vi "Lab Panel V4.6.vi"() -> ()   [LabVIEW 2013]
uses:
  <vilib>/Platform/TimedLoop/XDataNode/timing_clust.ctl
  <vilib>/Platform/TimedLoop/XDataNode/nitl_modes.ctl
  <vilib>/Platform/TimedLoop/XDataNode/wakeup.ctl
  Global 1.vi
  <vilib>/platform/TimedLoop/XDataNode/XDataNode.xnode
  <vilib>/Platform/TimedLoop/XDataNode/XDNodeRunTimeDep.lvlib
panel:
  in  "ADMIN PAGE":bool
  out "TEMP update":bool
  out "AI update":bool
  in  "Tab Control 2":T1(tab)
  out "SIG LAB05-2":T2 {"PF" format="%.2f"; "AMPS" format="%.1f"}
  out "SIG LAB05-1":T2 {"PF" format="%.2f"; "AMPS" format="%.1f"}
  out "SIG LAB04-2":T2 {"PF" format="%.2f"; "AMPS" format="%.1f"}
  out "SIG LAB04-1":T2 {"PF" format="%.2f"; "AMPS" format="%.1f"}
  out "SIG LAB03-2":T2 {"PF" format="%.2f"; "AMPS" format="%.1f"}
  out "SIG LAB03-1":T2 {"PF" format="%.2f"; "AMPS" format="%.1f"}
  out "SIG LAB02-2":T2 {"PF" format="%.2f"; "AMPS" format="%.1f"}
  in  "RUN LAB01-1":bool
  in  "O/I  LAB05-1":bool
  in  "O/I  LAB05-2":bool
  in  "O/I  LAB04-1":bool
  in  "O/I  LAB04-2":bool
  in  "O/I  LAB02-1":bool
  in  "O/I  LAB02-2":bool
  in  "O/I  LAB01-2":bool
  in  "O/I  LAB01-1":bool
  in  "O/I  LAB03-1":bool
  in  "RUN LAB05-2":bool
  in  "RUN LAB05-1":bool
  in  "RUN LAB04-2":bool
  in  "RUN LAB04-1":bool
  in  "RUN LAB03-2":bool
  in  "RUN LAB03-1":bool
  in  "RUN LAB02-2":bool
  in  "RUN LAB02-1":bool
  in  "RUN LAB01-2":bool
  in  "SELECT LAB05-2":T3(radio)
  in  "SELECT LAB05-1":T3(radio)
  in  "SELECT LAB04-2":T3(radio)
  in  "SELECT LAB04-1":T3(radio)
  in  "SELECT LAB03-2":T3(radio)
  in  "SELECT LAB03-1":T3(radio)
  in  "SELECT LAB02-2":T3(radio)
  in  "SELECT LAB02-1":T3(radio)
  in  "SELECT LAB01-2":T3(radio)
  in  "SELECT LAB01-1":T3(radio)
  in  "O/I  LAB03-2":bool
  out "SIG LAB01-1":T2 {"PF" format="%.2f"; "AMPS" format="%.1f"}
  out "SIG LAB01-2":T2 {"PF" format="%.2f"; "AMPS" format="%.1f"}
  out "SIG LAB02-1":T2 {"PF" format="%.2f"; "AMPS" format="%.1f"}
  out "DISP LAB05-2":T4 {"MINS" format="%.2g"}
  out "DISP LAB05-1":T4 {"MINS" format="%.2g"}
  out "DISP LAB04-2":T4 {"MINS" format="%.2g"}
  out "DISP LAB04-1":T4 {"MINS" format="%.2g"}
  out "DISP LAB03-2":T4 {"MINS" format="%.2g"}
  out "DISP LAB03-1":T4 {"MINS" format="%.2g"}
  in  "SET LAB05-2":T5={"NAME"="", "DESCRIPTION"="", "CYCLES"=5.0, "T-RISE mins"=0.0, "T-RISE deg C"=0.0} {"CYCLES" min=5.0 step=1.0}
  in  "SET LAB05-1":T5={"NAME"="", "DESCRIPTION"="", "CYCLES"=5.0, "T-RISE mins"=0.0, "T-RISE deg C"=0.0} {"CYCLES" min=5.0 step=1.0}
  in  "SET LAB04-2":T5={"NAME"="", "DESCRIPTION"="", "CYCLES"=5.0, "T-RISE mins"=0.0, "T-RISE deg C"=0.0} {"CYCLES" min=5.0 step=1.0}
  in  "SET LAB04-1":T5={"NAME"="", "DESCRIPTION"="", "CYCLES"=5.0, "T-RISE mins"=0.0, "T-RISE deg C"=0.0} {"CYCLES" min=5.0 step=1.0}
  in  "SET LAB03-2":T5={"NAME"="", "DESCRIPTION"="", "CYCLES"=5.0, "T-RISE mins"=0.0, "T-RISE deg C"=0.0} {"CYCLES" min=5.0 step=1.0}
  in  "SET LAB03-1":T5={"NAME"="", "DESCRIPTION"="", "CYCLES"=5.0, "T-RISE mins"=0.0, "T-RISE deg C"=0.0} {"CYCLES" min=5.0 step=1.0}
  out "DISP LAB02-2":T4 {"MINS" format="%.2g"}
  out "DISP LAB02-1":T4 {"MINS" format="%.2g"}
  in  "SET LAB02-2":T5={"NAME"="", "DESCRIPTION"="", "CYCLES"=5.0, "T-RISE mins"=0.0, "T-RISE deg C"=0.0} {"CYCLES" min=5.0 step=1.0}
  in  "SET LAB02-1":T5={"NAME"="", "DESCRIPTION"="", "CYCLES"=5.0, "T-RISE mins"=0.0, "T-RISE deg C"=0.0} {"CYCLES" min=5.0 step=1.0}
  out "RESULT LAB05-2":bool
  out "RESULT LAB05-1":bool
  out "RESULT LAB04-2":bool
  out "RESULT LAB04-1":bool
  out "RESULT LAB03-2":bool
  out "RESULT LAB03-1":bool
  out "RESULT LAB02-2":bool
  out "RESULT LAB02-1":bool
  out "RESULT LAB01-2":bool
  out "RESULT LAB01-1":bool
  in  "SET LAB01-1":T5={"NAME"="", "DESCRIPTION"="", "CYCLES"=5.0, "T-RISE mins"=0.0, "T-RISE deg C"=0.0} {"CYCLES" min=5.0 step=1.0}
  in  "SET LAB01-2":T5={"NAME"="", "DESCRIPTION"="", "CYCLES"=5.0, "T-RISE mins"=0.0, "T-RISE deg C"=0.0} {"CYCLES" min=5.0 step=1.0}
  out "DISP LAB01-1":T4 {"MINS" format="%.2g"}
  out "DISP LAB01-2":T4 {"MINS" format="%.2f"}
  out "TEMP RISE LAB05-2":cluster{"TL":dbl, "TN":dbl}
  out "TEMP RISE LAB05-1":cluster{"TL":dbl, "TN":dbl}
  out "TEMP RISE LAB04-2":cluster{"TL":dbl, "TN":dbl}
  out "TEMP RISE LAB04-1":cluster{"TL":dbl, "TN":dbl}
  out "TEMP RISE LAB03-2":cluster{"TL":dbl, "TN":dbl}
  out "TEMP RISE LAB03-1":cluster{"TL":dbl, "TN":dbl}
  out "TEMP RISE LAB02-2":cluster{"TL":dbl, "TN":dbl}
  out "TEMP RISE LAB02-1":cluster{"TL":dbl, "TN":dbl}
  out "TEMP RISE LAB01-2":cluster{"TL":dbl, "TN":dbl}
  out "TEMP RISE LAB01-1":cluster{"TL":dbl, "TN":dbl}
  in  "JIG OFF TIME (S)":dbl=2.0 min=2.0 max=10.0 step=0.5 format="%.1g"
  in  "JIG ON TIME (S)":dbl=1.0 min=1.0 max=10.0 step=0.5 format="%.1g"
  out "JIG LAB05-2":bool
  out "JIG LAB05-1":bool
  out "JIG LAB04-2":bool
  out "JIG LAB04-1":bool
  out "JIG LAB03-2":bool
  out "JIG LAB03-1":bool
  out "JIG LAB02-2":bool
  out "JIG LAB02-1":bool
  out "JIG LAB01-2":bool
  out "JIG LAB01-1":bool
  out "TEMP START LAB01-1":cluster{"TL":dbl, "TN":dbl}
  out "TEMP START LAB02-1":cluster{"TL":dbl, "TN":dbl}
  out "TEMP START LAB03-1":cluster{"TL":dbl, "TN":dbl}
  out "TEMP START LAB04-1":cluster{"TL":dbl, "TN":dbl}
  out "TEMP START LAB01-2":cluster{"TL":dbl, "TN":dbl}
  out "TEMP START LAB02-2":cluster{"TL":dbl, "TN":dbl}
  out "TEMP START LAB03-2":cluster{"TL":dbl, "TN":dbl}
  out "TEMP START LAB04-2":cluster{"TL":dbl, "TN":dbl}
  out "TEMP START LAB05-2":cluster{"TL":dbl, "TN":dbl}
  out "TEMP START LAB05-1":cluster{"TL":dbl, "TN":dbl}
  in  "MAIL SETTINGS":T6
  out "MAIL REPORT":string
  in  "TO (string):":string
  in  "Send Mail Now":bool
  in  "Auto Mail Send":bool
  in  "Network Directory":path
  out "CAL LAB01":T7 {"2 (TN) cal" min=0.0 step=0.01 format="%.2f"; "2 (TL) cal" min=0.0 step=0.01 format="%.2f"; "2 (PF) cal" min=0.0 step=0.01 format="%.2f"; "2 (V) cal" min=0.0 step=0.01 format="%.2f"; "2 (A) cal" min=0.0 step=0.01 format="%.2f"; "1 (TN) cal" min=0.0 step=0.01 format="%.2f"; "1 (TL) cal" min=0.0 step=0.01 format="%.2f"; "1 (PF) cal" min=0.0 step=0.01 format="%.2f"; "1 (V) cal" min=0.0 step=0.01 format="%.2f"; "1  (A) cal" min=0.0 step=0.01 format="%.2f"}
  out "CAL LAB03":T7 {"2 (TN) cal" min=0.0 step=0.01 format="%.2f"; "2 (TL) cal" min=0.0 step=0.01 format="%.2f"; "2 (PF) cal" min=0.0 step=0.01 format="%.2f"; "2 (V) cal" min=0.0 step=0.01 format="%.2f"; "2 (A) cal" min=0.0 step=0.01 format="%.2f"; "1 (TN) cal" min=0.0 step=0.01 format="%.2f"; "1 (TL) cal" min=0.0 step=0.01 format="%.2f"; "1 (PF) cal" min=0.0 step=0.01 format="%.2f"; "1 (V) cal" min=0.0 step=0.01 format="%.2f"; "1  (A) cal" min=0.0 step=0.01 format="%.2f"}
  out "CAL LAB02":T8 {"2 (TN) cal" min=0.0 step=0.01 format="%.2f"; "2 (TL) cal" min=0.0 step=0.01 format="%.2f"; "2 (PF) cal" min=0.0 step=0.01 format="%.2f"; "2 (V) cal" min=0.0 step=0.01 format="%.2f"; "2 (A) cal" min=0.0 step=0.01 format="%.2f"; "1 (TN) cal" min=0.0 step=0.01 format="%.2f"; "1 (TL) cal" min=0.0 step=0.01 format="%.2f"; "1 (PF) cal" min=0.0 step=0.01 format="%.2f"; "1 (V) cal" min=0.0 step=0.01 format="%.2f"; "1 (A) cal" min=0.0 step=0.01 format="%.2f"}
  out "CAL LAB05":T7 {"2 (TN) cal" min=0.0 step=0.01 format="%.2f"; "2 (TL) cal" min=0.0 step=0.01 format="%.2f"; "2 (PF) cal" min=0.0 step=0.01 format="%.2f"; "2 (V) cal" min=0.0 step=0.01 format="%.2f"; "2 (A) cal" min=0.0 step=0.01 format="%.2f"; "1 (TN) cal" min=0.0 step=0.01 format="%.2f"; "1 (TL) cal" min=0.0 step=0.01 format="%.2f"; "1 (PF) cal" min=0.0 step=0.01 format="%.2f"; "1 (V) cal" min=0.0 step=0.01 format="%.2f"; "1  (A) cal" min=0.0 step=0.01 format="%.2f"}
  out "CAL LAB04":T7 {"2 (TN) cal" min=0.0 step=0.01 format="%.2f"; "2 (TL) cal" min=0.0 step=0.01 format="%.2f"; "2 (PF) cal" min=0.0 step=0.01 format="%.2f"; "2 (V) cal" min=0.0 step=0.01 format="%.2f"; "2 (A) cal" min=0.0 step=0.01 format="%.2f"; "1 (TN) cal" min=0.0 step=0.01 format="%.2f"; "1 (TL) cal" min=0.0 step=0.01 format="%.2f"; "1 (PF) cal" min=0.0 step=0.01 format="%.2f"; "1 (V) cal" min=0.0 step=0.01 format="%.2f"; "1  (A) cal" min=0.0 step=0.01 format="%.2f"}
  out "calibration file error out":errorcluster
  in  "CALIBRATE":bool
  out "ON L05-2":cluster{"amps":dbl, "volts":dbl, "pf":dbl}
  out "ON L05-1":cluster{"amps":dbl, "volts":dbl, "pf":dbl}
  out "FAIL LAB05-2":cluster{"LO":dbl, "HI":dbl}
  out "FAIL LAB05-1":cluster{"LO":dbl, "HI":dbl}
  out "FAIL LAB04-2":cluster{"LO":dbl, "HI":dbl}
  out "FAIL LAB04-1":cluster{"LO":dbl, "HI":dbl}
  out "FAIL LAB03-2":cluster{"LO":dbl, "HI":dbl}
  out "FAIL LAB03-1":cluster{"LO":dbl, "HI":dbl}
  out "FAIL LAB02-2":cluster{"LO":dbl, "HI":dbl}
  out "FAIL LAB02-1":cluster{"LO":dbl, "HI":dbl}
  out "FAIL LAB01-2":cluster{"LO":dbl, "HI":dbl}
  out "FAIL LAB01-1":cluster{"LO":dbl, "HI":dbl}
  out "ON L01-1":cluster{"amps":dbl, "volts":dbl, "pf":dbl}
  out "ON L01-2":cluster{"amps":dbl, "volts":dbl, "pf":dbl}
  out "ON L02-1":cluster{"amps":dbl, "volts":dbl, "pf":dbl}
  out "ON L02-2":cluster{"amps":dbl, "volts":dbl, "pf":dbl}
  out "ON L03-1":cluster{"amps":dbl, "volts":dbl, "pf":dbl}
  out "ON L03-2":cluster{"amps":dbl, "volts":dbl, "pf":dbl}
  out "ON L04-1":cluster{"amps":dbl, "volts":dbl, "pf":dbl}
  out "ON L04-2":cluster{"amps":dbl, "volts":dbl, "pf":dbl}
  out "TEST VOLTS CHART":T9(graph)
  in  "Select  Cycle":enum32{"ON CYCLE", "OFF CYCLE"}(radio)
  out "TEST AMPS CHART":T9(graph)
  out "TEMPERATURE (N) CHART":T9(graph)
  out "TEMPERATURE (L) CHART":T9(graph)
  in  "SAMPLES":dbl
  in  "RATE (Hz)":dbl
  in  "JIG TEST":T10
  in  "C drive data root dir":path
  out "run lab05-2":bool
  out "run lab05-1":bool
  out "run lab04-2":bool
  out "run lab04-1":bool
  out "run lab03-2":bool
  out "run lab03-1":bool
  out "run lab02-2":bool
  out "run lab02-1":bool
  out "run lab01-2":bool
  out "run lab01-1":bool
  out "stop2":bool
  in  "Tab Control":T11(tab)
  out "LAB01-2 (GRAPH)":dynamicdata(graph)
  out "LAB01-1 (GRAPH)":dynamicdata(graph)
  out "LAB02-2 (GRAPH)":dynamicdata(graph)
  out "LAB02-1 (GRAPH)":dynamicdata(graph)
  out "LAB03-2 (GRAPH)":dynamicdata(graph)
  out "LAB03-1 (GRAPH)":dynamicdata(graph)
  out "LAB04-2 (GRAPH)":dynamicdata(graph)
  out "LAB04-1 (GRAPH)":dynamicdata(graph)
  out "LAB05-2 (GRAPH)":dynamicdata(graph)
  out "LAB05-1 (GRAPH)":dynamicdata(graph)
  out "LAB05 TEMP":T12
  out "LAB04 TEMP":T12
  out "LAB02 TEMP":T12
  out "LAB01 TEMP":T12
  out "LAB03 TEMP":T12
  out "Analog Error Array":errorcluster[](array[cluster])
  out "AI loop time":dbl format="%.6g"
  out "loops":dbl
  in  "loop  delay(mS)":dbl
  out "on loops":dbl
  out "off loops":dbl
  out "jig cycle":dbl
  out "TDMS LAB01-1":refnum<k34>
  out "data file error":errorcluster
  out "TDMS LAB02-1":refnum<k34>
  out "TDMS LAB01-2":refnum<k34>
  out "TDMS LAB02-2":refnum<k34>
  out "TDMS LAB03-1":refnum<k34>
  out "TDMS LAB03-2":refnum<k34>
  out "TDMS LAB04-1":refnum<k34>
  out "TDMS LAB04-2":refnum<k34>
  out "TDMS LAB05-1":refnum<k34>
  out "TDMS LAB05-2":refnum<k34>
  out "mail control":string
  out "File Time Stamp":timestamp
  in  "stop":bool
  in  "Select COM port":refnum<visa-resource-name>="COM6"
  out "COM port":refnum<visa-resource-name>="COM6"
  # "LAB01"
  # "LAB02"
  # "LAB05"
  # "LAB03"
  # "LAB04"
  # "LAB01"
  # "LAB02"
  # "LAB03"
  # "LAB04"
  # "LAB05"
  # "JIG SET"
  # "(Enter recipients address seperated by comma)"
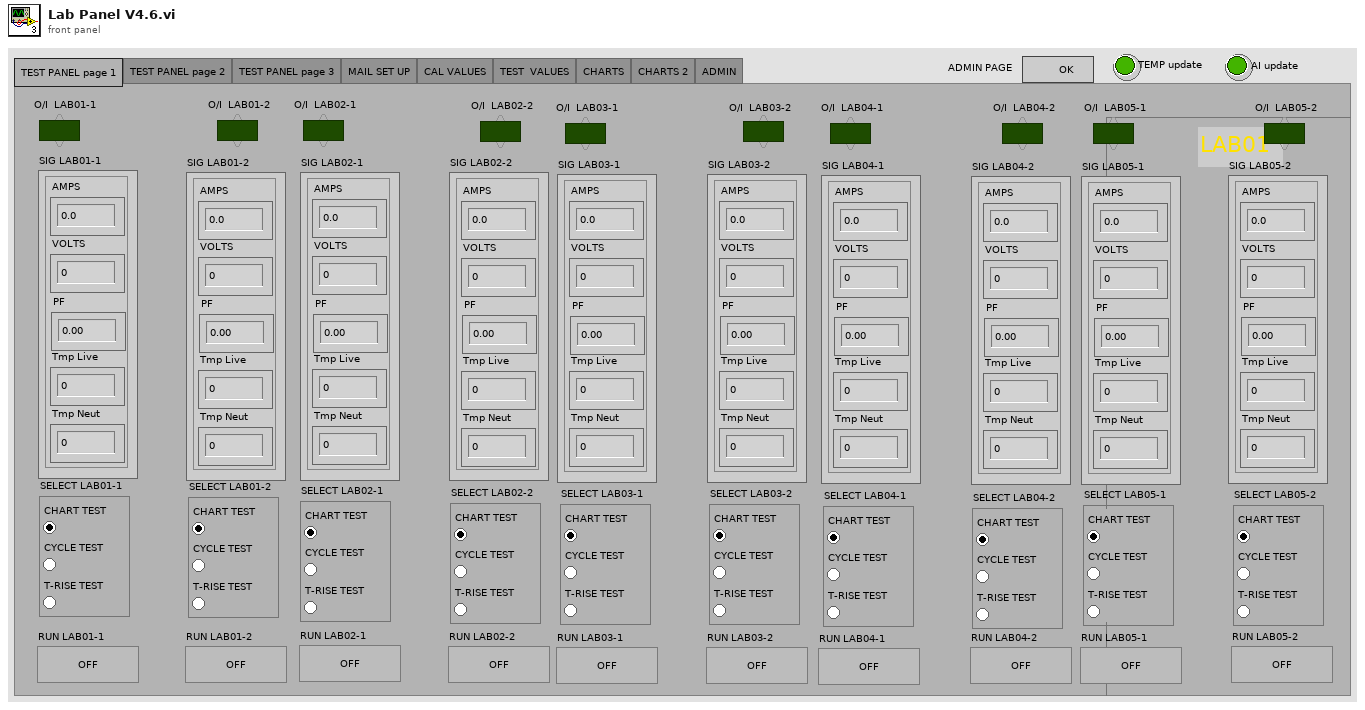
[diagram p1: front panel]
types:
  T1 = enum32{"TEST PANEL page 1", "TEST PANEL page 2", "TEST PANEL page 3", "MAIL SET UP", "CAL VALUES", "TEST  VALUES", "CHARTS", "CHARTS 2", "ADMIN"}
  T2 = cluster{"AMPS":dbl, "VOLTS":dbl, "PF":dbl, "Tmp Live":dbl, "Tmp Neut":dbl}
  T3 = enum32{"CHART TEST", "CYCLE TEST", "T-RISE TEST"}
  T4 = cluster{"CYCLE":dbl, "MINS":dbl, "STATUS":string}
  T5 = cluster{"NAME":string, "DESCRIPTION":string, "CYCLES":dbl, "T-RISE mins":dbl, "T-RISE deg C":dbl}
  T6 = cluster{"OUT SERVER ADDRESS":string, "FROM ACCOUNT":string, "USER NAME":string, "PASSWORD":string, "TEST MAIL":bool, "TEST MAIL STATUS":string, "mail error":errorcluster}
  T7 = cluster{"1  (A) cal":dbl, "1 (V) cal":dbl, "1 (PF) cal":dbl, "1 (TL) cal":dbl, "1 (TN) cal":dbl, "2 (A) cal":dbl, "2 (V) cal":dbl, "2 (PF) cal":dbl, "2 (TL) cal":dbl, "2 (TN) cal":dbl}
  T8 = cluster{"1 (A) cal":dbl, "1 (V) cal":dbl, "1 (PF) cal":dbl, "1 (TL) cal":dbl, "1 (TN) cal":dbl, "2 (A) cal":dbl, "2 (V) cal":dbl, "2 (PF) cal":dbl, "2 (TL) cal":dbl, "2 (TN) cal":dbl}
  T9 = cluster{"AMPS":dbl, "AMPS":dbl, "AMPS":dbl, "AMPS":dbl, "AMPS":dbl, "AMPS":dbl, "AMPS":dbl, "AMPS":dbl, "AMPS":dbl, "AMPS":dbl}
  T10 = cluster{" LAB01-1":bool, " LAB01-2":bool, "LAB02-1":bool, " LAB02-2":bool, "LAB03-1":bool, "LAB03-2":bool, "LAB04-1":bool, "LAB04-2":bool, "LAB05-1":bool, "LAB05-2":bool}
  T11 = enum32{"LAB01", "LAB02", "LAB03", "LAB04", "LAB05", "TEMPERATURE", "ERROR"}
  T12 = cluster{"T1 Live":dbl, "T1 Neut":dbl, "T2 Live":dbl, "T2 Neut":dbl, "ID":dbl, "ER":dbl}
  T13 = enum8{"Enabled", "Disabled", "Disabled and Grayed Out"}
  T14 = typedef "XDNodeRunTimeDep.lvlib/timing_clust.ctl" = cluster{"Expected End [f-1]":u64, "Actual End [f-1]":u64, "Finished Late? [f-1]":bool, "Expected End [i-1]":u64, "Actual End [i-1]":u64, "Finished Late? [i-1]":bool, "Expected Start [i]":u64, "Actual Start [i]":u64, "Expected Start [f]":u64, "Actual Start [f]":u64, "Source Name":string, "Structure Name":string, "Period":i64, "Deadline":i64, "Offset":i64, "Start":i64, "Priority":i32, "Timeout":i32, "Mode":T15, "Wakeup Reason":T16, "Error":errorcluster, "Source Type":string, "Secondary Source Type":string, "Global End Time":u64, "Global Start Time":u64, "Frame Duration":u64, "Iteration Duration":u64, "Assigned CPU":i32, "I/O Scan Engine Mode":u32}
  T15 = typedef "XDNodeRunTimeDep.lvlib/nitl_modes.ctl" = enum32{"No Change", "Process missed periods, maintain original phase", "Discard missed periods, maintain original phase", "Process missed periods, ignore original phase", "Discard missed periods, ignore original phase"}
  T16 = typedef "XDNodeRunTimeDep.lvlib/wakeup.ctl" = enum32{"Normal", "Aborted", "Asynchronous wakeup", "Timing source error", "Timed loop error", "Timeout"}
  T17 = enum16{"open", "open or create", "create or replace", "create", "open (read-only)"}
  T18 = enum16{"open", "replace", "create", "open or create", "replace or create", "replace or create with confirmation"}
  T19 = cluster{"SET LAB01-1":cluster{"NAME":string, "DESCRIPTION":string, "CYCLES":dbl, "T-RISE mins":dbl, "T-RISE deg C":dbl}, "SET LAB01-2":cluster{"NAME":string, "DESCRIPTION":string, "CYCLES":dbl, "T-RISE mins":dbl, "T-RISE deg C":dbl}, "SET LAB02-1":cluster{"NAME":string, "DESCRIPTION":string, "CYCLES":dbl, "T-RISE mins":dbl, "T-RISE deg C":dbl}, "SET LAB02-2":cluster{"NAME":string, "DESCRIPTION":string, "CYCLES":dbl, "T-RISE mins":dbl, "T-RISE deg C":dbl}, "SET LAB03-1":cluster{"NAME":string, "DESCRIPTION":string, "CYCLES":dbl, "T-RISE mins":dbl, "T-RISE deg C":dbl}, "SET LAB03-2":cluster{"NAME":string, "DESCRIPTION":string, "CYCLES":dbl, "T-RISE mins":dbl, "T-RISE deg C":dbl}, "SET LAB04-1":cluster{"NAME":string, "DESCRIPTION":string, "CYCLES":dbl, "T-RISE mins":dbl, "T-RISE deg C":dbl}, "SET LAB04-2":cluster{"NAME":string, "DESCRIPTION":string, "CYCLES":dbl, "T-RISE mins":dbl, "T-RISE deg C":dbl}, "SET LAB05-1":cluster{"NAME":string, "DESCRIPTION":string, "CYCLES":dbl, "T-RISE mins":dbl, "T-RISE deg C":dbl}, "SET LAB05-2":cluster{"NAME":string, "DESCRIPTION":string, "CYCLES":dbl, "T-RISE mins":dbl, "T-RISE deg C":dbl}, "Network Directory":path, "C drive data root dir":path, "RATE (Hz)":dbl, "SAMPLES":dbl, "Select COM port":refnum<visa-resource-name>}
  T20 = cluster{"MAIL SETTINGS":cluster{"OUT SERVER ADDRESS":string, "FROM ACCOUNT":string, "USER NAME":string, "PASSWORD":string, "TEST MAIL":bool, "TEST MAIL STATUS":string, "mail error":errorcluster}, "Auto Mail Send":bool, string}
  T21 = cluster{"T1":dbl, "T2":dbl, "T3":dbl, "T4":dbl, "ID":dbl, "ER":dbl}
  T22 = cluster{"LAB01-1 (A)":dbl, "LAB01-1 (V)":dbl, "LAB01-1 (PF)":dbl, "LAB01-2 (A)":dbl, "LAB01-2 (V)":dbl, "LAB01-2 (PF)":dbl}
  T23 = cluster{"LAB02-1 (A)":dbl, "LAB02-1 (V)":dbl, "LAB02-1 (PF)":dbl, "LAB02-2 (A)":dbl, "LAB02-2 (V)":dbl, "LAB02-2 (PF)":dbl}
  T24 = cluster{"LAB03-1 (A)":dbl, "LAB03-1 (V)":dbl, "LAB03-1 (PF)":dbl, "LAB03-2 (A)":dbl, "LAB03-2 (V)":dbl, "LAB03-2 (PF)":dbl}
  T25 = cluster{"LAB04-1 (A)":dbl, "LAB04-1 (V)":dbl, "LAB04-1 (PF)":dbl, "LAB04-2 (A)":dbl, "LAB04-2 (V)":dbl, "LAB04-2 (PF)":dbl}
  T26 = cluster{"LAB05-1 (A)":dbl, "LAB05-1 (V)":dbl, "LAB05-1 (PF)":dbl, "LAB05-2 (A)":dbl, "LAB05-2 (V)":dbl, "LAB05-2 (PF)":dbl}
  T27 = cluster{"VOLTS":dbl, "VOLTS":dbl, "VOLTS":dbl, "VOLTS":dbl, "VOLTS":dbl, "VOLTS":dbl, "VOLTS":dbl, "VOLTS":dbl, "VOLTS":dbl, "VOLTS":dbl}
  T28 = cluster{"Tmp Live":dbl, "Tmp Live":dbl, "Tmp Live":dbl, "Tmp Live":dbl, "Tmp Live":dbl, "Tmp Live":dbl, "Tmp Live":dbl, "Tmp Live":dbl, "Tmp Live":dbl, "Tmp Live":dbl}
  T29 = cluster{"Tmp Neut":dbl, "Tmp Neut":dbl, "Tmp Neut":dbl, "Tmp Neut":dbl, "Tmp Neut":dbl, "Tmp Neut":dbl, "Tmp Neut":dbl, "Tmp Neut":dbl, "Tmp Neut":dbl, "Tmp Neut":dbl}
  T30 = cluster{"FAIL LAB01-1":cluster{"LO":dbl, "HI":dbl}, "SIG LAB01-1":cluster{"AMPS":dbl, "VOLTS":dbl, "PF":dbl, "Tmp Live":dbl, "Tmp Neut":dbl}, "TEMP START LAB01-1":cluster{"TL":dbl, "TN":dbl}, "DISP LAB01-1":cluster{"CYCLE":dbl, "MINS":dbl, "STATUS":string}, "SET LAB01-1":cluster{"NAME":string, "DESCRIPTION":string, "CYCLES":dbl, "T-RISE mins":dbl, "T-RISE deg C":dbl}, "TDMS LAB01-1":refnum<k34>}
  T31 = cluster{"FAIL LAB01-2":cluster{"LO":dbl, "HI":dbl}, "SIG LAB01-2":cluster{"AMPS":dbl, "VOLTS":dbl, "PF":dbl, "Tmp Live":dbl, "Tmp Neut":dbl}, "TEMP START LAB01-2":cluster{"TL":dbl, "TN":dbl}, "DISP LAB01-2":cluster{"CYCLE":dbl, "MINS":dbl, "STATUS":string}, "SET LAB01-2":cluster{"NAME":string, "DESCRIPTION":string, "CYCLES":dbl, "T-RISE mins":dbl, "T-RISE deg C":dbl}, "TDMS LAB01-2":refnum<k34>}
  T32 = cluster{"FAIL LAB02-1":cluster{"LO":dbl, "HI":dbl}, "SIG LAB02-1":cluster{"AMPS":dbl, "VOLTS":dbl, "PF":dbl, "Tmp Live":dbl, "Tmp Neut":dbl}, "TEMP START LAB02-1":cluster{"TL":dbl, "TN":dbl}, "DISP LAB02-1":cluster{"CYCLE":dbl, "MINS":dbl, "STATUS":string}, "SET LAB02-1":cluster{"NAME":string, "DESCRIPTION":string, "CYCLES":dbl, "T-RISE mins":dbl, "T-RISE deg C":dbl}, "TDMS LAB02-1":refnum<k34>}
  T33 = cluster{"FAIL LAB02-2":cluster{"LO":dbl, "HI":dbl}, "SIG LAB02-2":cluster{"AMPS":dbl, "VOLTS":dbl, "PF":dbl, "Tmp Live":dbl, "Tmp Neut":dbl}, "TEMP START LAB02-2":cluster{"TL":dbl, "TN":dbl}, "DISP LAB02-2":cluster{"CYCLE":dbl, "MINS":dbl, "STATUS":string}, "SET LAB02-2":cluster{"NAME":string, "DESCRIPTION":string, "CYCLES":dbl, "T-RISE mins":dbl, "T-RISE deg C":dbl}, "TDMS LAB02-2":refnum<k34>}
  T34 = cluster{"FAIL LAB03-1":cluster{"LO":dbl, "HI":dbl}, "SIG LAB03-1":cluster{"AMPS":dbl, "VOLTS":dbl, "PF":dbl, "Tmp Live":dbl, "Tmp Neut":dbl}, "TEMP START LAB03-1":cluster{"TL":dbl, "TN":dbl}, "DISP LAB03-1":cluster{"CYCLE":dbl, "MINS":dbl, "STATUS":string}, "SET LAB03-1":cluster{"NAME":string, "DESCRIPTION":string, "CYCLES":dbl, "T-RISE mins":dbl, "T-RISE deg C":dbl}, "TDMS LAB03-1":refnum<k34>}
  T35 = cluster{"FAIL LAB03-2":cluster{"LO":dbl, "HI":dbl}, "SIG LAB03-2":cluster{"AMPS":dbl, "VOLTS":dbl, "PF":dbl, "Tmp Live":dbl, "Tmp Neut":dbl}, "TEMP START LAB03-2":cluster{"TL":dbl, "TN":dbl}, "DISP LAB03-2":cluster{"CYCLE":dbl, "MINS":dbl, "STATUS":string}, "SET LAB03-2":cluster{"NAME":string, "DESCRIPTION":string, "CYCLES":dbl, "T-RISE mins":dbl, "T-RISE deg C":dbl}, "TDMS LAB03-2":refnum<k34>}
  T36 = cluster{"FAIL LAB04-1":cluster{"LO":dbl, "HI":dbl}, "SIG LAB04-1":cluster{"AMPS":dbl, "VOLTS":dbl, "PF":dbl, "Tmp Live":dbl, "Tmp Neut":dbl}, "TEMP START LAB04-1":cluster{"TL":dbl, "TN":dbl}, "DISP LAB04-1":cluster{"CYCLE":dbl, "MINS":dbl, "STATUS":string}, "SET LAB04-1":cluster{"NAME":string, "DESCRIPTION":string, "CYCLES":dbl, "T-RISE mins":dbl, "T-RISE deg C":dbl}, "TDMS LAB04-1":refnum<k34>}
  T37 = cluster{"FAIL LAB04-2":cluster{"LO":dbl, "HI":dbl}, "SIG LAB04-2":cluster{"AMPS":dbl, "VOLTS":dbl, "PF":dbl, "Tmp Live":dbl, "Tmp Neut":dbl}, "TEMP START LAB04-2":cluster{"TL":dbl, "TN":dbl}, "DISP LAB04-2":cluster{"CYCLE":dbl, "MINS":dbl, "STATUS":string}, "SET LAB04-2":cluster{"NAME":string, "DESCRIPTION":string, "CYCLES":dbl, "T-RISE mins":dbl, "T-RISE deg C":dbl}, "TDMS LAB04-2":refnum<k34>}
  T38 = cluster{"FAIL LAB05-1":cluster{"LO":dbl, "HI":dbl}, "SIG LAB05-1":cluster{"AMPS":dbl, "VOLTS":dbl, "PF":dbl, "Tmp Live":dbl, "Tmp Neut":dbl}, "TEMP START LAB05-1":cluster{"TL":dbl, "TN":dbl}, "DISP LAB05-1":cluster{"CYCLE":dbl, "MINS":dbl, "STATUS":string}, "SET LAB05-1":cluster{"NAME":string, "DESCRIPTION":string, "CYCLES":dbl, "T-RISE mins":dbl, "T-RISE deg C":dbl}, "TDMS LAB05-1":refnum<k34>}
  T39 = cluster{"FAIL LAB05-2":cluster{"LO":dbl, "HI":dbl}, "SIG LAB05-2":cluster{"AMPS":dbl, "VOLTS":dbl, "PF":dbl, "Tmp Live":dbl, "Tmp Neut":dbl}, "TEMP START LAB05-2":cluster{"TL":dbl, "TN":dbl}, "DISP LAB05-2":cluster{"CYCLE":dbl, "MINS":dbl, "STATUS":string}, "SET LAB05-2":cluster{"NAME":string, "DESCRIPTION":string, "CYCLES":dbl, "T-RISE mins":dbl, "T-RISE deg C":dbl}, "TDMS LAB05-2":refnum<k34>}
  T40 = cluster{"MAIL SETTINGS":cluster{"OUT SERVER ADDRESS":string, "FROM ACCOUNT":string, "USER NAME":string, "PASSWORD":string, "TEST MAIL":bool, "TEST MAIL STATUS":string, "mail error":errorcluster}, "Auto Mail Send":bool, "TO (string):":string}
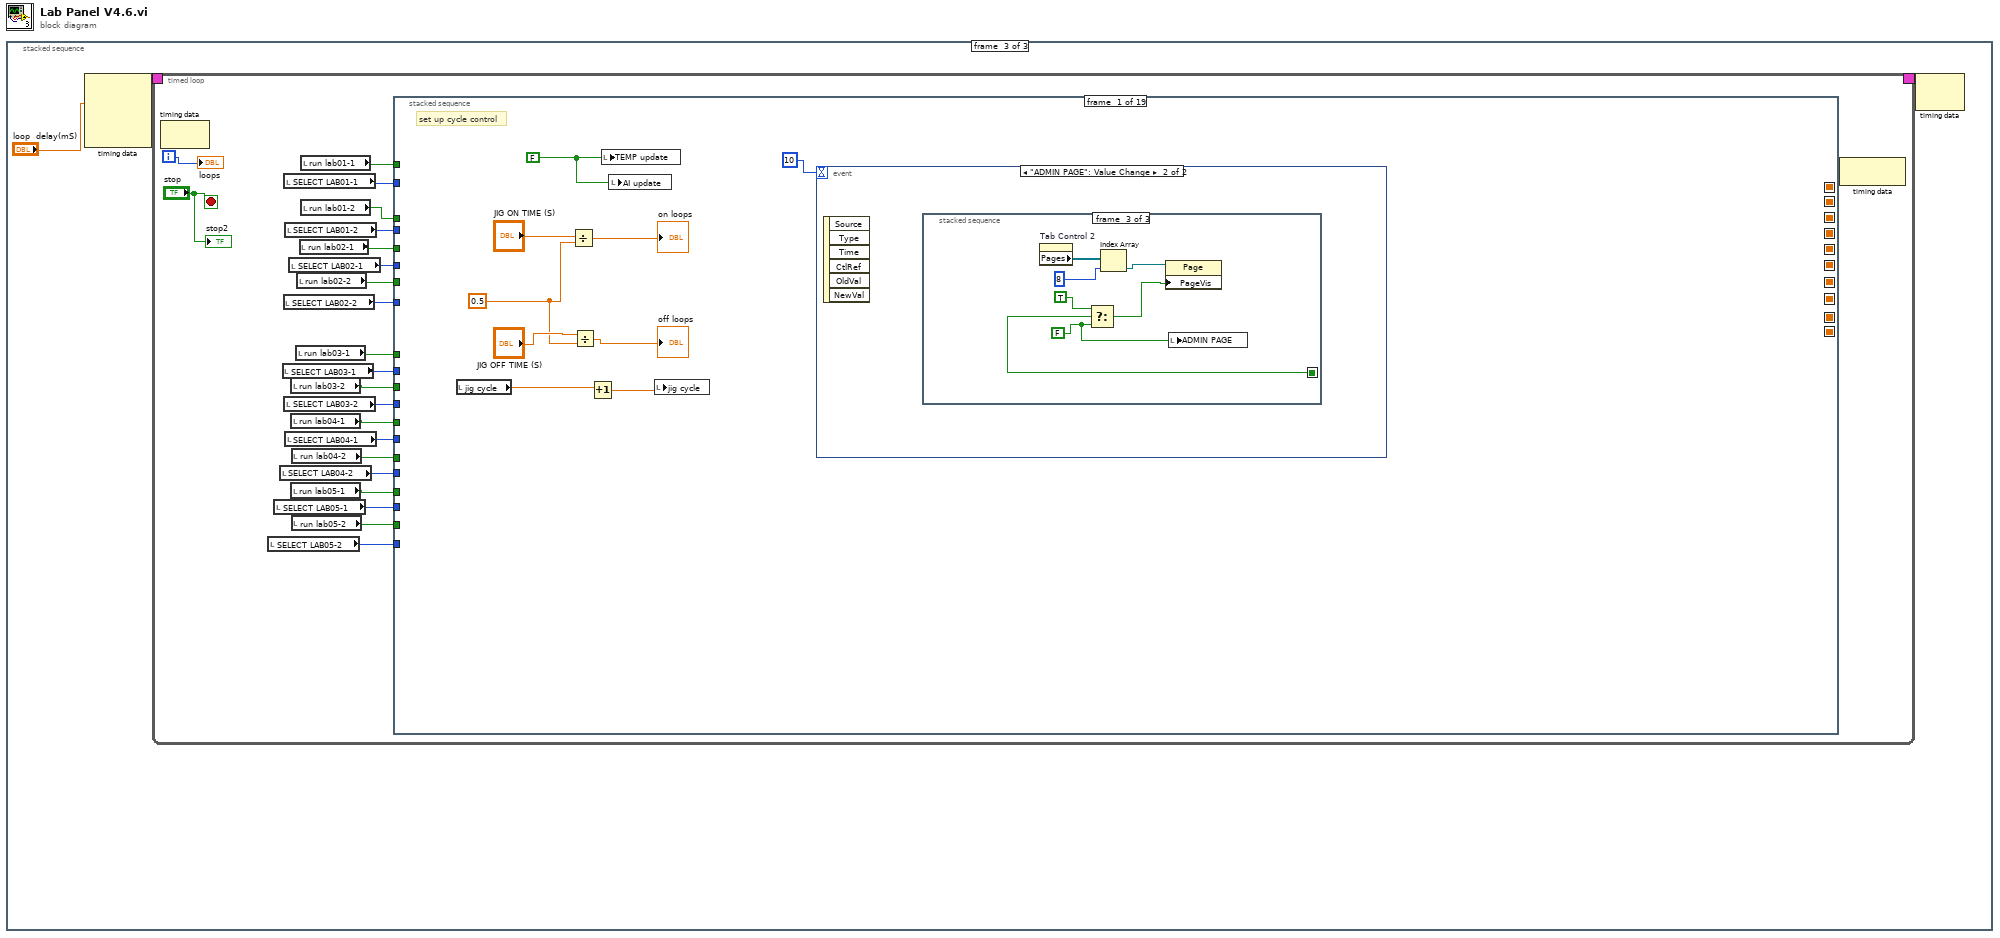
[diagram p0: block diagram]
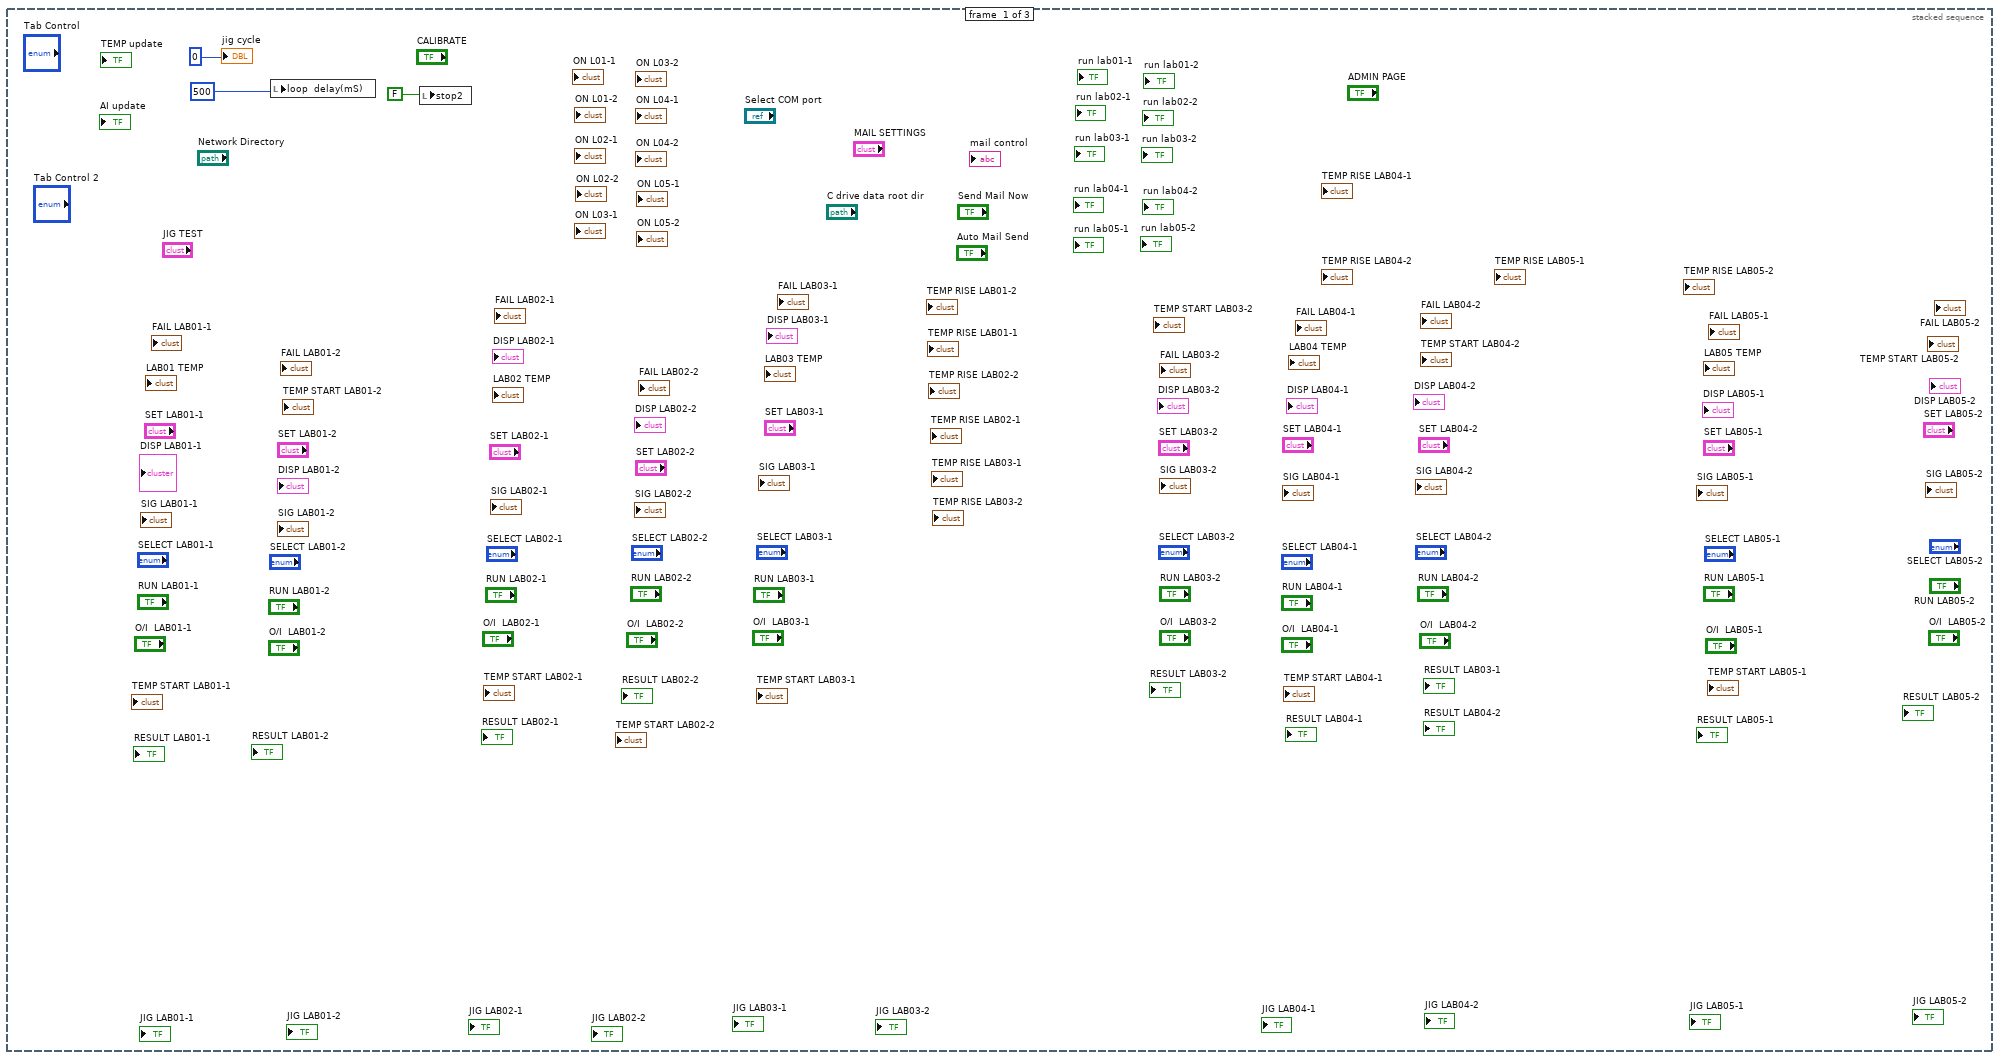
[diagram p2: hidden frame]
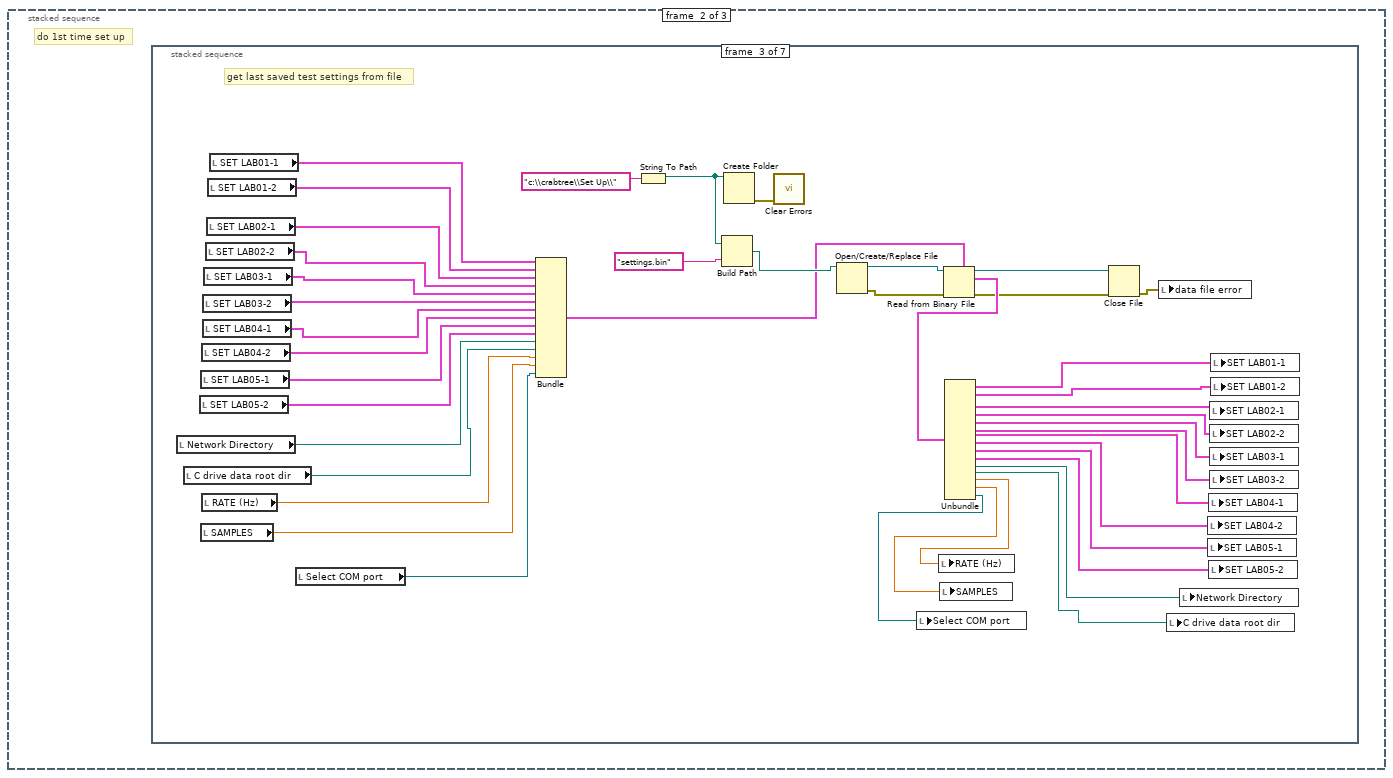
[diagram p3: hidden frame]
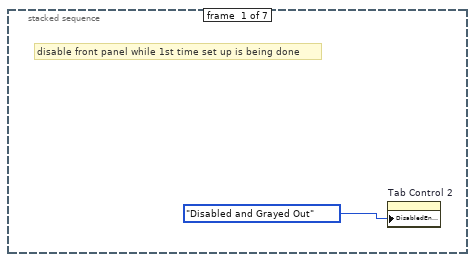
[diagram p4: hidden frame]
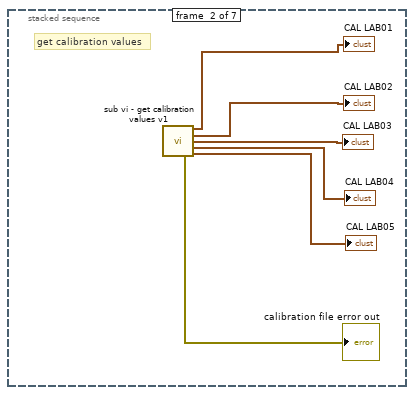
[diagram p5: hidden frame]
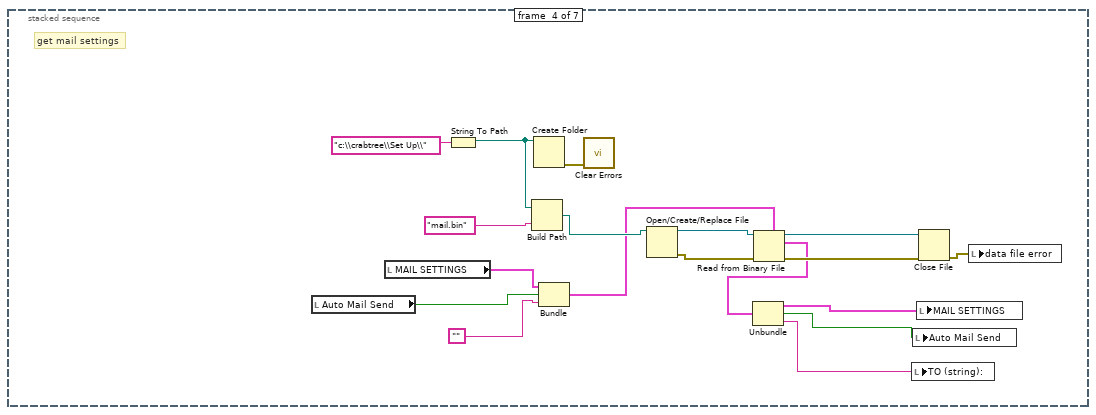
[diagram p6: hidden frame]
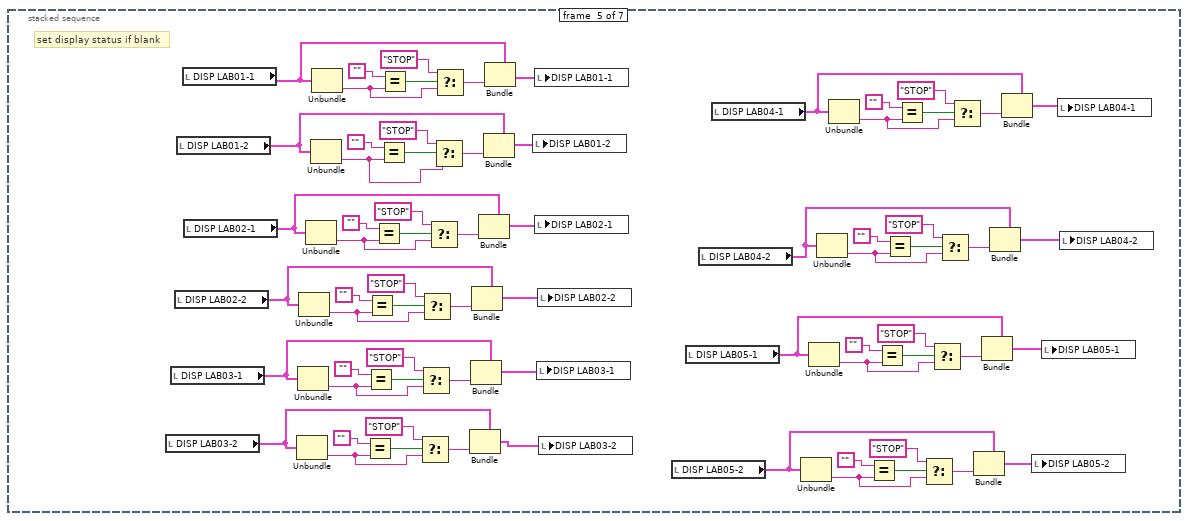
[diagram p7: hidden frame]
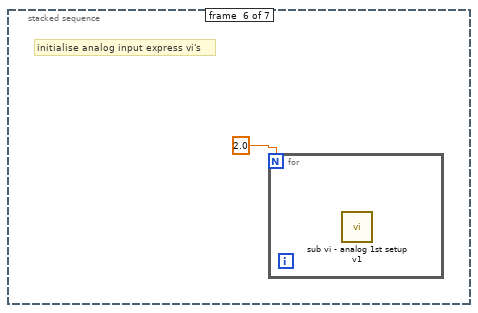
[diagram p8: hidden frame]
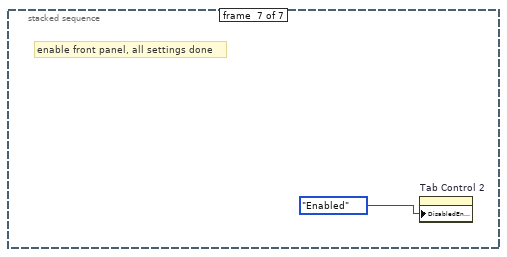
[diagram p9: hidden frame]
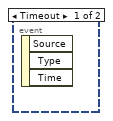
[diagram p10: hidden frame]
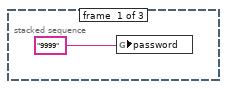
[diagram p11: hidden frame]
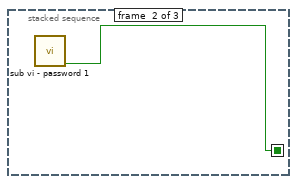
[diagram p12: hidden frame]
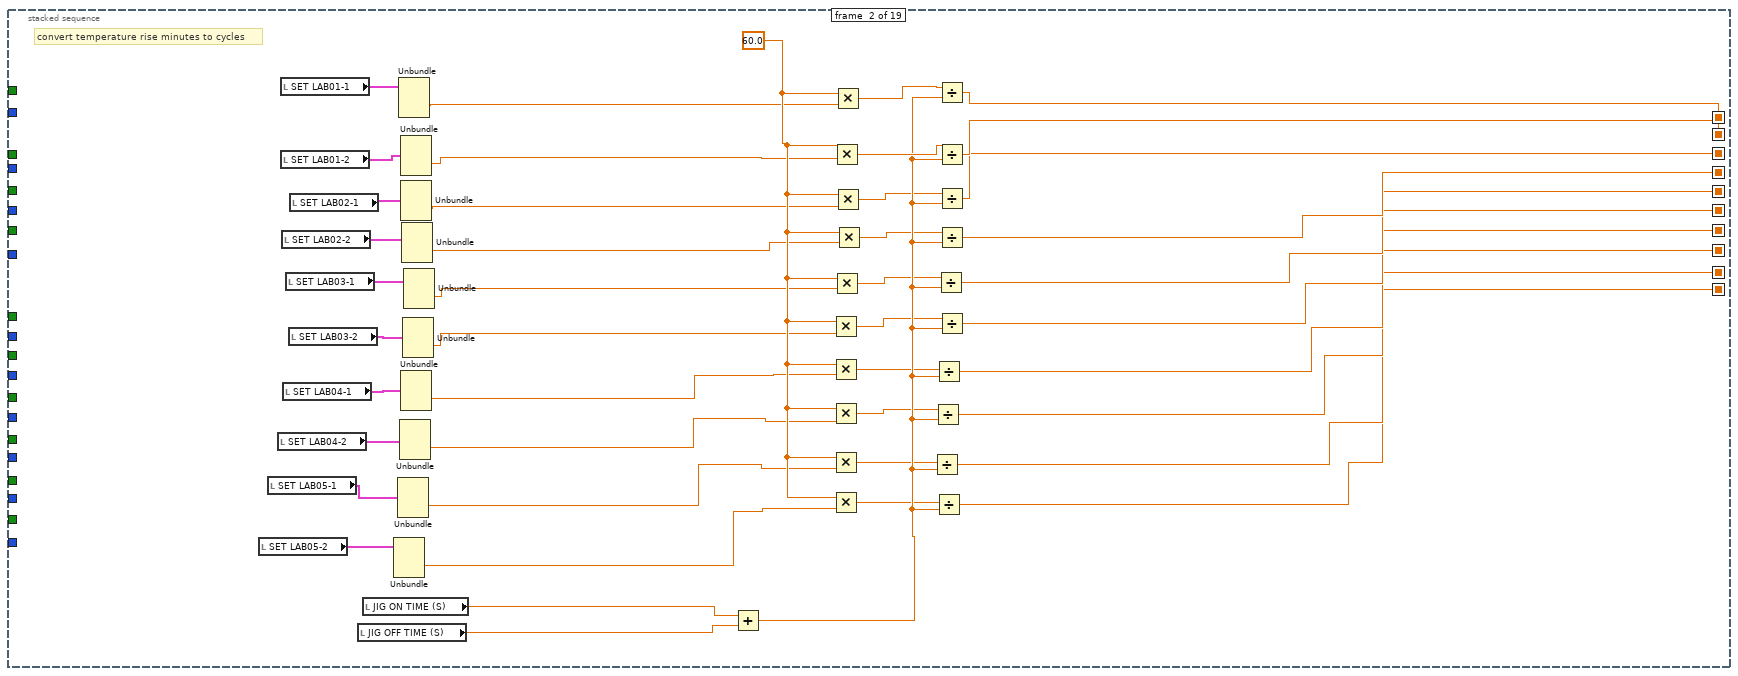
[diagram p13: hidden frame]
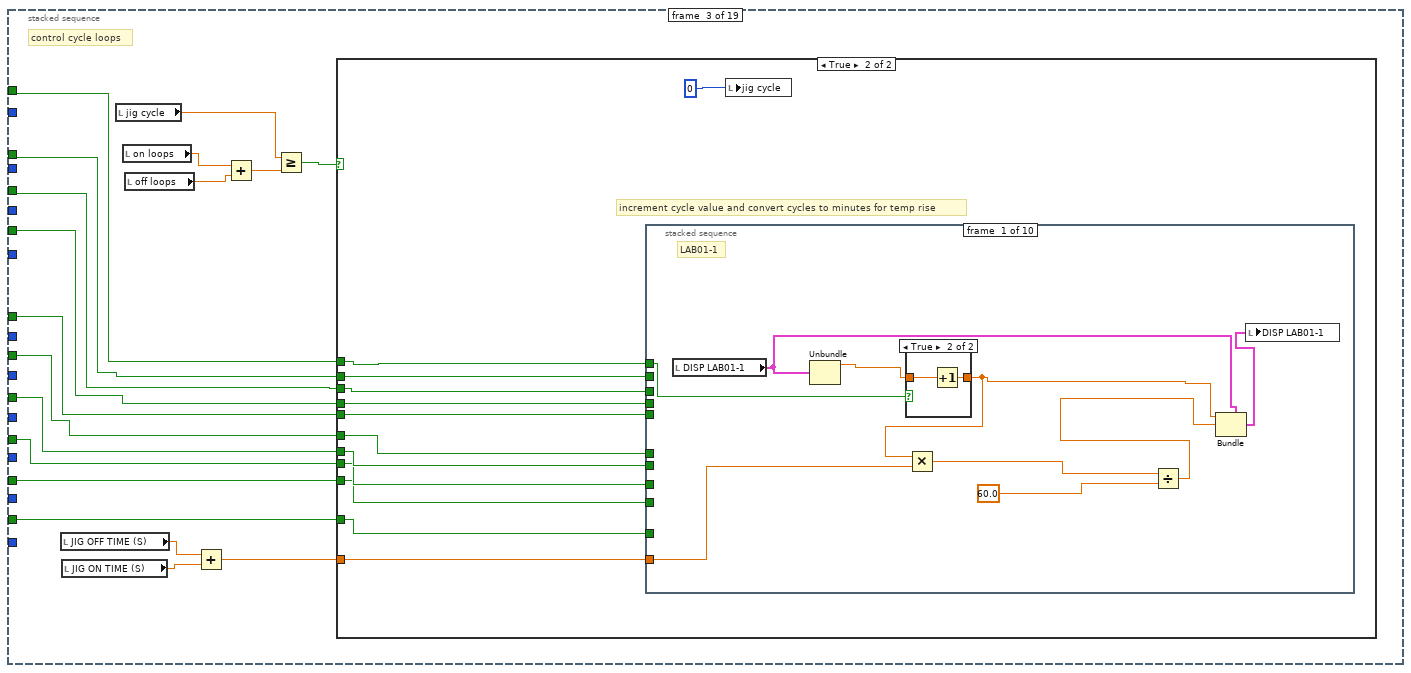
[diagram p14: hidden frame]
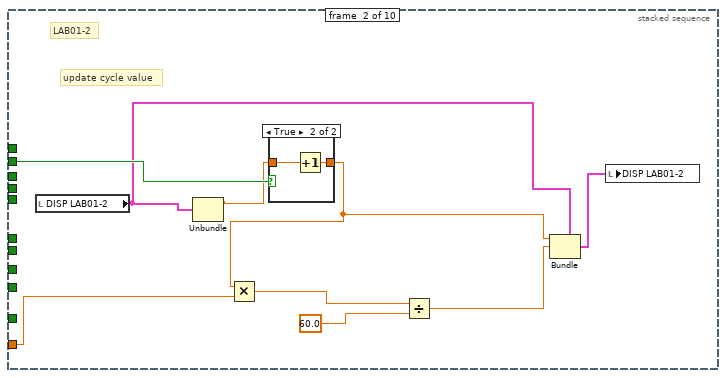
[diagram p17: hidden frame]
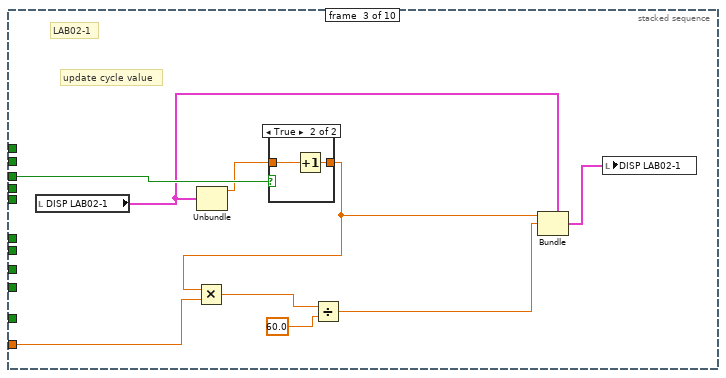
[diagram p19: hidden frame]
diagram:
  n1 = stacked-sequence {
    frame #0 {
      n2 = local write "loop  delay(mS)"(500) -> ()
      n3 = local write "stop2"(FALSE) -> ()
      "jig cycle" <- 0
    }
    frame #1 {
      # "do 1st time set up"
      n4 = stacked-sequence {
        frame #0 {
          # "disable front panel while 1st time set up is being done"
          n5 = property on="Tab Control 2" class="TabCtl (strict)"("DisabledEnum"=T13."Disabled and Grayed Out" ("Disabled")) -> ()  [unwired: 2 in, 2 out]
        }
        frame #1 {
          # "get calibration values"
          n6 = call "sub vi - get calibration values v1.vi"() -> ("LAB01 (CAL)"=→"CAL LAB01":T7, "LAB02 (CAL)"=→"CAL LAB02":T8, "LAB03 (CAL)"=→"CAL LAB03":T7, "LAB04 (CAL)"=→"CAL LAB04":T7, "calibration file error out"=→"calibration file error out":errorcluster, "LAB05 (CAL)"=→"CAL LAB05":T7)  [unwired: 10 in]
        }
        frame #2 {
          # "get last saved test settings from file"
          n7 = local read "Network Directory"() -> (w19:path)
          n8 = local read "C drive data root dir"() -> (w17:path)
          n9 = local read "SET LAB05-2"() -> (w49:T5)
          n10 = local read "SET LAB05-1"() -> (w50:T5)
          n11 = local read "SAMPLES"() -> (w15:dbl)
          n12 = local read "SET LAB04-2"() -> (w51:T5)
          n13 = local read "RATE (Hz)"() -> (w16:dbl)
          n14 = local read "SET LAB03-2"() -> (w48:T5)
          n15 = local read "SET LAB04-1"() -> (w52:T5)
          n16 = local read "SET LAB03-1"() -> (w47:T5)
          n17 = local read "SET LAB02-2"() -> (w46:T5)
          n18 = local read "SET LAB02-1"() -> (w45:T5)
          n19 = local read "SET LAB01-2"() -> (w44:T5)
          n20 = local read "SET LAB01-1"() -> (w43:T5)
          n21 = local read "Select COM port"() -> (w11:refnum<visa-resource-name>)
          n22 = Bundle("SET LAB01-1"=w43, "SET LAB01-2"=w44, "SET LAB02-1"=w45, "SET LAB02-2"=w46, "SET LAB03-1"=w47, "SET LAB03-2"=w48, "SET LAB04-1"=w52, "SET LAB04-2"=w51, "SET LAB05-1"=w50, "SET LAB05-2"=w49, "Network Directory"=w19, "C drive data root dir"=w17, "RATE (Hz)"=w16, "SAMPLES"=w15, "Select COM port"=w11) -> (w36:T19)  [unwired: 1 in]
          n23 = String To Path(string="c:\\crabtree\\Set Up\\") -> (path=w40:path)
          n24 = Build Path(base path=w40, name or relative path="settings.bin") -> (appended path=w38:path)
          n25 = Create Folder(path (use dialog)=w40) -> (error out=w42:errorcluster)  [unwired: 2 in, 2 out]
          n26 = call <vilib>:"Clear Errors.vi"("error in (no error)"=w42) -> ()  [unwired: 6 in, 1 out]
          n27 = Open/Create/Replace File(file path (use dialog)=w38) -> (refnum out=w35:refnum<file>, error out=w37:errorcluster)  [unwired: 5 in, 1 out]
          n28 = Read from Binary File(5:w36, 8:w37, 11:w35) -> (0:w32:errorcluster, 2:w34:T19, 3:w33:refnum<file>)  [unwired: 3 in, 1 out]
          n29 = Unbundle(w34) -> ("SET LAB01-1"=w30:T5, "SET LAB01-2"=w29:T5, "SET LAB02-1"=w28:T5, "SET LAB02-2"=w27:T5, "SET LAB03-1"=w26:T5, "SET LAB03-2"=w25:T5, "SET LAB04-1"=w24:T5, "SET LAB04-2"=w23:T5, "SET LAB05-1"=w22:T5, "SET LAB05-2"=w21:T5, "Network Directory"=w20:path, "C drive data root dir"=w18:path, "RATE (Hz)"=w13:dbl, "SAMPLES"=w14:dbl, "Select COM port"=w12:refnum<visa-resource-name>)
          n30 = local write "Select COM port"(w12) -> ()
          n31 = local write "RATE (Hz)"(w13) -> ()
          n32 = local write "SAMPLES"(w14) -> ()
          n33 = Close File(refnum=w33, error in=w32) -> (error out=w31:errorcluster)  [unwired: 1 out]
          n34 = local write "data file error"(w31) -> ()
          n35 = local write "C drive data root dir"(w18) -> ()
          n36 = local write "Network Directory"(w20) -> ()
          n37 = local write "SET LAB04-2"(w23) -> ()
          n38 = local write "SET LAB05-1"(w22) -> ()
          n39 = local write "SET LAB04-1"(w24) -> ()
          n40 = local write "SET LAB05-2"(w21) -> ()
          n41 = local write "SET LAB02-1"(w28) -> ()
          n42 = local write "SET LAB02-2"(w27) -> ()
          n43 = local write "SET LAB03-1"(w26) -> ()
          n44 = local write "SET LAB03-2"(w25) -> ()
          n45 = local write "SET LAB01-1"(w30) -> ()
          n46 = local write "SET LAB01-2"(w29) -> ()
        }
        frame #3 {
          # "get mail settings"
          n47 = local read "Auto Mail Send"() -> (w56:bool)
          n48 = local read "MAIL SETTINGS"() -> (w60:T6)
          n49 = String To Path(string="c:\\crabtree\\Set Up\\") -> (path=w68:path)
          n50 = Build Path(base path=w68, name or relative path="mail.bin") -> (appended path=w66:path)
          n51 = Create Folder(path (use dialog)=w68) -> (error out=w70:errorcluster)  [unwired: 2 in, 2 out]
          n52 = Bundle("MAIL SETTINGS"=w60, "Auto Mail Send"=w56, "") -> (w59:T20)  [unwired: 1 in]
          n53 = call <vilib>:"Clear Errors.vi"("error in (no error)"=w70) -> ()  [unwired: 6 in, 1 out]
          n54 = Open/Create/Replace File(file path (use dialog)=w66) -> (refnum out=w64:refnum<file>, error out=w65:errorcluster)  [unwired: 5 in, 1 out]
          n55 = Read from Binary File(5:w59, 8:w65, 11:w64) -> (0:w62:errorcluster, 2:w58:T20, 3:w63:refnum<file>)  [unwired: 3 in, 1 out]
          n56 = Unbundle(w58) -> ("MAIL SETTINGS"=w57:T6, "Auto Mail Send"=w55:bool, w54:string)
          n57 = local write "TO (string):"(w54) -> ()
          n58 = local write "Auto Mail Send"(w55) -> ()
          n59 = local write "MAIL SETTINGS"(w57) -> ()
          n60 = Close File(refnum=w63, error in=w62) -> (error out=w61:errorcluster)  [unwired: 1 out]
          n61 = local write "data file error"(w61) -> ()
        }
        frame #4 {
          # "set display status if blank"
          n62 = local read "DISP LAB03-2"() -> (w100:T4)
          n63 = local read "DISP LAB03-1"() -> (w107:T4)
          n64 = local read "DISP LAB02-2"() -> (w114:T4)
          n65 = local read "DISP LAB01-2"() -> (w127:T4)
          n66 = local read "DISP LAB01-1"() -> (w136:T4)
          n67 = local read "DISP LAB02-1"() -> (w121:T4)
          n68 = Unbundle(w100) -> ("STATUS"=w102:string)  [unwired: 2 out]
          n69 = Unbundle(w107) -> ("STATUS"=w109:string)  [unwired: 2 out]
          n70 = Unbundle(w114) -> ("STATUS"=w116:string)  [unwired: 2 out]
          n71 = Unbundle(w121) -> ("STATUS"=w123:string)  [unwired: 2 out]
          n72 = Unbundle(w127) -> ("STATUS"=w130:string)  [unwired: 2 out]
          n73 = Unbundle(w136) -> ("STATUS"=w137:string)  [unwired: 2 out]
          n74 = Equal?(x="", y=w102) -> (x = y?=w104:bool)
          n75 = Equal?(x="", y=w109) -> (x = y?=w111:bool)
          n76 = Equal?(x="", y=w116) -> (x = y?=w118:bool)
          n77 = Equal?(x="", y=w123) -> (x = y?=w125:bool)
          n78 = Equal?(x="", y=w130) -> (x = y?=w132:bool)
          n79 = Equal?(x="", y=w137) -> (x = y?=w139:bool)
          n80 = Select(t="STOP", s=w104, f=w102) -> (s? t:f=w101:string)
          n81 = Select(t="STOP", s=w111, f=w109) -> (s? t:f=w108:string)
          n82 = Select(t="STOP", s=w118, f=w116) -> (s? t:f=w115:string)
          n83 = Select(t="STOP", s=w125, f=w123) -> (s? t:f=w122:string)
          n84 = Select(t="STOP", s=w132, f=w130) -> (s? t:f=w129:string)
          n85 = Select(t="STOP", s=w139, f=w137) -> (s? t:f=w135:string)
          n86 = Bundle(cluster=w100, "STATUS"=w101) -> (w99:T4)  [unwired: 2 in]
          n87 = Bundle(cluster=w107, "STATUS"=w108) -> (w106:T4)  [unwired: 2 in]
          n88 = Bundle(cluster=w114, "STATUS"=w115) -> (w113:T4)  [unwired: 2 in]
          n89 = Bundle(cluster=w121, "STATUS"=w122) -> (w120:T4)  [unwired: 2 in]
          n90 = Bundle(cluster=w127, "STATUS"=w129) -> (w128:T4)  [unwired: 2 in]
          n91 = Bundle(cluster=w136, "STATUS"=w135) -> (w134:T4)  [unwired: 2 in]
          n92 = local write "DISP LAB01-2"(w128) -> ()
          n93 = local write "DISP LAB01-1"(w134) -> ()
          n94 = local write "DISP LAB02-1"(w120) -> ()
          n95 = local write "DISP LAB03-1"(w106) -> ()
          n96 = local write "DISP LAB02-2"(w113) -> ()
          n97 = local write "DISP LAB03-2"(w99) -> ()
          n98 = local read "DISP LAB05-2"() -> (w72:T4)
          n99 = local read "DISP LAB05-1"() -> (w79:T4)
          n100 = local read "DISP LAB04-2"() -> (w81:T4)
          n101 = local read "DISP LAB04-1"() -> (w83:T4)
          n102 = Unbundle(w72) -> ("STATUS"=w74:string)  [unwired: 2 out]
          n103 = Unbundle(w79) -> ("STATUS"=w85:string)  [unwired: 2 out]
          n104 = Unbundle(w81) -> ("STATUS"=w90:string)  [unwired: 2 out]
          n105 = Unbundle(w83) -> ("STATUS"=w95:string)  [unwired: 2 out]
          n106 = Equal?(x="", y=w74) -> (x = y?=w76:bool)
          n107 = Equal?(x="", y=w85) -> (x = y?=w87:bool)
          n108 = Equal?(x="", y=w90) -> (x = y?=w92:bool)
          n109 = Equal?(x="", y=w95) -> (x = y?=w97:bool)
          n110 = Select(t="STOP", s=w76, f=w74) -> (s? t:f=w73:string)
          n111 = Select(t="STOP", s=w87, f=w85) -> (s? t:f=w84:string)
          n112 = Select(t="STOP", s=w92, f=w90) -> (s? t:f=w89:string)
          n113 = Select(t="STOP", s=w97, f=w95) -> (s? t:f=w94:string)
          n114 = Bundle(cluster=w72, "STATUS"=w73) -> (w71:T4)  [unwired: 2 in]
          n115 = Bundle(cluster=w79, "STATUS"=w84) -> (w78:T4)  [unwired: 2 in]
          n116 = Bundle(cluster=w81, "STATUS"=w89) -> (w80:T4)  [unwired: 2 in]
          n117 = Bundle(cluster=w83, "STATUS"=w94) -> (w82:T4)  [unwired: 2 in]
          n118 = local write "DISP LAB05-2"(w71) -> ()
          n119 = local write "DISP LAB05-1"(w78) -> ()
          n120 = local write "DISP LAB04-1"(w82) -> ()
          n121 = local write "DISP LAB04-2"(w80) -> ()
        }
        frame #5 {
          # "initialise analog input express vi's"
          n122 = for {
            N: 2.0 -> [_]
            n123 = call "sub vi - analog 1st setup v1.vi"() -> ()  [unwired: 11 in, 5 out]
          }
        }
        frame #6 {
          # "enable front panel, all settings done"
          n124 = property on="Tab Control 2" class="TabCtl (strict)"("DisabledEnum"=T13."Enabled" ("Disabled")) -> ()  [unwired: 2 in, 2 out]
        }
      }
    }
    frame #2 {
      n125 = node-c288("loop  delay(mS)") -> (w145:T14)  [unwired: 3 in]
      n126 = timed-loop {
        timing: w145 -> [_]
        timing-out: [_] -> w144
        i -> [w167]
        stop <- "stop" stop-if-true
        n127 = node-c288() -> ()  [unwired: 1 in, 1 out]
        n128 = local read "SELECT LAB05-2"() -> (w147:T3)
        n129 = local read "SELECT LAB05-1"() -> (w148:T3)
        n130 = local read "SELECT LAB04-2"() -> (w149:T3)
        n131 = local read "SELECT LAB03-1"() -> (w152:T3)
        n132 = local read "SELECT LAB02-2"() -> (w153:T3)
        n133 = local read "SELECT LAB01-1"() -> (w156:T3)
        n134 = local read "SELECT LAB03-2"() -> (w151:T3)
        n135 = local read "SELECT LAB01-2"() -> (w155:T3)
        n136 = local read "SELECT LAB04-1"() -> (w150:T3)
        n137 = local read "SELECT LAB02-1"() -> (w154:T3)
        n138 = local read "run lab03-2"() -> (w161:bool)
        n139 = local read "run lab04-1"() -> (w160:bool)
        n140 = local read "run lab05-1"() -> (w158:bool)
        n141 = local read "run lab04-2"() -> (w159:bool)
        n142 = local read "run lab05-2"() -> (w157:bool)
        n143 = local read "run lab03-1"() -> (w162:bool)
        n144 = local read "run lab02-2"() -> (w163:bool)
        n145 = local read "run lab02-1"() -> (w164:bool)
        n146 = local read "run lab01-1"() -> (w166:bool)
        n147 = local read "run lab01-2"() -> (w165:bool)
        n148 = stacked-sequence {
          seq-local: [_ w229 _ _ _ _ _ _ _ _ _ _ _ _ _ _ _ _ _] -> [_ _ _ _ _ w1764 _ _ _ _ _ _ _ _ _ _ _ _ _]
          seq-local: [_ w228 _ _ _ _ _ _ _ _ _ _ _ _ _ _ _ _ _] -> [_ _ _ _ _ w1763 _ _ _ _ _ _ _ _ _ _ _ _ _]
          seq-local: [_ w215 _ _ _ _ _ _ _ _ _ _ _ _ _ _ _ _ _] -> [_ _ _ _ _ w1762 _ _ _ _ _ _ _ _ _ _ _ _ _]
          seq-local: [_ w214 _ _ _ _ _ _ _ _ _ _ _ _ _ _ _ _ _] -> [_ _ _ _ _ w1761 _ _ _ _ _ _ _ _ _ _ _ _ _]
          seq-local: [_ w213 _ _ _ _ _ _ _ _ _ _ _ _ _ _ _ _ _] -> [_ _ _ _ _ w1760 _ _ _ _ _ _ _ _ _ _ _ _ _]
          seq-local: [_ w212 _ _ _ _ _ _ _ _ _ _ _ _ _ _ _ _ _] -> [_ _ _ _ _ w1759 _ _ _ _ _ _ _ _ _ _ _ _ _]
          seq-local: [_ w211 _ _ _ _ _ _ _ _ _ _ _ _ _ _ _ _ _] -> [_ _ _ _ _ w1758 _ _ _ _ _ _ _ _ _ _ _ _ _]
          seq-local: [_ w210 _ _ _ _ _ _ _ _ _ _ _ _ _ _ _ _ _] -> [_ _ _ _ _ w1757 _ _ _ _ _ _ _ _ _ _ _ _ _]
          seq-local: [_ w209 _ _ _ _ _ _ _ _ _ _ _ _ _ _ _ _ _] -> [_ _ _ _ _ w1756 _ _ _ _ _ _ _ _ _ _ _ _ _]
          seq-local: [_ w208 _ _ _ _ _ _ _ _ _ _ _ _ _ _ _ _ _] -> [_ _ _ _ _ w1755 _ _ _ _ _ _ _ _ _ _ _ _ _]
          tunnel: w166 -> [_ _ w245 w410 w1354 w1784 w2094 w2339 _ _ _ _ _ w2815 _ w3742 _ _ w4020]
          tunnel: w165 -> [_ _ w244 w408 w1353 w1783 w2095 w2338 _ _ _ _ _ w2814 _ w3740 _ _ w4019]
          tunnel: w164 -> [_ _ w243 w406 w1352 w1782 w2093 w2337 _ _ _ _ _ w2813 _ w3738 _ _ w4018]
          tunnel: w163 -> [_ _ w242 w404 w1351 w1781 w2092 w2336 _ _ _ _ _ w2812 _ w3736 _ _ w4017]
          tunnel: w162 -> [_ _ w241 w402 w1350 w1780 w2091 w2335 _ _ _ _ _ w2811 _ w3734 _ _ w4016]
          tunnel: w161 -> [_ _ w240 w400 w1349 w1779 w2090 w2334 _ _ _ _ _ w2810 _ w3732 _ _ w4015]
          tunnel: w160 -> [_ _ w239 w398 w1348 w1778 w2089 w2333 _ _ _ _ _ w2809 _ w3730 _ _ w4014]
          tunnel: w159 -> [_ _ w238 w396 w1347 w1777 w2088 w2332 _ _ _ _ _ w2808 _ w3728 _ _ w4013]
          tunnel: w158 -> [_ _ w237 w394 w1346 w1776 w2087 w2331 _ _ _ _ _ w2807 _ w3726 _ _ w4012]
          tunnel: w157 -> [_ _ w236 w392 w1345 w1775 w2086 w2330 _ _ _ _ _ w2806 _ w3724 _ _ w4011]
          tunnel: w156 -> [_ _ _ w409 w1344 w1774 _ _ _ _ _ _ _ _ _ w3744 _ _ _]
          tunnel: w155 -> [_ _ _ w407 w1343 w1773 _ _ _ _ _ _ _ _ _ w3739 _ _ _]
          tunnel: w154 -> [_ _ _ w405 w1342 w1772 _ _ _ _ _ _ _ _ _ w3737 _ _ _]
          tunnel: w153 -> [_ _ _ w403 w1341 w1771 _ _ _ _ _ _ _ _ _ w3735 _ _ _]
          tunnel: w152 -> [_ _ _ w401 w1340 w1770 _ _ _ _ _ _ _ _ _ w3733 _ _ _]
          tunnel: w151 -> [_ _ _ w399 w1339 w1769 _ _ _ _ _ _ _ _ _ w3731 _ _ _]
          tunnel: w150 -> [_ _ _ w397 w1338 w1768 _ _ _ _ _ _ _ _ _ w3729 _ _ _]
          tunnel: w149 -> [_ _ _ w395 w1337 w1767 _ _ _ _ _ _ _ _ _ w3727 _ _ _]
          tunnel: w148 -> [_ _ _ w393 w1336 w1766 _ _ _ _ _ _ _ _ _ w3725 _ _ _]
          tunnel: w147 -> [_ _ _ w391 w1335 w1765 _ _ _ _ _ _ _ _ _ w3723 _ _ _]
          frame #0 {
            w171 = FALSE
            w176 = 0.5
            # "set up cycle control"
            n149 = local read "jig cycle"() -> (w175:dbl)
            n150 = Divide(x="JIG ON TIME (S)", y=w176) -> (x/y=→"on loops":dbl)
            n151 = Divide(x="JIG OFF TIME (S)", y=w176) -> (x/y=→"off loops":dbl)
            n152 = Increment(x=w175) -> (x+1=w174:dbl)
            n153 = local write "TEMP update"(w171) -> ()
            n154 = local write "AI update"(w171) -> ()
            n155 = local write "jig cycle"(w174) -> ()
            n156 = event shown="[1] \"ADMIN PAGE\": Value Change" {
              selector: _ -> [_ _]
              dyn-events: _ -> [_ _]
              timeout: 10 -> [_ _]
              event Timeout {
                n157 = event-data() -> ()  [unwired: 1 in, 3 out]
              }
              event "ADMIN PAGE": Value Change {
                n158 = event-data() -> ()  [unwired: 1 in, 6 out]
                n159 = stacked-sequence {
                  seq-local: [_ w180 _] -> [_ _ w181]
                  frame #0 {
                    n160 = global write "Global 1.vi" "password"("9999") -> ()
                  }
                  frame #1 {
                    n161 = call "sub vi - password 1.vi"() -> ("RESULT"=w180:bool)  [unwired: 11 in]
                  }
                  frame #2 {
                    w183 = FALSE
                    n162 = property on="Tab Control 2" class="TabCtl (strict)"() -> ("Pages"=w187:refnum<vi>[])  [unwired: 2 in, 2 out]
                    n163 = Select(t=TRUE, s=w181, f=w183) -> (s? t:f=w182:bool)
                    n164 = Index Array(array=w187, index=8) -> (element=w185:refnum<vi>)
                    n165 = property class="Page"(reference=w185, "PageVis"=w182) -> ()  [unwired: 1 in, 2 out]
                    n166 = local write "ADMIN PAGE"(w183) -> ()
                  }
                }
              }
            }
          }
          frame #1 {
            w225 = 60.0
            # "convert temperature rise minutes to cycles"
            n167 = local read "SET LAB05-2"() -> (w189:T5)
            n168 = local read "SET LAB05-1"() -> (w191:T5)
            n169 = local read "SET LAB04-2"() -> (w193:T5)
            n170 = local read "SET LAB01-1"() -> (w207:T5)
            n171 = local read "SET LAB01-2"() -> (w205:T5)
            n172 = local read "SET LAB02-2"() -> (w201:T5)
            n173 = local read "SET LAB04-1"() -> (w195:T5)
            n174 = local read "SET LAB03-1"() -> (w199:T5)
            n175 = local read "SET LAB03-2"() -> (w197:T5)
            n176 = local read "SET LAB02-1"() -> (w203:T5)
            n177 = local read "JIG OFF TIME (S)"() -> (w230:dbl)
            n178 = local read "JIG ON TIME (S)"() -> (w231:dbl)
            n179 = Unbundle(w189) -> ("T-RISE mins"=w188:dbl)  [unwired: 4 out]
            n180 = Unbundle(w191) -> ("T-RISE mins"=w190:dbl)  [unwired: 4 out]
            n181 = Unbundle(w207) -> ("T-RISE mins"=w206:dbl)  [unwired: 4 out]
            n182 = Unbundle(w193) -> ("T-RISE mins"=w192:dbl)  [unwired: 4 out]
            n183 = Unbundle(w205) -> ("T-RISE mins"=w204:dbl)  [unwired: 4 out]
            n184 = Unbundle(w203) -> ("T-RISE mins"=w202:dbl)  [unwired: 4 out]
            n185 = Unbundle(w195) -> ("T-RISE mins"=w194:dbl)  [unwired: 4 out]
            n186 = Unbundle(w201) -> ("T-RISE mins"=w200:dbl)  [unwired: 4 out]
            n187 = Unbundle(w197) -> ("T-RISE mins"=w196:dbl)  [unwired: 4 out]
            n188 = Unbundle(w199) -> ("T-RISE mins"=w198:dbl)  [unwired: 4 out]
            n189 = Add(x=w231, y=w230) -> (x+y=w224:dbl)
            n190 = Multiply(x=w225, y=w196) -> (x*y=w220:dbl)
            n191 = Multiply(x=w225, y=w194) -> (x*y=w219:dbl)
            n192 = Multiply(x=w225, y=w192) -> (x*y=w218:dbl)
            n193 = Multiply(x=w225, y=w190) -> (x*y=w217:dbl)
            n194 = Multiply(x=w225, y=w188) -> (x*y=w216:dbl)
            n195 = Multiply(x=w225, y=w204) -> (x*y=w226:dbl)
            n196 = Multiply(x=w225, y=w198) -> (x*y=w221:dbl)
            n197 = Multiply(x=w225, y=w206) -> (x*y=w227:dbl)
            n198 = Multiply(x=w225, y=w202) -> (x*y=w223:dbl)
            n199 = Multiply(x=w225, y=w200) -> (x*y=w222:dbl)
            n200 = Divide(x=w217, y=w224) -> (x/y=w209:dbl)
            n201 = Divide(x=w218, y=w224) -> (x/y=w210:dbl)
            n202 = Divide(x=w219, y=w224) -> (x/y=w211:dbl)
            n203 = Divide(x=w216, y=w224) -> (x/y=w208:dbl)
            n204 = Divide(x=w221, y=w224) -> (x/y=w213:dbl)
            n205 = Divide(x=w227, y=w224) -> (x/y=w229:dbl)
            n206 = Divide(x=w226, y=w224) -> (x/y=w228:dbl)
            n207 = Divide(x=w223, y=w224) -> (x/y=w215:dbl)
            n208 = Divide(x=w222, y=w224) -> (x/y=w214:dbl)
            n209 = Divide(x=w220, y=w224) -> (x/y=w212:dbl)
          }
          frame #2 {
            # "control cycle loops"
            n210 = local read "JIG OFF TIME (S)"() -> (w234:dbl)
            n211 = local read "JIG ON TIME (S)"() -> (w233:dbl)
            n212 = local read "jig cycle"() -> (w247:dbl)
            n213 = local read "on loops"() -> (w249:dbl)
            n214 = local read "off loops"() -> (w248:dbl)
            n215 = Add(x=w234, y=w233) -> (x+y=w232:dbl)
            n216 = Add(x=w249, y=w248) -> (x+y=w235:dbl)
            n217 = Greater Or Equal?(x=w247, y=w235) -> (x >= y?=w246:bool)
            n218 = case shown="True" w246 {
              tunnel: w245 -> [_ w260]
              tunnel: w244 -> [_ w259]
              tunnel: w243 -> [_ w258]
              tunnel: w242 -> [_ w257]
              tunnel: w241 -> [_ w256]
              tunnel: w240 -> [_ w255]
              tunnel: w239 -> [_ w254]
              tunnel: w238 -> [_ w253]
              tunnel: w237 -> [_ w252]
              tunnel: w236 -> [_ w251]
              tunnel: w232 -> [_ w250]
              frame False {
              }
              frame True {
                # "increment cycle value and convert cycles to minutes for temp rise"
                n219 = stacked-sequence {
                  tunnel: w260 -> [w270 _ _ _ _ _ _ _ _ _]
                  tunnel: w259 -> [_ w282 _ _ _ _ _ _ _ _]
                  tunnel: w258 -> [_ _ w294 _ _ _ _ _ _ _]
                  tunnel: w257 -> [_ _ _ w306 _ _ _ _ _ _]
                  tunnel: w256 -> [_ _ _ _ w318 _ _ _ _ _]
                  tunnel: w255 -> [_ _ _ _ _ w330 _ _ _ _]
                  tunnel: w254 -> [_ _ _ _ _ _ w342 _ _ _]
                  tunnel: w253 -> [_ _ _ _ _ _ _ w354 _ _]
                  tunnel: w252 -> [_ _ _ _ _ _ _ _ w366 _]
                  tunnel: w251 -> [_ _ _ _ _ _ _ _ _ w378]
                  tunnel: w250 -> [w267 w279 w291 w303 w315 w327 w339 w351 w363 w375]
                  frame #0 {
                    # "LAB01-1"
                    n220 = local read "DISP LAB01-1"() -> (w265:T4)
                    n221 = Unbundle(w265) -> ("CYCLE"=w266:dbl)  [unwired: 2 out]
                    n222 = case shown="True" w270 {
                      tunnel: w266 -> [w271 w273]
                      tunnel: [w271 w272] -> w264
                      frame False {
                      }
                      frame True {
                        n223 = Increment(x=w273) -> (x+1=w272:dbl)
                      }
                    }
                    n224 = Multiply(x=w264, y=w267) -> (x*y=w268:dbl)
                    n225 = Divide(x=w268, y=60.0) -> (x/y=w263:dbl)
                    n226 = Bundle(cluster=w265, "CYCLE"=w264, "MINS"=w263) -> (w262:T4)  [unwired: 1 in]
                    n227 = local write "DISP LAB01-1"(w262) -> ()
                  }
                  frame #1 {
                    # "update cycle value"
                    # "LAB01-2"
                    n228 = local read "DISP LAB01-2"() -> (w277:T4)
                    n229 = Unbundle(w277) -> ("CYCLE"=w278:dbl)  [unwired: 2 out]
                    n230 = case shown="True" w282 {
                      tunnel: w278 -> [w283 w285]
                      tunnel: [w283 w284] -> w275
                      frame False {
                      }
                      frame True {
                        n231 = Increment(x=w285) -> (x+1=w284:dbl)
                      }
                    }
                    n232 = Multiply(x=w275, y=w279) -> (x*y=w280:dbl)
                    n233 = Divide(x=w280, y=60.0) -> (x/y=w274:dbl)
                    n234 = Bundle(cluster=w277, "CYCLE"=w275, "MINS"=w274) -> (w276:T4)  [unwired: 1 in]
                    n235 = local write "DISP LAB01-2"(w276) -> ()
                  }
                  frame #2 {
                    # "update cycle value"
                    # "LAB02-1"
                    n236 = local read "DISP LAB02-1"() -> (w289:T4)
                    n237 = Unbundle(w289) -> ("CYCLE"=w290:dbl)  [unwired: 2 out]
                    n238 = case shown="True" w294 {
                      tunnel: [w295 w297] -> w287
                      tunnel: w290 -> [w295 w296]
                      frame False {
                      }
                      frame True {
                        n239 = Increment(x=w296) -> (x+1=w297:dbl)
                      }
                    }
                    n240 = Multiply(x=w287, y=w291) -> (x*y=w292:dbl)
                    n241 = Divide(x=w292, y=60.0) -> (x/y=w286:dbl)
                    n242 = Bundle(cluster=w289, "CYCLE"=w287, "MINS"=w286) -> (w288:T4)  [unwired: 1 in]
                    n243 = local write "DISP LAB02-1"(w288) -> ()
                  }
                  frame #3 {
                    # "update cycle value"
                    # "LAB02-2"
                    n244 = local read "DISP LAB02-2"() -> (w301:T4)
                    n245 = Unbundle(w301) -> ("CYCLE"=w302:dbl)  [unwired: 2 out]
                    n246 = case shown="True" w306 {
                      tunnel: [w307 w309] -> w300
                      tunnel: w302 -> [w307 w308]
                      frame False {
                      }
                      frame True {
                        n247 = Increment(x=w308) -> (x+1=w309:dbl)
                      }
                    }
                    n248 = Multiply(x=w300, y=w303) -> (x*y=w304:dbl)
                    n249 = Divide(x=w304, y=60.0) -> (x/y=w299:dbl)
                    n250 = Bundle(cluster=w301, "CYCLE"=w300, "MINS"=w299) -> (w298:T4)  [unwired: 1 in]
                    n251 = local write "DISP LAB02-2"(w298) -> ()
                  }
                  frame #4 {
                    # "update cycle value"
                    # "LAB03-1"
                    n252 = local read "DISP LAB03-1"() -> (w313:T4)
                    n253 = Unbundle(w313) -> ("CYCLE"=w314:dbl)  [unwired: 2 out]
                    n254 = case shown="True" w318 {
                      tunnel: [w319 w321] -> w310
                      tunnel: w314 -> [w319 w320]
                      frame False {
                      }
                      frame True {
                        n255 = Increment(x=w320) -> (x+1=w321:dbl)
                      }
                    }
                    n256 = Multiply(x=w310, y=w315) -> (x*y=w316:dbl)
                    n257 = Divide(x=w316, y=60.0) -> (x/y=w311:dbl)
                    n258 = Bundle(cluster=w313, "CYCLE"=w310, "MINS"=w311) -> (w312:T4)  [unwired: 1 in]
                    n259 = local write "DISP LAB03-1"(w312) -> ()
                  }
                  frame #5 {
                    # "update cycle value"
                    # "LAB03-2"
                    n260 = local read "DISP LAB03-2"() -> (w325:T4)
                    n261 = Unbundle(w325) -> ("CYCLE"=w326:dbl)  [unwired: 2 out]
                    n262 = case shown="False" w330 {
                      tunnel: [w331 w333] -> w324
                      tunnel: w326 -> [w331 w332]
                      frame False {
                      }
                      frame True {
                        n263 = Increment(x=w332) -> (x+1=w333:dbl)
                      }
                    }
                    n264 = Multiply(x=w324, y=w327) -> (x*y=w328:dbl)
                    n265 = Divide(x=w328, y=60.0) -> (x/y=w323:dbl)
                    n266 = Bundle(cluster=w325, "CYCLE"=w324, "MINS"=w323) -> (w322:T4)  [unwired: 1 in]
                    n267 = local write "DISP LAB03-2"(w322) -> ()
                  }
                  frame #6 {
                    # "update cycle value"
                    # "LAB04-1"
                    n268 = local read "DISP LAB04-1"() -> (w337:T4)
                    n269 = Unbundle(w337) -> ("CYCLE"=w338:dbl)  [unwired: 2 out]
                    n270 = case shown="True" w342 {
                      tunnel: [w343 w345] -> w335
                      tunnel: w338 -> [w343 w344]
                      frame False {
                      }
                      frame True {
                        n271 = Increment(x=w344) -> (x+1=w345:dbl)
                      }
                    }
                    n272 = Multiply(x=w335, y=w339) -> (x*y=w340:dbl)
                    n273 = Divide(x=w340, y=60.0) -> (x/y=w334:dbl)
                    n274 = Bundle(cluster=w337, "CYCLE"=w335, "MINS"=w334) -> (w336:T4)  [unwired: 1 in]
                    n275 = local write "DISP LAB04-1"(w336) -> ()
                  }
                  frame #7 {
                    # "update cycle value"
                    # "LAB04-2"
                    n276 = local read "DISP LAB04-2"() -> (w349:T4)
                    n277 = Unbundle(w349) -> ("CYCLE"=w350:dbl)  [unwired: 2 out]
                    n278 = case shown="True" w354 {
                      tunnel: [w355 w357] -> w347
                      tunnel: w350 -> [w355 w356]
                      frame False {
                      }
                      frame True {
                        n279 = Increment(x=w356) -> (x+1=w357:dbl)
                      }
                    }
                    n280 = Multiply(x=w347, y=w351) -> (x*y=w353:dbl)
                    n281 = Divide(x=w353, y=60.0) -> (x/y=w346:dbl)
                    n282 = Bundle(cluster=w349, "CYCLE"=w347, "MINS"=w346) -> (w348:T4)  [unwired: 1 in]
                    n283 = local write "DISP LAB04-2"(w348) -> ()
                  }
                  frame #8 {
                    # "update cycle value"
                    # "LAB05-1"
                    n284 = local read "DISP LAB05-1"() -> (w361:T4)
                    n285 = Unbundle(w361) -> ("CYCLE"=w362:dbl)  [unwired: 2 out]
                    n286 = case shown="True" w366 {
                      tunnel: [w367 w369] -> w359
                      tunnel: w362 -> [w367 w368]
                      frame False {
                      }
                      frame True {
                        n287 = Increment(x=w368) -> (x+1=w369:dbl)
                      }
                    }
                    n288 = Multiply(x=w359, y=w363) -> (x*y=w364:dbl)
                    n289 = Divide(x=w364, y=60.0) -> (x/y=w358:dbl)
                    n290 = Bundle(cluster=w361, "CYCLE"=w359, "MINS"=w358) -> (w360:T4)  [unwired: 1 in]
                    n291 = local write "DISP LAB05-1"(w360) -> ()
                  }
                  frame #9 {
                    # "update cycle value"
                    # "LAB05-2"
                    n292 = local read "DISP LAB05-2"() -> (w374:T4)
                    n293 = Unbundle(w374) -> ("CYCLE"=w373:dbl)  [unwired: 2 out]
                    n294 = case shown="True" w378 {
                      tunnel: [w379 w381] -> w372
                      tunnel: w373 -> [w379 w380]
                      frame False {
                      }
                      frame True {
                        n295 = Increment(x=w380) -> (x+1=w381:dbl)
                      }
                    }
                    n296 = Multiply(x=w372, y=w375) -> (x*y=w376:dbl)
                    n297 = Divide(x=w376, y=60.0) -> (x/y=w371:dbl)
                    n298 = Bundle(cluster=w374, "CYCLE"=w372, "MINS"=w371) -> (w370:T4)  [unwired: 1 in]
                    n299 = local write "DISP LAB05-2"(w370) -> ()
                  }
                }
                n300 = local write "jig cycle"(0) -> ()
              }
            }
          }
          frame #3 {
            # "START & STOP test RUN switch change, start test if true and stop test if false"
            n301 = Get Date/Time In Seconds() -> (seconds since 1Jan1904=w389:timestamp)
            n302 = local read "C drive data root dir"() -> (w382:path)
            n303 = Format Date/Time String(time format string (%c)="%b\\%a%d", seconds (now)=w389) -> (date/time string=w413:string)  [unwired: 1 in]
            n304 = Format Date/Time String(time format string (%c)="%H%M", seconds (now)=w389) -> (date/time string=w411:string)  [unwired: 1 in]
            n305 = Format Date/Time String(time format string (%c)="LabPanel%Y", seconds (now)=w389) -> (date/time string=w388:string)  [unwired: 1 in]
            n306 = Path To String(path=w382) -> (string=w385:string)
            n307 = global write "Global 1.vi" "C drive root path"(w382) -> ()
            n308 = Concatenate Strings(w385, "\\") -> (w383:string)
            n309 = event shown="[2] \"RUN LAB01-2\": Value Change" {
              selector: _ -> [_ _ _ _ _ _ _ _ _ _ _]
              dyn-events: _ -> [_ _ _ _ _ _ _ _ _ _ _]
              timeout: 10 -> [_ _ _ _ _ _ _ _ _ _ _]
              tunnel: w383 -> [_ w421 w513 w605 w697 w789 w881 w973 w1065 w1157 w1249]
              tunnel: w413 -> [_ w420 w512 w604 w696 w788 w880 w972 w1064 w1156 w1248]
              tunnel: w411 -> [_ w418 w511 w603 w695 w787 w879 w971 w1063 w1155 w1247]
              tunnel: w409 -> [_ w419 _ _ _ _ _ _ _ _ _]
              tunnel: w410 -> [_ _ _ _ _ _ _ _ _ _ _]
              tunnel: w408 -> [_ _ _ _ _ _ _ _ _ _ _]
              tunnel: w407 -> [_ _ w510 _ _ _ _ _ _ _ _]
              tunnel: w406 -> [_ _ _ _ _ _ _ _ _ _ _]
              tunnel: w405 -> [_ _ _ w602 _ _ _ _ _ _ _]
              tunnel: w404 -> [_ _ _ _ _ _ _ _ _ _ _]
              tunnel: w403 -> [_ _ _ _ w694 _ _ _ _ _ _]
              tunnel: w402 -> [_ _ _ _ _ _ _ _ _ _ _]
              tunnel: w401 -> [_ _ _ _ _ w786 _ _ _ _ _]
              tunnel: w400 -> [_ _ _ _ _ _ _ _ _ _ _]
              tunnel: w399 -> [_ _ _ _ _ _ w878 _ _ _ _]
              tunnel: w398 -> [_ _ _ _ _ _ _ _ _ _ _]
              tunnel: w397 -> [_ _ _ _ _ _ _ w970 _ _ _]
              tunnel: w396 -> [_ _ _ _ _ _ _ _ _ _ _]
              tunnel: w395 -> [_ _ _ _ _ _ _ _ w1062 _ _]
              tunnel: w394 -> [_ _ _ _ _ _ _ _ _ _ _]
              tunnel: w393 -> [_ _ _ _ _ _ _ _ _ w1154 _]
              tunnel: w392 -> [_ _ _ _ _ _ _ _ _ _ _]
              tunnel: w391 -> [_ _ _ _ _ _ _ _ _ _ w1246]
              tunnel: w388 -> [_ w417 w509 w601 w693 w785 w877 w969 w1061 w1153 w1245]
              tunnel: [_ w416 w508 w600 w692 w784 w876 w968 w1060 w1152 w1244] -> w386
              event Timeout {
                n310 = event-data() -> ()  [unwired: 1 in, 3 out]
              }
              event "RUN LAB01-1": Value Change {
                n311 = event-data() -> ("NewVal"=w415:bool)  [unwired: 1 in, 5 out]
                n312 = local write "run lab01-1"(w415) -> ()
                n313 = case shown="True" w415 {
                  tunnel: w421 -> [_ w454]
                  tunnel: w420 -> [_ w453]
                  tunnel: w419 -> [w423 w452]
                  tunnel: w418 -> [_ w451]
                  tunnel: w417 -> [_ w450]
                  tunnel: [w422 w449] -> w416
                  frame False {
                    # "stop test"
                    n314 = stacked-sequence {
                      tunnel: w423 -> [_ w435 _ _]
                      tunnel: [_ w427 _ _] -> w422
                      frame #0 {
                        n315 = local read "DISP LAB01-1"() -> (w426:T4)
                        n316 = Bundle(cluster=w426, "STATUS"="STOP") -> (w424:T4)  [unwired: 2 in]
                        n317 = local write "DISP LAB01-1"(w424) -> ()
                      }
                      frame #1 {
                        n318 = local read "DISP LAB01-1"() -> (w434:T4)
                        n319 = Unbundle(w434) -> ("CYCLE"=w432:dbl, "MINS"=w433:dbl)  [unwired: 1 out]
                        n320 = case shown="\"CYCLE TEST\"" w435 {
                          tunnel: w433 -> [_ _ w442]
                          tunnel: w432 -> [w440 w441 _]
                          tunnel: [w440 w441 w442] -> w431
                          frame "CHART TEST", Default {
                          }
                          frame "CYCLE TEST" {
                          }
                          frame "T-RISE TEST" {
                          }
                        }
                        n321 = local read "TDMS LAB01-1"() -> (w439:refnum<k34>)
                        n322 = Build Array("STOPPED") -> (w436:string[])
                        n323 = Build Array(w431) -> (w430:dbl[])
                        n324 = TDMS Write(0:w439, 5:"TEST RESULT", 7:w436, 9:w430) -> (4:w428:refnum<k34>, 15:w429:errorcluster)  [unwired: 2 in, 2 out]
                        n325 = TDMS Close(8:w429, 11:w428) -> (0:w427:errorcluster)  [unwired: 1 out]
                      }
                      frame #2 {
                        n326 = stacked-sequence {
                          tunnel: "LAB01-1" -> [w445 w447]
                          frame #0 {
                            n327 = call "sub vi - defrag tdms v1.vi"("panel id"=w445) -> ("error out"=w444:errorcluster)  [unwired: 10 in]
                            n328 = local write "data file error"(w444) -> ()
                          }
                          frame #1 {
                            n329 = call "Save data file to network drive v1.vi"("panel id"=w447) -> ("network file save error"=w446:errorcluster)  [unwired: 9 in, 1 out]
                            n330 = local write "RESULT LAB01-1"(FALSE) -> ()
                            n331 = local write "data file error"(w446) -> ()
                          }
                        }
                      }
                      frame #3 {
                      }
                    }
                  }
                  frame True {
                    # "start new test and create test file"
                    n332 = stacked-sequence {
                      seq-local: [w455 _ _ _ _] -> [_ w476 _ _ _]
                      tunnel: w454 -> [w460 _ _ _ _]
                      tunnel: w453 -> [w456 _ _ _ _]
                      tunnel: w452 -> [w470 _ _ _ _]
                      tunnel: w451 -> [w463 _ _ _ _]
                      tunnel: w450 -> [w458 _ _ _ _]
                      tunnel: [_ w477 _ _ _] -> w449
                      frame #0 {
                        w457 = "\\"
                        n333 = case shown="\"CHART TEST\", Default" w470 {
                          tunnel: ["L01-1-CHART TEST-" "L01-1-CYCLE TEST-" "L01-1-T-RISE TEST-"] -> w466
                          frame "CHART TEST", Default {
                          }
                          frame "CYCLE TEST" {
                          }
                          frame "T-RISE TEST" {
                          }
                        }
                        n334 = local read "SET LAB01-1"() -> (w465:T5)
                        n335 = Unbundle(w465) -> ("DESCRIPTION"=w464:string)  [unwired: 4 out]
                        n336 = Concatenate Strings(w460, "\\", w458, w457, w456, w457) -> (w467:string)
                        n337 = String To Path(string=w467) -> (path=w469:path)
                        n338 = Concatenate Strings(w467, w466, w464, "-", w463, ".tdms") -> (w455:string)
                        n339 = Create Folder(path (use dialog)=w469) -> (error out=w468:errorcluster)  [unwired: 2 in, 2 out]
                        n340 = call <vilib>:"Clear Errors.vi"("error in (no error)"=w468) -> ()  [unwired: 6 in, 1 out]
                        n341 = global write "Global 1.vi" "LAB01-1 FILE"(w455) -> ()
                      }
                      frame #1 {
                        n342 = String To Path(string=w476) -> (path=w474:path)
                        n343 = TDMS Open(5:FALSE, 6:FALSE, 10:T17."create or replace" ("operation (0:open)"), 11:w474) -> (0:w477:errorcluster, 3:→"TDMS LAB01-1":refnum<k34>)  [unwired: 3 in]
                      }
                      frame #2 {
                        n344 = local read "TDMS LAB01-1"() -> (w497:refnum<k34>)
                        n345 = local read "SET LAB01-1"() -> (w486:T5)
                        n346 = Build Array("Testers Name", "Description", "Set Test Cycles", "T-Rise minutes", "T-Rise Deg C") -> (w487:string[])
                        n347 = Unbundle(w486) -> ("NAME"=w485:string, "DESCRIPTION"=w484:string, "CYCLES"=w483:dbl, "T-RISE mins"=w482:dbl, "T-RISE deg C"=w481:dbl)
                        n348 = Number To Decimal String(number=w483) -> (decimal integer string=w496:string)  [unwired: 1 in]
                        n349 = Number To Decimal String(number=w482) -> (decimal integer string=w495:string)  [unwired: 1 in]
                        n350 = Number To Decimal String(number=w481) -> (decimal integer string=w494:string)  [unwired: 1 in]
                        n351 = Build Array(w485, w484, w496, w495, w494) -> (w493:string[])
                        n352 = TDMS Set Properties(5:w493, 7:w487, 11:w497) -> ()  [unwired: 3 in, 4 out]
                      }
                      frame #3 {
                        w498 = 0.0
                        n353 = local read "DISP LAB01-1"() -> (w501:T4)
                        n354 = Bundle(cluster=w501, "CYCLE"=w498, "MINS"=w498, "STATUS"="RUN") -> (w500:T4)
                        n355 = local write "DISP LAB01-1"(w500) -> ()
                      }
                      frame #4 {
                        n356 = local read "SIG LAB01-1"() -> (w504:T2)
                        n357 = local read "TEMP START LAB01-1"() -> (w506:cluster{"TL":dbl, "TN":dbl})
                        n358 = Unbundle(w504) -> ("Tmp Live"=w503:dbl, "Tmp Neut"=w502:dbl)  [unwired: 3 out]
                        n359 = Bundle(cluster=w506, "TL"=w503, "TN"=w502) -> (w505:cluster{"TL":dbl, "TN":dbl})
                        n360 = local write "TEMP START LAB01-1"(w505) -> ()
                      }
                    }
                  }
                }
              }
              event "RUN LAB01-2": Value Change {
                n361 = event-data() -> ("NewVal"=w507:bool)  [unwired: 1 in, 5 out]
                n362 = local write "run lab01-2"(w507) -> ()
                n363 = case shown="True" w507 {
                  tunnel: w513 -> [_ w546]
                  tunnel: w512 -> [_ w545]
                  tunnel: w510 -> [w515 w544]
                  tunnel: w511 -> [_ w543]
                  tunnel: w509 -> [_ w542]
                  tunnel: [w514 w541] -> w508
                  frame False {
                    # "stop test"
                    n364 = stacked-sequence {
                      tunnel: w515 -> [w524 _]
                      tunnel: [w516 _] -> w514
                      frame #0 {
                        n365 = local read "DISP LAB01-2"() -> (w523:T4)
                        n366 = Unbundle(w523) -> ("CYCLE"=w521:dbl, "MINS"=w522:dbl)  [unwired: 1 out]
                        n367 = case shown="\"CHART TEST\", Default" w524 {
                          tunnel: w522 -> [_ _ w531]
                          tunnel: w521 -> [w529 w530 _]
                          tunnel: [w529 w530 w531] -> w520
                          frame "CHART TEST", Default {
                          }
                          frame "CYCLE TEST" {
                          }
                          frame "T-RISE TEST" {
                          }
                        }
                        n368 = local read "TDMS LAB01-2"() -> (w528:refnum<k34>)
                        n369 = Build Array("STOPPED") -> (w525:string[])
                        n370 = Build Array(w520) -> (w519:dbl[])
                        n371 = TDMS Write(0:w528, 5:"TEST RESULT", 7:w525, 9:w519) -> (4:w517:refnum<k34>, 15:w518:errorcluster)  [unwired: 2 in, 2 out]
                        n372 = TDMS Close(8:w518, 11:w517) -> (0:w516:errorcluster)  [unwired: 1 out]
                      }
                      frame #1 {
                        n373 = local read "DISP LAB01-2"() -> (w535:T4)
                        n374 = stacked-sequence {
                          tunnel: "LAB01-2" -> [w537 w539]
                          frame #0 {
                            n375 = call "sub vi - defrag tdms v1.vi"("panel id"=w537) -> ("error out"=w536:errorcluster)  [unwired: 10 in]
                            n376 = local write "data file error"(w536) -> ()
                          }
                          frame #1 {
                            n377 = call "Save data file to network drive v1.vi"("panel id"=w539) -> ("network file save error"=w538:errorcluster)  [unwired: 9 in, 1 out]
                            n378 = local write "RESULT LAB01-2"(FALSE) -> ()
                            n379 = local write "data file error"(w538) -> ()
                          }
                        }
                        n380 = Bundle(cluster=w535, "STATUS"="STOP") -> (w533:T4)  [unwired: 2 in]
                        n381 = local write "DISP LAB01-2"(w533) -> ()
                      }
                    }
                  }
                  frame True {
                    # "start new test and create test file"
                    n382 = stacked-sequence {
                      seq-local: [w547 _ _ _ _] -> [_ w572 _ _ _]
                      tunnel: w546 -> [w552 _ _ _ _]
                      tunnel: w545 -> [w549 _ _ _ _]
                      tunnel: w544 -> [w562 _ _ _ _]
                      tunnel: w543 -> [w555 _ _ _ _]
                      tunnel: w542 -> [w550 _ _ _ _]
                      tunnel: [_ w566 _ _ _] -> w541
                      frame #0 {
                        w548 = "\\"
                        n383 = local read "SET LAB01-2"() -> (w557:T5)
                        n384 = case shown="\"CYCLE TEST\"" w562 {
                          tunnel: ["L01-2-CHART TEST-" "L01-2-CYCLE TEST-" "L01-2-T-RISE TEST-"] -> w558
                          frame "CHART TEST", Default {
                          }
                          frame "CYCLE TEST" {
                          }
                          frame "T-RISE TEST" {
                          }
                        }
                        n385 = Unbundle(w557) -> ("DESCRIPTION"=w556:string)  [unwired: 4 out]
                        n386 = Concatenate Strings(w552, "\\", w550, w548, w549, w548) -> (w559:string)
                        n387 = String To Path(string=w559) -> (path=w561:path)
                        n388 = Concatenate Strings(w559, w558, w556, "-", w555, ".tdms") -> (w547:string)
                        n389 = Create Folder(path (use dialog)=w561) -> (error out=w560:errorcluster)  [unwired: 2 in, 2 out]
                        n390 = global write "Global 1.vi" "LAB01-2 FILE"(w547) -> ()
                        n391 = call <vilib>:"Clear Errors.vi"("error in (no error)"=w560) -> ()  [unwired: 6 in, 1 out]
                      }
                      frame #1 {
                        n392 = String To Path(string=w572) -> (path=w567:path)
                        n393 = TDMS Open(5:FALSE, 6:FALSE, 10:T17."create or replace" ("operation (0:open)"), 11:w567) -> (0:w566:errorcluster, 3:→"TDMS LAB01-2":refnum<k34>)  [unwired: 3 in]
                      }
                      frame #2 {
                        n394 = local read "SET LAB01-2"() -> (w578:T5)
                        n395 = local read "TDMS LAB01-2"() -> (w589:refnum<k34>)
                        n396 = Build Array("Testers Name", "Description", "Set Test Cycles", "T-Rise minutes", "T-Rise Deg C") -> (w579:string[])
                        n397 = Unbundle(w578) -> ("NAME"=w577:string, "DESCRIPTION"=w576:string, "CYCLES"=w575:dbl, "T-RISE mins"=w574:dbl, "T-RISE deg C"=w573:dbl)
                        n398 = Number To Decimal String(number=w575) -> (decimal integer string=w588:string)  [unwired: 1 in]
                        n399 = Number To Decimal String(number=w574) -> (decimal integer string=w587:string)  [unwired: 1 in]
                        n400 = Number To Decimal String(number=w573) -> (decimal integer string=w586:string)  [unwired: 1 in]
                        n401 = Build Array(w577, w576, w588, w587, w586) -> (w585:string[])
                        n402 = TDMS Set Properties(5:w585, 7:w579, 11:w589) -> ()  [unwired: 3 in, 4 out]
                      }
                      frame #3 {
                        w591 = 0.0
                        n403 = local read "DISP LAB01-2"() -> (w593:T4)
                        n404 = Bundle(cluster=w593, "CYCLE"=w591, "MINS"=w591, "STATUS"="RUN") -> (w592:T4)
                        n405 = local write "DISP LAB01-2"(w592) -> ()
                      }
                      frame #4 {
                        n406 = local read "SIG LAB01-2"() -> (w596:T2)
                        n407 = local read "TEMP START LAB01-2"() -> (w598:cluster{"TL":dbl, "TN":dbl})
                        n408 = Unbundle(w596) -> ("Tmp Live"=w595:dbl, "Tmp Neut"=w594:dbl)  [unwired: 3 out]
                        n409 = Bundle(cluster=w598, "TL"=w595, "TN"=w594) -> (w597:cluster{"TL":dbl, "TN":dbl})
                        n410 = local write "TEMP START LAB01-2"(w597) -> ()
                      }
                    }
                  }
                }
              }
              event "RUN LAB02-1": Value Change {
                n411 = event-data() -> ("NewVal"=w599:bool)  [unwired: 1 in, 5 out]
                n412 = local write "run lab02-1"(w599) -> ()
                n413 = case shown="True" w599 {
                  tunnel: w605 -> [_ w638]
                  tunnel: w604 -> [_ w637]
                  tunnel: w602 -> [w607 w636]
                  tunnel: w603 -> [_ w635]
                  tunnel: w601 -> [_ w634]
                  tunnel: [w606 w633] -> w600
                  frame False {
                    # "stop test"
                    n414 = stacked-sequence {
                      tunnel: w607 -> [w616 _]
                      tunnel: [w608 _] -> w606
                      frame #0 {
                        n415 = local read "DISP LAB02-1"() -> (w615:T4)
                        n416 = Unbundle(w615) -> ("CYCLE"=w613:dbl, "MINS"=w614:dbl)  [unwired: 1 out]
                        n417 = case shown="\"CYCLE TEST\"" w616 {
                          tunnel: w614 -> [_ _ w623]
                          tunnel: w613 -> [w621 w622 _]
                          tunnel: [w621 w622 w623] -> w612
                          frame "CHART TEST", Default {
                          }
                          frame "CYCLE TEST" {
                          }
                          frame "T-RISE TEST" {
                          }
                        }
                        n418 = local read "TDMS LAB02-1"() -> (w620:refnum<k34>)
                        n419 = Build Array("STOPPED") -> (w617:string[])
                        n420 = Build Array(w612) -> (w611:dbl[])
                        n421 = TDMS Write(0:w620, 5:"TEST RESULT", 7:w617, 9:w611) -> (4:w609:refnum<k34>, 15:w610:errorcluster)  [unwired: 2 in, 2 out]
                        n422 = TDMS Close(8:w610, 11:w609) -> (0:w608:errorcluster)  [unwired: 1 out]
                      }
                      frame #1 {
                        n423 = local read "DISP LAB02-1"() -> (w627:T4)
                        n424 = stacked-sequence {
                          tunnel: "LAB02-1" -> [w629 w631]
                          frame #0 {
                            n425 = call "sub vi - defrag tdms v1.vi"("panel id"=w629) -> ("error out"=w628:errorcluster)  [unwired: 10 in]
                            n426 = local write "data file error"(w628) -> ()
                          }
                          frame #1 {
                            n427 = local write "RESULT LAB02-1"(FALSE) -> ()
                            n428 = call "Save data file to network drive v1.vi"("panel id"=w631) -> ("network file save error"=w630:errorcluster)  [unwired: 9 in, 1 out]
                            n429 = local write "data file error"(w630) -> ()
                          }
                        }
                        n430 = Bundle(cluster=w627, "STATUS"="STOP") -> (w625:T4)  [unwired: 2 in]
                        n431 = local write "DISP LAB02-1"(w625) -> ()
                      }
                    }
                  }
                  frame True {
                    # "start new test and create test file"
                    n432 = stacked-sequence {
                      seq-local: [w639 _ _ _ _] -> [_ w664 _ _ _]
                      tunnel: w638 -> [w644 _ _ _ _]
                      tunnel: w637 -> [w641 _ _ _ _]
                      tunnel: w636 -> [w654 _ _ _ _]
                      tunnel: w635 -> [w647 _ _ _ _]
                      tunnel: w634 -> [w642 _ _ _ _]
                      tunnel: [_ w658 _ _ _] -> w633
                      frame #0 {
                        w640 = "\\"
                        n433 = local read "SET LAB02-1"() -> (w649:T5)
                        n434 = case shown="\"CYCLE TEST\"" w654 {
                          tunnel: ["L02-1-CHART TEST-" "L02-1-CYCLE TEST-" "L02-1-T-RISE TEST-"] -> w650
                          frame "CHART TEST", Default {
                          }
                          frame "CYCLE TEST" {
                          }
                          frame "T-RISE TEST" {
                          }
                        }
                        n435 = Unbundle(w649) -> ("DESCRIPTION"=w648:string)  [unwired: 4 out]
                        n436 = Concatenate Strings(w644, "\\", w642, w640, w641, w640) -> (w651:string)
                        n437 = String To Path(string=w651) -> (path=w653:path)
                        n438 = Concatenate Strings(w651, w650, w648, "-", w647, ".tdms") -> (w639:string)
                        n439 = Create Folder(path (use dialog)=w653) -> (error out=w652:errorcluster)  [unwired: 2 in, 2 out]
                        n440 = global write "Global 1.vi" "LAB02-1 FILE"(w639) -> ()
                        n441 = call <vilib>:"Clear Errors.vi"("error in (no error)"=w652) -> ()  [unwired: 6 in, 1 out]
                      }
                      frame #1 {
                        n442 = String To Path(string=w664) -> (path=w659:path)
                        n443 = TDMS Open(5:FALSE, 6:FALSE, 10:T17."create or replace" ("operation (0:open)"), 11:w659) -> (0:w658:errorcluster, 3:→"TDMS LAB02-1":refnum<k34>)  [unwired: 3 in]
                      }
                      frame #2 {
                        n444 = local read "SET LAB02-1"() -> (w670:T5)
                        n445 = local read "TDMS LAB02-1"() -> (w681:refnum<k34>)
                        n446 = Build Array("Testers Name", "Description", "Set Test Cycles", "T-Rise minutes", "T-Rise Deg C") -> (w671:string[])
                        n447 = Unbundle(w670) -> ("NAME"=w669:string, "DESCRIPTION"=w668:string, "CYCLES"=w667:dbl, "T-RISE mins"=w666:dbl, "T-RISE deg C"=w665:dbl)
                        n448 = Number To Decimal String(number=w667) -> (decimal integer string=w680:string)  [unwired: 1 in]
                        n449 = Number To Decimal String(number=w666) -> (decimal integer string=w679:string)  [unwired: 1 in]
                        n450 = Number To Decimal String(number=w665) -> (decimal integer string=w678:string)  [unwired: 1 in]
                        n451 = Build Array(w669, w668, w680, w679, w678) -> (w677:string[])
                        n452 = TDMS Set Properties(5:w677, 7:w671, 11:w681) -> ()  [unwired: 3 in, 4 out]
                      }
                      frame #3 {
                        w683 = 0.0
                        n453 = local read "DISP LAB02-1"() -> (w685:T4)
                        n454 = Bundle(cluster=w685, "CYCLE"=w683, "MINS"=w683, "STATUS"="RUN") -> (w684:T4)
                        n455 = local write "DISP LAB02-1"(w684) -> ()
                      }
                      frame #4 {
                        n456 = local read "SIG LAB02-1"() -> (w688:T2)
                        n457 = local read "TEMP START LAB02-1"() -> (w690:cluster{"TL":dbl, "TN":dbl})
                        n458 = Unbundle(w688) -> ("Tmp Live"=w687:dbl, "Tmp Neut"=w686:dbl)  [unwired: 3 out]
                        n459 = Bundle(cluster=w690, "TL"=w687, "TN"=w686) -> (w689:cluster{"TL":dbl, "TN":dbl})
                        n460 = local write "TEMP START LAB02-1"(w689) -> ()
                      }
                    }
                  }
                }
              }
              event "RUN LAB02-2": Value Change {
                n461 = event-data() -> ("NewVal"=w691:bool)  [unwired: 1 in, 5 out]
                n462 = local write "run lab02-2"(w691) -> ()
                n463 = case shown="True" w691 {
                  tunnel: w697 -> [_ w730]
                  tunnel: w696 -> [_ w729]
                  tunnel: w694 -> [w699 w728]
                  tunnel: w695 -> [_ w727]
                  tunnel: w693 -> [_ w726]
                  tunnel: [w698 w725] -> w692
                  frame False {
                    # "stop test"
                    n464 = stacked-sequence {
                      tunnel: w699 -> [w708 _]
                      tunnel: [w700 _] -> w698
                      frame #0 {
                        n465 = local read "DISP LAB02-2"() -> (w707:T4)
                        n466 = Unbundle(w707) -> ("CYCLE"=w705:dbl, "MINS"=w706:dbl)  [unwired: 1 out]
                        n467 = case shown="\"CYCLE TEST\"" w708 {
                          tunnel: w706 -> [_ _ w715]
                          tunnel: w705 -> [w713 w714 _]
                          tunnel: [w713 w714 w715] -> w704
                          frame "CHART TEST", Default {
                          }
                          frame "CYCLE TEST" {
                          }
                          frame "T-RISE TEST" {
                          }
                        }
                        n468 = local read "TDMS LAB02-2"() -> (w712:refnum<k34>)
                        n469 = Build Array("STOPPED") -> (w709:string[])
                        n470 = Build Array(w704) -> (w703:dbl[])
                        n471 = TDMS Write(0:w712, 5:"TEST RESULT", 7:w709, 9:w703) -> (4:w701:refnum<k34>, 15:w702:errorcluster)  [unwired: 2 in, 2 out]
                        n472 = TDMS Close(8:w702, 11:w701) -> (0:w700:errorcluster)  [unwired: 1 out]
                      }
                      frame #1 {
                        n473 = local read "DISP LAB02-2"() -> (w719:T4)
                        n474 = stacked-sequence {
                          tunnel: "LAB02-2" -> [w721 w723]
                          frame #0 {
                            n475 = call "sub vi - defrag tdms v1.vi"("panel id"=w721) -> ("error out"=w720:errorcluster)  [unwired: 10 in]
                            n476 = local write "data file error"(w720) -> ()
                          }
                          frame #1 {
                            n477 = call "Save data file to network drive v1.vi"("panel id"=w723) -> ("network file save error"=w722:errorcluster)  [unwired: 9 in, 1 out]
                            n478 = local write "RESULT LAB02-2"(FALSE) -> ()
                            n479 = local write "data file error"(w722) -> ()
                          }
                        }
                        n480 = Bundle(cluster=w719, "STATUS"="STOP") -> (w717:T4)  [unwired: 2 in]
                        n481 = local write "DISP LAB02-2"(w717) -> ()
                      }
                    }
                  }
                  frame True {
                    # "start new test and create test file"
                    n482 = stacked-sequence {
                      seq-local: [w731 _ _ _ _] -> [_ w756 _ _ _]
                      tunnel: w730 -> [w736 _ _ _ _]
                      tunnel: w729 -> [w733 _ _ _ _]
                      tunnel: w728 -> [w746 _ _ _ _]
                      tunnel: w727 -> [w739 _ _ _ _]
                      tunnel: w726 -> [w734 _ _ _ _]
                      tunnel: [_ w750 _ _ _] -> w725
                      frame #0 {
                        w732 = "\\"
                        n483 = local read "SET LAB02-2"() -> (w741:T5)
                        n484 = case shown="\"CYCLE TEST\"" w746 {
                          tunnel: ["L02-2-CHART TEST-" "L02-2-CYCLE TEST-" "L02-2-T-RISE TEST-"] -> w742
                          frame "CHART TEST", Default {
                          }
                          frame "CYCLE TEST" {
                          }
                          frame "T-RISE TEST" {
                          }
                        }
                        n485 = Unbundle(w741) -> ("DESCRIPTION"=w740:string)  [unwired: 4 out]
                        n486 = Concatenate Strings(w736, "\\", w734, w732, w733, w732) -> (w743:string)
                        n487 = String To Path(string=w743) -> (path=w745:path)
                        n488 = Concatenate Strings(w743, w742, w740, "-", w739, ".tdms") -> (w731:string)
                        n489 = Create Folder(path (use dialog)=w745) -> (error out=w744:errorcluster)  [unwired: 2 in, 2 out]
                        n490 = global write "Global 1.vi" "LAB02-2 FILE"(w731) -> ()
                        n491 = call <vilib>:"Clear Errors.vi"("error in (no error)"=w744) -> ()  [unwired: 6 in, 1 out]
                      }
                      frame #1 {
                        n492 = String To Path(string=w756) -> (path=w751:path)
                        n493 = TDMS Open(5:FALSE, 6:FALSE, 10:T17."create or replace" ("operation (0:open)"), 11:w751) -> (0:w750:errorcluster, 3:→"TDMS LAB02-2":refnum<k34>)  [unwired: 3 in]
                      }
                      frame #2 {
                        n494 = local read "SET LAB02-2"() -> (w762:T5)
                        n495 = local read "TDMS LAB02-2"() -> (w773:refnum<k34>)
                        n496 = Build Array("Testers Name", "Description", "Set Test Cycles", "T-Rise minutes", "T-Rise Deg C") -> (w763:string[])
                        n497 = Unbundle(w762) -> ("NAME"=w761:string, "DESCRIPTION"=w760:string, "CYCLES"=w759:dbl, "T-RISE mins"=w758:dbl, "T-RISE deg C"=w757:dbl)
                        n498 = Number To Decimal String(number=w759) -> (decimal integer string=w772:string)  [unwired: 1 in]
                        n499 = Number To Decimal String(number=w758) -> (decimal integer string=w771:string)  [unwired: 1 in]
                        n500 = Number To Decimal String(number=w757) -> (decimal integer string=w770:string)  [unwired: 1 in]
                        n501 = Build Array(w761, w760, w772, w771, w770) -> (w769:string[])
                        n502 = TDMS Set Properties(5:w769, 7:w763, 11:w773) -> ()  [unwired: 3 in, 4 out]
                      }
                      frame #3 {
                        w775 = 0.0
                        n503 = local read "DISP LAB02-2"() -> (w777:T4)
                        n504 = Bundle(cluster=w777, "CYCLE"=w775, "MINS"=w775, "STATUS"="RUN") -> (w776:T4)
                        n505 = local write "DISP LAB02-2"(w776) -> ()
                      }
                      frame #4 {
                        n506 = local read "SIG LAB02-2"() -> (w780:T2)
                        n507 = local read "TEMP START LAB02-2"() -> (w782:cluster{"TL":dbl, "TN":dbl})
                        n508 = Unbundle(w780) -> ("Tmp Live"=w779:dbl, "Tmp Neut"=w778:dbl)  [unwired: 3 out]
                        n509 = Bundle(cluster=w782, "TL"=w779, "TN"=w778) -> (w781:cluster{"TL":dbl, "TN":dbl})
                        n510 = local write "TEMP START LAB02-2"(w781) -> ()
                      }
                    }
                  }
                }
              }
              event "RUN LAB03-1": Value Change {
                n511 = event-data() -> ("NewVal"=w783:bool)  [unwired: 1 in, 5 out]
                n512 = local write "run lab03-1"(w783) -> ()
                n513 = case shown="True" w783 {
                  tunnel: w789 -> [_ w822]
                  tunnel: w788 -> [_ w821]
                  tunnel: w786 -> [w791 w820]
                  tunnel: w787 -> [_ w819]
                  tunnel: w785 -> [_ w818]
                  tunnel: [w790 w817] -> w784
                  frame False {
                    # "stop test"
                    n514 = stacked-sequence {
                      tunnel: w791 -> [w800 _]
                      tunnel: [w792 _] -> w790
                      frame #0 {
                        n515 = local read "DISP LAB03-1"() -> (w799:T4)
                        n516 = Unbundle(w799) -> ("CYCLE"=w797:dbl, "MINS"=w798:dbl)  [unwired: 1 out]
                        n517 = case shown="\"CYCLE TEST\"" w800 {
                          tunnel: w798 -> [_ _ w807]
                          tunnel: w797 -> [w805 w806 _]
                          tunnel: [w805 w806 w807] -> w796
                          frame "CHART TEST", Default {
                          }
                          frame "CYCLE TEST" {
                          }
                          frame "T-RISE TEST" {
                          }
                        }
                        n518 = local read "TDMS LAB03-1"() -> (w804:refnum<k34>)
                        n519 = Build Array("STOPPED") -> (w801:string[])
                        n520 = Build Array(w796) -> (w795:dbl[])
                        n521 = TDMS Write(0:w804, 5:"TEST RESULT", 7:w801, 9:w795) -> (4:w793:refnum<k34>, 15:w794:errorcluster)  [unwired: 2 in, 2 out]
                        n522 = TDMS Close(8:w794, 11:w793) -> (0:w792:errorcluster)  [unwired: 1 out]
                      }
                      frame #1 {
                        n523 = local read "DISP LAB03-1"() -> (w811:T4)
                        n524 = stacked-sequence {
                          tunnel: "LAB03-1" -> [w813 w815]
                          frame #0 {
                            n525 = call "sub vi - defrag tdms v1.vi"("panel id"=w813) -> ("error out"=w812:errorcluster)  [unwired: 10 in]
                            n526 = local write "data file error"(w812) -> ()
                          }
                          frame #1 {
                            n527 = call "Save data file to network drive v1.vi"("panel id"=w815) -> ("network file save error"=w814:errorcluster)  [unwired: 9 in, 1 out]
                            n528 = local write "RESULT LAB03-1"(FALSE) -> ()
                            n529 = local write "data file error"(w814) -> ()
                          }
                        }
                        n530 = Bundle(cluster=w811, "STATUS"="STOP") -> (w809:T4)  [unwired: 2 in]
                        n531 = local write "DISP LAB03-1"(w809) -> ()
                      }
                    }
                  }
                  frame True {
                    # "start new test and create test file"
                    n532 = stacked-sequence {
                      seq-local: [w823 _ _ _ _] -> [_ w848 _ _ _]
                      tunnel: w822 -> [w828 _ _ _ _]
                      tunnel: w821 -> [w825 _ _ _ _]
                      tunnel: w820 -> [w838 _ _ _ _]
                      tunnel: w819 -> [w831 _ _ _ _]
                      tunnel: w818 -> [w826 _ _ _ _]
                      tunnel: [_ w842 _ _ _] -> w817
                      frame #0 {
                        w824 = "\\"
                        n533 = local read "SET LAB03-1"() -> (w833:T5)
                        n534 = case shown="\"T-RISE TEST\"" w838 {
                          tunnel: ["L03-1-CHART TEST-" "L03-1-CYCLE TEST-" "L03-1-T-RISE TEST-"] -> w834
                          frame "CHART TEST", Default {
                          }
                          frame "CYCLE TEST" {
                          }
                          frame "T-RISE TEST" {
                          }
                        }
                        n535 = Unbundle(w833) -> ("DESCRIPTION"=w832:string)  [unwired: 4 out]
                        n536 = Concatenate Strings(w828, "\\", w826, w824, w825, w824) -> (w835:string)
                        n537 = String To Path(string=w835) -> (path=w837:path)
                        n538 = Concatenate Strings(w835, w834, w832, "-", w831, ".tdms") -> (w823:string)
                        n539 = Create Folder(path (use dialog)=w837) -> (error out=w836:errorcluster)  [unwired: 2 in, 2 out]
                        n540 = global write "Global 1.vi" "LAB03-1 FILE"(w823) -> ()
                        n541 = call <vilib>:"Clear Errors.vi"("error in (no error)"=w836) -> ()  [unwired: 6 in, 1 out]
                      }
                      frame #1 {
                        n542 = String To Path(string=w848) -> (path=w843:path)
                        n543 = TDMS Open(5:FALSE, 6:FALSE, 10:T17."create or replace" ("operation (0:open)"), 11:w843) -> (0:w842:errorcluster, 3:→"TDMS LAB03-1":refnum<k34>)  [unwired: 3 in]
                      }
                      frame #2 {
                        n544 = local read "SET LAB03-1"() -> (w854:T5)
                        n545 = local read "TDMS LAB03-1"() -> (w865:refnum<k34>)
                        n546 = Build Array("Testers Name", "Description", "Set Test Cycles", "T-Rise minutes", "T-Rise Deg C") -> (w855:string[])
                        n547 = Unbundle(w854) -> ("NAME"=w853:string, "DESCRIPTION"=w852:string, "CYCLES"=w851:dbl, "T-RISE mins"=w850:dbl, "T-RISE deg C"=w849:dbl)
                        n548 = Number To Decimal String(number=w851) -> (decimal integer string=w864:string)  [unwired: 1 in]
                        n549 = Number To Decimal String(number=w850) -> (decimal integer string=w863:string)  [unwired: 1 in]
                        n550 = Number To Decimal String(number=w849) -> (decimal integer string=w862:string)  [unwired: 1 in]
                        n551 = Build Array(w853, w852, w864, w863, w862) -> (w861:string[])
                        n552 = TDMS Set Properties(5:w861, 7:w855, 11:w865) -> ()  [unwired: 3 in, 4 out]
                      }
                      frame #3 {
                        w867 = 0.0
                        n553 = local read "DISP LAB03-1"() -> (w869:T4)
                        n554 = Bundle(cluster=w869, "CYCLE"=w867, "MINS"=w867, "STATUS"="RUN") -> (w868:T4)
                        n555 = local write "DISP LAB03-1"(w868) -> ()
                      }
                      frame #4 {
                        n556 = local read "SIG LAB03-1"() -> (w872:T2)
                        n557 = local read "TEMP START LAB03-1"() -> (w874:cluster{"TL":dbl, "TN":dbl})
                        n558 = Unbundle(w872) -> ("Tmp Live"=w871:dbl, "Tmp Neut"=w870:dbl)  [unwired: 3 out]
                        n559 = Bundle(cluster=w874, "TL"=w871, "TN"=w870) -> (w873:cluster{"TL":dbl, "TN":dbl})
                        n560 = local write "TEMP START LAB03-1"(w873) -> ()
                      }
                    }
                  }
                }
              }
              event "RUN LAB03-2": Value Change {
                n561 = event-data() -> ("NewVal"=w875:bool)  [unwired: 1 in, 5 out]
                n562 = local write "run lab03-2"(w875) -> ()
                n563 = case shown="True" w875 {
                  tunnel: w881 -> [_ w914]
                  tunnel: w880 -> [_ w913]
                  tunnel: w878 -> [w883 w912]
                  tunnel: w879 -> [_ w911]
                  tunnel: w877 -> [_ w910]
                  tunnel: [w882 w909] -> w876
                  frame False {
                    # "stop test"
                    n564 = stacked-sequence {
                      tunnel: w883 -> [w892 _]
                      tunnel: [w884 _] -> w882
                      frame #0 {
                        n565 = local read "DISP LAB03-2"() -> (w891:T4)
                        n566 = Unbundle(w891) -> ("CYCLE"=w889:dbl, "MINS"=w890:dbl)  [unwired: 1 out]
                        n567 = case shown="\"CYCLE TEST\"" w892 {
                          tunnel: w890 -> [_ _ w899]
                          tunnel: w889 -> [w897 w898 _]
                          tunnel: [w897 w898 w899] -> w888
                          frame "CHART TEST", Default {
                          }
                          frame "CYCLE TEST" {
                          }
                          frame "T-RISE TEST" {
                          }
                        }
                        n568 = local read "TDMS LAB03-2"() -> (w896:refnum<k34>)
                        n569 = Build Array("STOPPED") -> (w893:string[])
                        n570 = Build Array(w888) -> (w887:dbl[])
                        n571 = TDMS Write(0:w896, 5:"TEST RESULT", 7:w893, 9:w887) -> (4:w885:refnum<k34>, 15:w886:errorcluster)  [unwired: 2 in, 2 out]
                        n572 = TDMS Close(8:w886, 11:w885) -> (0:w884:errorcluster)  [unwired: 1 out]
                      }
                      frame #1 {
                        n573 = local read "DISP LAB03-2"() -> (w903:T4)
                        n574 = stacked-sequence {
                          tunnel: "LAB03-2" -> [w905 w907]
                          frame #0 {
                            n575 = call "sub vi - defrag tdms v1.vi"("panel id"=w905) -> ("error out"=w904:errorcluster)  [unwired: 10 in]
                            n576 = local write "data file error"(w904) -> ()
                          }
                          frame #1 {
                            n577 = call "Save data file to network drive v1.vi"("panel id"=w907) -> ("network file save error"=w906:errorcluster)  [unwired: 9 in, 1 out]
                            n578 = local write "RESULT LAB03-2"(FALSE) -> ()
                            n579 = local write "data file error"(w906) -> ()
                          }
                        }
                        n580 = Bundle(cluster=w903, "STATUS"="STOP") -> (w901:T4)  [unwired: 2 in]
                        n581 = local write "DISP LAB03-2"(w901) -> ()
                      }
                    }
                  }
                  frame True {
                    # "start new test and create test file"
                    n582 = stacked-sequence {
                      seq-local: [w915 _ _ _ _] -> [_ w940 _ _ _]
                      tunnel: w914 -> [w920 _ _ _ _]
                      tunnel: w913 -> [w917 _ _ _ _]
                      tunnel: w912 -> [w930 _ _ _ _]
                      tunnel: w911 -> [w923 _ _ _ _]
                      tunnel: w910 -> [w918 _ _ _ _]
                      tunnel: [_ w934 _ _ _] -> w909
                      frame #0 {
                        w916 = "\\"
                        n583 = local read "SET LAB03-2"() -> (w925:T5)
                        n584 = case shown="\"T-RISE TEST\"" w930 {
                          tunnel: ["L03-2-CHART TEST-" "L03-2-CYCLE TEST-" "L03-2-T-RISE TEST-"] -> w926
                          frame "CHART TEST", Default {
                          }
                          frame "CYCLE TEST" {
                          }
                          frame "T-RISE TEST" {
                          }
                        }
                        n585 = Unbundle(w925) -> ("DESCRIPTION"=w924:string)  [unwired: 4 out]
                        n586 = Concatenate Strings(w920, "\\", w918, w916, w917, w916) -> (w927:string)
                        n587 = String To Path(string=w927) -> (path=w929:path)
                        n588 = Concatenate Strings(w927, w926, w924, "-", w923, ".tdms") -> (w915:string)
                        n589 = Create Folder(path (use dialog)=w929) -> (error out=w928:errorcluster)  [unwired: 2 in, 2 out]
                        n590 = global write "Global 1.vi" "LAB03-2 FILE"(w915) -> ()
                        n591 = call <vilib>:"Clear Errors.vi"("error in (no error)"=w928) -> ()  [unwired: 6 in, 1 out]
                      }
                      frame #1 {
                        n592 = String To Path(string=w940) -> (path=w935:path)
                        n593 = TDMS Open(5:FALSE, 6:FALSE, 10:T17."create or replace" ("operation (0:open)"), 11:w935) -> (0:w934:errorcluster, 3:→"TDMS LAB03-2":refnum<k34>)  [unwired: 3 in]
                      }
                      frame #2 {
                        n594 = local read "SET LAB03-2"() -> (w946:T5)
                        n595 = local read "TDMS LAB03-2"() -> (w957:refnum<k34>)
                        n596 = Build Array("Testers Name", "Description", "Set Test Cycles", "T-Rise minutes", "T-Rise Deg C") -> (w947:string[])
                        n597 = Unbundle(w946) -> ("NAME"=w945:string, "DESCRIPTION"=w944:string, "CYCLES"=w943:dbl, "T-RISE mins"=w942:dbl, "T-RISE deg C"=w941:dbl)
                        n598 = Number To Decimal String(number=w943) -> (decimal integer string=w956:string)  [unwired: 1 in]
                        n599 = Number To Decimal String(number=w942) -> (decimal integer string=w955:string)  [unwired: 1 in]
                        n600 = Number To Decimal String(number=w941) -> (decimal integer string=w954:string)  [unwired: 1 in]
                        n601 = Build Array(w945, w944, w956, w955, w954) -> (w953:string[])
                        n602 = TDMS Set Properties(5:w953, 7:w947, 11:w957) -> ()  [unwired: 3 in, 4 out]
                      }
                      frame #3 {
                        w959 = 0.0
                        n603 = local read "DISP LAB03-2"() -> (w961:T4)
                        n604 = Bundle(cluster=w961, "CYCLE"=w959, "MINS"=w959, "STATUS"="RUN") -> (w960:T4)
                        n605 = local write "DISP LAB03-2"(w960) -> ()
                      }
                      frame #4 {
                        n606 = local read "SIG LAB03-2"() -> (w964:T2)
                        n607 = local read "TEMP START LAB03-2"() -> (w966:cluster{"TL":dbl, "TN":dbl})
                        n608 = Unbundle(w964) -> ("Tmp Live"=w963:dbl, "Tmp Neut"=w962:dbl)  [unwired: 3 out]
                        n609 = Bundle(cluster=w966, "TL"=w963, "TN"=w962) -> (w965:cluster{"TL":dbl, "TN":dbl})
                        n610 = local write "TEMP START LAB03-2"(w965) -> ()
                      }
                    }
                  }
                }
              }
              event "RUN LAB04-1": Value Change {
                n611 = event-data() -> ("NewVal"=w967:bool)  [unwired: 1 in, 5 out]
                n612 = local write "run lab04-1"(w967) -> ()
                n613 = case shown="True" w967 {
                  tunnel: w973 -> [_ w1006]
                  tunnel: w972 -> [_ w1005]
                  tunnel: w970 -> [w975 w1004]
                  tunnel: w971 -> [_ w1003]
                  tunnel: w969 -> [_ w1002]
                  tunnel: [w974 w1001] -> w968
                  frame False {
                    # "stop test"
                    n614 = stacked-sequence {
                      tunnel: w975 -> [w984 _]
                      tunnel: [w976 _] -> w974
                      frame #0 {
                        n615 = local read "DISP LAB04-1"() -> (w983:T4)
                        n616 = Unbundle(w983) -> ("CYCLE"=w981:dbl, "MINS"=w982:dbl)  [unwired: 1 out]
                        n617 = case shown="\"CYCLE TEST\"" w984 {
                          tunnel: w982 -> [_ _ w991]
                          tunnel: w981 -> [w989 w990 _]
                          tunnel: [w989 w990 w991] -> w980
                          frame "CHART TEST", Default {
                          }
                          frame "CYCLE TEST" {
                          }
                          frame "T-RISE TEST" {
                          }
                        }
                        n618 = local read "TDMS LAB04-1"() -> (w988:refnum<k34>)
                        n619 = Build Array("STOPPED") -> (w985:string[])
                        n620 = Build Array(w980) -> (w979:dbl[])
                        n621 = TDMS Write(0:w988, 5:"TEST RESULT", 7:w985, 9:w979) -> (4:w977:refnum<k34>, 15:w978:errorcluster)  [unwired: 2 in, 2 out]
                        n622 = TDMS Close(8:w978, 11:w977) -> (0:w976:errorcluster)  [unwired: 1 out]
                      }
                      frame #1 {
                        n623 = local read "DISP LAB04-1"() -> (w995:T4)
                        n624 = stacked-sequence {
                          tunnel: "LAB04-1" -> [w997 w999]
                          frame #0 {
                            n625 = call "sub vi - defrag tdms v1.vi"("panel id"=w997) -> ("error out"=w996:errorcluster)  [unwired: 10 in]
                            n626 = local write "data file error"(w996) -> ()
                          }
                          frame #1 {
                            n627 = call "Save data file to network drive v1.vi"("panel id"=w999) -> ("network file save error"=w998:errorcluster)  [unwired: 9 in, 1 out]
                            n628 = local write "RESULT LAB04-1"(FALSE) -> ()
                            n629 = local write "data file error"(w998) -> ()
                          }
                        }
                        n630 = Bundle(cluster=w995, "STATUS"="STOP") -> (w993:T4)  [unwired: 2 in]
                        n631 = local write "DISP LAB04-1"(w993) -> ()
                      }
                    }
                  }
                  frame True {
                    # "start new test and create test file"
                    n632 = stacked-sequence {
                      seq-local: [w1007 _ _ _ _] -> [_ w1032 _ _ _]
                      tunnel: w1006 -> [w1012 _ _ _ _]
                      tunnel: w1005 -> [w1008 _ _ _ _]
                      tunnel: w1004 -> [w1022 _ _ _ _]
                      tunnel: w1003 -> [w1015 _ _ _ _]
                      tunnel: w1002 -> [w1010 _ _ _ _]
                      tunnel: [_ w1026 _ _ _] -> w1001
                      frame #0 {
                        w1009 = "\\"
                        n633 = local read "SET LAB04-1"() -> (w1017:T5)
                        n634 = case shown="\"CYCLE TEST\"" w1022 {
                          tunnel: ["L04-1-CHART TEST-" "L04-1-CYCLE TEST-" "L04-1-T-RISE TEST-"] -> w1018
                          frame "CHART TEST", Default {
                          }
                          frame "CYCLE TEST" {
                          }
                          frame "T-RISE TEST" {
                          }
                        }
                        n635 = Unbundle(w1017) -> ("DESCRIPTION"=w1016:string)  [unwired: 4 out]
                        n636 = Concatenate Strings(w1012, "\\", w1010, w1009, w1008, w1009) -> (w1019:string)
                        n637 = String To Path(string=w1019) -> (path=w1021:path)
                        n638 = Concatenate Strings(w1019, w1018, w1016, "-", w1015, ".tdms") -> (w1007:string)
                        n639 = Create Folder(path (use dialog)=w1021) -> (error out=w1020:errorcluster)  [unwired: 2 in, 2 out]
                        n640 = global write "Global 1.vi" "LAB04-1 FILE"(w1007) -> ()
                        n641 = call <vilib>:"Clear Errors.vi"("error in (no error)"=w1020) -> ()  [unwired: 6 in, 1 out]
                      }
                      frame #1 {
                        n642 = String To Path(string=w1032) -> (path=w1027:path)
                        n643 = TDMS Open(5:FALSE, 6:FALSE, 10:T17."create or replace" ("operation (0:open)"), 11:w1027) -> (0:w1026:errorcluster, 3:→"TDMS LAB04-1":refnum<k34>)  [unwired: 3 in]
                      }
                      frame #2 {
                        n644 = local read "SET LAB04-1"() -> (w1038:T5)
                        n645 = local read "TDMS LAB04-1"() -> (w1049:refnum<k34>)
                        n646 = Build Array("Testers Name", "Description", "Set Test Cycles", "T-Rise minutes", "T-Rise Deg C") -> (w1039:string[])
                        n647 = Unbundle(w1038) -> ("NAME"=w1037:string, "DESCRIPTION"=w1036:string, "CYCLES"=w1035:dbl, "T-RISE mins"=w1034:dbl, "T-RISE deg C"=w1033:dbl)
                        n648 = Number To Decimal String(number=w1035) -> (decimal integer string=w1048:string)  [unwired: 1 in]
                        n649 = Number To Decimal String(number=w1034) -> (decimal integer string=w1047:string)  [unwired: 1 in]
                        n650 = Number To Decimal String(number=w1033) -> (decimal integer string=w1046:string)  [unwired: 1 in]
                        n651 = Build Array(w1037, w1036, w1048, w1047, w1046) -> (w1045:string[])
                        n652 = TDMS Set Properties(5:w1045, 7:w1039, 11:w1049) -> ()  [unwired: 3 in, 4 out]
                      }
                      frame #3 {
                        w1051 = 0.0
                        n653 = local read "DISP LAB04-1"() -> (w1053:T4)
                        n654 = Bundle(cluster=w1053, "CYCLE"=w1051, "MINS"=w1051, "STATUS"="RUN") -> (w1052:T4)
                        n655 = local write "DISP LAB04-1"(w1052) -> ()
                      }
                      frame #4 {
                        n656 = local read "SIG LAB04-1"() -> (w1056:T2)
                        n657 = local read "TEMP START LAB04-1"() -> (w1058:cluster{"TL":dbl, "TN":dbl})
                        n658 = Unbundle(w1056) -> ("Tmp Live"=w1055:dbl, "Tmp Neut"=w1054:dbl)  [unwired: 3 out]
                        n659 = Bundle(cluster=w1058, "TL"=w1055, "TN"=w1054) -> (w1057:cluster{"TL":dbl, "TN":dbl})
                        n660 = local write "TEMP START LAB04-1"(w1057) -> ()
                      }
                    }
                  }
                }
              }
              event "RUN LAB04-2": Value Change {
                n661 = event-data() -> ("NewVal"=w1059:bool)  [unwired: 1 in, 5 out]
                n662 = local write "run lab04-2"(w1059) -> ()
                n663 = case shown="True" w1059 {
                  tunnel: w1065 -> [_ w1098]
                  tunnel: w1064 -> [_ w1097]
                  tunnel: w1062 -> [w1067 w1096]
                  tunnel: w1063 -> [_ w1095]
                  tunnel: w1061 -> [_ w1094]
                  tunnel: [w1066 w1093] -> w1060
                  frame False {
                    # "stop test"
                    n664 = stacked-sequence {
                      tunnel: w1067 -> [w1076 _]
                      tunnel: [w1068 _] -> w1066
                      frame #0 {
                        n665 = local read "DISP LAB04-2"() -> (w1075:T4)
                        n666 = Unbundle(w1075) -> ("CYCLE"=w1073:dbl, "MINS"=w1074:dbl)  [unwired: 1 out]
                        n667 = case shown="\"CYCLE TEST\"" w1076 {
                          tunnel: w1074 -> [_ _ w1083]
                          tunnel: w1073 -> [w1081 w1082 _]
                          tunnel: [w1081 w1082 w1083] -> w1072
                          frame "CHART TEST", Default {
                          }
                          frame "CYCLE TEST" {
                          }
                          frame "T-RISE TEST" {
                          }
                        }
                        n668 = local read "TDMS LAB04-2"() -> (w1080:refnum<k34>)
                        n669 = Build Array("STOPPED") -> (w1077:string[])
                        n670 = Build Array(w1072) -> (w1071:dbl[])
                        n671 = TDMS Write(0:w1080, 5:"TEST RESULT", 7:w1077, 9:w1071) -> (4:w1069:refnum<k34>, 15:w1070:errorcluster)  [unwired: 2 in, 2 out]
                        n672 = TDMS Close(8:w1070, 11:w1069) -> (0:w1068:errorcluster)  [unwired: 1 out]
                      }
                      frame #1 {
                        n673 = local read "DISP LAB04-2"() -> (w1087:T4)
                        n674 = stacked-sequence {
                          tunnel: "LAB04-2" -> [w1089 w1091]
                          frame #0 {
                            n675 = call "sub vi - defrag tdms v1.vi"("panel id"=w1089) -> ("error out"=w1088:errorcluster)  [unwired: 10 in]
                            n676 = local write "data file error"(w1088) -> ()
                          }
                          frame #1 {
                            n677 = call "Save data file to network drive v1.vi"("panel id"=w1091) -> ("network file save error"=w1090:errorcluster)  [unwired: 9 in, 1 out]
                            n678 = local write "RESULT LAB04-2"(FALSE) -> ()
                            n679 = local write "data file error"(w1090) -> ()
                          }
                        }
                        n680 = Bundle(cluster=w1087, "STATUS"="STOP") -> (w1085:T4)  [unwired: 2 in]
                        n681 = local write "DISP LAB04-2"(w1085) -> ()
                      }
                    }
                  }
                  frame True {
                    # "start new test and create test file"
                    n682 = stacked-sequence {
                      seq-local: [w1099 _ _ _ _] -> [_ w1124 _ _ _]
                      tunnel: w1098 -> [w1104 _ _ _ _]
                      tunnel: w1097 -> [w1100 _ _ _ _]
                      tunnel: w1096 -> [w1114 _ _ _ _]
                      tunnel: w1095 -> [w1107 _ _ _ _]
                      tunnel: w1094 -> [w1102 _ _ _ _]
                      tunnel: [_ w1118 _ _ _] -> w1093
                      frame #0 {
                        w1101 = "\\"
                        n683 = local read "SET LAB04-2"() -> (w1109:T5)
                        n684 = case shown="\"CHART TEST\", Default" w1114 {
                          tunnel: ["L04-2-CHART TEST-" "L04-2-CYCLE TEST-" "L04-2-T-RISE TEST-"] -> w1110
                          frame "CHART TEST", Default {
                          }
                          frame "CYCLE TEST" {
                          }
                          frame "T-RISE TEST" {
                          }
                        }
                        n685 = Unbundle(w1109) -> ("DESCRIPTION"=w1108:string)  [unwired: 4 out]
                        n686 = Concatenate Strings(w1104, "\\", w1102, w1101, w1100, w1101) -> (w1111:string)
                        n687 = String To Path(string=w1111) -> (path=w1113:path)
                        n688 = Concatenate Strings(w1111, w1110, w1108, "-", w1107, ".tdms") -> (w1099:string)
                        n689 = Create Folder(path (use dialog)=w1113) -> (error out=w1112:errorcluster)  [unwired: 2 in, 2 out]
                        n690 = global write "Global 1.vi" "LAB04-2 FILE"(w1099) -> ()
                        n691 = call <vilib>:"Clear Errors.vi"("error in (no error)"=w1112) -> ()  [unwired: 6 in, 1 out]
                      }
                      frame #1 {
                        n692 = String To Path(string=w1124) -> (path=w1119:path)
                        n693 = TDMS Open(5:FALSE, 6:FALSE, 10:T17."create or replace" ("operation (0:open)"), 11:w1119) -> (0:w1118:errorcluster, 3:→"TDMS LAB04-2":refnum<k34>)  [unwired: 3 in]
                      }
                      frame #2 {
                        n694 = local read "SET LAB04-2"() -> (w1130:T5)
                        n695 = local read "TDMS LAB04-2"() -> (w1141:refnum<k34>)
                        n696 = Build Array("Testers Name", "Description", "Set Test Cycles", "T-Rise minutes", "T-Rise Deg C") -> (w1131:string[])
                        n697 = Unbundle(w1130) -> ("NAME"=w1129:string, "DESCRIPTION"=w1128:string, "CYCLES"=w1127:dbl, "T-RISE mins"=w1126:dbl, "T-RISE deg C"=w1125:dbl)
                        n698 = Number To Decimal String(number=w1127) -> (decimal integer string=w1140:string)  [unwired: 1 in]
                        n699 = Number To Decimal String(number=w1126) -> (decimal integer string=w1139:string)  [unwired: 1 in]
                        n700 = Number To Decimal String(number=w1125) -> (decimal integer string=w1138:string)  [unwired: 1 in]
                        n701 = Build Array(w1129, w1128, w1140, w1139, w1138) -> (w1137:string[])
                        n702 = TDMS Set Properties(5:w1137, 7:w1131, 11:w1141) -> ()  [unwired: 3 in, 4 out]
                      }
                      frame #3 {
                        w1143 = 0.0
                        n703 = local read "DISP LAB04-2"() -> (w1145:T4)
                        n704 = Bundle(cluster=w1145, "CYCLE"=w1143, "MINS"=w1143, "STATUS"="RUN") -> (w1144:T4)
                        n705 = local write "DISP LAB04-2"(w1144) -> ()
                      }
                      frame #4 {
                        n706 = local read "SIG LAB04-2"() -> (w1148:T2)
                        n707 = local read "TEMP START LAB04-2"() -> (w1150:cluster{"TL":dbl, "TN":dbl})
                        n708 = Unbundle(w1148) -> ("Tmp Live"=w1147:dbl, "Tmp Neut"=w1146:dbl)  [unwired: 3 out]
                        n709 = Bundle(cluster=w1150, "TL"=w1147, "TN"=w1146) -> (w1149:cluster{"TL":dbl, "TN":dbl})
                        n710 = local write "TEMP START LAB04-2"(w1149) -> ()
                      }
                    }
                  }
                }
              }
              event "RUN LAB05-1": Value Change {
                n711 = event-data() -> ("NewVal"=w1151:bool)  [unwired: 1 in, 5 out]
                n712 = local write "run lab05-1"(w1151) -> ()
                n713 = case shown="True" w1151 {
                  tunnel: w1157 -> [_ w1190]
                  tunnel: w1156 -> [_ w1189]
                  tunnel: w1154 -> [w1159 w1188]
                  tunnel: w1155 -> [_ w1187]
                  tunnel: w1153 -> [_ w1186]
                  tunnel: [w1158 w1185] -> w1152
                  frame False {
                    # "stop test"
                    n714 = stacked-sequence {
                      tunnel: w1159 -> [w1168 _]
                      tunnel: [w1160 _] -> w1158
                      frame #0 {
                        n715 = local read "DISP LAB05-1"() -> (w1167:T4)
                        n716 = Unbundle(w1167) -> ("CYCLE"=w1165:dbl, "MINS"=w1166:dbl)  [unwired: 1 out]
                        n717 = case shown="\"CYCLE TEST\"" w1168 {
                          tunnel: w1166 -> [_ _ w1175]
                          tunnel: w1165 -> [w1173 w1174 _]
                          tunnel: [w1173 w1174 w1175] -> w1164
                          frame "CHART TEST", Default {
                          }
                          frame "CYCLE TEST" {
                          }
                          frame "T-RISE TEST" {
                          }
                        }
                        n718 = local read "TDMS LAB05-1"() -> (w1172:refnum<k34>)
                        n719 = Build Array("STOPPED") -> (w1169:string[])
                        n720 = Build Array(w1164) -> (w1163:dbl[])
                        n721 = TDMS Write(0:w1172, 5:"TEST RESULT", 7:w1169, 9:w1163) -> (4:w1161:refnum<k34>, 15:w1162:errorcluster)  [unwired: 2 in, 2 out]
                        n722 = TDMS Close(8:w1162, 11:w1161) -> (0:w1160:errorcluster)  [unwired: 1 out]
                      }
                      frame #1 {
                        n723 = local read "DISP LAB05-1"() -> (w1179:T4)
                        n724 = stacked-sequence {
                          tunnel: "LAB05-1" -> [w1181 w1183]
                          frame #0 {
                            n725 = call "sub vi - defrag tdms v1.vi"("panel id"=w1181) -> ("error out"=w1180:errorcluster)  [unwired: 10 in]
                            n726 = local write "data file error"(w1180) -> ()
                          }
                          frame #1 {
                            n727 = call "Save data file to network drive v1.vi"("panel id"=w1183) -> ("network file save error"=w1182:errorcluster)  [unwired: 9 in, 1 out]
                            n728 = local write "RESULT LAB05-1"(FALSE) -> ()
                            n729 = local write "data file error"(w1182) -> ()
                          }
                        }
                        n730 = Bundle(cluster=w1179, "STATUS"="STOP") -> (w1177:T4)  [unwired: 2 in]
                        n731 = local write "DISP LAB05-1"(w1177) -> ()
                      }
                    }
                  }
                  frame True {
                    # "start new test and create test file"
                    n732 = stacked-sequence {
                      seq-local: [w1191 _ _ _ _] -> [_ w1216 _ _ _]
                      tunnel: w1190 -> [w1196 _ _ _ _]
                      tunnel: w1189 -> [w1192 _ _ _ _]
                      tunnel: w1188 -> [w1206 _ _ _ _]
                      tunnel: w1187 -> [w1199 _ _ _ _]
                      tunnel: w1186 -> [w1194 _ _ _ _]
                      tunnel: [_ w1210 _ _ _] -> w1185
                      frame #0 {
                        w1193 = "\\"
                        n733 = local read "SET LAB05-1"() -> (w1201:T5)
                        n734 = case shown="\"CYCLE TEST\"" w1206 {
                          tunnel: ["L05-1-CHART TEST-" "L05-1-CYCLE TEST-" "L05-1-T-RISE TEST-"] -> w1202
                          frame "CHART TEST", Default {
                          }
                          frame "CYCLE TEST" {
                          }
                          frame "T-RISE TEST" {
                          }
                        }
                        n735 = Unbundle(w1201) -> ("DESCRIPTION"=w1200:string)  [unwired: 4 out]
                        n736 = Concatenate Strings(w1196, "\\", w1194, w1193, w1192, w1193) -> (w1203:string)
                        n737 = String To Path(string=w1203) -> (path=w1205:path)
                        n738 = Concatenate Strings(w1203, w1202, w1200, "-", w1199, ".tdms") -> (w1191:string)
                        n739 = Create Folder(path (use dialog)=w1205) -> (error out=w1204:errorcluster)  [unwired: 2 in, 2 out]
                        n740 = global write "Global 1.vi" "LAB05-1 FILE"(w1191) -> ()
                        n741 = call <vilib>:"Clear Errors.vi"("error in (no error)"=w1204) -> ()  [unwired: 6 in, 1 out]
                      }
                      frame #1 {
                        n742 = String To Path(string=w1216) -> (path=w1211:path)
                        n743 = TDMS Open(5:FALSE, 6:FALSE, 10:T17."create or replace" ("operation (0:open)"), 11:w1211) -> (0:w1210:errorcluster, 3:→"TDMS LAB05-1":refnum<k34>)  [unwired: 3 in]
                      }
                      frame #2 {
                        n744 = local read "SET LAB05-1"() -> (w1222:T5)
                        n745 = local read "TDMS LAB05-1"() -> (w1233:refnum<k34>)
                        n746 = Build Array("Testers Name", "Description", "Set Test Cycles", "T-Rise minutes", "T-Rise Deg C") -> (w1223:string[])
                        n747 = Unbundle(w1222) -> ("NAME"=w1221:string, "DESCRIPTION"=w1220:string, "CYCLES"=w1219:dbl, "T-RISE mins"=w1218:dbl, "T-RISE deg C"=w1217:dbl)
                        n748 = Number To Decimal String(number=w1219) -> (decimal integer string=w1232:string)  [unwired: 1 in]
                        n749 = Number To Decimal String(number=w1218) -> (decimal integer string=w1231:string)  [unwired: 1 in]
                        n750 = Number To Decimal String(number=w1217) -> (decimal integer string=w1230:string)  [unwired: 1 in]
                        n751 = Build Array(w1221, w1220, w1232, w1231, w1230) -> (w1229:string[])
                        n752 = TDMS Set Properties(5:w1229, 7:w1223, 11:w1233) -> ()  [unwired: 3 in, 4 out]
                      }
                      frame #3 {
                        w1235 = 0.0
                        n753 = local read "DISP LAB05-1"() -> (w1237:T4)
                        n754 = Bundle(cluster=w1237, "CYCLE"=w1235, "MINS"=w1235, "STATUS"="RUN") -> (w1236:T4)
                        n755 = local write "DISP LAB05-1"(w1236) -> ()
                      }
                      frame #4 {
                        n756 = local read "SIG LAB05-1"() -> (w1240:T2)
                        n757 = local read "TEMP START LAB05-1"() -> (w1242:cluster{"TL":dbl, "TN":dbl})
                        n758 = Unbundle(w1240) -> ("Tmp Live"=w1239:dbl, "Tmp Neut"=w1238:dbl)  [unwired: 3 out]
                        n759 = Bundle(cluster=w1242, "TL"=w1239, "TN"=w1238) -> (w1241:cluster{"TL":dbl, "TN":dbl})
                        n760 = local write "TEMP START LAB05-1"(w1241) -> ()
                      }
                    }
                  }
                }
              }
              event "RUN LAB05-2": Value Change {
                n761 = event-data() -> ("NewVal"=w1243:bool)  [unwired: 1 in, 5 out]
                n762 = local write "run lab05-2"(w1243) -> ()
                n763 = case shown="True" w1243 {
                  tunnel: w1249 -> [_ w1282]
                  tunnel: w1248 -> [_ w1281]
                  tunnel: w1246 -> [w1251 w1280]
                  tunnel: w1247 -> [_ w1279]
                  tunnel: w1245 -> [_ w1278]
                  tunnel: [w1250 w1277] -> w1244
                  frame False {
                    # "stop test"
                    n764 = stacked-sequence {
                      tunnel: w1251 -> [w1260 _]
                      tunnel: [w1252 _] -> w1250
                      frame #0 {
                        n765 = local read "DISP LAB05-2"() -> (w1259:T4)
                        n766 = Unbundle(w1259) -> ("CYCLE"=w1257:dbl, "MINS"=w1258:dbl)  [unwired: 1 out]
                        n767 = case shown="\"CYCLE TEST\"" w1260 {
                          tunnel: w1258 -> [_ _ w1267]
                          tunnel: w1257 -> [w1265 w1266 _]
                          tunnel: [w1265 w1266 w1267] -> w1256
                          frame "CHART TEST", Default {
                          }
                          frame "CYCLE TEST" {
                          }
                          frame "T-RISE TEST" {
                          }
                        }
                        n768 = local read "TDMS LAB05-2"() -> (w1264:refnum<k34>)
                        n769 = Build Array("STOPPED") -> (w1261:string[])
                        n770 = Build Array(w1256) -> (w1255:dbl[])
                        n771 = TDMS Write(0:w1264, 5:"TEST RESULT", 7:w1261, 9:w1255) -> (4:w1253:refnum<k34>, 15:w1254:errorcluster)  [unwired: 2 in, 2 out]
                        n772 = TDMS Close(8:w1254, 11:w1253) -> (0:w1252:errorcluster)  [unwired: 1 out]
                      }
                      frame #1 {
                        n773 = local read "DISP LAB05-2"() -> (w1271:T4)
                        n774 = stacked-sequence {
                          tunnel: "LAB05-2" -> [w1273 w1275]
                          frame #0 {
                            n775 = call "sub vi - defrag tdms v1.vi"("panel id"=w1273) -> ("error out"=w1272:errorcluster)  [unwired: 10 in]
                            n776 = local write "data file error"(w1272) -> ()
                          }
                          frame #1 {
                            n777 = local write "RESULT LAB05-2"(FALSE) -> ()
                            n778 = call "Save data file to network drive v1.vi"("panel id"=w1275) -> ("network file save error"=w1274:errorcluster)  [unwired: 9 in, 1 out]
                            n779 = local write "data file error"(w1274) -> ()
                          }
                        }
                        n780 = Bundle(cluster=w1271, "STATUS"="STOP") -> (w1269:T4)  [unwired: 2 in]
                        n781 = local write "DISP LAB05-2"(w1269) -> ()
                      }
                    }
                  }
                  frame True {
                    # "start new test and create test file"
                    n782 = stacked-sequence {
                      seq-local: [w1283 _ _ _ _] -> [_ w1308 _ _ _]
                      tunnel: w1282 -> [w1288 _ _ _ _]
                      tunnel: w1281 -> [w1284 _ _ _ _]
                      tunnel: w1280 -> [w1298 _ _ _ _]
                      tunnel: w1279 -> [w1291 _ _ _ _]
                      tunnel: w1278 -> [w1286 _ _ _ _]
                      tunnel: [_ w1302 _ _ _] -> w1277
                      frame #0 {
                        w1285 = "\\"
                        n783 = local read "SET LAB05-2"() -> (w1293:T5)
                        n784 = case shown="\"CYCLE TEST\"" w1298 {
                          tunnel: ["L05-2-CHART TEST-" "L05-2-CYCLE TEST-" "L05-2-T-RISE TEST-"] -> w1294
                          frame "CHART TEST", Default {
                          }
                          frame "CYCLE TEST" {
                          }
                          frame "T-RISE TEST" {
                          }
                        }
                        n785 = Unbundle(w1293) -> ("DESCRIPTION"=w1292:string)  [unwired: 4 out]
                        n786 = Concatenate Strings(w1288, "\\", w1286, w1285, w1284, w1285) -> (w1295:string)
                        n787 = String To Path(string=w1295) -> (path=w1297:path)
                        n788 = Concatenate Strings(w1295, w1294, w1292, "-", w1291, ".tdms") -> (w1283:string)
                        n789 = Create Folder(path (use dialog)=w1297) -> (error out=w1296:errorcluster)  [unwired: 2 in, 2 out]
                        n790 = global write "Global 1.vi" "LAB05-2 FILE"(w1283) -> ()
                        n791 = call <vilib>:"Clear Errors.vi"("error in (no error)"=w1296) -> ()  [unwired: 6 in, 1 out]
                      }
                      frame #1 {
                        n792 = String To Path(string=w1308) -> (path=w1303:path)
                        n793 = TDMS Open(5:FALSE, 6:FALSE, 10:T17."create or replace" ("operation (0:open)"), 11:w1303) -> (0:w1302:errorcluster, 3:→"TDMS LAB05-2":refnum<k34>)  [unwired: 3 in]
                      }
                      frame #2 {
                        n794 = local read "SET LAB05-2"() -> (w1314:T5)
                        n795 = local read "TDMS LAB05-2"() -> (w1325:refnum<k34>)
                        n796 = Build Array("Testers Name", "Description", "Set Test Cycles", "T-Rise minutes", "T-Rise Deg C") -> (w1315:string[])
                        n797 = Unbundle(w1314) -> ("NAME"=w1313:string, "DESCRIPTION"=w1312:string, "CYCLES"=w1311:dbl, "T-RISE mins"=w1310:dbl, "T-RISE deg C"=w1309:dbl)
                        n798 = Number To Decimal String(number=w1311) -> (decimal integer string=w1324:string)  [unwired: 1 in]
                        n799 = Number To Decimal String(number=w1310) -> (decimal integer string=w1323:string)  [unwired: 1 in]
                        n800 = Number To Decimal String(number=w1309) -> (decimal integer string=w1322:string)  [unwired: 1 in]
                        n801 = Build Array(w1313, w1312, w1324, w1323, w1322) -> (w1321:string[])
                        n802 = TDMS Set Properties(5:w1321, 7:w1315, 11:w1325) -> ()  [unwired: 3 in, 4 out]
                      }
                      frame #3 {
                        w1327 = 0.0
                        n803 = local read "DISP LAB05-2"() -> (w1329:T4)
                        n804 = Bundle(cluster=w1329, "CYCLE"=w1327, "MINS"=w1327, "STATUS"="RUN") -> (w1328:T4)
                        n805 = local write "DISP LAB05-2"(w1328) -> ()
                      }
                      frame #4 {
                        n806 = local read "SIG LAB05-2"() -> (w1332:T2)
                        n807 = local read "TEMP START LAB05-2"() -> (w1334:cluster{"TL":dbl, "TN":dbl})
                        n808 = Unbundle(w1332) -> ("Tmp Live"=w1331:dbl, "Tmp Neut"=w1330:dbl)  [unwired: 3 out]
                        n809 = Bundle(cluster=w1334, "TL"=w1331, "TN"=w1330) -> (w1333:cluster{"TL":dbl, "TN":dbl})
                        n810 = local write "TEMP START LAB05-2"(w1333) -> ()
                      }
                    }
                  }
                }
              }
            }
            n811 = local write "data file error"(w386) -> ()
          }
          frame #4 {
            # "check if test cycles reached for cycle tests, if so then test pass"
            n812 = stacked-sequence {
              tunnel: w1354 -> [_ _ _ _ _ _ _ _ _ _]
              tunnel: w1353 -> [_ _ _ _ _ _ _ _ _ _]
              tunnel: w1352 -> [_ _ _ _ _ _ _ _ _ _]
              tunnel: w1351 -> [_ _ _ _ _ _ _ _ _ _]
              tunnel: w1350 -> [_ _ _ _ _ _ _ _ _ _]
              tunnel: w1349 -> [_ _ _ _ _ _ _ _ _ _]
              tunnel: w1348 -> [_ _ _ _ _ _ _ _ _ _]
              tunnel: w1347 -> [_ _ _ _ _ _ _ _ _ _]
              tunnel: w1346 -> [_ _ _ _ _ _ _ _ _ _]
              tunnel: w1345 -> [_ _ _ _ _ _ _ _ _ _]
              tunnel: w1344 -> [w1360 _ _ _ _ _ _ _ _ _]
              tunnel: w1343 -> [_ w1395 _ _ _ _ _ _ _ _]
              tunnel: w1342 -> [_ _ w1435 _ _ _ _ _ _ _]
              tunnel: w1341 -> [_ _ _ w1475 _ _ _ _ _ _]
              tunnel: w1340 -> [_ _ _ _ w1515 _ _ _ _ _]
              tunnel: w1339 -> [_ _ _ _ _ w1555 _ _ _ _]
              tunnel: w1338 -> [_ _ _ _ _ _ w1595 _ _ _]
              tunnel: w1337 -> [_ _ _ _ _ _ _ w1635 _ _]
              tunnel: w1336 -> [_ _ _ _ _ _ _ _ w1675 _]
              tunnel: w1335 -> [_ _ _ _ _ _ _ _ _ w1715]
              frame #0 {
                # "LAB01-1"
                n813 = Less?(x=w1360, y=2) -> (x < y?=w1358:bool)
                n814 = local read "DISP LAB01-1"() -> (w1361:T4)
                n815 = Unbundle(w1361) -> ("STATUS"=w1355:string)  [unwired: 2 out]
                n816 = Equal?(x=w1355, y="RUN") -> (x = y?=w1357:bool)
                n817 = And(x=w1357, y=w1358) -> (x .and. y?=w1356:bool)
                n818 = case shown="True" w1356 {
                  tunnel: w1361 -> [_ w1366]
                  tunnel: w1360 -> [_ w1370]
                  frame False {
                  }
                  frame True {
                    n819 = local read "SET LAB01-1"() -> (w1372:T5)
                    n820 = local read "TDMS LAB01-1"() -> (w1365:refnum<k34>)
                    n821 = Unbundle(w1372) -> ("CYCLES"=w1363:dbl, "T-RISE mins"=w1369:dbl)  [unwired: 3 out]
                    n822 = case shown="\"CYCLE TEST\"" w1370 {
                      tunnel: w1369 -> [_ _ w1379]
                      tunnel: [w1374 w1376 w1379] -> w1368
                      tunnel: w1363 -> [w1374 w1376 _]
                      tunnel: ["CHART PASS" "CYCLE PASS" "T-RISE PASS"] -> w1367
                      frame "CHART TEST", Default {
                      }
                      frame "CYCLE TEST" {
                      }
                      frame "T-RISE TEST" {
                      }
                    }
                    n823 = Unbundle(w1366) -> ("CYCLE"=w1371:dbl)  [unwired: 2 out]
                    n824 = Increment(x=w1363) -> (x+1=w1364:dbl)
                    n825 = Greater Or Equal?(x=w1371, y=w1364) -> (x >= y?=w1373:bool)
                    n826 = case shown="True" w1373 {
                      tunnel: w1368 -> [w1383 _]
                      tunnel: w1367 -> [w1382 _]
                      tunnel: w1366 -> [w1381 _]
                      tunnel: w1365 -> [w1380 _]
                      frame True {
                        n827 = stacked-sequence {
                          tunnel: w1383 -> [w1387 _]
                          tunnel: w1382 -> [w1385 w1391]
                          tunnel: w1381 -> [_ w1394]
                          tunnel: w1380 -> [w1384 _]
                          frame #0 {
                            n828 = Build Array(w1385) -> (w1388:string[])
                            n829 = Build Array(w1387) -> (w1386:dbl[])
                            n830 = TDMS Write(0:w1384, 5:"TEST PASS", 7:w1388, 9:w1386) -> (15:w1390:errorcluster)  [unwired: 2 in, 3 out]
                            n831 = local write "data file error"(w1390) -> ()
                          }
                          frame #1 {
                            n832 = Bundle(cluster=w1394, "STATUS"=w1391) -> (w1392:T4)  [unwired: 2 in]
                            n833 = local write "RESULT LAB01-1"(TRUE) -> ()
                            n834 = local write "DISP LAB01-1"(w1392) -> ()
                          }
                        }
                      }
                      frame False {
                      }
                    }
                  }
                }
              }
              frame #1 {
                # "LAB01-2"
                n835 = Less?(x=w1395, y=2) -> (x < y?=w1398:bool)
                n836 = local read "DISP LAB01-2"() -> (w1400:T4)
                n837 = Unbundle(w1400) -> ("STATUS"=w1401:string)  [unwired: 2 out]
                n838 = Equal?(x=w1401, y="RUN") -> (x = y?=w1397:bool)
                n839 = And(x=w1397, y=w1398) -> (x .and. y?=w1396:bool)
                n840 = case shown="True" w1396 {
                  tunnel: w1400 -> [_ w1406]
                  tunnel: w1395 -> [_ w1410]
                  frame False {
                  }
                  frame True {
                    n841 = local read "SET LAB01-2"() -> (w1412:T5)
                    n842 = local read "TDMS LAB01-2"() -> (w1405:refnum<k34>)
                    n843 = Unbundle(w1412) -> ("CYCLES"=w1403:dbl, "T-RISE mins"=w1409:dbl)  [unwired: 3 out]
                    n844 = case shown="\"T-RISE TEST\"" w1410 {
                      tunnel: w1409 -> [_ _ w1419]
                      tunnel: [w1414 w1416 w1419] -> w1408
                      tunnel: w1403 -> [w1414 w1416 _]
                      tunnel: ["CHART PASS" "CYCLE PASS" "T-RISE PASS"] -> w1407
                      frame "CHART TEST", Default {
                      }
                      frame "CYCLE TEST" {
                      }
                      frame "T-RISE TEST" {
                      }
                    }
                    n845 = Unbundle(w1406) -> ("CYCLE"=w1411:dbl)  [unwired: 2 out]
                    n846 = Increment(x=w1403) -> (x+1=w1404:dbl)
                    n847 = Greater Or Equal?(x=w1411, y=w1404) -> (x >= y?=w1413:bool)
                    n848 = case shown="True" w1413 {
                      tunnel: w1408 -> [w1423 _]
                      tunnel: w1407 -> [w1422 _]
                      tunnel: w1406 -> [w1421 _]
                      tunnel: w1405 -> [w1420 _]
                      frame True {
                        n849 = stacked-sequence {
                          tunnel: w1423 -> [w1427 _]
                          tunnel: w1422 -> [w1425 w1431]
                          tunnel: w1421 -> [_ w1434]
                          tunnel: w1420 -> [w1424 _]
                          frame #0 {
                            n850 = Build Array(w1425) -> (w1428:string[])
                            n851 = Build Array(w1427) -> (w1426:dbl[])
                            n852 = TDMS Write(0:w1424, 5:"TEST PASS", 7:w1428, 9:w1426) -> (15:w1430:errorcluster)  [unwired: 2 in, 3 out]
                            n853 = local write "data file error"(w1430) -> ()
                          }
                          frame #1 {
                            n854 = Bundle(cluster=w1434, "STATUS"=w1431) -> (w1432:T4)  [unwired: 2 in]
                            n855 = local write "RESULT LAB01-2"(TRUE) -> ()
                            n856 = local write "DISP LAB01-2"(w1432) -> ()
                          }
                        }
                      }
                      frame False {
                      }
                    }
                  }
                }
              }
              frame #2 {
                # "LAB02-1"
                n857 = Less?(x=w1435, y=2) -> (x < y?=w1438:bool)
                n858 = local read "DISP LAB02-1"() -> (w1440:T4)
                n859 = Unbundle(w1440) -> ("STATUS"=w1441:string)  [unwired: 2 out]
                n860 = Equal?(x=w1441, y="RUN") -> (x = y?=w1437:bool)
                n861 = And(x=w1437, y=w1438) -> (x .and. y?=w1436:bool)
                n862 = case shown="True" w1436 {
                  tunnel: w1440 -> [_ w1446]
                  tunnel: w1435 -> [_ w1450]
                  frame False {
                  }
                  frame True {
                    n863 = local read "SET LAB02-1"() -> (w1452:T5)
                    n864 = local read "TDMS LAB02-1"() -> (w1445:refnum<k34>)
                    n865 = Unbundle(w1446) -> ("CYCLE"=w1451:dbl)  [unwired: 2 out]
                    n866 = Unbundle(w1452) -> ("CYCLES"=w1443:dbl, "T-RISE mins"=w1449:dbl)  [unwired: 3 out]
                    n867 = case shown="\"T-RISE TEST\"" w1450 {
                      tunnel: w1449 -> [_ _ w1459]
                      tunnel: [w1454 w1456 w1459] -> w1448
                      tunnel: w1443 -> [w1454 w1456 _]
                      tunnel: ["CHART PASS" "CYCLE PASS" "T-RISE PASS"] -> w1447
                      frame "CHART TEST", Default {
                      }
                      frame "CYCLE TEST" {
                      }
                      frame "T-RISE TEST" {
                      }
                    }
                    n868 = Increment(x=w1443) -> (x+1=w1444:dbl)
                    n869 = Greater Or Equal?(x=w1451, y=w1444) -> (x >= y?=w1453:bool)
                    n870 = case shown="True" w1453 {
                      tunnel: w1448 -> [w1463 _]
                      tunnel: w1447 -> [w1462 _]
                      tunnel: w1446 -> [w1461 _]
                      tunnel: w1445 -> [w1460 _]
                      frame True {
                        n871 = stacked-sequence {
                          tunnel: w1463 -> [w1467 _]
                          tunnel: w1462 -> [w1465 w1471]
                          tunnel: w1461 -> [_ w1474]
                          tunnel: w1460 -> [w1464 _]
                          frame #0 {
                            n872 = Build Array(w1465) -> (w1468:string[])
                            n873 = Build Array(w1467) -> (w1466:dbl[])
                            n874 = TDMS Write(0:w1464, 5:"TEST PASS", 7:w1468, 9:w1466) -> (15:w1470:errorcluster)  [unwired: 2 in, 3 out]
                            n875 = local write "data file error"(w1470) -> ()
                          }
                          frame #1 {
                            n876 = Bundle(cluster=w1474, "STATUS"=w1471) -> (w1472:T4)  [unwired: 2 in]
                            n877 = local write "RESULT LAB02-1"(TRUE) -> ()
                            n878 = local write "DISP LAB02-1"(w1472) -> ()
                          }
                        }
                      }
                      frame False {
                      }
                    }
                  }
                }
              }
              frame #3 {
                # "LAB02-2"
                n879 = Less?(x=w1475, y=2) -> (x < y?=w1478:bool)
                n880 = local read "DISP LAB02-2"() -> (w1480:T4)
                n881 = Unbundle(w1480) -> ("STATUS"=w1481:string)  [unwired: 2 out]
                n882 = Equal?(x=w1481, y="RUN") -> (x = y?=w1477:bool)
                n883 = And(x=w1477, y=w1478) -> (x .and. y?=w1476:bool)
                n884 = case shown="True" w1476 {
                  tunnel: w1480 -> [_ w1486]
                  tunnel: w1475 -> [_ w1490]
                  frame False {
                  }
                  frame True {
                    n885 = local read "SET LAB02-2"() -> (w1492:T5)
                    n886 = local read "TDMS LAB02-2"() -> (w1485:refnum<k34>)
                    n887 = Unbundle(w1486) -> ("CYCLE"=w1491:dbl)  [unwired: 2 out]
                    n888 = Unbundle(w1492) -> ("CYCLES"=w1483:dbl, "T-RISE mins"=w1489:dbl)  [unwired: 3 out]
                    n889 = case shown="\"T-RISE TEST\"" w1490 {
                      tunnel: w1489 -> [_ _ w1499]
                      tunnel: [w1494 w1496 w1499] -> w1488
                      tunnel: w1483 -> [w1494 w1496 _]
                      tunnel: ["CHART PASS" "CYCLE PASS" "T-RISE PASS"] -> w1487
                      frame "CHART TEST", Default {
                      }
                      frame "CYCLE TEST" {
                      }
                      frame "T-RISE TEST" {
                      }
                    }
                    n890 = Increment(x=w1483) -> (x+1=w1484:dbl)
                    n891 = Greater Or Equal?(x=w1491, y=w1484) -> (x >= y?=w1493:bool)
                    n892 = case shown="True" w1493 {
                      tunnel: w1488 -> [w1503 _]
                      tunnel: w1487 -> [w1502 _]
                      tunnel: w1486 -> [w1501 _]
                      tunnel: w1485 -> [w1500 _]
                      frame True {
                        n893 = stacked-sequence {
                          tunnel: w1503 -> [w1507 _]
                          tunnel: w1502 -> [w1505 w1511]
                          tunnel: w1501 -> [_ w1514]
                          tunnel: w1500 -> [w1504 _]
                          frame #0 {
                            n894 = Build Array(w1505) -> (w1508:string[])
                            n895 = Build Array(w1507) -> (w1506:dbl[])
                            n896 = TDMS Write(0:w1504, 5:"TEST PASS", 7:w1508, 9:w1506) -> (15:w1510:errorcluster)  [unwired: 2 in, 3 out]
                            n897 = local write "data file error"(w1510) -> ()
                          }
                          frame #1 {
                            n898 = Bundle(cluster=w1514, "STATUS"=w1511) -> (w1512:T4)  [unwired: 2 in]
                            n899 = local write "RESULT LAB02-2"(TRUE) -> ()
                            n900 = local write "DISP LAB02-2"(w1512) -> ()
                          }
                        }
                      }
                      frame False {
                      }
                    }
                  }
                }
              }
              frame #4 {
                # "LAB03-1"
                n901 = Less?(x=w1515, y=2) -> (x < y?=w1518:bool)
                n902 = local read "DISP LAB03-1"() -> (w1520:T4)
                n903 = Unbundle(w1520) -> ("STATUS"=w1521:string)  [unwired: 2 out]
                n904 = Equal?(x=w1521, y="RUN") -> (x = y?=w1517:bool)
                n905 = And(x=w1517, y=w1518) -> (x .and. y?=w1516:bool)
                n906 = case shown="True" w1516 {
                  tunnel: w1520 -> [_ w1526]
                  tunnel: w1515 -> [_ w1530]
                  frame False {
                  }
                  frame True {
                    n907 = local read "SET LAB03-1"() -> (w1532:T5)
                    n908 = local read "TDMS LAB03-1"() -> (w1525:refnum<k34>)
                    n909 = Unbundle(w1526) -> ("CYCLE"=w1531:dbl)  [unwired: 2 out]
                    n910 = Unbundle(w1532) -> ("CYCLES"=w1523:dbl, "T-RISE mins"=w1529:dbl)  [unwired: 3 out]
                    n911 = case shown="\"T-RISE TEST\"" w1530 {
                      tunnel: w1529 -> [_ _ w1539]
                      tunnel: [w1534 w1536 w1539] -> w1528
                      tunnel: w1523 -> [w1534 w1536 _]
                      tunnel: ["CHART PASS" "CYCLE PASS" "T-RISE PASS"] -> w1527
                      frame "CHART TEST", Default {
                      }
                      frame "CYCLE TEST" {
                      }
                      frame "T-RISE TEST" {
                      }
                    }
                    n912 = Increment(x=w1523) -> (x+1=w1524:dbl)
                    n913 = Greater Or Equal?(x=w1531, y=w1524) -> (x >= y?=w1533:bool)
                    n914 = case shown="True" w1533 {
                      tunnel: w1528 -> [w1543 _]
                      tunnel: w1527 -> [w1542 _]
                      tunnel: w1526 -> [w1541 _]
                      tunnel: w1525 -> [w1540 _]
                      frame True {
                        n915 = stacked-sequence {
                          tunnel: w1543 -> [w1547 _]
                          tunnel: w1542 -> [w1545 w1551]
                          tunnel: w1541 -> [_ w1554]
                          tunnel: w1540 -> [w1544 _]
                          frame #0 {
                            n916 = Build Array(w1545) -> (w1548:string[])
                            n917 = Build Array(w1547) -> (w1546:dbl[])
                            n918 = TDMS Write(0:w1544, 5:"TEST PASS", 7:w1548, 9:w1546) -> (15:w1550:errorcluster)  [unwired: 2 in, 3 out]
                            n919 = local write "data file error"(w1550) -> ()
                          }
                          frame #1 {
                            n920 = Bundle(cluster=w1554, "STATUS"=w1551) -> (w1552:T4)  [unwired: 2 in]
                            n921 = local write "RESULT LAB03-1"(TRUE) -> ()
                            n922 = local write "DISP LAB03-1"(w1552) -> ()
                          }
                        }
                      }
                      frame False {
                      }
                    }
                  }
                }
              }
              frame #5 {
                # "LAB03-2"
                n923 = Less?(x=w1555, y=2) -> (x < y?=w1558:bool)
                n924 = local read "DISP LAB03-2"() -> (w1560:T4)
                n925 = Unbundle(w1560) -> ("STATUS"=w1561:string)  [unwired: 2 out]
                n926 = Equal?(x=w1561, y="RUN") -> (x = y?=w1557:bool)
                n927 = And(x=w1557, y=w1558) -> (x .and. y?=w1556:bool)
                n928 = case shown="True" w1556 {
                  tunnel: w1560 -> [_ w1566]
                  tunnel: w1555 -> [_ w1570]
                  frame False {
                  }
                  frame True {
                    n929 = local read "SET LAB03-2"() -> (w1572:T5)
                    n930 = local read "TDMS LAB03-2"() -> (w1565:refnum<k34>)
                    n931 = Unbundle(w1566) -> ("CYCLE"=w1571:dbl)  [unwired: 2 out]
                    n932 = Unbundle(w1572) -> ("CYCLES"=w1563:dbl, "T-RISE mins"=w1569:dbl)  [unwired: 3 out]
                    n933 = case shown="\"T-RISE TEST\"" w1570 {
                      tunnel: w1569 -> [_ _ w1579]
                      tunnel: [w1574 w1576 w1579] -> w1568
                      tunnel: w1563 -> [w1574 w1576 _]
                      tunnel: ["CHART PASS" "CYCLE PASS" "T-RISE PASS"] -> w1567
                      frame "CHART TEST", Default {
                      }
                      frame "CYCLE TEST" {
                      }
                      frame "T-RISE TEST" {
                      }
                    }
                    n934 = Increment(x=w1563) -> (x+1=w1564:dbl)
                    n935 = Greater Or Equal?(x=w1571, y=w1564) -> (x >= y?=w1573:bool)
                    n936 = case shown="True" w1573 {
                      tunnel: w1568 -> [w1583 _]
                      tunnel: w1567 -> [w1582 _]
                      tunnel: w1566 -> [w1581 _]
                      tunnel: w1565 -> [w1580 _]
                      frame True {
                        n937 = stacked-sequence {
                          tunnel: w1583 -> [w1587 _]
                          tunnel: w1582 -> [w1585 w1591]
                          tunnel: w1581 -> [_ w1594]
                          tunnel: w1580 -> [w1584 _]
                          frame #0 {
                            n938 = Build Array(w1585) -> (w1588:string[])
                            n939 = Build Array(w1587) -> (w1586:dbl[])
                            n940 = TDMS Write(0:w1584, 5:"TEST PASS", 7:w1588, 9:w1586) -> (15:w1590:errorcluster)  [unwired: 2 in, 3 out]
                            n941 = local write "data file error"(w1590) -> ()
                          }
                          frame #1 {
                            n942 = Bundle(cluster=w1594, "STATUS"=w1591) -> (w1592:T4)  [unwired: 2 in]
                            n943 = local write "RESULT LAB03-2"(TRUE) -> ()
                            n944 = local write "DISP LAB03-2"(w1592) -> ()
                          }
                        }
                      }
                      frame False {
                      }
                    }
                  }
                }
              }
              frame #6 {
                # "LAB04-1"
                n945 = Less?(x=w1595, y=2) -> (x < y?=w1598:bool)
                n946 = local read "DISP LAB04-1"() -> (w1600:T4)
                n947 = Unbundle(w1600) -> ("STATUS"=w1601:string)  [unwired: 2 out]
                n948 = Equal?(x=w1601, y="RUN") -> (x = y?=w1597:bool)
                n949 = And(x=w1597, y=w1598) -> (x .and. y?=w1596:bool)
                n950 = case shown="True" w1596 {
                  tunnel: w1600 -> [_ w1606]
                  tunnel: w1595 -> [_ w1610]
                  frame False {
                  }
                  frame True {
                    n951 = local read "SET LAB04-1"() -> (w1612:T5)
                    n952 = local read "TDMS LAB04-1"() -> (w1605:refnum<k34>)
                    n953 = Unbundle(w1606) -> ("CYCLE"=w1611:dbl)  [unwired: 2 out]
                    n954 = Unbundle(w1612) -> ("CYCLES"=w1603:dbl, "T-RISE mins"=w1609:dbl)  [unwired: 3 out]
                    n955 = case shown="\"T-RISE TEST\"" w1610 {
                      tunnel: w1609 -> [_ _ w1619]
                      tunnel: [w1614 w1616 w1619] -> w1608
                      tunnel: w1603 -> [w1614 w1616 _]
                      tunnel: ["CHART PASS" "CYCLE PASS" "T-RISE PASS"] -> w1607
                      frame "CHART TEST", Default {
                      }
                      frame "CYCLE TEST" {
                      }
                      frame "T-RISE TEST" {
                      }
                    }
                    n956 = Increment(x=w1603) -> (x+1=w1604:dbl)
                    n957 = Greater Or Equal?(x=w1611, y=w1604) -> (x >= y?=w1613:bool)
                    n958 = case shown="True" w1613 {
                      tunnel: w1608 -> [w1623 _]
                      tunnel: w1607 -> [w1622 _]
                      tunnel: w1606 -> [w1621 _]
                      tunnel: w1605 -> [w1620 _]
                      frame True {
                        n959 = stacked-sequence {
                          tunnel: w1623 -> [w1627 _]
                          tunnel: w1622 -> [w1625 w1631]
                          tunnel: w1621 -> [_ w1634]
                          tunnel: w1620 -> [w1624 _]
                          frame #0 {
                            n960 = Build Array(w1625) -> (w1628:string[])
                            n961 = Build Array(w1627) -> (w1626:dbl[])
                            n962 = TDMS Write(0:w1624, 5:"TEST PASS", 7:w1628, 9:w1626) -> (15:w1630:errorcluster)  [unwired: 2 in, 3 out]
                            n963 = local write "data file error"(w1630) -> ()
                          }
                          frame #1 {
                            n964 = Bundle(cluster=w1634, "STATUS"=w1631) -> (w1632:T4)  [unwired: 2 in]
                            n965 = local write "RESULT LAB04-1"(TRUE) -> ()
                            n966 = local write "DISP LAB04-1"(w1632) -> ()
                          }
                        }
                      }
                      frame False {
                      }
                    }
                  }
                }
              }
              frame #7 {
                # "LAB04-2"
                n967 = Less?(x=w1635, y=2) -> (x < y?=w1638:bool)
                n968 = local read "DISP LAB04-2"() -> (w1640:T4)
                n969 = Unbundle(w1640) -> ("STATUS"=w1641:string)  [unwired: 2 out]
                n970 = Equal?(x=w1641, y="RUN") -> (x = y?=w1637:bool)
                n971 = And(x=w1637, y=w1638) -> (x .and. y?=w1636:bool)
                n972 = case shown="True" w1636 {
                  tunnel: w1640 -> [_ w1646]
                  tunnel: w1635 -> [_ w1650]
                  frame False {
                  }
                  frame True {
                    n973 = local read "SET LAB04-2"() -> (w1652:T5)
                    n974 = local read "TDMS LAB04-2"() -> (w1645:refnum<k34>)
                    n975 = Unbundle(w1646) -> ("CYCLE"=w1651:dbl)  [unwired: 2 out]
                    n976 = Unbundle(w1652) -> ("CYCLES"=w1643:dbl, "T-RISE mins"=w1649:dbl)  [unwired: 3 out]
                    n977 = case shown="\"T-RISE TEST\"" w1650 {
                      tunnel: w1649 -> [_ _ w1659]
                      tunnel: [w1654 w1656 w1659] -> w1648
                      tunnel: w1643 -> [w1654 w1656 _]
                      tunnel: ["CHART PASS" "CYCLE PASS" "T-RISE PASS"] -> w1647
                      frame "CHART TEST", Default {
                      }
                      frame "CYCLE TEST" {
                      }
                      frame "T-RISE TEST" {
                      }
                    }
                    n978 = Increment(x=w1643) -> (x+1=w1644:dbl)
                    n979 = Greater Or Equal?(x=w1651, y=w1644) -> (x >= y?=w1653:bool)
                    n980 = case shown="True" w1653 {
                      tunnel: w1648 -> [w1663 _]
                      tunnel: w1647 -> [w1662 _]
                      tunnel: w1646 -> [w1661 _]
                      tunnel: w1645 -> [w1660 _]
                      frame True {
                        n981 = stacked-sequence {
                          tunnel: w1663 -> [w1667 _]
                          tunnel: w1662 -> [w1665 w1671]
                          tunnel: w1661 -> [_ w1674]
                          tunnel: w1660 -> [w1664 _]
                          frame #0 {
                            n982 = Build Array(w1665) -> (w1668:string[])
                            n983 = Build Array(w1667) -> (w1666:dbl[])
                            n984 = TDMS Write(0:w1664, 5:"TEST PASS", 7:w1668, 9:w1666) -> (15:w1670:errorcluster)  [unwired: 2 in, 3 out]
                            n985 = local write "data file error"(w1670) -> ()
                          }
                          frame #1 {
                            n986 = Bundle(cluster=w1674, "STATUS"=w1671) -> (w1672:T4)  [unwired: 2 in]
                            n987 = local write "RESULT LAB04-2"(TRUE) -> ()
                            n988 = local write "DISP LAB04-2"(w1672) -> ()
                          }
                        }
                      }
                      frame False {
                      }
                    }
                  }
                }
              }
              frame #8 {
                # "LAB05-1"
                n989 = Less?(x=w1675, y=2) -> (x < y?=w1678:bool)
                n990 = local read "DISP LAB05-1"() -> (w1680:T4)
                n991 = Unbundle(w1680) -> ("STATUS"=w1681:string)  [unwired: 2 out]
                n992 = Equal?(x=w1681, y="RUN") -> (x = y?=w1677:bool)
                n993 = And(x=w1677, y=w1678) -> (x .and. y?=w1676:bool)
                n994 = case shown="True" w1676 {
                  tunnel: w1680 -> [_ w1686]
                  tunnel: w1675 -> [_ w1690]
                  frame False {
                  }
                  frame True {
                    n995 = local read "SET LAB05-1"() -> (w1692:T5)
                    n996 = local read "TDMS LAB05-1"() -> (w1685:refnum<k34>)
                    n997 = Unbundle(w1686) -> ("CYCLE"=w1691:dbl)  [unwired: 2 out]
                    n998 = Unbundle(w1692) -> ("CYCLES"=w1683:dbl, "T-RISE mins"=w1689:dbl)  [unwired: 3 out]
                    n999 = case shown="\"T-RISE TEST\"" w1690 {
                      tunnel: w1689 -> [_ _ w1699]
                      tunnel: [w1694 w1696 w1699] -> w1688
                      tunnel: w1683 -> [w1694 w1696 _]
                      tunnel: ["CHART PASS" "CYCLE PASS" "T-RISE PASS"] -> w1687
                      frame "CHART TEST", Default {
                      }
                      frame "CYCLE TEST" {
                      }
                      frame "T-RISE TEST" {
                      }
                    }
                    n1000 = Increment(x=w1683) -> (x+1=w1684:dbl)
                    n1001 = Greater Or Equal?(x=w1691, y=w1684) -> (x >= y?=w1693:bool)
                    n1002 = case shown="True" w1693 {
                      tunnel: w1688 -> [w1703 _]
                      tunnel: w1687 -> [w1702 _]
                      tunnel: w1686 -> [w1701 _]
                      tunnel: w1685 -> [w1700 _]
                      frame True {
                        n1003 = stacked-sequence {
                          tunnel: w1703 -> [w1707 _]
                          tunnel: w1702 -> [w1705 w1711]
                          tunnel: w1701 -> [_ w1714]
                          tunnel: w1700 -> [w1704 _]
                          frame #0 {
                            n1004 = Build Array(w1705) -> (w1708:string[])
                            n1005 = Build Array(w1707) -> (w1706:dbl[])
                            n1006 = TDMS Write(0:w1704, 5:"TEST PASS", 7:w1708, 9:w1706) -> (15:w1710:errorcluster)  [unwired: 2 in, 3 out]
                            n1007 = local write "data file error"(w1710) -> ()
                          }
                          frame #1 {
                            n1008 = Bundle(cluster=w1714, "STATUS"=w1711) -> (w1712:T4)  [unwired: 2 in]
                            n1009 = local write "RESULT LAB05-1"(TRUE) -> ()
                            n1010 = local write "DISP LAB05-1"(w1712) -> ()
                          }
                        }
                      }
                      frame False {
                      }
                    }
                  }
                }
              }
              frame #9 {
                # "LAB05-2"
                n1011 = Less?(x=w1715, y=2) -> (x < y?=w1718:bool)
                n1012 = local read "DISP LAB05-2"() -> (w1720:T4)
                n1013 = Unbundle(w1720) -> ("STATUS"=w1721:string)  [unwired: 2 out]
                n1014 = Equal?(x=w1721, y="RUN") -> (x = y?=w1717:bool)
                n1015 = And(x=w1717, y=w1718) -> (x .and. y?=w1716:bool)
                n1016 = case shown="True" w1716 {
                  tunnel: w1720 -> [_ w1726]
                  tunnel: w1715 -> [_ w1730]
                  frame False {
                  }
                  frame True {
                    n1017 = local read "SET LAB05-2"() -> (w1732:T5)
                    n1018 = local read "TDMS LAB05-2"() -> (w1725:refnum<k34>)
                    n1019 = Unbundle(w1726) -> ("CYCLE"=w1731:dbl)  [unwired: 2 out]
                    n1020 = Unbundle(w1732) -> ("CYCLES"=w1723:dbl, "T-RISE mins"=w1729:dbl)  [unwired: 3 out]
                    n1021 = case shown="\"T-RISE TEST\"" w1730 {
                      tunnel: w1729 -> [_ _ w1739]
                      tunnel: [w1734 w1736 w1739] -> w1728
                      tunnel: w1723 -> [w1734 w1736 _]
                      tunnel: ["CHART PASS" "CYCLE PASS" "T-RISE PASS"] -> w1727
                      frame "CHART TEST", Default {
                      }
                      frame "CYCLE TEST" {
                      }
                      frame "T-RISE TEST" {
                      }
                    }
                    n1022 = Increment(x=w1723) -> (x+1=w1724:dbl)
                    n1023 = Greater Or Equal?(x=w1731, y=w1724) -> (x >= y?=w1733:bool)
                    n1024 = case shown="True" w1733 {
                      tunnel: w1728 -> [w1743 _]
                      tunnel: w1727 -> [w1742 _]
                      tunnel: w1726 -> [w1741 _]
                      tunnel: w1725 -> [w1740 _]
                      frame True {
                        n1025 = stacked-sequence {
                          tunnel: w1743 -> [w1747 _]
                          tunnel: w1742 -> [w1745 w1751]
                          tunnel: w1741 -> [_ w1754]
                          tunnel: w1740 -> [w1744 _]
                          frame #0 {
                            n1026 = Build Array(w1745) -> (w1748:string[])
                            n1027 = Build Array(w1747) -> (w1746:dbl[])
                            n1028 = TDMS Write(0:w1744, 5:"TEST PASS", 7:w1748, 9:w1746) -> (15:w1750:errorcluster)  [unwired: 2 in, 3 out]
                            n1029 = local write "data file error"(w1750) -> ()
                          }
                          frame #1 {
                            n1030 = Bundle(cluster=w1754, "STATUS"=w1751) -> (w1752:T4)  [unwired: 2 in]
                            n1031 = local write "RESULT LAB05-2"(TRUE) -> ()
                            n1032 = local write "DISP LAB05-2"(w1752) -> ()
                          }
                        }
                      }
                      frame False {
                      }
                    }
                  }
                }
              }
            }
          }
          frame #5 {
            # "check if test cycles reached for temperature rise test"
            n1033 = stacked-sequence {
              tunnel: w1784 -> [_ _ _ _ _ _ _ _ _ _]
              tunnel: w1783 -> [_ _ _ _ _ _ _ _ _ _]
              tunnel: w1782 -> [_ _ _ _ _ _ _ _ _ _]
              tunnel: w1781 -> [_ _ _ _ _ _ _ _ _ _]
              tunnel: w1780 -> [_ _ _ _ _ _ _ _ _ _]
              tunnel: w1779 -> [_ _ _ _ _ _ _ _ _ _]
              tunnel: w1778 -> [_ _ _ _ _ _ _ _ _ _]
              tunnel: w1777 -> [_ _ _ _ _ _ _ _ _ _]
              tunnel: w1776 -> [_ _ _ _ _ _ _ _ _ _]
              tunnel: w1775 -> [_ _ _ _ _ _ _ _ _ _]
              tunnel: w1774 -> [w1790 _ _ _ _ _ _ _ _ _]
              tunnel: w1764 -> [w1785 _ _ _ _ _ _ _ _ _]
              tunnel: w1773 -> [_ w1816 _ _ _ _ _ _ _ _]
              tunnel: w1772 -> [_ _ w1846 _ _ _ _ _ _ _]
              tunnel: w1771 -> [_ _ _ w1876 _ _ _ _ _ _]
              tunnel: w1770 -> [_ _ _ _ w1906 _ _ _ _ _]
              tunnel: w1769 -> [_ _ _ _ _ w1936 _ _ _ _]
              tunnel: w1768 -> [_ _ _ _ _ _ w1966 _ _ _]
              tunnel: w1767 -> [_ _ _ _ _ _ _ w1996 _ _]
              tunnel: w1766 -> [_ _ _ _ _ _ _ _ w2026 _]
              tunnel: w1765 -> [_ _ _ _ _ _ _ _ _ w2056]
              tunnel: w1763 -> [_ w1815 _ _ _ _ _ _ _ _]
              tunnel: w1762 -> [_ _ w1845 _ _ _ _ _ _ _]
              tunnel: w1761 -> [_ _ _ w1875 _ _ _ _ _ _]
              tunnel: w1760 -> [_ _ _ _ w1905 _ _ _ _ _]
              tunnel: w1759 -> [_ _ _ _ _ w1935 _ _ _ _]
              tunnel: w1758 -> [_ _ _ _ _ _ w1965 _ _ _]
              tunnel: w1757 -> [_ _ _ _ _ _ _ w1995 _ _]
              tunnel: w1756 -> [_ _ _ _ _ _ _ _ w2025 _]
              tunnel: w1755 -> [_ _ _ _ _ _ _ _ _ w2055]
              frame #0 {
                # "LAB01-1"
                n1034 = Equal?(x=w1790, y=2) -> (x = y?=w1788:bool)
                n1035 = local read "DISP LAB01-1"() -> (w1791:T4)
                n1036 = Unbundle(w1791) -> ("STATUS"=w1792:string)  [unwired: 2 out]
                n1037 = Equal?(x=w1792, y="RUN") -> (x = y?=w1787:bool)
                n1038 = And(x=w1787, y=w1788) -> (x .and. y?=w1786:bool)
                n1039 = case shown="True" w1786 {
                  tunnel: w1791 -> [_ w1795]
                  tunnel: w1785 -> [_ w1798]
                  frame False {
                  }
                  frame True {
                    n1040 = local read "SET LAB01-1"() -> (w1797:T5)
                    n1041 = local read "TDMS LAB01-1"() -> (w1794:refnum<k34>)
                    n1042 = Unbundle(w1795) -> ("CYCLE"=w1799:dbl)  [unwired: 2 out]
                    n1043 = Unbundle(w1797) -> ("T-RISE mins"=w1796:dbl)  [unwired: 4 out]
                    n1044 = Greater Or Equal?(x=w1799, y=w1798) -> (x >= y?=w1800:bool)
                    n1045 = case shown="True" w1800 {
                      tunnel: w1796 -> [w1803 _]
                      tunnel: w1795 -> [w1802 _]
                      tunnel: w1794 -> [w1801 _]
                      frame True {
                        n1046 = stacked-sequence {
                          tunnel: w1803 -> [w1806 _]
                          tunnel: w1802 -> [_ w1811]
                          tunnel: w1801 -> [w1804 _]
                          frame #0 {
                            n1047 = Build Array("T-RISE") -> (w1808:string[])
                            n1048 = Build Array(w1806) -> (w1807:dbl[])
                            n1049 = TDMS Write(0:w1804, 5:"TEST PASS", 7:w1808, 9:w1807) -> (15:w1810:errorcluster)  [unwired: 2 in, 3 out]
                            n1050 = local write "data file error"(w1810) -> ()
                          }
                          frame #1 {
                            n1051 = Bundle(cluster=w1811, "STATUS"="T-RISE PASS") -> (w1813:T4)  [unwired: 2 in]
                            n1052 = local write "RESULT LAB01-1"(TRUE) -> ()
                            n1053 = local write "DISP LAB01-1"(w1813) -> ()
                          }
                        }
                      }
                      frame False {
                      }
                    }
                  }
                }
              }
              frame #1 {
                # "LAB01-2"
                n1054 = Equal?(x=w1816, y=2) -> (x = y?=w1819:bool)
                n1055 = local read "DISP LAB01-2"() -> (w1821:T4)
                n1056 = Unbundle(w1821) -> ("STATUS"=w1822:string)  [unwired: 2 out]
                n1057 = Equal?(x=w1822, y="RUN") -> (x = y?=w1818:bool)
                n1058 = And(x=w1818, y=w1819) -> (x .and. y?=w1817:bool)
                n1059 = case shown="True" w1817 {
                  tunnel: w1821 -> [_ w1825]
                  tunnel: w1815 -> [_ w1828]
                  frame False {
                  }
                  frame True {
                    n1060 = local read "SET LAB01-2"() -> (w1827:T5)
                    n1061 = local read "TDMS LAB01-2"() -> (w1824:refnum<k34>)
                    n1062 = Unbundle(w1825) -> ("CYCLE"=w1829:dbl)  [unwired: 2 out]
                    n1063 = Unbundle(w1827) -> ("T-RISE mins"=w1826:dbl)  [unwired: 4 out]
                    n1064 = Greater Or Equal?(x=w1829, y=w1828) -> (x >= y?=w1830:bool)
                    n1065 = case shown="True" w1830 {
                      tunnel: w1826 -> [w1833 _]
                      tunnel: w1825 -> [w1832 _]
                      tunnel: w1824 -> [w1831 _]
                      frame True {
                        n1066 = stacked-sequence {
                          tunnel: w1833 -> [w1836 _]
                          tunnel: w1832 -> [_ w1841]
                          tunnel: w1831 -> [w1834 _]
                          frame #0 {
                            n1067 = Build Array("T-RISE") -> (w1838:string[])
                            n1068 = Build Array(w1836) -> (w1837:dbl[])
                            n1069 = TDMS Write(0:w1834, 5:"TEST PASS", 7:w1838, 9:w1837) -> (15:w1840:errorcluster)  [unwired: 2 in, 3 out]
                            n1070 = local write "data file error"(w1840) -> ()
                          }
                          frame #1 {
                            n1071 = Bundle(cluster=w1841, "STATUS"="T-RISE PASS") -> (w1843:T4)  [unwired: 2 in]
                            n1072 = local write "RESULT LAB01-2"(TRUE) -> ()
                            n1073 = local write "DISP LAB01-2"(w1843) -> ()
                          }
                        }
                      }
                      frame False {
                      }
                    }
                  }
                }
              }
              frame #2 {
                # "LAB02-1"
                n1074 = Equal?(x=w1846, y=2) -> (x = y?=w1849:bool)
                n1075 = local read "DISP LAB02-1"() -> (w1851:T4)
                n1076 = Unbundle(w1851) -> ("STATUS"=w1852:string)  [unwired: 2 out]
                n1077 = Equal?(x=w1852, y="RUN") -> (x = y?=w1848:bool)
                n1078 = And(x=w1848, y=w1849) -> (x .and. y?=w1847:bool)
                n1079 = case shown="True" w1847 {
                  tunnel: w1851 -> [_ w1855]
                  tunnel: w1845 -> [_ w1858]
                  frame False {
                  }
                  frame True {
                    n1080 = local read "SET LAB02-1"() -> (w1857:T5)
                    n1081 = local read "TDMS LAB02-1"() -> (w1854:refnum<k34>)
                    n1082 = Unbundle(w1855) -> ("CYCLE"=w1859:dbl)  [unwired: 2 out]
                    n1083 = Unbundle(w1857) -> ("T-RISE mins"=w1856:dbl)  [unwired: 4 out]
                    n1084 = Greater Or Equal?(x=w1859, y=w1858) -> (x >= y?=w1860:bool)
                    n1085 = case shown="True" w1860 {
                      tunnel: w1856 -> [w1863 _]
                      tunnel: w1855 -> [w1862 _]
                      tunnel: w1854 -> [w1861 _]
                      frame True {
                        n1086 = stacked-sequence {
                          tunnel: w1863 -> [w1866 _]
                          tunnel: w1862 -> [_ w1871]
                          tunnel: w1861 -> [w1864 _]
                          frame #0 {
                            n1087 = Build Array("T-RISE") -> (w1868:string[])
                            n1088 = Build Array(w1866) -> (w1867:dbl[])
                            n1089 = TDMS Write(0:w1864, 5:"TEST PASS", 7:w1868, 9:w1867) -> (15:w1870:errorcluster)  [unwired: 2 in, 3 out]
                            n1090 = local write "data file error"(w1870) -> ()
                          }
                          frame #1 {
                            n1091 = Bundle(cluster=w1871, "STATUS"="T-RISE PASS") -> (w1873:T4)  [unwired: 2 in]
                            n1092 = local write "RESULT LAB02-1"(TRUE) -> ()
                            n1093 = local write "DISP LAB02-1"(w1873) -> ()
                          }
                        }
                      }
                      frame False {
                      }
                    }
                  }
                }
              }
              frame #3 {
                # "LAB02-2"
                n1094 = Equal?(x=w1876, y=2) -> (x = y?=w1879:bool)
                n1095 = local read "DISP LAB02-2"() -> (w1881:T4)
                n1096 = Unbundle(w1881) -> ("STATUS"=w1882:string)  [unwired: 2 out]
                n1097 = Equal?(x=w1882, y="RUN") -> (x = y?=w1878:bool)
                n1098 = And(x=w1878, y=w1879) -> (x .and. y?=w1877:bool)
                n1099 = case shown="True" w1877 {
                  tunnel: w1881 -> [_ w1885]
                  tunnel: w1875 -> [_ w1888]
                  frame False {
                  }
                  frame True {
                    n1100 = local read "SET LAB02-2"() -> (w1887:T5)
                    n1101 = local read "TDMS LAB02-2"() -> (w1884:refnum<k34>)
                    n1102 = Unbundle(w1885) -> ("CYCLE"=w1889:dbl)  [unwired: 2 out]
                    n1103 = Unbundle(w1887) -> ("T-RISE mins"=w1886:dbl)  [unwired: 4 out]
                    n1104 = Greater Or Equal?(x=w1889, y=w1888) -> (x >= y?=w1890:bool)
                    n1105 = case shown="True" w1890 {
                      tunnel: w1886 -> [w1893 _]
                      tunnel: w1885 -> [w1892 _]
                      tunnel: w1884 -> [w1891 _]
                      frame True {
                        n1106 = stacked-sequence {
                          tunnel: w1893 -> [w1896 _]
                          tunnel: w1892 -> [_ w1901]
                          tunnel: w1891 -> [w1894 _]
                          frame #0 {
                            n1107 = Build Array("T-RISE") -> (w1898:string[])
                            n1108 = Build Array(w1896) -> (w1897:dbl[])
                            n1109 = TDMS Write(0:w1894, 5:"TEST PASS", 7:w1898, 9:w1897) -> (15:w1900:errorcluster)  [unwired: 2 in, 3 out]
                            n1110 = local write "data file error"(w1900) -> ()
                          }
                          frame #1 {
                            n1111 = Bundle(cluster=w1901, "STATUS"="T-RISE PASS") -> (w1903:T4)  [unwired: 2 in]
                            n1112 = local write "RESULT LAB02-2"(TRUE) -> ()
                            n1113 = local write "DISP LAB02-2"(w1903) -> ()
                          }
                        }
                      }
                      frame False {
                      }
                    }
                  }
                }
              }
              frame #4 {
                # "LAB03-1"
                n1114 = Equal?(x=w1906, y=2) -> (x = y?=w1909:bool)
                n1115 = local read "DISP LAB03-1"() -> (w1911:T4)
                n1116 = Unbundle(w1911) -> ("STATUS"=w1912:string)  [unwired: 2 out]
                n1117 = Equal?(x=w1912, y="RUN") -> (x = y?=w1908:bool)
                n1118 = And(x=w1908, y=w1909) -> (x .and. y?=w1907:bool)
                n1119 = case shown="True" w1907 {
                  tunnel: w1911 -> [_ w1915]
                  tunnel: w1905 -> [_ w1918]
                  frame False {
                  }
                  frame True {
                    n1120 = local read "SET LAB03-1"() -> (w1917:T5)
                    n1121 = local read "TDMS LAB03-1"() -> (w1914:refnum<k34>)
                    n1122 = Unbundle(w1915) -> ("CYCLE"=w1919:dbl)  [unwired: 2 out]
                    n1123 = Unbundle(w1917) -> ("T-RISE mins"=w1916:dbl)  [unwired: 4 out]
                    n1124 = Greater Or Equal?(x=w1919, y=w1918) -> (x >= y?=w1920:bool)
                    n1125 = case shown="True" w1920 {
                      tunnel: w1916 -> [w1923 _]
                      tunnel: w1915 -> [w1922 _]
                      tunnel: w1914 -> [w1921 _]
                      frame True {
                        n1126 = stacked-sequence {
                          tunnel: w1923 -> [w1926 _]
                          tunnel: w1922 -> [_ w1931]
                          tunnel: w1921 -> [w1924 _]
                          frame #0 {
                            n1127 = Build Array("T-RISE") -> (w1928:string[])
                            n1128 = Build Array(w1926) -> (w1927:dbl[])
                            n1129 = TDMS Write(0:w1924, 5:"TEST PASS", 7:w1928, 9:w1927) -> (15:w1930:errorcluster)  [unwired: 2 in, 3 out]
                            n1130 = local write "data file error"(w1930) -> ()
                          }
                          frame #1 {
                            n1131 = Bundle(cluster=w1931, "STATUS"="T-RISE PASS") -> (w1933:T4)  [unwired: 2 in]
                            n1132 = local write "RESULT LAB03-1"(TRUE) -> ()
                            n1133 = local write "DISP LAB03-1"(w1933) -> ()
                          }
                        }
                      }
                      frame False {
                      }
                    }
                  }
                }
              }
              frame #5 {
                # "LAB03-2"
                n1134 = Equal?(x=w1936, y=2) -> (x = y?=w1939:bool)
                n1135 = local read "DISP LAB03-2"() -> (w1941:T4)
                n1136 = Unbundle(w1941) -> ("STATUS"=w1942:string)  [unwired: 2 out]
                n1137 = Equal?(x=w1942, y="RUN") -> (x = y?=w1938:bool)
                n1138 = And(x=w1938, y=w1939) -> (x .and. y?=w1937:bool)
                n1139 = case shown="True" w1937 {
                  tunnel: w1941 -> [_ w1945]
                  tunnel: w1935 -> [_ w1948]
                  frame False {
                  }
                  frame True {
                    n1140 = local read "SET LAB03-2"() -> (w1947:T5)
                    n1141 = local read "TDMS LAB03-2"() -> (w1944:refnum<k34>)
                    n1142 = Unbundle(w1945) -> ("CYCLE"=w1949:dbl)  [unwired: 2 out]
                    n1143 = Unbundle(w1947) -> ("T-RISE mins"=w1946:dbl)  [unwired: 4 out]
                    n1144 = Greater Or Equal?(x=w1949, y=w1948) -> (x >= y?=w1950:bool)
                    n1145 = case shown="True" w1950 {
                      tunnel: w1946 -> [w1953 _]
                      tunnel: w1945 -> [w1952 _]
                      tunnel: w1944 -> [w1951 _]
                      frame True {
                        n1146 = stacked-sequence {
                          tunnel: w1953 -> [w1956 _]
                          tunnel: w1952 -> [_ w1961]
                          tunnel: w1951 -> [w1954 _]
                          frame #0 {
                            n1147 = Build Array("T-RISE") -> (w1958:string[])
                            n1148 = Build Array(w1956) -> (w1957:dbl[])
                            n1149 = TDMS Write(0:w1954, 5:"TEST PASS", 7:w1958, 9:w1957) -> (15:w1960:errorcluster)  [unwired: 2 in, 3 out]
                            n1150 = local write "data file error"(w1960) -> ()
                          }
                          frame #1 {
                            n1151 = Bundle(cluster=w1961, "STATUS"="T-RISE PASS") -> (w1963:T4)  [unwired: 2 in]
                            n1152 = local write "RESULT LAB03-2"(TRUE) -> ()
                            n1153 = local write "DISP LAB03-2"(w1963) -> ()
                          }
                        }
                      }
                      frame False {
                      }
                    }
                  }
                }
              }
              frame #6 {
                # "LAB04-1"
                n1154 = Equal?(x=w1966, y=2) -> (x = y?=w1969:bool)
                n1155 = local read "DISP LAB04-1"() -> (w1971:T4)
                n1156 = Unbundle(w1971) -> ("STATUS"=w1972:string)  [unwired: 2 out]
                n1157 = Equal?(x=w1972, y="RUN") -> (x = y?=w1968:bool)
                n1158 = And(x=w1968, y=w1969) -> (x .and. y?=w1967:bool)
                n1159 = case shown="True" w1967 {
                  tunnel: w1971 -> [_ w1975]
                  tunnel: w1965 -> [_ w1978]
                  frame False {
                  }
                  frame True {
                    n1160 = local read "SET LAB04-1"() -> (w1977:T5)
                    n1161 = local read "TDMS LAB04-1"() -> (w1974:refnum<k34>)
                    n1162 = Unbundle(w1975) -> ("CYCLE"=w1979:dbl)  [unwired: 2 out]
                    n1163 = Unbundle(w1977) -> ("T-RISE mins"=w1976:dbl)  [unwired: 4 out]
                    n1164 = Greater Or Equal?(x=w1979, y=w1978) -> (x >= y?=w1980:bool)
                    n1165 = case shown="True" w1980 {
                      tunnel: w1976 -> [w1983 _]
                      tunnel: w1975 -> [w1982 _]
                      tunnel: w1974 -> [w1981 _]
                      frame True {
                        n1166 = stacked-sequence {
                          tunnel: w1983 -> [w1986 _]
                          tunnel: w1982 -> [_ w1991]
                          tunnel: w1981 -> [w1984 _]
                          frame #0 {
                            n1167 = Build Array("T-RISE") -> (w1988:string[])
                            n1168 = Build Array(w1986) -> (w1987:dbl[])
                            n1169 = TDMS Write(0:w1984, 5:"TEST PASS", 7:w1988, 9:w1987) -> (15:w1990:errorcluster)  [unwired: 2 in, 3 out]
                            n1170 = local write "data file error"(w1990) -> ()
                          }
                          frame #1 {
                            n1171 = Bundle(cluster=w1991, "STATUS"="T-RISE PASS") -> (w1993:T4)  [unwired: 2 in]
                            n1172 = local write "RESULT LAB04-1"(TRUE) -> ()
                            n1173 = local write "DISP LAB04-1"(w1993) -> ()
                          }
                        }
                      }
                      frame False {
                      }
                    }
                  }
                }
              }
              frame #7 {
                # "LAB04-2"
                n1174 = Equal?(x=w1996, y=2) -> (x = y?=w1999:bool)
                n1175 = local read "DISP LAB04-2"() -> (w2001:T4)
                n1176 = Unbundle(w2001) -> ("STATUS"=w2002:string)  [unwired: 2 out]
                n1177 = Equal?(x=w2002, y="RUN") -> (x = y?=w1998:bool)
                n1178 = And(x=w1998, y=w1999) -> (x .and. y?=w1997:bool)
                n1179 = case shown="True" w1997 {
                  tunnel: w2001 -> [_ w2005]
                  tunnel: w1995 -> [_ w2008]
                  frame False {
                  }
                  frame True {
                    n1180 = local read "SET LAB04-2"() -> (w2007:T5)
                    n1181 = local read "TDMS LAB04-2"() -> (w2004:refnum<k34>)
                    n1182 = Unbundle(w2005) -> ("CYCLE"=w2009:dbl)  [unwired: 2 out]
                    n1183 = Unbundle(w2007) -> ("T-RISE mins"=w2006:dbl)  [unwired: 4 out]
                    n1184 = Greater Or Equal?(x=w2009, y=w2008) -> (x >= y?=w2010:bool)
                    n1185 = case shown="True" w2010 {
                      tunnel: w2006 -> [w2013 _]
                      tunnel: w2005 -> [w2012 _]
                      tunnel: w2004 -> [w2011 _]
                      frame True {
                        n1186 = stacked-sequence {
                          tunnel: w2013 -> [w2016 _]
                          tunnel: w2012 -> [_ w2021]
                          tunnel: w2011 -> [w2014 _]
                          frame #0 {
                            n1187 = Build Array("T-RISE") -> (w2018:string[])
                            n1188 = Build Array(w2016) -> (w2017:dbl[])
                            n1189 = TDMS Write(0:w2014, 5:"TEST PASS", 7:w2018, 9:w2017) -> (15:w2020:errorcluster)  [unwired: 2 in, 3 out]
                            n1190 = local write "data file error"(w2020) -> ()
                          }
                          frame #1 {
                            n1191 = Bundle(cluster=w2021, "STATUS"="T-RISE PASS") -> (w2023:T4)  [unwired: 2 in]
                            n1192 = local write "RESULT LAB04-2"(TRUE) -> ()
                            n1193 = local write "DISP LAB04-2"(w2023) -> ()
                          }
                        }
                      }
                      frame False {
                      }
                    }
                  }
                }
              }
              frame #8 {
                # "LAB05-1"
                n1194 = Equal?(x=w2026, y=2) -> (x = y?=w2029:bool)
                n1195 = local read "DISP LAB05-1"() -> (w2031:T4)
                n1196 = Unbundle(w2031) -> ("STATUS"=w2032:string)  [unwired: 2 out]
                n1197 = Equal?(x=w2032, y="RUN") -> (x = y?=w2028:bool)
                n1198 = And(x=w2028, y=w2029) -> (x .and. y?=w2027:bool)
                n1199 = case shown="True" w2027 {
                  tunnel: w2031 -> [_ w2035]
                  tunnel: w2025 -> [_ w2038]
                  frame False {
                  }
                  frame True {
                    n1200 = local read "SET LAB05-1"() -> (w2037:T5)
                    n1201 = local read "TDMS LAB05-1"() -> (w2034:refnum<k34>)
                    n1202 = Unbundle(w2035) -> ("CYCLE"=w2039:dbl)  [unwired: 2 out]
                    n1203 = Unbundle(w2037) -> ("T-RISE mins"=w2036:dbl)  [unwired: 4 out]
                    n1204 = Greater Or Equal?(x=w2039, y=w2038) -> (x >= y?=w2040:bool)
                    n1205 = case shown="True" w2040 {
                      tunnel: w2036 -> [w2043 _]
                      tunnel: w2035 -> [w2042 _]
                      tunnel: w2034 -> [w2041 _]
                      frame True {
                        n1206 = stacked-sequence {
                          tunnel: w2043 -> [w2046 _]
                          tunnel: w2042 -> [_ w2051]
                          tunnel: w2041 -> [w2044 _]
                          frame #0 {
                            n1207 = Build Array("T-RISE") -> (w2048:string[])
                            n1208 = Build Array(w2046) -> (w2047:dbl[])
                            n1209 = TDMS Write(0:w2044, 5:"TEST PASS", 7:w2048, 9:w2047) -> (15:w2050:errorcluster)  [unwired: 2 in, 3 out]
                            n1210 = local write "data file error"(w2050) -> ()
                          }
                          frame #1 {
                            n1211 = Bundle(cluster=w2051, "STATUS"="T-RISE PASS") -> (w2053:T4)  [unwired: 2 in]
                            n1212 = local write "RESULT LAB05-1"(TRUE) -> ()
                            n1213 = local write "DISP LAB05-1"(w2053) -> ()
                          }
                        }
                      }
                      frame False {
                      }
                    }
                  }
                }
              }
              frame #9 {
                # "LAB05-2"
                n1214 = Equal?(x=w2056, y=2) -> (x = y?=w2059:bool)
                n1215 = local read "DISP LAB05-2"() -> (w2061:T4)
                n1216 = Unbundle(w2061) -> ("STATUS"=w2062:string)  [unwired: 2 out]
                n1217 = Equal?(x=w2062, y="RUN") -> (x = y?=w2058:bool)
                n1218 = And(x=w2058, y=w2059) -> (x .and. y?=w2057:bool)
                n1219 = case shown="True" w2057 {
                  tunnel: w2061 -> [_ w2065]
                  tunnel: w2055 -> [_ w2068]
                  frame False {
                  }
                  frame True {
                    n1220 = local read "SET LAB05-2"() -> (w2067:T5)
                    n1221 = local read "TDMS LAB05-2"() -> (w2064:refnum<k34>)
                    n1222 = Unbundle(w2065) -> ("CYCLE"=w2069:dbl)  [unwired: 2 out]
                    n1223 = Unbundle(w2067) -> ("T-RISE mins"=w2066:dbl)  [unwired: 4 out]
                    n1224 = Greater Or Equal?(x=w2069, y=w2068) -> (x >= y?=w2070:bool)
                    n1225 = case shown="True" w2070 {
                      tunnel: w2066 -> [w2073 _]
                      tunnel: w2065 -> [w2072 _]
                      tunnel: w2064 -> [w2071 _]
                      frame True {
                        n1226 = stacked-sequence {
                          tunnel: w2073 -> [w2076 _]
                          tunnel: w2072 -> [_ w2081]
                          tunnel: w2071 -> [w2074 _]
                          frame #0 {
                            n1227 = Build Array("T-RISE") -> (w2078:string[])
                            n1228 = Build Array(w2076) -> (w2077:dbl[])
                            n1229 = TDMS Write(0:w2074, 5:"TEST PASS", 7:w2078, 9:w2077) -> (15:w2080:errorcluster)  [unwired: 2 in, 3 out]
                            n1230 = local write "data file error"(w2080) -> ()
                          }
                          frame #1 {
                            n1231 = Bundle(cluster=w2081, "STATUS"="T-RISE PASS") -> (w2083:T4)  [unwired: 2 in]
                            n1232 = local write "RESULT LAB05-2"(TRUE) -> ()
                            n1233 = local write "DISP LAB05-2"(w2083) -> ()
                          }
                        }
                      }
                      frame False {
                      }
                    }
                  }
                }
              }
            }
          }
          frame #6 {
            # "end test & close test files"
            n1234 = stacked-sequence {
              tunnel: w2094 -> [_ _ _ _ _ _ _ _ _ _]
              tunnel: w2095 -> [_ _ _ _ _ _ _ _ _ _]
              tunnel: w2093 -> [_ _ _ _ _ _ _ _ _ _]
              tunnel: w2092 -> [_ _ _ _ _ _ _ _ _ _]
              tunnel: w2091 -> [_ _ _ _ _ _ _ _ _ _]
              tunnel: w2090 -> [_ _ _ _ _ _ _ _ _ _]
              tunnel: w2089 -> [_ _ _ _ _ _ _ _ _ _]
              tunnel: w2088 -> [_ _ _ _ _ _ _ _ _ _]
              tunnel: w2087 -> [_ _ _ _ _ _ _ _ _ _]
              tunnel: w2086 -> [_ _ _ _ _ _ _ _ _ _]
              frame #0 {
                # "LAB01-1"
                n1235 = local read "DISP LAB01-1"() -> (w2099:T4)
                n1236 = local read "run lab01-1"() -> (w2096:bool)
                n1237 = local read "TDMS LAB01-1"() -> (w2097:refnum<k34>)
                n1238 = Unbundle(w2099) -> ("CYCLE"=w2100:dbl, "STATUS"=w2098:string)  [unwired: 1 out]
                n1239 = case shown="True" w2096 {
                  tunnel: w2100 -> [_ w2104]
                  tunnel: w2099 -> [_ w2103]
                  tunnel: w2098 -> [_ w2102]
                  tunnel: w2097 -> [_ w2101]
                  frame False {
                  }
                  frame True {
                    n1240 = Not Equal?(x=w2102, y="RUN") -> (x != y?=w2105:bool)
                    n1241 = Greater?(x=w2104, y=2.0) -> (0:w2107:bool)
                    n1242 = And(x=w2107, y=w2105) -> (x .and. y?=w2106:bool)
                    n1243 = case shown="True" w2106 {
                      tunnel: w2103 -> [_ w2111]
                      tunnel: w2101 -> [_ w2110]
                      frame False {
                      }
                      frame True {
                        n1244 = stacked-sequence {
                          tunnel: w2111 -> [w2115 _ _]
                          tunnel: w2110 -> [_ w2117 _]
                          frame #0 {
                            w2112 = FALSE
                            n1245 = local write "mail control"("END") -> ()
                            n1246 = Bundle(cluster=w2115) -> (w2114:T4)  [unwired: 3 in]
                            n1247 = local write "DISP LAB01-1"(w2114) -> ()
                            n1248 = local write "O/I  LAB01-1"(w2112) -> ()
                            n1249 = local write "run lab01-1"(w2112) -> ()
                            n1250 = local write "RUN LAB01-1"(w2112) -> ()
                          }
                          frame #1 {
                            n1251 = TDMS Close(11:w2117) -> (0:w2116:errorcluster)  [unwired: 1 in, 1 out]
                            n1252 = local write "data file error"(w2116) -> ()
                          }
                          frame #2 {
                            n1253 = stacked-sequence {
                              tunnel: "LAB01-1" -> [w2120 w2122]
                              frame #0 {
                                n1254 = call "sub vi - defrag tdms v1.vi"("panel id"=w2120) -> ("error out"=w2119:errorcluster)  [unwired: 10 in]
                                n1255 = local write "data file error"(w2119) -> ()
                              }
                              frame #1 {
                                n1256 = call "Save data file to network drive v1.vi"("panel id"=w2122) -> ("network file save error"=w2121:errorcluster)  [unwired: 9 in, 1 out]
                                n1257 = local write "data file error"(w2121) -> ()
                              }
                            }
                          }
                        }
                      }
                    }
                  }
                }
              }
              frame #1 {
                # "LAB01-2"
                n1258 = local read "run lab01-2"() -> (w2123:bool)
                n1259 = case shown="True" w2123 {
                  frame False {
                  }
                  frame True {
                    n1260 = local read "DISP LAB01-2"() -> (w2130:T4)
                    n1261 = local read "TDMS LAB01-2"() -> (w2129:refnum<k34>)
                    n1262 = Unbundle(w2130) -> ("CYCLE"=w2126:dbl, "STATUS"=w2131:string)  [unwired: 1 out]
                    n1263 = Not Equal?(x=w2131, y="RUN") -> (x != y?=w2125:bool)
                    n1264 = Greater?(x=w2126, y=2.0) -> (0:w2127:bool)
                    n1265 = And(x=w2127, y=w2125) -> (x .and. y?=w2124:bool)
                    n1266 = case shown="True" w2124 {
                      tunnel: w2130 -> [_ w2134]
                      tunnel: w2129 -> [_ w2133]
                      frame False {
                      }
                      frame True {
                        n1267 = stacked-sequence {
                          tunnel: w2134 -> [w2137 _ _]
                          tunnel: w2133 -> [_ w2139 _]
                          frame #0 {
                            w2135 = FALSE
                            n1268 = local write "mail control"("END") -> ()
                            n1269 = Bundle(cluster=w2137) -> (w2138:T4)  [unwired: 3 in]
                            n1270 = local write "RUN LAB01-2"(w2135) -> ()
                            n1271 = local write "run lab01-2"(w2135) -> ()
                            n1272 = local write "O/I  LAB01-2"(w2135) -> ()
                            n1273 = local write "DISP LAB01-2"(w2138) -> ()
                          }
                          frame #1 {
                            n1274 = TDMS Close(11:w2139) -> (0:w2140:errorcluster)  [unwired: 1 in, 1 out]
                            n1275 = local write "data file error"(w2140) -> ()
                          }
                          frame #2 {
                            n1276 = stacked-sequence {
                              tunnel: "LAB01-2" -> [w2143 w2145]
                              frame #0 {
                                n1277 = call "sub vi - defrag tdms v1.vi"("panel id"=w2143) -> ("error out"=w2142:errorcluster)  [unwired: 10 in]
                                n1278 = local write "data file error"(w2142) -> ()
                              }
                              frame #1 {
                                n1279 = call "Save data file to network drive v1.vi"("panel id"=w2145) -> ("network file save error"=w2144:errorcluster)  [unwired: 9 in, 1 out]
                                n1280 = local write "data file error"(w2144) -> ()
                              }
                            }
                          }
                        }
                      }
                    }
                  }
                }
              }
              frame #2 {
                # "LAB02-1"
                n1281 = local read "run lab02-1"() -> (w2146:bool)
                n1282 = case shown="True" w2146 {
                  frame False {
                  }
                  frame True {
                    n1283 = local read "DISP LAB02-1"() -> (w2153:T4)
                    n1284 = Unbundle(w2153) -> ("CYCLE"=w2149:dbl, "STATUS"=w2154:string)  [unwired: 1 out]
                    n1285 = local read "TDMS LAB02-1"() -> (w2152:refnum<k34>)
                    n1286 = Not Equal?(x=w2154, y="RUN") -> (x != y?=w2148:bool)
                    n1287 = Greater?(x=w2149, y=2.0) -> (0:w2150:bool)
                    n1288 = And(x=w2150, y=w2148) -> (x .and. y?=w2147:bool)
                    n1289 = case shown="True" w2147 {
                      tunnel: w2153 -> [_ w2157]
                      tunnel: w2152 -> [_ w2156]
                      frame False {
                      }
                      frame True {
                        n1290 = stacked-sequence {
                          tunnel: w2157 -> [w2160 _ _]
                          tunnel: w2156 -> [_ w2162 _]
                          frame #0 {
                            w2158 = FALSE
                            n1291 = local write "mail control"("END") -> ()
                            n1292 = Bundle(cluster=w2160) -> (w2161:T4)  [unwired: 3 in]
                            n1293 = local write "O/I  LAB02-1"(w2158) -> ()
                            n1294 = local write "RUN LAB02-1"(w2158) -> ()
                            n1295 = local write "run lab02-1"(w2158) -> ()
                            n1296 = local write "DISP LAB02-1"(w2161) -> ()
                          }
                          frame #1 {
                            n1297 = TDMS Close(11:w2162) -> (0:w2163:errorcluster)  [unwired: 1 in, 1 out]
                            n1298 = local write "data file error"(w2163) -> ()
                          }
                          frame #2 {
                            n1299 = stacked-sequence {
                              tunnel: "LAB02-1" -> [w2166 w2168]
                              frame #0 {
                                n1300 = call "sub vi - defrag tdms v1.vi"("panel id"=w2166) -> ("error out"=w2165:errorcluster)  [unwired: 10 in]
                                n1301 = local write "data file error"(w2165) -> ()
                              }
                              frame #1 {
                                n1302 = call "Save data file to network drive v1.vi"("panel id"=w2168) -> ("network file save error"=w2167:errorcluster)  [unwired: 9 in, 1 out]
                                n1303 = local write "data file error"(w2167) -> ()
                              }
                            }
                          }
                        }
                      }
                    }
                  }
                }
              }
              frame #3 {
                # "LAB02-2"
                n1304 = local read "run lab02-2"() -> (w2169:bool)
                n1305 = case shown="True" w2169 {
                  frame False {
                  }
                  frame True {
                    n1306 = local read "DISP LAB02-2"() -> (w2176:T4)
                    n1307 = local read "TDMS LAB02-2"() -> (w2175:refnum<k34>)
                    n1308 = Unbundle(w2176) -> ("CYCLE"=w2172:dbl, "STATUS"=w2177:string)  [unwired: 1 out]
                    n1309 = Not Equal?(x=w2177, y="RUN") -> (x != y?=w2171:bool)
                    n1310 = Greater?(x=w2172, y=2.0) -> (0:w2173:bool)
                    n1311 = And(x=w2173, y=w2171) -> (x .and. y?=w2170:bool)
                    n1312 = case shown="True" w2170 {
                      tunnel: w2176 -> [_ w2180]
                      tunnel: w2175 -> [_ w2179]
                      frame False {
                      }
                      frame True {
                        n1313 = stacked-sequence {
                          tunnel: w2180 -> [w2183 _ _]
                          tunnel: w2179 -> [_ w2185 _]
                          frame #0 {
                            w2181 = FALSE
                            n1314 = local write "mail control"("END") -> ()
                            n1315 = Bundle(cluster=w2183) -> (w2184:T4)  [unwired: 3 in]
                            n1316 = local write "O/I  LAB02-2"(w2181) -> ()
                            n1317 = local write "run lab02-2"(w2181) -> ()
                            n1318 = local write "RUN LAB02-2"(w2181) -> ()
                            n1319 = local write "DISP LAB02-2"(w2184) -> ()
                          }
                          frame #1 {
                            n1320 = TDMS Close(11:w2185) -> (0:w2186:errorcluster)  [unwired: 1 in, 1 out]
                            n1321 = local write "data file error"(w2186) -> ()
                          }
                          frame #2 {
                            n1322 = stacked-sequence {
                              tunnel: "LAB02-2" -> [w2189 w2191]
                              frame #0 {
                                n1323 = call "sub vi - defrag tdms v1.vi"("panel id"=w2189) -> ("error out"=w2188:errorcluster)  [unwired: 10 in]
                                n1324 = local write "data file error"(w2188) -> ()
                              }
                              frame #1 {
                                n1325 = call "Save data file to network drive v1.vi"("panel id"=w2191) -> ("network file save error"=w2190:errorcluster)  [unwired: 9 in, 1 out]
                                n1326 = local write "data file error"(w2190) -> ()
                              }
                            }
                          }
                        }
                      }
                    }
                  }
                }
              }
              frame #4 {
                # "LAB03-1"
                n1327 = local read "run lab03-1"() -> (w2192:bool)
                n1328 = case shown="True" w2192 {
                  frame False {
                  }
                  frame True {
                    n1329 = local read "DISP LAB03-1"() -> (w2199:T4)
                    n1330 = local read "TDMS LAB03-1"() -> (w2198:refnum<k34>)
                    n1331 = Unbundle(w2199) -> ("CYCLE"=w2195:dbl, "STATUS"=w2200:string)  [unwired: 1 out]
                    n1332 = Not Equal?(x=w2200, y="RUN") -> (x != y?=w2194:bool)
                    n1333 = Greater?(x=w2195, y=2.0) -> (0:w2196:bool)
                    n1334 = And(x=w2196, y=w2194) -> (x .and. y?=w2193:bool)
                    n1335 = case shown="True" w2193 {
                      tunnel: w2199 -> [_ w2203]
                      tunnel: w2198 -> [_ w2202]
                      frame False {
                      }
                      frame True {
                        n1336 = stacked-sequence {
                          tunnel: w2203 -> [w2206 _ _]
                          tunnel: w2202 -> [_ w2208 _]
                          frame #0 {
                            w2204 = FALSE
                            n1337 = local write "mail control"("END") -> ()
                            n1338 = Bundle(cluster=w2206) -> (w2207:T4)  [unwired: 3 in]
                            n1339 = local write "O/I  LAB03-1"(w2204) -> ()
                            n1340 = local write "run lab03-1"(w2204) -> ()
                            n1341 = local write "RUN LAB03-1"(w2204) -> ()
                            n1342 = local write "DISP LAB03-1"(w2207) -> ()
                          }
                          frame #1 {
                            n1343 = TDMS Close(11:w2208) -> (0:w2209:errorcluster)  [unwired: 1 in, 1 out]
                            n1344 = local write "data file error"(w2209) -> ()
                          }
                          frame #2 {
                            n1345 = stacked-sequence {
                              tunnel: "LAB03-1" -> [w2212 w2214]
                              frame #0 {
                                n1346 = call "sub vi - defrag tdms v1.vi"("panel id"=w2212) -> ("error out"=w2211:errorcluster)  [unwired: 10 in]
                                n1347 = local write "data file error"(w2211) -> ()
                              }
                              frame #1 {
                                n1348 = call "Save data file to network drive v1.vi"("panel id"=w2214) -> ("network file save error"=w2213:errorcluster)  [unwired: 9 in, 1 out]
                                n1349 = local write "data file error"(w2213) -> ()
                              }
                            }
                          }
                        }
                      }
                    }
                  }
                }
              }
              frame #5 {
                # "LAB03-2"
                n1350 = local read "run lab03-2"() -> (w2215:bool)
                n1351 = case shown="True" w2215 {
                  frame False {
                  }
                  frame True {
                    n1352 = local read "DISP LAB03-2"() -> (w2222:T4)
                    n1353 = Unbundle(w2222) -> ("CYCLE"=w2218:dbl, "STATUS"=w2223:string)  [unwired: 1 out]
                    n1354 = local read "TDMS LAB03-2"() -> (w2221:refnum<k34>)
                    n1355 = Not Equal?(x=w2223, y="RUN") -> (x != y?=w2217:bool)
                    n1356 = Greater?(x=w2218, y=2.0) -> (0:w2219:bool)
                    n1357 = And(x=w2219, y=w2217) -> (x .and. y?=w2216:bool)
                    n1358 = case shown="True" w2216 {
                      tunnel: w2222 -> [_ w2226]
                      tunnel: w2221 -> [_ w2225]
                      frame False {
                      }
                      frame True {
                        n1359 = stacked-sequence {
                          tunnel: w2226 -> [w2229 _ _]
                          tunnel: w2225 -> [_ w2231 _]
                          frame #0 {
                            w2227 = FALSE
                            n1360 = local write "mail control"("END") -> ()
                            n1361 = Bundle(cluster=w2229) -> (w2230:T4)  [unwired: 3 in]
                            n1362 = local write "RUN LAB03-2"(w2227) -> ()
                            n1363 = local write "O/I  LAB03-2"(w2227) -> ()
                            n1364 = local write "DISP LAB03-2"(w2230) -> ()
                            n1365 = local write "run lab03-2"(w2227) -> ()
                          }
                          frame #1 {
                            n1366 = TDMS Close(11:w2231) -> (0:w2232:errorcluster)  [unwired: 1 in, 1 out]
                            n1367 = local write "data file error"(w2232) -> ()
                          }
                          frame #2 {
                            n1368 = stacked-sequence {
                              tunnel: "LAB03-2" -> [w2235 w2237]
                              frame #0 {
                                n1369 = call "sub vi - defrag tdms v1.vi"("panel id"=w2235) -> ("error out"=w2234:errorcluster)  [unwired: 10 in]
                                n1370 = local write "data file error"(w2234) -> ()
                              }
                              frame #1 {
                                n1371 = call "Save data file to network drive v1.vi"("panel id"=w2237) -> ("network file save error"=w2236:errorcluster)  [unwired: 9 in, 1 out]
                                n1372 = local write "data file error"(w2236) -> ()
                              }
                            }
                          }
                        }
                      }
                    }
                  }
                }
              }
              frame #6 {
                # "LAB04-1"
                n1373 = local read "run lab04-1"() -> (w2238:bool)
                n1374 = case shown="True" w2238 {
                  frame False {
                  }
                  frame True {
                    n1375 = local read "DISP LAB04-1"() -> (w2245:T4)
                    n1376 = Unbundle(w2245) -> ("CYCLE"=w2241:dbl, "STATUS"=w2246:string)  [unwired: 1 out]
                    n1377 = local read "TDMS LAB04-1"() -> (w2244:refnum<k34>)
                    n1378 = Not Equal?(x=w2246, y="RUN") -> (x != y?=w2240:bool)
                    n1379 = Greater?(x=w2241, y=2.0) -> (0:w2242:bool)
                    n1380 = And(x=w2242, y=w2240) -> (x .and. y?=w2239:bool)
                    n1381 = case shown="True" w2239 {
                      tunnel: w2245 -> [_ w2249]
                      tunnel: w2244 -> [_ w2248]
                      frame False {
                      }
                      frame True {
                        n1382 = stacked-sequence {
                          tunnel: w2249 -> [w2252 _ _]
                          tunnel: w2248 -> [_ w2254 _]
                          frame #0 {
                            w2250 = FALSE
                            n1383 = local write "mail control"("END") -> ()
                            n1384 = Bundle(cluster=w2252) -> (w2253:T4)  [unwired: 3 in]
                            n1385 = local write "RUN LAB04-1"(w2250) -> ()
                            n1386 = local write "O/I  LAB04-1"(w2250) -> ()
                            n1387 = local write "run lab04-1"(w2250) -> ()
                            n1388 = local write "DISP LAB04-1"(w2253) -> ()
                          }
                          frame #1 {
                            n1389 = TDMS Close(11:w2254) -> (0:w2255:errorcluster)  [unwired: 1 in, 1 out]
                            n1390 = local write "data file error"(w2255) -> ()
                          }
                          frame #2 {
                            n1391 = stacked-sequence {
                              tunnel: "LAB04-1" -> [w2258 w2260]
                              frame #0 {
                                n1392 = call "sub vi - defrag tdms v1.vi"("panel id"=w2258) -> ("error out"=w2257:errorcluster)  [unwired: 10 in]
                                n1393 = local write "data file error"(w2257) -> ()
                              }
                              frame #1 {
                                n1394 = call "Save data file to network drive v1.vi"("panel id"=w2260) -> ("network file save error"=w2259:errorcluster)  [unwired: 9 in, 1 out]
                                n1395 = local write "data file error"(w2259) -> ()
                              }
                            }
                          }
                        }
                      }
                    }
                  }
                }
              }
              frame #7 {
                # "LAB04-2"
                n1396 = local read "run lab04-2"() -> (w2261:bool)
                n1397 = case shown="True" w2261 {
                  frame False {
                  }
                  frame True {
                    n1398 = local read "DISP LAB04-2"() -> (w2268:T4)
                    n1399 = Unbundle(w2268) -> ("CYCLE"=w2264:dbl, "STATUS"=w2269:string)  [unwired: 1 out]
                    n1400 = Not Equal?(x=w2269, y="RUN") -> (x != y?=w2263:bool)
                    n1401 = local read "TDMS LAB04-2"() -> (w2267:refnum<k34>)
                    n1402 = Greater?(x=w2264, y=2.0) -> (0:w2265:bool)
                    n1403 = And(x=w2265, y=w2263) -> (x .and. y?=w2262:bool)
                    n1404 = case shown="True" w2262 {
                      tunnel: w2268 -> [_ w2272]
                      tunnel: w2267 -> [_ w2271]
                      frame False {
                      }
                      frame True {
                        n1405 = stacked-sequence {
                          tunnel: w2272 -> [w2275 _ _]
                          tunnel: w2271 -> [_ w2277 _]
                          frame #0 {
                            w2273 = FALSE
                            n1406 = local write "mail control"("END") -> ()
                            n1407 = Bundle(cluster=w2275) -> (w2276:T4)  [unwired: 3 in]
                            n1408 = local write "O/I  LAB04-2"(w2273) -> ()
                            n1409 = local write "RUN LAB04-2"(w2273) -> ()
                            n1410 = local write "run lab04-2"(w2273) -> ()
                            n1411 = local write "DISP LAB04-2"(w2276) -> ()
                          }
                          frame #1 {
                            n1412 = TDMS Close(11:w2277) -> (0:w2278:errorcluster)  [unwired: 1 in, 1 out]
                            n1413 = local write "data file error"(w2278) -> ()
                          }
                          frame #2 {
                            n1414 = stacked-sequence {
                              tunnel: "LAB04-2" -> [w2281 w2283]
                              frame #0 {
                                n1415 = call "sub vi - defrag tdms v1.vi"("panel id"=w2281) -> ("error out"=w2280:errorcluster)  [unwired: 10 in]
                                n1416 = local write "data file error"(w2280) -> ()
                              }
                              frame #1 {
                                n1417 = call "Save data file to network drive v1.vi"("panel id"=w2283) -> ("network file save error"=w2282:errorcluster)  [unwired: 9 in, 1 out]
                                n1418 = local write "data file error"(w2282) -> ()
                              }
                            }
                          }
                        }
                      }
                    }
                  }
                }
              }
              frame #8 {
                # "LAB05-1"
                n1419 = local read "run lab05-1"() -> (w2284:bool)
                n1420 = case shown="True" w2284 {
                  frame False {
                  }
                  frame True {
                    n1421 = local read "DISP LAB05-1"() -> (w2291:T4)
                    n1422 = Unbundle(w2291) -> ("CYCLE"=w2287:dbl, "STATUS"=w2292:string)  [unwired: 1 out]
                    n1423 = Not Equal?(x=w2292, y="RUN") -> (x != y?=w2286:bool)
                    n1424 = local read "TDMS LAB05-1"() -> (w2290:refnum<k34>)
                    n1425 = Greater?(x=w2287, y=2.0) -> (0:w2288:bool)
                    n1426 = And(x=w2288, y=w2286) -> (x .and. y?=w2285:bool)
                    n1427 = case shown="True" w2285 {
                      tunnel: w2291 -> [_ w2295]
                      tunnel: w2290 -> [_ w2294]
                      frame False {
                      }
                      frame True {
                        n1428 = stacked-sequence {
                          tunnel: w2295 -> [w2298 _ _]
                          tunnel: w2294 -> [_ w2300 _]
                          frame #0 {
                            w2296 = FALSE
                            n1429 = local write "mail control"("END") -> ()
                            n1430 = Bundle(cluster=w2298) -> (w2299:T4)  [unwired: 3 in]
                            n1431 = local write "O/I  LAB05-1"(w2296) -> ()
                            n1432 = local write "RUN LAB05-1"(w2296) -> ()
                            n1433 = local write "run lab05-1"(w2296) -> ()
                            n1434 = local write "DISP LAB05-1"(w2299) -> ()
                          }
                          frame #1 {
                            n1435 = TDMS Close(11:w2300) -> (0:w2301:errorcluster)  [unwired: 1 in, 1 out]
                            n1436 = local write "data file error"(w2301) -> ()
                          }
                          frame #2 {
                            n1437 = stacked-sequence {
                              tunnel: "LAB05-1" -> [w2304 w2306]
                              frame #0 {
                                n1438 = call "sub vi - defrag tdms v1.vi"("panel id"=w2304) -> ("error out"=w2303:errorcluster)  [unwired: 10 in]
                                n1439 = local write "data file error"(w2303) -> ()
                              }
                              frame #1 {
                                n1440 = call "Save data file to network drive v1.vi"("panel id"=w2306) -> ("network file save error"=w2305:errorcluster)  [unwired: 9 in, 1 out]
                                n1441 = local write "data file error"(w2305) -> ()
                              }
                            }
                          }
                        }
                      }
                    }
                  }
                }
              }
              frame #9 {
                # "LAB05-2"
                n1442 = local read "run lab05-2"() -> (w2307:bool)
                n1443 = case shown="True" w2307 {
                  frame False {
                  }
                  frame True {
                    n1444 = local read "DISP LAB05-2"() -> (w2314:T4)
                    n1445 = Unbundle(w2314) -> ("CYCLE"=w2310:dbl, "STATUS"=w2315:string)  [unwired: 1 out]
                    n1446 = Not Equal?(x=w2315, y="RUN") -> (x != y?=w2309:bool)
                    n1447 = local read "TDMS LAB05-2"() -> (w2313:refnum<k34>)
                    n1448 = Greater?(x=w2310, y=2.0) -> (0:w2311:bool)
                    n1449 = And(x=w2311, y=w2309) -> (x .and. y?=w2308:bool)
                    n1450 = case shown="True" w2308 {
                      tunnel: w2314 -> [_ w2318]
                      tunnel: w2313 -> [_ w2317]
                      frame False {
                      }
                      frame True {
                        n1451 = stacked-sequence {
                          tunnel: w2318 -> [w2321 _ _]
                          tunnel: w2317 -> [_ w2323 _]
                          frame #0 {
                            w2319 = FALSE
                            n1452 = local write "mail control"("END") -> ()
                            n1453 = Bundle(cluster=w2321) -> (w2322:T4)  [unwired: 3 in]
                            n1454 = local write "RUN LAB05-2"(w2319) -> ()
                            n1455 = local write "O/I  LAB05-2"(w2319) -> ()
                            n1456 = local write "run lab05-2"(w2319) -> ()
                            n1457 = local write "DISP LAB05-2"(w2322) -> ()
                          }
                          frame #1 {
                            n1458 = TDMS Close(11:w2323) -> (0:w2324:errorcluster)  [unwired: 1 in, 1 out]
                            n1459 = local write "data file error"(w2324) -> ()
                          }
                          frame #2 {
                            n1460 = stacked-sequence {
                              tunnel: "LAB05-2" -> [w2327 w2329]
                              frame #0 {
                                n1461 = call "sub vi - defrag tdms v1.vi"("panel id"=w2327) -> ("error out"=w2326:errorcluster)  [unwired: 10 in]
                                n1462 = local write "data file error"(w2326) -> ()
                              }
                              frame #1 {
                                n1463 = call "Save data file to network drive v1.vi"("panel id"=w2329) -> ("network file save error"=w2328:errorcluster)  [unwired: 9 in, 1 out]
                                n1464 = local write "data file error"(w2328) -> ()
                              }
                            }
                          }
                        }
                      }
                    }
                  }
                }
              }
            }
            n1465 = local read "Network Directory"() -> (w2085:path)
            n1466 = global write "Global 1.vi" "Network Drive"(w2085) -> ()
          }
          frame #7 {
            # "disable functions"
            n1467 = stacked-sequence {
              tunnel: w2339 -> [w2353 _ w2409]
              tunnel: w2338 -> [w2348 _ w2408]
              tunnel: w2337 -> [w2347 _ w2407]
              tunnel: w2336 -> [w2345 _ w2406]
              tunnel: w2335 -> [w2346 _ w2405]
              tunnel: w2334 -> [_ w2370 w2404]
              tunnel: w2333 -> [_ w2371 w2403]
              tunnel: w2332 -> [_ w2372 w2402]
              tunnel: w2331 -> [_ w2373 w2401]
              tunnel: w2330 -> [_ w2374 w2400]
              frame #0 {
                n1468 = Select(t=2, s=w2345, f=0) -> (s? t:f=w2341:i32)
                n1469 = Select(t=2, s=w2347, f=0) -> (s? t:f=w2342:i32)
                n1470 = Select(t=2, s=w2346, f=0) -> (s? t:f=w2340:i32)
                n1471 = Select(t=2, s=w2353, f=0) -> (s? t:f=w2344:i32)
                n1472 = Select(t=2, s=w2348, f=0) -> (s? t:f=w2343:i32)
                n1473 = property on="SELECT LAB02-2" class="RadioBtnsControl (strict)"("DisabledEnum"=w2341) -> ()  [unwired: 2 in, 2 out]
                n1474 = property on="SELECT LAB02-1" class="RadioBtnsControl (strict)"("DisabledEnum"=w2342) -> ()  [unwired: 2 in, 2 out]
                n1475 = property on="SELECT LAB03-1" class="RadioBtnsControl (strict)"("DisabledEnum"=w2340) -> ()  [unwired: 2 in, 2 out]
                n1476 = property on="SELECT LAB01-1" class="RadioBtnsControl (strict)"("DisabledEnum"=w2344) -> ()  [unwired: 2 in, 2 out]
                n1477 = property on="SELECT LAB01-2" class="RadioBtnsControl (strict)"("DisabledEnum"=w2343) -> ()  [unwired: 2 in, 2 out]
                n1478 = Not(x=w2353) -> (.not. x?=w2354:bool)
                n1479 = property on="RESULT LAB01-1" class="Bool (strict)"("Visible"=w2354) -> ()  [unwired: 2 in, 2 out]
                n1480 = Not(x=w2348) -> (.not. x?=w2352:bool)
                n1481 = Not(x=w2347) -> (.not. x?=w2351:bool)
                n1482 = Not(x=w2345) -> (.not. x?=w2350:bool)
                n1483 = property on="RESULT LAB01-2" class="Bool (strict)"("Visible"=w2352) -> ()  [unwired: 2 in, 2 out]
                n1484 = Not(x=w2346) -> (.not. x?=w2349:bool)
                n1485 = property on="RESULT LAB02-1" class="Bool (strict)"("Visible"=w2351) -> ()  [unwired: 2 in, 2 out]
                n1486 = property on="RESULT LAB02-2" class="Bool (strict)"("Visible"=w2350) -> ()  [unwired: 2 in, 2 out]
                n1487 = property on="RESULT LAB03-1" class="Bool (strict)"("Visible"=w2349) -> ()  [unwired: 2 in, 2 out]
                n1488 = property on="SET LAB01-1" class="Clust (strict)"("DisabledEnum"=w2344) -> ()  [unwired: 2 in, 2 out]
                n1489 = property on="SET LAB01-2" class="Clust (strict)"("DisabledEnum"=w2343) -> ()  [unwired: 2 in, 2 out]
                n1490 = property on="SET LAB02-1" class="Clust (strict)"("DisabledEnum"=w2342) -> ()  [unwired: 2 in, 2 out]
                n1491 = property on="SET LAB02-2" class="Clust (strict)"("DisabledEnum"=w2341) -> ()  [unwired: 2 in, 2 out]
                n1492 = property on="SET LAB03-1" class="Clust (strict)"("DisabledEnum"=w2340) -> ()  [unwired: 2 in, 2 out]
                n1493 = property on="O/I  LAB01-1" class="Bool (strict)"("DisabledEnum"=w2344) -> ()  [unwired: 2 in, 2 out]
                n1494 = property on="O/I  LAB01-2" class="Bool (strict)"("DisabledEnum"=w2343) -> ()  [unwired: 2 in, 2 out]
                n1495 = property on="O/I  LAB02-1" class="Bool (strict)"("DisabledEnum"=w2342) -> ()  [unwired: 2 in, 2 out]
                n1496 = property on="O/I  LAB02-2" class="Bool (strict)"("DisabledEnum"=w2341) -> ()  [unwired: 2 in, 2 out]
                n1497 = property on="O/I  LAB03-1" class="Bool (strict)"("DisabledEnum"=w2340) -> ()  [unwired: 2 in, 2 out]
              }
              frame #1 {
                n1498 = Select(t=2, s=w2374, f=0) -> (s? t:f=w2365:i32)
                n1499 = Select(t=2, s=w2373, f=0) -> (s? t:f=w2366:i32)
                n1500 = Select(t=2, s=w2370, f=0) -> (s? t:f=w2369:i32)
                n1501 = Select(t=2, s=w2371, f=0) -> (s? t:f=w2368:i32)
                n1502 = Select(t=2, s=w2372, f=0) -> (s? t:f=w2367:i32)
                n1503 = property on="SELECT LAB05-2" class="RadioBtnsControl (strict)"("DisabledEnum"=w2365) -> ()  [unwired: 2 in, 2 out]
                n1504 = property on="SELECT LAB05-1" class="RadioBtnsControl (strict)"("DisabledEnum"=w2366) -> ()  [unwired: 2 in, 2 out]
                n1505 = property on="SELECT LAB03-2" class="RadioBtnsControl (strict)"("DisabledEnum"=w2369) -> ()  [unwired: 2 in, 2 out]
                n1506 = property on="SELECT LAB04-1" class="RadioBtnsControl (strict)"("DisabledEnum"=w2368) -> ()  [unwired: 2 in, 2 out]
                n1507 = property on="SELECT LAB04-2" class="RadioBtnsControl (strict)"("DisabledEnum"=w2367) -> ()  [unwired: 2 in, 2 out]
                n1508 = property on="SET LAB05-2" class="Clust (strict)"("DisabledEnum"=w2365) -> ()  [unwired: 2 in, 2 out]
                n1509 = property on="SET LAB05-1" class="Clust (strict)"("DisabledEnum"=w2366) -> ()  [unwired: 2 in, 2 out]
                n1510 = property on="SET LAB03-2" class="Clust (strict)"("DisabledEnum"=w2369) -> ()  [unwired: 2 in, 2 out]
                n1511 = property on="SET LAB04-1" class="Clust (strict)"("DisabledEnum"=w2368) -> ()  [unwired: 2 in, 2 out]
                n1512 = property on="SET LAB04-2" class="Clust (strict)"("DisabledEnum"=w2367) -> ()  [unwired: 2 in, 2 out]
                n1513 = property on="O/I  LAB05-2" class="Bool (strict)"("DisabledEnum"=w2365) -> ()  [unwired: 2 in, 2 out]
                n1514 = property on="O/I  LAB05-1" class="Bool (strict)"("DisabledEnum"=w2366) -> ()  [unwired: 2 in, 2 out]
                n1515 = property on="O/I  LAB04-1" class="Bool (strict)"("DisabledEnum"=w2368) -> ()  [unwired: 2 in, 2 out]
                n1516 = property on="O/I  LAB04-2" class="Bool (strict)"("DisabledEnum"=w2367) -> ()  [unwired: 2 in, 2 out]
                n1517 = property on="O/I  LAB03-2" class="Bool (strict)"("DisabledEnum"=w2369) -> ()  [unwired: 2 in, 2 out]
                n1518 = Not(x=w2374) -> (.not. x?=w2375:bool)
                n1519 = Not(x=w2373) -> (.not. x?=w2376:bool)
                n1520 = Not(x=w2372) -> (.not. x?=w2377:bool)
                n1521 = property on="RESULT LAB05-2" class="Bool (strict)"("Visible"=w2375) -> ()  [unwired: 2 in, 2 out]
                n1522 = property on="RESULT LAB05-1" class="Bool (strict)"("Visible"=w2376) -> ()  [unwired: 2 in, 2 out]
                n1523 = Not(x=w2371) -> (.not. x?=w2378:bool)
                n1524 = property on="RESULT LAB04-2" class="Bool (strict)"("Visible"=w2377) -> ()  [unwired: 2 in, 2 out]
                n1525 = Not(x=w2370) -> (.not. x?=w2379:bool)
                n1526 = property on="RESULT LAB04-1" class="Bool (strict)"("Visible"=w2378) -> ()  [unwired: 2 in, 2 out]
                n1527 = property on="RESULT LAB03-2" class="Bool (strict)"("Visible"=w2379) -> ()  [unwired: 2 in, 2 out]
              }
              frame #2 {
                # "disable calibrate if any test running"
                n1528 = Or(x=w2401, y=w2400) -> (x .or. y?=w2394:bool)
                n1529 = Or(x=w2403, y=w2402) -> (x .or. y?=w2396:bool)
                n1530 = Or(x=w2407, y=w2406) -> (x .or. y?=w2398:bool)
                n1531 = Or(x=w2405, y=w2404) -> (x .or. y?=w2397:bool)
                n1532 = Or(x=w2409, y=w2408) -> (x .or. y?=w2399:bool)
                n1533 = Or(x=w2397, y=w2396) -> (x .or. y?=w2395:bool)
                n1534 = Or(x=w2399, y=w2398) -> (x .or. y?=w2393:bool)
                n1535 = Or(x=w2395, y=w2394) -> (x .or. y?=w2392:bool)
                n1536 = Or(x=w2393, y=w2392) -> (x .or. y?=w2391:bool)
                n1537 = case shown="True" w2391 {
                  tunnel: [0 2] -> w2390
                  frame False {
                  }
                  frame True {
                  }
                }
                n1538 = property on="JIG TEST" class="Clust (strict)"("DisabledEnum"=w2390) -> ()  [unwired: 2 in, 2 out]
                n1539 = property on="Network Directory" class="Path"("DisabledEnum"=w2390) -> ()  [unwired: 2 in, 2 out]
                n1540 = property on="MAIL SETTINGS" class="Clust (strict)"("DisabledEnum"=w2390) -> ()  [unwired: 2 in, 2 out]
                n1541 = property on="CALIBRATE" class="Bool (strict)"("DisabledEnum"=w2390) -> ()  [unwired: 2 in, 2 out]
                n1542 = property on="ADMIN PAGE" class="Bool (strict)"("DisabledEnum"=w2390) -> ()  [unwired: 2 in, 2 out]
              }
            }
          }
          frame #8 {
            # "drive jigs"
            n1543 = stacked-sequence {
              frame #0 {
                # "jig on"
                n1544 = local read "jig cycle"() -> (w2417:dbl)
                n1545 = property on="JIG TEST" class="Clust (strict)"() -> ("DisabledEnum"=w2414:T13)  [unwired: 2 in, 2 out]
                n1546 = Equal?(x=w2414, y=2) -> (x = y?=w2413:bool)
                n1547 = Equal?(x=w2417, y=0) -> (x = y?=w2415:bool)
                n1548 = And(x=w2415, y=w2413) -> (x .and. y?=w2412:bool)
                n1549 = case shown="True" w2412 {
                  frame False {
                  }
                  frame True {
                    n1550 = local read "run lab01-1"() -> (w2428:bool)
                    n1551 = local read "run lab01-2"() -> (w2427:bool)
                    n1552 = local read "run lab02-1"() -> (w2426:bool)
                    n1553 = local read "run lab02-2"() -> (w2425:bool)
                    n1554 = local read "run lab03-1"() -> (w2424:bool)
                    n1555 = local read "run lab03-2"() -> (w2423:bool)
                    n1556 = local read "run lab04-1"() -> (w2422:bool)
                    n1557 = local read "run lab04-2"() -> (w2421:bool)
                    n1558 = local read "run lab05-1"() -> (w2420:bool)
                    n1559 = local read "run lab05-2"() -> (w2419:bool)
                    n1560 = local write "JIG LAB03-2"(w2423) -> ()
                    n1561 = local write "JIG LAB01-1"(w2428) -> ()
                    n1562 = local write "JIG LAB01-2"(w2427) -> ()
                    n1563 = local write "JIG LAB02-1"(w2426) -> ()
                    n1564 = local write "JIG LAB02-2"(w2425) -> ()
                    n1565 = local write "JIG LAB03-1"(w2424) -> ()
                    n1566 = local write "JIG LAB04-1"(w2422) -> ()
                    n1567 = local write "JIG LAB04-2"(w2421) -> ()
                    n1568 = local write "JIG LAB05-1"(w2420) -> ()
                    n1569 = local write "JIG LAB05-2"(w2419) -> ()
                  }
                }
              }
              frame #1 {
                # "jig off"
                n1570 = local read "jig cycle"() -> (w2435:dbl)
                n1571 = local read "on loops"() -> (w2434:dbl)
                n1572 = property on="JIG TEST" class="Clust (strict)"() -> ("DisabledEnum"=w2433:T13)  [unwired: 2 in, 2 out]
                n1573 = Equal?(x=w2433, y=2) -> (x = y?=w2431:bool)
                n1574 = Equal?(x=w2435, y=w2434) -> (x = y?=w2430:bool)
                n1575 = And(x=w2430, y=w2431) -> (x .and. y?=w2429:bool)
                n1576 = case shown="True" w2429 {
                  frame False {
                  }
                  frame True {
                    w2486 = FALSE
                    w2487 = TRUE
                    w2485 = 2
                    n1577 = local read "SELECT LAB05-2"() -> (w2476:T3)
                    n1578 = local read "SELECT LAB04-2"() -> (w2478:T3)
                    n1579 = local read "SELECT LAB04-1"() -> (w2479:T3)
                    n1580 = local read "SELECT LAB05-1"() -> (w2477:T3)
                    n1581 = local read "SELECT LAB03-2"() -> (w2480:T3)
                    n1582 = local read "SELECT LAB02-1"() -> (w2483:T3)
                    n1583 = local read "SELECT LAB03-1"() -> (w2481:T3)
                    n1584 = local read "SELECT LAB02-2"() -> (w2482:T3)
                    n1585 = local read "SELECT LAB01-2"() -> (w2484:T3)
                    n1586 = local read "run lab05-1"() -> (w2446:bool)
                    n1587 = local read "run lab05-2"() -> (w2445:bool)
                    n1588 = local read "SELECT LAB01-1"() -> (w2488:T3)
                    n1589 = local read "run lab04-2"() -> (w2447:bool)
                    n1590 = local read "run lab04-1"() -> (w2448:bool)
                    n1591 = local read "run lab01-1"() -> (w2464:bool)
                    n1592 = local read "run lab01-2"() -> (w2453:bool)
                    n1593 = local read "run lab03-2"() -> (w2449:bool)
                    n1594 = local read "run lab03-1"() -> (w2450:bool)
                    n1595 = local read "run lab02-1"() -> (w2452:bool)
                    n1596 = local read "run lab02-2"() -> (w2451:bool)
                    n1597 = Equal?(x=w2485, y=w2481) -> (x = y?=w2459:bool)
                    n1598 = Equal?(x=w2485, y=w2480) -> (x = y?=w2458:bool)
                    n1599 = Equal?(x=w2485, y=w2479) -> (x = y?=w2457:bool)
                    n1600 = Equal?(x=w2485, y=w2478) -> (x = y?=w2456:bool)
                    n1601 = Equal?(x=w2485, y=w2477) -> (x = y?=w2455:bool)
                    n1602 = Equal?(x=w2485, y=w2476) -> (x = y?=w2454:bool)
                    n1603 = Equal?(x=w2485, y=w2488) -> (x = y?=w2465:bool)
                    n1604 = Equal?(x=w2485, y=w2483) -> (x = y?=w2461:bool)
                    n1605 = Equal?(x=w2485, y=w2482) -> (x = y?=w2460:bool)
                    n1606 = Equal?(x=w2485, y=w2484) -> (x = y?=w2462:bool)
                    n1607 = And(x=w2456, y=w2447) -> (x .and. y?=w2438:bool)
                    n1608 = And(x=w2459, y=w2450) -> (x .and. y?=w2441:bool)
                    n1609 = And(x=w2457, y=w2448) -> (x .and. y?=w2439:bool)
                    n1610 = And(x=w2454, y=w2445) -> (x .and. y?=w2436:bool)
                    n1611 = And(x=w2460, y=w2451) -> (x .and. y?=w2442:bool)
                    n1612 = And(x=w2458, y=w2449) -> (x .and. y?=w2440:bool)
                    n1613 = And(x=w2455, y=w2446) -> (x .and. y?=w2437:bool)
                    n1614 = And(x=w2462, y=w2453) -> (x .and. y?=w2444:bool)
                    n1615 = And(x=w2465, y=w2464) -> (x .and. y?=w2463:bool)
                    n1616 = And(x=w2461, y=w2452) -> (x .and. y?=w2443:bool)
                    n1617 = Select(t=w2487, s=w2463, f=w2486) -> (s? t:f=w2466:bool)
                    n1618 = Select(t=w2487, s=w2444, f=w2486) -> (s? t:f=w2467:bool)
                    n1619 = Select(t=w2487, s=w2443, f=w2486) -> (s? t:f=w2468:bool)
                    n1620 = Select(t=w2487, s=w2442, f=w2486) -> (s? t:f=w2469:bool)
                    n1621 = Select(t=w2487, s=w2441, f=w2486) -> (s? t:f=w2470:bool)
                    n1622 = Select(t=w2487, s=w2440, f=w2486) -> (s? t:f=w2471:bool)
                    n1623 = Select(t=w2487, s=w2439, f=w2486) -> (s? t:f=w2472:bool)
                    n1624 = Select(t=w2487, s=w2438, f=w2486) -> (s? t:f=w2473:bool)
                    n1625 = Select(t=w2487, s=w2437, f=w2486) -> (s? t:f=w2474:bool)
                    n1626 = Select(t=w2487, s=w2436, f=w2486) -> (s? t:f=w2475:bool)
                    n1627 = local write "JIG LAB03-2"(w2471) -> ()
                    n1628 = local write "JIG LAB02-1"(w2468) -> ()
                    n1629 = local write "JIG LAB02-2"(w2469) -> ()
                    n1630 = local write "JIG LAB01-2"(w2467) -> ()
                    n1631 = local write "JIG LAB03-1"(w2470) -> ()
                    n1632 = local write "JIG LAB01-1"(w2466) -> ()
                    n1633 = local write "JIG LAB05-2"(w2475) -> ()
                    n1634 = local write "JIG LAB04-1"(w2472) -> ()
                    n1635 = local write "JIG LAB05-1"(w2474) -> ()
                    n1636 = local write "JIG LAB04-2"(w2473) -> ()
                  }
                }
              }
            }
          }
          frame #9 {
            # "enable  jig test output if no test busy"
            n1637 = property on="JIG TEST" class="Clust (strict)"() -> ("DisabledEnum"=w2491:T13)  [unwired: 2 in, 2 out]
            n1638 = Equal?(x=w2491, y=0) -> (x = y?=w2489:bool)
            n1639 = case shown="True" w2489 {
              frame False {
              }
              frame True {
                n1640 = local read "JIG TEST"() -> (w2502:T10)
                n1641 = Unbundle(w2502) -> ("LAB01-1"=w2501:bool, "LAB01-2"=w2500:bool, "LAB02-1"=w2499:bool, "LAB02-2"=w2498:bool, "LAB03-1"=w2497:bool, "LAB03-2"=w2496:bool, "LAB04-1"=w2495:bool, "LAB04-2"=w2494:bool, "LAB05-1"=w2493:bool, "LAB05-2"=w2492:bool)
                n1642 = local write "JIG LAB05-1"(w2493) -> ()
                n1643 = local write "JIG LAB05-2"(w2492) -> ()
                n1644 = local write "JIG LAB04-1"(w2495) -> ()
                n1645 = local write "JIG LAB04-2"(w2494) -> ()
                n1646 = local write "JIG LAB03-2"(w2496) -> ()
                n1647 = local write "JIG LAB01-1"(w2501) -> ()
                n1648 = local write "JIG LAB02-1"(w2499) -> ()
                n1649 = local write "JIG LAB03-1"(w2497) -> ()
                n1650 = local write "JIG LAB01-2"(w2500) -> ()
                n1651 = local write "JIG LAB02-2"(w2498) -> ()
              }
            }
          }
          frame #10 {
            # "drive digital output"
            n1652 = local read "O/I  LAB05-2"() -> (w2508:bool)
            n1653 = local read "O/I  LAB05-1"() -> (w2510:bool)
            n1654 = local read "JIG LAB05-2"() -> (w2507:bool)
            n1655 = local read "O/I  LAB04-2"() -> (w2512:bool)
            n1656 = local read "JIG LAB05-1"() -> (w2509:bool)
            n1657 = local read "JIG LAB04-2"() -> (w2511:bool)
            n1658 = local read "O/I  LAB03-1"() -> (w2517:bool)
            n1659 = local read "O/I  LAB04-1"() -> (w2513:bool)
            n1660 = local read "O/I  LAB02-1"() -> (w2521:bool)
            n1661 = local read "O/I  LAB02-2"() -> (w2519:bool)
            n1662 = local read "O/I  LAB03-2"() -> (w2515:bool)
            n1663 = local read "JIG LAB04-1"() -> (w2506:bool)
            n1664 = local read "JIG LAB03-2"() -> (w2514:bool)
            n1665 = local read "O/I  LAB01-2"() -> (w2523:bool)
            n1666 = local read "JIG LAB02-1"() -> (w2520:bool)
            n1667 = local read "JIG LAB02-2"() -> (w2518:bool)
            n1668 = local read "JIG LAB03-1"() -> (w2516:bool)
            n1669 = local read "O/I  LAB01-1"() -> (w2525:bool)
            n1670 = local read "JIG LAB01-2"() -> (w2522:bool)
            n1671 = local read "JIG LAB01-1"() -> (w2524:bool)
            n1672 = Build Array(w2512, w2511, w2510, w2509, w2508, w2507) -> (w2503:bool[])
            n1673 = Build Array(w2518, w2517, w2516, w2515, w2514, w2513, w2506) -> (w2504:bool[])
            n1674 = Build Array(w2525, w2524, w2523, w2522, w2521, w2520, w2519) -> (w2505:bool[])
            n1675 = call "sub vi - Drive Relays All v6.vi"("Array #2"=w2503, "Array #1"=w2504, "Array #0"=w2505) -> ()  [unwired: 8 in, 1 out]
          }
          frame #11 {
            # "get temperature values"
            n1676 = stacked-sequence {
              frame #0 {
                n1677 = local read "Select COM port"() -> (w2526:refnum<visa-resource-name>)
                "COM port" <- w2526
                n1678 = local read "jig cycle"() -> (w2527:dbl)
                n1679 = local read "on loops"() -> (w2530:dbl)
                n1680 = local read "jig cycle"() -> (w2532:dbl)
                n1681 = Add(x=w2530, y=2) -> (x+y=w2531:dbl)
                n1682 = global write "Global 1.vi" "COM port"(w2526) -> ()
                n1683 = Equal?(x=w2532, y=0) -> (x = y?=w2533:bool)
                n1684 = Equal?(x=w2527, y=w2531) -> (x = y?=w2528:bool)
                n1685 = case shown="True" w2533 {
                  frame False {
                  }
                  frame True {
                    w2545 = FALSE
                    w2546 = TRUE
                    n1686 = local write "TEMP update"(TRUE) -> ()
                    n1687 = call "sub vi - GET ALL TEMP v4.vi"("LA01-EN"=w2546, "LA02-EN"=w2546, "LA03-EN"=w2546, "LA04-EN"=w2545, "LA05-EN"=w2545, "Gen Cal Value"=1.0) -> ("LA01 TEMP"=w2544:T21, "LA02 TEMP"=w2542:T21, "LA03 TEMP"=w2541:T21)  [unwired: 4 in, 3 out]
                    n1688 = local write "LAB03 TEMP"(w2541) -> ()
                    n1689 = local write "LAB02 TEMP"(w2542) -> ()
                    n1690 = local write "LAB01 TEMP"(w2544) -> ()
                  }
                }
                n1691 = case shown="True" w2528 {
                  frame False {
                  }
                  frame True {
                    w2538 = TRUE
                    w2539 = FALSE
                    n1692 = local write "TEMP update"(TRUE) -> ()
                    n1693 = call "sub vi - GET ALL TEMP v4.vi"("LA01-EN"=w2539, "LA02-EN"=w2539, "LA03-EN"=w2539, "LA04-EN"=w2538, "LA05-EN"=w2538, "Gen Cal Value"=1.0) -> ("LA04 TEMP"=w2536:T21, "LA05 TEMP"=w2535:T21)  [unwired: 4 in, 4 out]
                    n1694 = local write "LAB04 TEMP"(w2536) -> ()
                    n1695 = local write "LAB05 TEMP"(w2535) -> ()
                  }
                }
              }
              frame #1 {
                n1696 = local read "CAL LAB01"() -> (w2564:T7)
                n1697 = local read "LAB01 TEMP"() -> (w2565:T12)
                n1698 = Unbundle By Name(w2565) -> ("T1 Live"=w2555:dbl, "T1 Neut"=w2554:dbl, "T2 Live"=w2553:dbl, "T2 Neut"=w2552:dbl)  [unwired: 2 out]
                n1699 = Unbundle By Name(w2564) -> ("1 (TL) cal"=w2551:dbl, "1 (TN) cal"=w2550:dbl, "2 (TL) cal"=w2549:dbl, "2 (TN) cal"=w2548:dbl)  [unwired: 6 out]
                n1700 = Multiply(x=w2555, y=w2551) -> (x*y=w2561:dbl)
                n1701 = Multiply(x=w2554, y=w2550) -> (x*y=w2560:dbl)
                n1702 = Multiply(x=w2553, y=w2549) -> (x*y=w2557:dbl)
                n1703 = Multiply(x=w2552, y=w2548) -> (x*y=w2556:dbl)
                n1704 = local read "SIG LAB01-2"() -> (w2559:T2)
                n1705 = local read "SIG LAB01-1"() -> (w2563:T2)
                n1706 = Bundle By Name(cluster=w2563, "Tmp Live"=w2561, "Tmp Neut"=w2560) -> (w2562:T2)
                n1707 = Bundle By Name(cluster=w2559, "Tmp Live"=w2557, "Tmp Neut"=w2556) -> (w2558:T2)
                n1708 = local write "SIG LAB01-1"(w2562) -> ()
                n1709 = local write "SIG LAB01-2"(w2558) -> ()
              }
              frame #2 {
                n1710 = local read "CAL LAB02"() -> (w2582:T8)
                n1711 = local read "LAB02 TEMP"() -> (w2583:T12)
                n1712 = Unbundle By Name(w2583) -> ("T1 Live"=w2573:dbl, "T1 Neut"=w2572:dbl, "T2 Live"=w2571:dbl, "T2 Neut"=w2570:dbl)  [unwired: 2 out]
                n1713 = Unbundle By Name(w2582) -> ("1 (TL) cal"=w2569:dbl, "1 (TN) cal"=w2568:dbl, "2 (TL) cal"=w2567:dbl, "2 (TN) cal"=w2566:dbl)  [unwired: 6 out]
                n1714 = Multiply(x=w2573, y=w2569) -> (x*y=w2579:dbl)
                n1715 = Multiply(x=w2572, y=w2568) -> (x*y=w2578:dbl)
                n1716 = Multiply(x=w2571, y=w2567) -> (x*y=w2575:dbl)
                n1717 = Multiply(x=w2570, y=w2566) -> (x*y=w2574:dbl)
                n1718 = local read "SIG LAB02-2"() -> (w2577:T2)
                n1719 = local read "SIG LAB02-1"() -> (w2581:T2)
                n1720 = Bundle By Name(cluster=w2581, "Tmp Live"=w2579, "Tmp Neut"=w2578) -> (w2580:T2)
                n1721 = Bundle By Name(cluster=w2577, "Tmp Live"=w2575, "Tmp Neut"=w2574) -> (w2576:T2)
                n1722 = local write "SIG LAB02-1"(w2580) -> ()
                n1723 = local write "SIG LAB02-2"(w2576) -> ()
              }
              frame #3 {
                n1724 = local read "CAL LAB03"() -> (w2600:T7)
                n1725 = local read "LAB03 TEMP"() -> (w2601:T12)
                n1726 = Unbundle By Name(w2601) -> ("T1 Live"=w2591:dbl, "T1 Neut"=w2590:dbl, "T2 Live"=w2589:dbl, "T2 Neut"=w2588:dbl)  [unwired: 2 out]
                n1727 = Unbundle By Name(w2600) -> ("1 (TL) cal"=w2587:dbl, "1 (TN) cal"=w2586:dbl, "2 (TL) cal"=w2585:dbl, "2 (TN) cal"=w2584:dbl)  [unwired: 6 out]
                n1728 = Multiply(x=w2591, y=w2587) -> (x*y=w2597:dbl)
                n1729 = Multiply(x=w2590, y=w2586) -> (x*y=w2596:dbl)
                n1730 = Multiply(x=w2589, y=w2585) -> (x*y=w2593:dbl)
                n1731 = Multiply(x=w2588, y=w2584) -> (x*y=w2592:dbl)
                n1732 = local read "SIG LAB03-2"() -> (w2595:T2)
                n1733 = local read "SIG LAB03-1"() -> (w2599:T2)
                n1734 = Bundle By Name(cluster=w2599, "Tmp Live"=w2597, "Tmp Neut"=w2596) -> (w2598:T2)
                n1735 = Bundle By Name(cluster=w2595, "Tmp Live"=w2593, "Tmp Neut"=w2592) -> (w2594:T2)
                n1736 = local write "SIG LAB03-1"(w2598) -> ()
                n1737 = local write "SIG LAB03-2"(w2594) -> ()
              }
              frame #4 {
                n1738 = local read "CAL LAB04"() -> (w2618:T7)
                n1739 = local read "LAB04 TEMP"() -> (w2619:T12)
                n1740 = Unbundle By Name(w2619) -> ("T1 Live"=w2609:dbl, "T1 Neut"=w2608:dbl, "T2 Live"=w2607:dbl, "T2 Neut"=w2606:dbl)  [unwired: 2 out]
                n1741 = Unbundle By Name(w2618) -> ("1 (TL) cal"=w2605:dbl, "1 (TN) cal"=w2604:dbl, "2 (TL) cal"=w2603:dbl, "2 (TN) cal"=w2602:dbl)  [unwired: 6 out]
                n1742 = Multiply(x=w2609, y=w2605) -> (x*y=w2615:dbl)
                n1743 = Multiply(x=w2608, y=w2604) -> (x*y=w2614:dbl)
                n1744 = Multiply(x=w2607, y=w2603) -> (x*y=w2611:dbl)
                n1745 = Multiply(x=w2606, y=w2602) -> (x*y=w2610:dbl)
                n1746 = local read "SIG LAB04-2"() -> (w2613:T2)
                n1747 = local read "SIG LAB04-1"() -> (w2617:T2)
                n1748 = Bundle By Name(cluster=w2617, "Tmp Live"=w2615, "Tmp Neut"=w2614) -> (w2616:T2)
                n1749 = Bundle By Name(cluster=w2613, "Tmp Live"=w2611, "Tmp Neut"=w2610) -> (w2612:T2)
                n1750 = local write "SIG LAB04-1"(w2616) -> ()
                n1751 = local write "SIG LAB04-2"(w2612) -> ()
              }
              frame #5 {
                n1752 = local read "CAL LAB05"() -> (w2636:T7)
                n1753 = local read "LAB05 TEMP"() -> (w2637:T12)
                n1754 = Unbundle By Name(w2637) -> ("T1 Live"=w2627:dbl, "T1 Neut"=w2626:dbl, "T2 Live"=w2625:dbl, "T2 Neut"=w2624:dbl)  [unwired: 2 out]
                n1755 = Unbundle By Name(w2636) -> ("1 (TL) cal"=w2623:dbl, "1 (TN) cal"=w2622:dbl, "2 (TL) cal"=w2621:dbl, "2 (TN) cal"=w2620:dbl)  [unwired: 6 out]
                n1756 = Multiply(x=w2627, y=w2623) -> (x*y=w2633:dbl)
                n1757 = Multiply(x=w2626, y=w2622) -> (x*y=w2632:dbl)
                n1758 = Multiply(x=w2625, y=w2621) -> (x*y=w2629:dbl)
                n1759 = Multiply(x=w2624, y=w2620) -> (x*y=w2628:dbl)
                n1760 = local read "SIG LAB05-2"() -> (w2631:T2)
                n1761 = local read "SIG LAB05-1"() -> (w2635:T2)
                n1762 = Bundle By Name(cluster=w2635, "Tmp Live"=w2633, "Tmp Neut"=w2632) -> (w2634:T2)
                n1763 = Bundle By Name(cluster=w2631, "Tmp Live"=w2629, "Tmp Neut"=w2628) -> (w2630:T2)
                n1764 = local write "SIG LAB05-1"(w2634) -> ()
                n1765 = local write "SIG LAB05-2"(w2630) -> ()
              }
            }
          }
          frame #12 {
            # "get analog values"
            n1766 = local read "on loops"() -> (w2644:dbl)
            n1767 = local read "jig cycle"() -> (w2641:dbl)
            n1768 = Add(x=w2644, y=1) -> (x+y=w2642:dbl)
            n1769 = Equal?(x=w2641, y=1) -> (x = y?=w2639:bool)
            n1770 = Equal?(x=w2641, y=w2642) -> (x = y?=w2640:bool)
            n1771 = Or(x=w2639, y=w2640) -> (x .or. y?=w2638:bool)
            n1772 = case shown="True" w2638 {
              frame False {
              }
              frame True {
                n1773 = call "sub vi - Read Analog All v8.vi"() -> ("Analog loop time"=w2652:dbl, "array GRAPH"=w2651:dynamicdata[], "LAB01"=w2650:T22, "LAB02"=w2649:T23, "LAB03"=w2648:T24, "LAB04"=w2647:T25, "array ERROR"=w2653:errorcluster[], "LAB05"=w2646:T26)  [unwired: 8 in]
                n1774 = stacked-sequence {
                  tunnel: w2653 -> [w2658 _ _ _ _ _]
                  tunnel: w2652 -> [w2657 _ _ _ _ _]
                  tunnel: w2651 -> [w2656 _ _ _ _ _]
                  tunnel: w2650 -> [_ w2703 _ _ _ _]
                  tunnel: w2649 -> [_ _ w2704 _ _ _]
                  tunnel: w2648 -> [_ _ _ w2729 _ _]
                  tunnel: w2647 -> [_ _ _ _ w2752 _]
                  tunnel: w2646 -> [_ _ _ _ _ w2777]
                  frame #0 {
                    n1775 = local write "AI update"(TRUE) -> ()
                    n1776 = global write "Global 1.vi" "RATE(Hz)"("RATE (Hz)") -> ()
                    n1777 = global write "Global 1.vi" "SAMPLES"("SAMPLES") -> ()
                    n1778 = Index Array(array=w2656, index=6) -> (element=→"LAB04-1 (GRAPH)":dynamicdata)
                    n1779 = Index Array(array=w2656, index=7) -> (element=→"LAB04-2 (GRAPH)":dynamicdata)
                    n1780 = Index Array(array=w2656, index=9) -> (element=→"LAB05-2 (GRAPH)":dynamicdata)
                    n1781 = Index Array(array=w2656, index=8) -> (element=→"LAB05-1 (GRAPH)":dynamicdata)
                    n1782 = Index Array(array=w2656, index=5) -> (element=→"LAB03-2 (GRAPH)":dynamicdata)
                    n1783 = Index Array(array=w2656, index=0) -> (element=→"LAB01-1 (GRAPH)":dynamicdata)
                    n1784 = Index Array(array=w2656, index=1) -> (element=→"LAB01-2 (GRAPH)":dynamicdata)
                    n1785 = Index Array(array=w2656, index=2) -> (element=→"LAB02-1 (GRAPH)":dynamicdata)
                    n1786 = Index Array(array=w2656, index=3) -> (element=→"LAB02-2 (GRAPH)":dynamicdata)
                    n1787 = Index Array(array=w2656, index=4) -> (element=→"LAB03-1 (GRAPH)":dynamicdata)
                    "AI loop time" <- w2657
                    "Analog Error Array" <- w2658
                  }
                  frame #1 {
                    n1788 = local read "CAL LAB01"() -> (w2702:T7)
                    n1789 = Unbundle By Name(w2703) -> ("LAB01-1 (A)"=w2701:dbl, "LAB01-1 (V)"=w2700:dbl, "LAB01-1 (PF)"=w2699:dbl, "LAB01-2 (A)"=w2698:dbl, "LAB01-2 (V)"=w2697:dbl, "LAB01-2 (PF)"=w2696:dbl)
                    n1790 = Unbundle By Name(w2702) -> ("1  (A) cal"=w2695:dbl, "1 (V) cal"=w2694:dbl, "1 (PF) cal"=w2693:dbl, "2 (A) cal"=w2692:dbl, "2 (V) cal"=w2691:dbl, "2 (PF) cal"=w2690:dbl)  [unwired: 4 out]
                    n1791 = Multiply(x=w2701, y=w2695) -> (x*y=w2688:dbl)
                    n1792 = Multiply(x=w2700, y=w2694) -> (x*y=w2687:dbl)
                    n1793 = Multiply(x=w2699, y=w2693) -> (x*y=w2686:dbl)
                    n1794 = Multiply(x=w2698, y=w2692) -> (x*y=w2682:dbl)
                    n1795 = Multiply(x=w2697, y=w2691) -> (x*y=w2681:dbl)
                    n1796 = Multiply(x=w2696, y=w2690) -> (x*y=w2680:dbl)
                    n1797 = local read "SIG LAB01-1"() -> (w2689:T2)
                    n1798 = local read "SIG LAB01-2"() -> (w2684:T2)
                    n1799 = Bundle By Name(cluster=w2689, "AMPS"=w2688, "VOLTS"=w2687, "PF"=w2686) -> (w2685:T2)
                    n1800 = Bundle By Name(cluster=w2684, "AMPS"=w2682, "VOLTS"=w2681, "PF"=w2680) -> (w2683:T2)
                    n1801 = local write "SIG LAB01-2"(w2683) -> ()
                    n1802 = local write "SIG LAB01-1"(w2685) -> ()
                  }
                  frame #2 {
                    n1803 = local read "CAL LAB02"() -> (w2727:T8)
                    n1804 = Unbundle By Name(w2704) -> ("LAB02-1 (A)"=w2726:dbl, "LAB02-1 (V)"=w2725:dbl, "LAB02-1 (PF)"=w2724:dbl, "LAB02-2 (A)"=w2723:dbl, "LAB02-2 (V)"=w2722:dbl, "LAB02-2 (PF)"=w2721:dbl)
                    n1805 = Unbundle By Name(w2727) -> ("1 (A) cal"=w2720:dbl, "1 (V) cal"=w2719:dbl, "1 (PF) cal"=w2718:dbl, "2 (A) cal"=w2717:dbl, "2 (V) cal"=w2716:dbl, "2 (PF) cal"=w2715:dbl)  [unwired: 4 out]
                    n1806 = Multiply(x=w2726, y=w2720) -> (x*y=w2713:dbl)
                    n1807 = Multiply(x=w2725, y=w2719) -> (x*y=w2712:dbl)
                    n1808 = Multiply(x=w2724, y=w2718) -> (x*y=w2711:dbl)
                    n1809 = Multiply(x=w2723, y=w2717) -> (x*y=w2707:dbl)
                    n1810 = Multiply(x=w2722, y=w2716) -> (x*y=w2706:dbl)
                    n1811 = Multiply(x=w2721, y=w2715) -> (x*y=w2705:dbl)
                    n1812 = local read "SIG LAB02-1"() -> (w2714:T2)
                    n1813 = local read "SIG LAB02-2"() -> (w2709:T2)
                    n1814 = Bundle By Name(cluster=w2714, "AMPS"=w2713, "VOLTS"=w2712, "PF"=w2711) -> (w2710:T2)
                    n1815 = Bundle By Name(cluster=w2709, "AMPS"=w2707, "VOLTS"=w2706, "PF"=w2705) -> (w2708:T2)
                    n1816 = local write "SIG LAB02-2"(w2708) -> ()
                    n1817 = local write "SIG LAB02-1"(w2710) -> ()
                  }
                  frame #3 {
                    n1818 = local read "CAL LAB03"() -> (w2751:T7)
                    n1819 = Unbundle By Name(w2729) -> ("LAB03-1 (A)"=w2750:dbl, "LAB03-1 (V)"=w2749:dbl, "LAB03-1 (PF)"=w2748:dbl, "LAB03-2 (A)"=w2747:dbl, "LAB03-2 (V)"=w2746:dbl, "LAB03-2 (PF)"=w2745:dbl)
                    n1820 = Unbundle By Name(w2751) -> ("1  (A) cal"=w2744:dbl, "1 (V) cal"=w2743:dbl, "1 (PF) cal"=w2742:dbl, "2 (A) cal"=w2741:dbl, "2 (V) cal"=w2740:dbl, "2 (PF) cal"=w2739:dbl)  [unwired: 4 out]
                    n1821 = Multiply(x=w2750, y=w2744) -> (x*y=w2737:dbl)
                    n1822 = Multiply(x=w2749, y=w2743) -> (x*y=w2728:dbl)
                    n1823 = Multiply(x=w2748, y=w2742) -> (x*y=w2736:dbl)
                    n1824 = Multiply(x=w2747, y=w2741) -> (x*y=w2732:dbl)
                    n1825 = Multiply(x=w2746, y=w2740) -> (x*y=w2731:dbl)
                    n1826 = Multiply(x=w2745, y=w2739) -> (x*y=w2730:dbl)
                    n1827 = local read "SIG LAB03-1"() -> (w2738:T2)
                    n1828 = local read "SIG LAB03-2"() -> (w2734:T2)
                    n1829 = Bundle By Name(cluster=w2738, "AMPS"=w2737, "VOLTS"=w2728, "PF"=w2736) -> (w2735:T2)
                    n1830 = Bundle By Name(cluster=w2734, "AMPS"=w2732, "VOLTS"=w2731, "PF"=w2730) -> (w2733:T2)
                    n1831 = local write "SIG LAB03-2"(w2733) -> ()
                    n1832 = local write "SIG LAB03-1"(w2735) -> ()
                  }
                  frame #4 {
                    n1833 = local read "CAL LAB04"() -> (w2775:T7)
                    n1834 = Unbundle By Name(w2752) -> ("LAB04-1 (A)"=w2774:dbl, "LAB04-1 (V)"=w2773:dbl, "LAB04-1 (PF)"=w2772:dbl, "LAB04-2 (A)"=w2771:dbl, "LAB04-2 (V)"=w2770:dbl, "LAB04-2 (PF)"=w2769:dbl)
                    n1835 = Unbundle By Name(w2775) -> ("1  (A) cal"=w2768:dbl, "1 (V) cal"=w2767:dbl, "1 (PF) cal"=w2766:dbl, "2 (A) cal"=w2765:dbl, "2 (V) cal"=w2764:dbl, "2 (PF) cal"=w2763:dbl)  [unwired: 4 out]
                    n1836 = Multiply(x=w2774, y=w2768) -> (x*y=w2761:dbl)
                    n1837 = Multiply(x=w2773, y=w2767) -> (x*y=w2760:dbl)
                    n1838 = Multiply(x=w2772, y=w2766) -> (x*y=w2759:dbl)
                    n1839 = Multiply(x=w2771, y=w2765) -> (x*y=w2755:dbl)
                    n1840 = Multiply(x=w2770, y=w2764) -> (x*y=w2754:dbl)
                    n1841 = Multiply(x=w2769, y=w2763) -> (x*y=w2753:dbl)
                    n1842 = local read "SIG LAB04-1"() -> (w2762:T2)
                    n1843 = local read "SIG LAB04-2"() -> (w2757:T2)
                    n1844 = Bundle By Name(cluster=w2762, "AMPS"=w2761, "VOLTS"=w2760, "PF"=w2759) -> (w2758:T2)
                    n1845 = Bundle By Name(cluster=w2757, "AMPS"=w2755, "VOLTS"=w2754, "PF"=w2753) -> (w2756:T2)
                    n1846 = local write "SIG LAB04-2"(w2756) -> ()
                    n1847 = local write "SIG LAB04-1"(w2758) -> ()
                  }
                  frame #5 {
                    n1848 = local read "CAL LAB05"() -> (w2799:T7)
                    n1849 = Unbundle By Name(w2777) -> ("LAB05-1 (A)"=w2798:dbl, "LAB05-1 (V)"=w2776:dbl, "LAB05-1 (PF)"=w2797:dbl, "LAB05-2 (A)"=w2796:dbl, "LAB05-2 (V)"=w2795:dbl, "LAB05-2 (PF)"=w2794:dbl)
                    n1850 = Unbundle By Name(w2799) -> ("1  (A) cal"=w2793:dbl, "1 (V) cal"=w2792:dbl, "1 (PF) cal"=w2791:dbl, "2 (A) cal"=w2790:dbl, "2 (V) cal"=w2789:dbl, "2 (PF) cal"=w2788:dbl)  [unwired: 4 out]
                    n1851 = Multiply(x=w2798, y=w2793) -> (x*y=w2786:dbl)
                    n1852 = Multiply(x=w2776, y=w2792) -> (x*y=w2785:dbl)
                    n1853 = Multiply(x=w2797, y=w2791) -> (x*y=w2784:dbl)
                    n1854 = Multiply(x=w2796, y=w2790) -> (x*y=w2780:dbl)
                    n1855 = Multiply(x=w2795, y=w2789) -> (x*y=w2779:dbl)
                    n1856 = Multiply(x=w2794, y=w2788) -> (x*y=w2778:dbl)
                    n1857 = local read "SIG LAB05-1"() -> (w2787:T2)
                    n1858 = local read "SIG LAB05-2"() -> (w2782:T2)
                    n1859 = Bundle By Name(cluster=w2787, "AMPS"=w2786, "VOLTS"=w2785, "PF"=w2784) -> (w2783:T2)
                    n1860 = Bundle By Name(cluster=w2782, "AMPS"=w2780, "VOLTS"=w2779, "PF"=w2778) -> (w2781:T2)
                    n1861 = local write "SIG LAB05-2"(w2781) -> ()
                    n1862 = local write "SIG LAB05-1"(w2783) -> ()
                  }
                }
              }
            }
          }
          frame #13 {
            # "save test data to file"
            n1863 = Get Date/Time In Seconds() -> (seconds since 1Jan1904=w2800:timestamp)
            "File Time Stamp" <- w2800
            n1864 = local read "on loops"() -> (w2819:dbl)
            n1865 = local read "jig cycle"() -> (w2816:dbl)
            n1866 = Format Date/Time String(time format string (%c)="%H:%M%:%S", seconds (now)=w2800) -> (date/time string=w2804:string)  [unwired: 1 in]
            n1867 = Add(x=w2819, y=2) -> (x+y=w2817:dbl)
            n1868 = Build Array(w2804) -> (w2803:string[])
            n1869 = Equal?(x=w2816, y=1) -> (x = y?=w2802:bool)
            n1870 = Equal?(x=w2816, y=w2817) -> (x = y?=w2801:bool)
            n1871 = stacked-sequence {
              tunnel: w2815 -> [w2825 _ _ _ _ _ _ _ _ _]
              tunnel: w2814 -> [_ w2901 _ _ _ _ _ _ _ _]
              tunnel: w2813 -> [_ _ w2981 _ _ _ _ _ _ _]
              tunnel: w2812 -> [_ _ _ w3061 _ _ _ _ _ _]
              tunnel: w2811 -> [_ _ _ _ w3141 _ _ _ _ _]
              tunnel: w2810 -> [_ _ _ _ _ w3221 _ _ _ _]
              tunnel: w2809 -> [_ _ _ _ _ _ w3301 _ _ _]
              tunnel: w2808 -> [_ _ _ _ _ _ _ w3381 _ _]
              tunnel: w2807 -> [_ _ _ _ _ _ _ _ w3461 _]
              tunnel: w2806 -> [_ _ _ _ _ _ _ _ _ w3541]
              tunnel: w2803 -> [w2824 w2905 w2985 w3065 w3145 w3225 w3305 w3385 w3465 w3545]
              tunnel: w2802 -> [w2823 w2904 w2984 w3064 w3144 w3224 w3304 w3384 w3464 w3544]
              tunnel: w2801 -> [w2822 w2903 w2983 w3063 w3143 w3223 w3303 w3383 w3463 w3543]
              tunnel: w2800 -> [w2821 w2902 w2982 w3062 w3142 w3222 w3302 w3382 w3462 w3542]
              frame #0 {
                n1872 = case shown="True" w2825 {
                  tunnel: w2824 -> [_ w2830]
                  tunnel: w2823 -> [_ w2829]
                  tunnel: w2822 -> [_ w2827]
                  tunnel: w2821 -> [_ w2826]
                  frame False {
                  }
                  frame True {
                    n1873 = local read "DISP LAB01-1"() -> (w2831:T4)
                    n1874 = local read "SIG LAB01-1"() -> (w2832:T2)
                    n1875 = local read "ON L01-1"() -> (w2828:cluster{"amps":dbl, "volts":dbl, "pf":dbl})
                    n1876 = Unbundle(w2832) -> ("AMPS"=w2838:dbl, "VOLTS"=w2836:dbl, "PF"=w2835:dbl, "Tmp Live"=w2834:dbl, "Tmp Neut"=w2837:dbl)
                    n1877 = Unbundle(w2831) -> ("CYCLE"=w2833:dbl)  [unwired: 2 out]
                    n1878 = stacked-sequence {
                      tunnel: w2838 -> [w2842 w2861]
                      tunnel: w2837 -> [_ w2860]
                      tunnel: w2836 -> [w2841 w2859]
                      tunnel: w2835 -> [w2840 w2858]
                      tunnel: w2834 -> [_ w2857]
                      tunnel: w2833 -> [_ w2856]
                      tunnel: w2830 -> [_ w2855]
                      tunnel: w2829 -> [w2843 _]
                      tunnel: w2828 -> [w2839 w2853]
                      tunnel: w2827 -> [_ w2854]
                      tunnel: w2826 -> [_ w2849]
                      frame #0 {
                        n1879 = case shown="True" w2843 {
                          tunnel: w2842 -> [_ w2848]
                          tunnel: w2841 -> [_ w2847]
                          tunnel: w2840 -> [_ w2846]
                          tunnel: w2839 -> [_ w2844]
                          frame False {
                          }
                          frame True {
                            n1880 = Bundle(cluster=w2844, "amps"=w2848, "volts"=w2847, "pf"=w2846) -> (w2845:cluster{"amps":dbl, "volts":dbl, "pf":dbl})
                            n1881 = local write "ON L01-1"(w2845) -> ()
                          }
                        }
                      }
                      frame #1 {
                        n1882 = Unbundle(w2853) -> ("amps"=w2852:dbl, "volts"=w2851:dbl, "pf"=w2850:dbl)
                        n1883 = case shown="True" w2854 {
                          tunnel: w2861 -> [_ w2862]
                          tunnel: w2860 -> [_ w2900]
                          tunnel: w2859 -> [_ _]
                          tunnel: w2858 -> [_ _]
                          tunnel: w2857 -> [_ w2899]
                          tunnel: w2856 -> [_ w2898]
                          tunnel: w2855 -> [_ w2866]
                          tunnel: w2852 -> [_ w2863]
                          tunnel: w2851 -> [_ w2895]
                          tunnel: w2850 -> [_ w2894]
                          tunnel: w2849 -> [_ w2864]
                          frame False {
                          }
                          frame True {
                            n1884 = local read "TDMS LAB01-1"() -> (w2897:refnum<k34>)
                            n1885 = Build Array(w2895) -> (w2891:dbl[])
                            n1886 = Build Array(w2894) -> (w2890:dbl[])
                            n1887 = Build Array(w2899) -> (w2889:dbl[])
                            n1888 = Build Array(w2900) -> (w2888:dbl[])
                            n1889 = Build Array(w2863) -> (w2893:dbl[])
                            n1890 = Build Array(w2862) -> (w2892:dbl[])
                            n1891 = Build Array(w2898) -> (w2887:dbl[])
                            n1892 = Build Array("AMPS ON", "AMPS OFF", "VOLTS", "PF", "TEMP Live", "TEMP Neut", "CYCLE") -> (w2871:string[])
                            n1893 = Bundle By Name("Y"=w2893, "t0"=w2864) -> (w2886:waveform(dbl))  [unwired: 1 in]
                            n1894 = Bundle By Name("Y"=w2892, "t0"=w2864) -> (w2885:waveform(dbl))  [unwired: 1 in]
                            n1895 = Bundle By Name("Y"=w2891, "t0"=w2864) -> (w2884:waveform(dbl))  [unwired: 1 in]
                            n1896 = Bundle By Name("Y"=w2890, "t0"=w2864) -> (w2883:waveform(dbl))  [unwired: 1 in]
                            n1897 = Bundle By Name("Y"=w2889, "t0"=w2864) -> (w2882:waveform(dbl))  [unwired: 1 in]
                            n1898 = Bundle By Name("Y"=w2888, "t0"=w2864) -> (w2881:waveform(dbl))  [unwired: 1 in]
                            n1899 = Bundle By Name("Y"=w2887, "t0"=w2864) -> (w2880:waveform(dbl))  [unwired: 1 in]
                            n1900 = Build Array(w2886, w2885, w2884, w2883, w2882, w2881, w2880) -> (w2879:waveform(dbl)[])
                            n1901 = TDMS Write(0:w2897, 5:"TEST VALUES", 7:w2871, 9:w2879) -> (4:w2870:refnum<k34>, 6:w2869:string, 15:w2868:errorcluster)  [unwired: 2 in, 1 out]
                            n1902 = TDMS Write(0:w2870, 5:w2869, 7:"TIME", 9:w2866, 11:w2868) -> (15:w2865:errorcluster)  [unwired: 1 in, 3 out]
                            n1903 = local write "data file error"(w2865) -> ()
                          }
                        }
                      }
                    }
                  }
                }
              }
              frame #1 {
                n1904 = case shown="True" w2901 {
                  tunnel: w2905 -> [_ w2910]
                  tunnel: w2904 -> [_ w2909]
                  tunnel: w2903 -> [_ w2907]
                  tunnel: w2902 -> [_ w2906]
                  frame False {
                  }
                  frame True {
                    n1905 = local read "DISP LAB01-2"() -> (w2911:T4)
                    n1906 = local read "SIG LAB01-2"() -> (w2912:T2)
                    n1907 = local read "ON L01-2"() -> (w2908:cluster{"amps":dbl, "volts":dbl, "pf":dbl})
                    n1908 = Unbundle(w2912) -> ("AMPS"=w2918:dbl, "VOLTS"=w2916:dbl, "PF"=w2915:dbl, "Tmp Live"=w2914:dbl, "Tmp Neut"=w2917:dbl)
                    n1909 = Unbundle(w2911) -> ("CYCLE"=w2913:dbl)  [unwired: 2 out]
                    n1910 = stacked-sequence {
                      tunnel: w2918 -> [w2922 w2941]
                      tunnel: w2917 -> [_ w2940]
                      tunnel: w2916 -> [w2921 w2939]
                      tunnel: w2915 -> [w2920 w2938]
                      tunnel: w2914 -> [_ w2937]
                      tunnel: w2913 -> [_ w2936]
                      tunnel: w2910 -> [_ w2935]
                      tunnel: w2909 -> [w2923 _]
                      tunnel: w2908 -> [w2919 w2933]
                      tunnel: w2907 -> [_ w2934]
                      tunnel: w2906 -> [_ w2929]
                      frame #0 {
                        n1911 = case shown="True" w2923 {
                          tunnel: w2922 -> [_ w2928]
                          tunnel: w2921 -> [_ w2927]
                          tunnel: w2920 -> [_ w2926]
                          tunnel: w2919 -> [_ w2924]
                          frame False {
                          }
                          frame True {
                            n1912 = Bundle(cluster=w2924, "amps"=w2928, "volts"=w2927, "pf"=w2926) -> (w2925:cluster{"amps":dbl, "volts":dbl, "pf":dbl})
                            n1913 = local write "ON L01-2"(w2925) -> ()
                          }
                        }
                      }
                      frame #1 {
                        n1914 = Unbundle(w2933) -> ("amps"=w2932:dbl, "volts"=w2931:dbl, "pf"=w2930:dbl)
                        n1915 = case shown="True" w2934 {
                          tunnel: w2941 -> [_ w2973]
                          tunnel: w2940 -> [_ w2980]
                          tunnel: w2939 -> [_ _]
                          tunnel: w2938 -> [_ _]
                          tunnel: w2937 -> [_ w2979]
                          tunnel: w2936 -> [_ w2978]
                          tunnel: w2935 -> [_ w2943]
                          tunnel: w2932 -> [_ w2975]
                          tunnel: w2931 -> [_ w2974]
                          tunnel: w2930 -> [_ w2972]
                          tunnel: w2929 -> [_ w2964]
                          frame False {
                          }
                          frame True {
                            n1916 = local read "TDMS LAB01-2"() -> (w2977:refnum<k34>)
                            n1917 = Build Array(w2974) -> (w2969:dbl[])
                            n1918 = Build Array(w2972) -> (w2968:dbl[])
                            n1919 = Build Array(w2979) -> (w2967:dbl[])
                            n1920 = Build Array(w2980) -> (w2966:dbl[])
                            n1921 = Build Array(w2975) -> (w2971:dbl[])
                            n1922 = Build Array(w2973) -> (w2970:dbl[])
                            n1923 = Build Array(w2978) -> (w2965:dbl[])
                            n1924 = Build Array("AMPS ON", "AMPS OFF", "VOLTS", "PF", "TEMP Live", "TEMP Neut", "CYCLE") -> (w2948:string[])
                            n1925 = Bundle By Name("Y"=w2971, "t0"=w2964) -> (w2963:waveform(dbl))  [unwired: 1 in]
                            n1926 = Bundle By Name("Y"=w2970, "t0"=w2964) -> (w2962:waveform(dbl))  [unwired: 1 in]
                            n1927 = Bundle By Name("Y"=w2969, "t0"=w2964) -> (w2961:waveform(dbl))  [unwired: 1 in]
                            n1928 = Bundle By Name("Y"=w2968, "t0"=w2964) -> (w2960:waveform(dbl))  [unwired: 1 in]
                            n1929 = Bundle By Name("Y"=w2967, "t0"=w2964) -> (w2959:waveform(dbl))  [unwired: 1 in]
                            n1930 = Bundle By Name("Y"=w2966, "t0"=w2964) -> (w2958:waveform(dbl))  [unwired: 1 in]
                            n1931 = Bundle By Name("Y"=w2965, "t0"=w2964) -> (w2957:waveform(dbl))  [unwired: 1 in]
                            n1932 = Build Array(w2963, w2962, w2961, w2960, w2959, w2958, w2957) -> (w2956:waveform(dbl)[])
                            n1933 = TDMS Write(0:w2977, 5:"TEST VALUES", 7:w2948, 9:w2956) -> (4:w2947:refnum<k34>, 6:w2946:string, 15:w2945:errorcluster)  [unwired: 2 in, 1 out]
                            n1934 = TDMS Write(0:w2947, 5:w2946, 7:"TIME", 9:w2943, 11:w2945) -> (15:w2942:errorcluster)  [unwired: 1 in, 3 out]
                            n1935 = local write "data file error"(w2942) -> ()
                          }
                        }
                      }
                    }
                  }
                }
              }
              frame #2 {
                n1936 = case shown="True" w2981 {
                  tunnel: w2985 -> [_ w2990]
                  tunnel: w2984 -> [_ w2989]
                  tunnel: w2983 -> [_ w2987]
                  tunnel: w2982 -> [_ w2986]
                  frame False {
                  }
                  frame True {
                    n1937 = local read "DISP LAB02-1"() -> (w2991:T4)
                    n1938 = local read "SIG LAB02-1"() -> (w2992:T2)
                    n1939 = local read "ON L02-1"() -> (w2988:cluster{"amps":dbl, "volts":dbl, "pf":dbl})
                    n1940 = Unbundle(w2992) -> ("AMPS"=w2998:dbl, "VOLTS"=w2996:dbl, "PF"=w2995:dbl, "Tmp Live"=w2994:dbl, "Tmp Neut"=w2997:dbl)
                    n1941 = Unbundle(w2991) -> ("CYCLE"=w2993:dbl)  [unwired: 2 out]
                    n1942 = stacked-sequence {
                      tunnel: w2998 -> [w3002 w3021]
                      tunnel: w2997 -> [_ w3020]
                      tunnel: w2996 -> [w3001 w3019]
                      tunnel: w2995 -> [w3000 w3018]
                      tunnel: w2994 -> [_ w3017]
                      tunnel: w2993 -> [_ w3016]
                      tunnel: w2990 -> [_ w3015]
                      tunnel: w2989 -> [w3003 _]
                      tunnel: w2988 -> [w2999 w3013]
                      tunnel: w2987 -> [_ w3014]
                      tunnel: w2986 -> [_ w3009]
                      frame #0 {
                        n1943 = case shown="True" w3003 {
                          tunnel: w3002 -> [_ w3008]
                          tunnel: w3001 -> [_ w3007]
                          tunnel: w3000 -> [_ w3006]
                          tunnel: w2999 -> [_ w3004]
                          frame False {
                          }
                          frame True {
                            n1944 = Bundle(cluster=w3004, "amps"=w3008, "volts"=w3007, "pf"=w3006) -> (w3005:cluster{"amps":dbl, "volts":dbl, "pf":dbl})
                            n1945 = local write "ON L02-1"(w3005) -> ()
                          }
                        }
                      }
                      frame #1 {
                        n1946 = Unbundle(w3013) -> ("amps"=w3012:dbl, "volts"=w3011:dbl, "pf"=w3010:dbl)
                        n1947 = case shown="True" w3014 {
                          tunnel: w3021 -> [_ w3053]
                          tunnel: w3020 -> [_ w3060]
                          tunnel: w3019 -> [_ _]
                          tunnel: w3018 -> [_ _]
                          tunnel: w3017 -> [_ w3059]
                          tunnel: w3016 -> [_ w3058]
                          tunnel: w3015 -> [_ w3023]
                          tunnel: w3012 -> [_ w3055]
                          tunnel: w3011 -> [_ w3054]
                          tunnel: w3010 -> [_ w3052]
                          tunnel: w3009 -> [_ w3044]
                          frame False {
                          }
                          frame True {
                            n1948 = local read "TDMS LAB02-1"() -> (w3057:refnum<k34>)
                            n1949 = Build Array(w3054) -> (w3049:dbl[])
                            n1950 = Build Array(w3052) -> (w3048:dbl[])
                            n1951 = Build Array(w3059) -> (w3047:dbl[])
                            n1952 = Build Array(w3060) -> (w3046:dbl[])
                            n1953 = Build Array(w3055) -> (w3051:dbl[])
                            n1954 = Build Array(w3053) -> (w3050:dbl[])
                            n1955 = Build Array(w3058) -> (w3045:dbl[])
                            n1956 = Build Array("AMPS ON", "AMPS OFF", "VOLTS", "PF", "TEMP Live", "TEMP Neut", "CYCLE") -> (w3028:string[])
                            n1957 = Bundle By Name("Y"=w3051, "t0"=w3044) -> (w3043:waveform(dbl))  [unwired: 1 in]
                            n1958 = Bundle By Name("Y"=w3050, "t0"=w3044) -> (w3042:waveform(dbl))  [unwired: 1 in]
                            n1959 = Bundle By Name("Y"=w3049, "t0"=w3044) -> (w3041:waveform(dbl))  [unwired: 1 in]
                            n1960 = Bundle By Name("Y"=w3048, "t0"=w3044) -> (w3040:waveform(dbl))  [unwired: 1 in]
                            n1961 = Bundle By Name("Y"=w3047, "t0"=w3044) -> (w3039:waveform(dbl))  [unwired: 1 in]
                            n1962 = Bundle By Name("Y"=w3046, "t0"=w3044) -> (w3038:waveform(dbl))  [unwired: 1 in]
                            n1963 = Bundle By Name("Y"=w3045, "t0"=w3044) -> (w3037:waveform(dbl))  [unwired: 1 in]
                            n1964 = Build Array(w3043, w3042, w3041, w3040, w3039, w3038, w3037) -> (w3036:waveform(dbl)[])
                            n1965 = TDMS Write(0:w3057, 5:"TEST VALUES", 7:w3028, 9:w3036) -> (4:w3027:refnum<k34>, 6:w3026:string, 15:w3025:errorcluster)  [unwired: 2 in, 1 out]
                            n1966 = TDMS Write(0:w3027, 5:w3026, 7:"TIME", 9:w3023, 11:w3025) -> (15:w3022:errorcluster)  [unwired: 1 in, 3 out]
                            n1967 = local write "data file error"(w3022) -> ()
                          }
                        }
                      }
                    }
                  }
                }
              }
              frame #3 {
                n1968 = case shown="True" w3061 {
                  tunnel: w3065 -> [_ w3070]
                  tunnel: w3064 -> [_ w3069]
                  tunnel: w3063 -> [_ w3067]
                  tunnel: w3062 -> [_ w3066]
                  frame False {
                  }
                  frame True {
                    n1969 = local read "DISP LAB02-2"() -> (w3071:T4)
                    n1970 = local read "SIG LAB02-2"() -> (w3072:T2)
                    n1971 = local read "ON L02-2"() -> (w3068:cluster{"amps":dbl, "volts":dbl, "pf":dbl})
                    n1972 = Unbundle(w3072) -> ("AMPS"=w3078:dbl, "VOLTS"=w3076:dbl, "PF"=w3075:dbl, "Tmp Live"=w3074:dbl, "Tmp Neut"=w3077:dbl)
                    n1973 = Unbundle(w3071) -> ("CYCLE"=w3073:dbl)  [unwired: 2 out]
                    n1974 = stacked-sequence {
                      tunnel: w3078 -> [w3082 w3101]
                      tunnel: w3077 -> [_ w3100]
                      tunnel: w3076 -> [w3081 w3099]
                      tunnel: w3075 -> [w3080 w3098]
                      tunnel: w3074 -> [_ w3097]
                      tunnel: w3073 -> [_ w3096]
                      tunnel: w3070 -> [_ w3095]
                      tunnel: w3069 -> [w3083 _]
                      tunnel: w3068 -> [w3079 w3093]
                      tunnel: w3067 -> [_ w3094]
                      tunnel: w3066 -> [_ w3089]
                      frame #0 {
                        n1975 = case shown="True" w3083 {
                          tunnel: w3082 -> [_ w3088]
                          tunnel: w3081 -> [_ w3087]
                          tunnel: w3080 -> [_ w3086]
                          tunnel: w3079 -> [_ w3084]
                          frame False {
                          }
                          frame True {
                            n1976 = Bundle(cluster=w3084, "amps"=w3088, "volts"=w3087, "pf"=w3086) -> (w3085:cluster{"amps":dbl, "volts":dbl, "pf":dbl})
                            n1977 = local write "ON L02-2"(w3085) -> ()
                          }
                        }
                      }
                      frame #1 {
                        n1978 = Unbundle(w3093) -> ("amps"=w3092:dbl, "volts"=w3091:dbl, "pf"=w3090:dbl)
                        n1979 = case shown="True" w3094 {
                          tunnel: w3101 -> [_ w3133]
                          tunnel: w3100 -> [_ w3140]
                          tunnel: w3099 -> [_ _]
                          tunnel: w3098 -> [_ _]
                          tunnel: w3097 -> [_ w3139]
                          tunnel: w3096 -> [_ w3138]
                          tunnel: w3095 -> [_ w3103]
                          tunnel: w3092 -> [_ w3135]
                          tunnel: w3091 -> [_ w3134]
                          tunnel: w3090 -> [_ w3132]
                          tunnel: w3089 -> [_ w3124]
                          frame False {
                          }
                          frame True {
                            n1980 = local read "TDMS LAB02-2"() -> (w3137:refnum<k34>)
                            n1981 = Build Array(w3134) -> (w3129:dbl[])
                            n1982 = Build Array(w3132) -> (w3128:dbl[])
                            n1983 = Build Array(w3139) -> (w3127:dbl[])
                            n1984 = Build Array(w3140) -> (w3126:dbl[])
                            n1985 = Build Array(w3135) -> (w3131:dbl[])
                            n1986 = Build Array(w3133) -> (w3130:dbl[])
                            n1987 = Build Array(w3138) -> (w3125:dbl[])
                            n1988 = Build Array("AMPS ON", "AMPS OFF", "VOLTS", "PF", "TEMP Live", "TEMP Neut", "CYCLE") -> (w3108:string[])
                            n1989 = Bundle By Name("Y"=w3131, "t0"=w3124) -> (w3123:waveform(dbl))  [unwired: 1 in]
                            n1990 = Bundle By Name("Y"=w3130, "t0"=w3124) -> (w3122:waveform(dbl))  [unwired: 1 in]
                            n1991 = Bundle By Name("Y"=w3129, "t0"=w3124) -> (w3121:waveform(dbl))  [unwired: 1 in]
                            n1992 = Bundle By Name("Y"=w3128, "t0"=w3124) -> (w3120:waveform(dbl))  [unwired: 1 in]
                            n1993 = Bundle By Name("Y"=w3127, "t0"=w3124) -> (w3119:waveform(dbl))  [unwired: 1 in]
                            n1994 = Bundle By Name("Y"=w3126, "t0"=w3124) -> (w3118:waveform(dbl))  [unwired: 1 in]
                            n1995 = Bundle By Name("Y"=w3125, "t0"=w3124) -> (w3117:waveform(dbl))  [unwired: 1 in]
                            n1996 = Build Array(w3123, w3122, w3121, w3120, w3119, w3118, w3117) -> (w3116:waveform(dbl)[])
                            n1997 = TDMS Write(0:w3137, 5:"TEST VALUES", 7:w3108, 9:w3116) -> (4:w3107:refnum<k34>, 6:w3106:string, 15:w3105:errorcluster)  [unwired: 2 in, 1 out]
                            n1998 = TDMS Write(0:w3107, 5:w3106, 7:"TIME", 9:w3103, 11:w3105) -> (15:w3102:errorcluster)  [unwired: 1 in, 3 out]
                            n1999 = local write "data file error"(w3102) -> ()
                          }
                        }
                      }
                    }
                  }
                }
              }
              frame #4 {
                n2000 = case shown="True" w3141 {
                  tunnel: w3145 -> [_ w3150]
                  tunnel: w3144 -> [_ w3149]
                  tunnel: w3143 -> [_ w3147]
                  tunnel: w3142 -> [_ w3146]
                  frame False {
                  }
                  frame True {
                    n2001 = local read "DISP LAB03-1"() -> (w3151:T4)
                    n2002 = local read "SIG LAB03-1"() -> (w3152:T2)
                    n2003 = local read "ON L03-1"() -> (w3148:cluster{"amps":dbl, "volts":dbl, "pf":dbl})
                    n2004 = Unbundle(w3152) -> ("AMPS"=w3158:dbl, "VOLTS"=w3156:dbl, "PF"=w3155:dbl, "Tmp Live"=w3154:dbl, "Tmp Neut"=w3157:dbl)
                    n2005 = Unbundle(w3151) -> ("CYCLE"=w3153:dbl)  [unwired: 2 out]
                    n2006 = stacked-sequence {
                      tunnel: w3158 -> [w3162 w3181]
                      tunnel: w3157 -> [_ w3180]
                      tunnel: w3156 -> [w3161 w3179]
                      tunnel: w3155 -> [w3160 w3178]
                      tunnel: w3154 -> [_ w3177]
                      tunnel: w3153 -> [_ w3176]
                      tunnel: w3150 -> [_ w3175]
                      tunnel: w3149 -> [w3163 _]
                      tunnel: w3148 -> [w3159 w3173]
                      tunnel: w3147 -> [_ w3174]
                      tunnel: w3146 -> [_ w3169]
                      frame #0 {
                        n2007 = case shown="True" w3163 {
                          tunnel: w3162 -> [_ w3168]
                          tunnel: w3161 -> [_ w3167]
                          tunnel: w3160 -> [_ w3166]
                          tunnel: w3159 -> [_ w3164]
                          frame False {
                          }
                          frame True {
                            n2008 = Bundle(cluster=w3164, "amps"=w3168, "volts"=w3167, "pf"=w3166) -> (w3165:cluster{"amps":dbl, "volts":dbl, "pf":dbl})
                            n2009 = local write "ON L03-1"(w3165) -> ()
                          }
                        }
                      }
                      frame #1 {
                        n2010 = Unbundle(w3173) -> ("amps"=w3172:dbl, "volts"=w3171:dbl, "pf"=w3170:dbl)
                        n2011 = case shown="True" w3174 {
                          tunnel: w3181 -> [_ w3213]
                          tunnel: w3180 -> [_ w3220]
                          tunnel: w3179 -> [_ _]
                          tunnel: w3178 -> [_ _]
                          tunnel: w3177 -> [_ w3219]
                          tunnel: w3176 -> [_ w3218]
                          tunnel: w3175 -> [_ w3183]
                          tunnel: w3172 -> [_ w3215]
                          tunnel: w3171 -> [_ w3214]
                          tunnel: w3170 -> [_ w3212]
                          tunnel: w3169 -> [_ w3204]
                          frame False {
                          }
                          frame True {
                            n2012 = local read "TDMS LAB03-1"() -> (w3217:refnum<k34>)
                            n2013 = Build Array(w3214) -> (w3209:dbl[])
                            n2014 = Build Array(w3212) -> (w3208:dbl[])
                            n2015 = Build Array(w3219) -> (w3207:dbl[])
                            n2016 = Build Array(w3220) -> (w3206:dbl[])
                            n2017 = Build Array(w3215) -> (w3211:dbl[])
                            n2018 = Build Array(w3213) -> (w3210:dbl[])
                            n2019 = Build Array(w3218) -> (w3205:dbl[])
                            n2020 = Build Array("AMPS ON", "AMPS OFF", "VOLTS", "PF", "TEMP Live", "TEMP Neut", "CYCLE") -> (w3188:string[])
                            n2021 = Bundle By Name("Y"=w3211, "t0"=w3204) -> (w3203:waveform(dbl))  [unwired: 1 in]
                            n2022 = Bundle By Name("Y"=w3210, "t0"=w3204) -> (w3202:waveform(dbl))  [unwired: 1 in]
                            n2023 = Bundle By Name("Y"=w3209, "t0"=w3204) -> (w3201:waveform(dbl))  [unwired: 1 in]
                            n2024 = Bundle By Name("Y"=w3208, "t0"=w3204) -> (w3200:waveform(dbl))  [unwired: 1 in]
                            n2025 = Bundle By Name("Y"=w3207, "t0"=w3204) -> (w3199:waveform(dbl))  [unwired: 1 in]
                            n2026 = Bundle By Name("Y"=w3206, "t0"=w3204) -> (w3198:waveform(dbl))  [unwired: 1 in]
                            n2027 = Bundle By Name("Y"=w3205, "t0"=w3204) -> (w3197:waveform(dbl))  [unwired: 1 in]
                            n2028 = Build Array(w3203, w3202, w3201, w3200, w3199, w3198, w3197) -> (w3196:waveform(dbl)[])
                            n2029 = TDMS Write(0:w3217, 5:"TEST VALUES", 7:w3188, 9:w3196) -> (4:w3187:refnum<k34>, 6:w3186:string, 15:w3185:errorcluster)  [unwired: 2 in, 1 out]
                            n2030 = TDMS Write(0:w3187, 5:w3186, 7:"TIME", 9:w3183, 11:w3185) -> (15:w3182:errorcluster)  [unwired: 1 in, 3 out]
                            n2031 = local write "data file error"(w3182) -> ()
                          }
                        }
                      }
                    }
                  }
                }
              }
              frame #5 {
                n2032 = case shown="True" w3221 {
                  tunnel: w3225 -> [_ w3230]
                  tunnel: w3224 -> [_ w3229]
                  tunnel: w3223 -> [_ w3227]
                  tunnel: w3222 -> [_ w3226]
                  frame False {
                  }
                  frame True {
                    n2033 = local read "DISP LAB03-2"() -> (w3231:T4)
                    n2034 = local read "SIG LAB03-2"() -> (w3232:T2)
                    n2035 = local read "ON L03-2"() -> (w3228:cluster{"amps":dbl, "volts":dbl, "pf":dbl})
                    n2036 = Unbundle(w3232) -> ("AMPS"=w3238:dbl, "VOLTS"=w3236:dbl, "PF"=w3235:dbl, "Tmp Live"=w3234:dbl, "Tmp Neut"=w3237:dbl)
                    n2037 = Unbundle(w3231) -> ("CYCLE"=w3233:dbl)  [unwired: 2 out]
                    n2038 = stacked-sequence {
                      tunnel: w3238 -> [w3242 w3261]
                      tunnel: w3237 -> [_ w3260]
                      tunnel: w3236 -> [w3241 w3259]
                      tunnel: w3235 -> [w3240 w3258]
                      tunnel: w3234 -> [_ w3257]
                      tunnel: w3233 -> [_ w3256]
                      tunnel: w3230 -> [_ w3255]
                      tunnel: w3229 -> [w3243 _]
                      tunnel: w3228 -> [w3239 w3253]
                      tunnel: w3227 -> [_ w3254]
                      tunnel: w3226 -> [_ w3249]
                      frame #0 {
                        n2039 = case shown="True" w3243 {
                          tunnel: w3242 -> [_ w3248]
                          tunnel: w3241 -> [_ w3247]
                          tunnel: w3240 -> [_ w3246]
                          tunnel: w3239 -> [_ w3244]
                          frame False {
                          }
                          frame True {
                            n2040 = Bundle(cluster=w3244, "amps"=w3248, "volts"=w3247, "pf"=w3246) -> (w3245:cluster{"amps":dbl, "volts":dbl, "pf":dbl})
                            n2041 = local write "ON L03-2"(w3245) -> ()
                          }
                        }
                      }
                      frame #1 {
                        n2042 = Unbundle(w3253) -> ("amps"=w3252:dbl, "volts"=w3251:dbl, "pf"=w3250:dbl)
                        n2043 = case shown="True" w3254 {
                          tunnel: w3261 -> [_ w3293]
                          tunnel: w3260 -> [_ w3300]
                          tunnel: w3259 -> [_ _]
                          tunnel: w3258 -> [_ _]
                          tunnel: w3257 -> [_ w3299]
                          tunnel: w3256 -> [_ w3298]
                          tunnel: w3255 -> [_ w3263]
                          tunnel: w3252 -> [_ w3295]
                          tunnel: w3251 -> [_ w3294]
                          tunnel: w3250 -> [_ w3292]
                          tunnel: w3249 -> [_ w3284]
                          frame False {
                          }
                          frame True {
                            n2044 = local read "TDMS LAB03-2"() -> (w3297:refnum<k34>)
                            n2045 = Build Array(w3294) -> (w3289:dbl[])
                            n2046 = Build Array(w3292) -> (w3288:dbl[])
                            n2047 = Build Array(w3299) -> (w3287:dbl[])
                            n2048 = Build Array(w3300) -> (w3286:dbl[])
                            n2049 = Build Array(w3295) -> (w3291:dbl[])
                            n2050 = Build Array(w3293) -> (w3290:dbl[])
                            n2051 = Build Array(w3298) -> (w3285:dbl[])
                            n2052 = Build Array("AMPS ON", "AMPS OFF", "VOLTS", "PF", "TEMP Live", "TEMP Neut", "CYCLE") -> (w3268:string[])
                            n2053 = Bundle By Name("Y"=w3291, "t0"=w3284) -> (w3283:waveform(dbl))  [unwired: 1 in]
                            n2054 = Bundle By Name("Y"=w3290, "t0"=w3284) -> (w3282:waveform(dbl))  [unwired: 1 in]
                            n2055 = Bundle By Name("Y"=w3289, "t0"=w3284) -> (w3281:waveform(dbl))  [unwired: 1 in]
                            n2056 = Bundle By Name("Y"=w3288, "t0"=w3284) -> (w3280:waveform(dbl))  [unwired: 1 in]
                            n2057 = Bundle By Name("Y"=w3287, "t0"=w3284) -> (w3279:waveform(dbl))  [unwired: 1 in]
                            n2058 = Bundle By Name("Y"=w3286, "t0"=w3284) -> (w3278:waveform(dbl))  [unwired: 1 in]
                            n2059 = Bundle By Name("Y"=w3285, "t0"=w3284) -> (w3277:waveform(dbl))  [unwired: 1 in]
                            n2060 = Build Array(w3283, w3282, w3281, w3280, w3279, w3278, w3277) -> (w3276:waveform(dbl)[])
                            n2061 = TDMS Write(0:w3297, 5:"TEST VALUES", 7:w3268, 9:w3276) -> (4:w3267:refnum<k34>, 6:w3266:string, 15:w3265:errorcluster)  [unwired: 2 in, 1 out]
                            n2062 = TDMS Write(0:w3267, 5:w3266, 7:"TIME", 9:w3263, 11:w3265) -> (15:w3262:errorcluster)  [unwired: 1 in, 3 out]
                            n2063 = local write "data file error"(w3262) -> ()
                          }
                        }
                      }
                    }
                  }
                }
              }
              frame #6 {
                n2064 = case shown="True" w3301 {
                  tunnel: w3305 -> [_ w3310]
                  tunnel: w3304 -> [_ w3309]
                  tunnel: w3303 -> [_ w3307]
                  tunnel: w3302 -> [_ w3306]
                  frame False {
                  }
                  frame True {
                    n2065 = local read "DISP LAB04-1"() -> (w3311:T4)
                    n2066 = local read "SIG LAB04-1"() -> (w3312:T2)
                    n2067 = local read "ON L04-1"() -> (w3308:cluster{"amps":dbl, "volts":dbl, "pf":dbl})
                    n2068 = Unbundle(w3312) -> ("AMPS"=w3318:dbl, "VOLTS"=w3316:dbl, "PF"=w3315:dbl, "Tmp Live"=w3314:dbl, "Tmp Neut"=w3317:dbl)
                    n2069 = Unbundle(w3311) -> ("CYCLE"=w3313:dbl)  [unwired: 2 out]
                    n2070 = stacked-sequence {
                      tunnel: w3318 -> [w3322 w3341]
                      tunnel: w3317 -> [_ w3340]
                      tunnel: w3316 -> [w3321 w3339]
                      tunnel: w3315 -> [w3320 w3338]
                      tunnel: w3314 -> [_ w3337]
                      tunnel: w3313 -> [_ w3336]
                      tunnel: w3310 -> [_ w3335]
                      tunnel: w3309 -> [w3323 _]
                      tunnel: w3308 -> [w3319 w3333]
                      tunnel: w3307 -> [_ w3334]
                      tunnel: w3306 -> [_ w3329]
                      frame #0 {
                        n2071 = case shown="True" w3323 {
                          tunnel: w3322 -> [_ w3328]
                          tunnel: w3321 -> [_ w3327]
                          tunnel: w3320 -> [_ w3326]
                          tunnel: w3319 -> [_ w3324]
                          frame False {
                          }
                          frame True {
                            n2072 = Bundle(cluster=w3324, "amps"=w3328, "volts"=w3327, "pf"=w3326) -> (w3325:cluster{"amps":dbl, "volts":dbl, "pf":dbl})
                            n2073 = local write "ON L04-1"(w3325) -> ()
                          }
                        }
                      }
                      frame #1 {
                        n2074 = Unbundle(w3333) -> ("amps"=w3332:dbl, "volts"=w3331:dbl, "pf"=w3330:dbl)
                        n2075 = case shown="True" w3334 {
                          tunnel: w3341 -> [_ w3373]
                          tunnel: w3340 -> [_ w3380]
                          tunnel: w3339 -> [_ _]
                          tunnel: w3338 -> [_ _]
                          tunnel: w3337 -> [_ w3379]
                          tunnel: w3336 -> [_ w3378]
                          tunnel: w3335 -> [_ w3343]
                          tunnel: w3332 -> [_ w3375]
                          tunnel: w3331 -> [_ w3374]
                          tunnel: w3330 -> [_ w3372]
                          tunnel: w3329 -> [_ w3364]
                          frame False {
                          }
                          frame True {
                            n2076 = local read "TDMS LAB04-1"() -> (w3377:refnum<k34>)
                            n2077 = Build Array(w3374) -> (w3369:dbl[])
                            n2078 = Build Array(w3372) -> (w3368:dbl[])
                            n2079 = Build Array(w3379) -> (w3367:dbl[])
                            n2080 = Build Array(w3380) -> (w3366:dbl[])
                            n2081 = Build Array(w3375) -> (w3371:dbl[])
                            n2082 = Build Array(w3373) -> (w3370:dbl[])
                            n2083 = Build Array(w3378) -> (w3365:dbl[])
                            n2084 = Build Array("AMPS ON", "AMPS OFF", "VOLTS", "PF", "TEMP Live", "TEMP Neut", "CYCLE") -> (w3348:string[])
                            n2085 = Bundle By Name("Y"=w3371, "t0"=w3364) -> (w3363:waveform(dbl))  [unwired: 1 in]
                            n2086 = Bundle By Name("Y"=w3370, "t0"=w3364) -> (w3362:waveform(dbl))  [unwired: 1 in]
                            n2087 = Bundle By Name("Y"=w3369, "t0"=w3364) -> (w3361:waveform(dbl))  [unwired: 1 in]
                            n2088 = Bundle By Name("Y"=w3368, "t0"=w3364) -> (w3360:waveform(dbl))  [unwired: 1 in]
                            n2089 = Bundle By Name("Y"=w3367, "t0"=w3364) -> (w3359:waveform(dbl))  [unwired: 1 in]
                            n2090 = Bundle By Name("Y"=w3366, "t0"=w3364) -> (w3358:waveform(dbl))  [unwired: 1 in]
                            n2091 = Bundle By Name("Y"=w3365, "t0"=w3364) -> (w3357:waveform(dbl))  [unwired: 1 in]
                            n2092 = Build Array(w3363, w3362, w3361, w3360, w3359, w3358, w3357) -> (w3356:waveform(dbl)[])
                            n2093 = TDMS Write(0:w3377, 5:"TEST VALUES", 7:w3348, 9:w3356) -> (4:w3347:refnum<k34>, 6:w3346:string, 15:w3345:errorcluster)  [unwired: 2 in, 1 out]
                            n2094 = TDMS Write(0:w3347, 5:w3346, 7:"TIME", 9:w3343, 11:w3345) -> (15:w3342:errorcluster)  [unwired: 1 in, 3 out]
                            n2095 = local write "data file error"(w3342) -> ()
                          }
                        }
                      }
                    }
                  }
                }
              }
              frame #7 {
                n2096 = case shown="True" w3381 {
                  tunnel: w3385 -> [_ w3390]
                  tunnel: w3384 -> [_ w3389]
                  tunnel: w3383 -> [_ w3387]
                  tunnel: w3382 -> [_ w3386]
                  frame False {
                  }
                  frame True {
                    n2097 = local read "DISP LAB04-2"() -> (w3391:T4)
                    n2098 = local read "SIG LAB04-2"() -> (w3392:T2)
                    n2099 = local read "ON L04-2"() -> (w3388:cluster{"amps":dbl, "volts":dbl, "pf":dbl})
                    n2100 = Unbundle(w3392) -> ("AMPS"=w3398:dbl, "VOLTS"=w3396:dbl, "PF"=w3395:dbl, "Tmp Live"=w3394:dbl, "Tmp Neut"=w3397:dbl)
                    n2101 = Unbundle(w3391) -> ("CYCLE"=w3393:dbl)  [unwired: 2 out]
                    n2102 = stacked-sequence {
                      tunnel: w3398 -> [w3402 w3421]
                      tunnel: w3397 -> [_ w3420]
                      tunnel: w3396 -> [w3401 w3419]
                      tunnel: w3395 -> [w3400 w3418]
                      tunnel: w3394 -> [_ w3417]
                      tunnel: w3393 -> [_ w3416]
                      tunnel: w3390 -> [_ w3415]
                      tunnel: w3389 -> [w3403 _]
                      tunnel: w3388 -> [w3399 w3413]
                      tunnel: w3387 -> [_ w3414]
                      tunnel: w3386 -> [_ w3409]
                      frame #0 {
                        n2103 = case shown="True" w3403 {
                          tunnel: w3402 -> [_ w3408]
                          tunnel: w3401 -> [_ w3407]
                          tunnel: w3400 -> [_ w3406]
                          tunnel: w3399 -> [_ w3404]
                          frame False {
                          }
                          frame True {
                            n2104 = Bundle(cluster=w3404, "amps"=w3408, "volts"=w3407, "pf"=w3406) -> (w3405:cluster{"amps":dbl, "volts":dbl, "pf":dbl})
                            n2105 = local write "ON L04-2"(w3405) -> ()
                          }
                        }
                      }
                      frame #1 {
                        n2106 = Unbundle(w3413) -> ("amps"=w3412:dbl, "volts"=w3411:dbl, "pf"=w3410:dbl)
                        n2107 = case shown="True" w3414 {
                          tunnel: w3421 -> [_ w3453]
                          tunnel: w3420 -> [_ w3460]
                          tunnel: w3419 -> [_ _]
                          tunnel: w3418 -> [_ _]
                          tunnel: w3417 -> [_ w3459]
                          tunnel: w3416 -> [_ w3458]
                          tunnel: w3415 -> [_ w3423]
                          tunnel: w3412 -> [_ w3455]
                          tunnel: w3411 -> [_ w3454]
                          tunnel: w3410 -> [_ w3452]
                          tunnel: w3409 -> [_ w3444]
                          frame False {
                          }
                          frame True {
                            n2108 = local read "TDMS LAB04-2"() -> (w3457:refnum<k34>)
                            n2109 = Build Array(w3454) -> (w3449:dbl[])
                            n2110 = Build Array(w3452) -> (w3448:dbl[])
                            n2111 = Build Array(w3459) -> (w3447:dbl[])
                            n2112 = Build Array(w3460) -> (w3446:dbl[])
                            n2113 = Build Array(w3455) -> (w3451:dbl[])
                            n2114 = Build Array(w3453) -> (w3450:dbl[])
                            n2115 = Build Array(w3458) -> (w3445:dbl[])
                            n2116 = Build Array("AMPS ON", "AMPS OFF", "VOLTS", "PF", "TEMP Live", "TEMP Neut", "CYCLE") -> (w3428:string[])
                            n2117 = Bundle By Name("Y"=w3451, "t0"=w3444) -> (w3443:waveform(dbl))  [unwired: 1 in]
                            n2118 = Bundle By Name("Y"=w3450, "t0"=w3444) -> (w3442:waveform(dbl))  [unwired: 1 in]
                            n2119 = Bundle By Name("Y"=w3449, "t0"=w3444) -> (w3441:waveform(dbl))  [unwired: 1 in]
                            n2120 = Bundle By Name("Y"=w3448, "t0"=w3444) -> (w3440:waveform(dbl))  [unwired: 1 in]
                            n2121 = Bundle By Name("Y"=w3447, "t0"=w3444) -> (w3439:waveform(dbl))  [unwired: 1 in]
                            n2122 = Bundle By Name("Y"=w3446, "t0"=w3444) -> (w3438:waveform(dbl))  [unwired: 1 in]
                            n2123 = Bundle By Name("Y"=w3445, "t0"=w3444) -> (w3437:waveform(dbl))  [unwired: 1 in]
                            n2124 = Build Array(w3443, w3442, w3441, w3440, w3439, w3438, w3437) -> (w3436:waveform(dbl)[])
                            n2125 = TDMS Write(0:w3457, 5:"TEST VALUES", 7:w3428, 9:w3436) -> (4:w3427:refnum<k34>, 6:w3426:string, 15:w3425:errorcluster)  [unwired: 2 in, 1 out]
                            n2126 = TDMS Write(0:w3427, 5:w3426, 7:"TIME", 9:w3423, 11:w3425) -> (15:w3422:errorcluster)  [unwired: 1 in, 3 out]
                            n2127 = local write "data file error"(w3422) -> ()
                          }
                        }
                      }
                    }
                  }
                }
              }
              frame #8 {
                n2128 = case shown="True" w3461 {
                  tunnel: w3465 -> [_ w3470]
                  tunnel: w3464 -> [_ w3469]
                  tunnel: w3463 -> [_ w3467]
                  tunnel: w3462 -> [_ w3466]
                  frame False {
                  }
                  frame True {
                    n2129 = local read "DISP LAB05-1"() -> (w3471:T4)
                    n2130 = local read "SIG LAB05-1"() -> (w3472:T2)
                    n2131 = local read "ON L05-1"() -> (w3468:cluster{"amps":dbl, "volts":dbl, "pf":dbl})
                    n2132 = Unbundle(w3472) -> ("AMPS"=w3478:dbl, "VOLTS"=w3476:dbl, "PF"=w3475:dbl, "Tmp Live"=w3474:dbl, "Tmp Neut"=w3477:dbl)
                    n2133 = Unbundle(w3471) -> ("CYCLE"=w3473:dbl)  [unwired: 2 out]
                    n2134 = stacked-sequence {
                      tunnel: w3478 -> [w3482 w3501]
                      tunnel: w3477 -> [_ w3500]
                      tunnel: w3476 -> [w3481 w3499]
                      tunnel: w3475 -> [w3480 w3498]
                      tunnel: w3474 -> [_ w3497]
                      tunnel: w3473 -> [_ w3496]
                      tunnel: w3470 -> [_ w3495]
                      tunnel: w3469 -> [w3483 _]
                      tunnel: w3468 -> [w3479 w3493]
                      tunnel: w3467 -> [_ w3494]
                      tunnel: w3466 -> [_ w3489]
                      frame #0 {
                        n2135 = case shown="True" w3483 {
                          tunnel: w3482 -> [_ w3488]
                          tunnel: w3481 -> [_ w3487]
                          tunnel: w3480 -> [_ w3486]
                          tunnel: w3479 -> [_ w3484]
                          frame False {
                          }
                          frame True {
                            n2136 = Bundle(cluster=w3484, "amps"=w3488, "volts"=w3487, "pf"=w3486) -> (w3485:cluster{"amps":dbl, "volts":dbl, "pf":dbl})
                            n2137 = local write "ON L05-1"(w3485) -> ()
                          }
                        }
                      }
                      frame #1 {
                        n2138 = Unbundle(w3493) -> ("amps"=w3492:dbl, "volts"=w3491:dbl, "pf"=w3490:dbl)
                        n2139 = case shown="True" w3494 {
                          tunnel: w3501 -> [_ w3533]
                          tunnel: w3500 -> [_ w3540]
                          tunnel: w3499 -> [_ _]
                          tunnel: w3498 -> [_ _]
                          tunnel: w3497 -> [_ w3539]
                          tunnel: w3496 -> [_ w3538]
                          tunnel: w3495 -> [_ w3503]
                          tunnel: w3492 -> [_ w3535]
                          tunnel: w3491 -> [_ w3534]
                          tunnel: w3490 -> [_ w3532]
                          tunnel: w3489 -> [_ w3524]
                          frame False {
                          }
                          frame True {
                            n2140 = local read "TDMS LAB05-1"() -> (w3537:refnum<k34>)
                            n2141 = Build Array(w3534) -> (w3529:dbl[])
                            n2142 = Build Array(w3532) -> (w3528:dbl[])
                            n2143 = Build Array(w3539) -> (w3527:dbl[])
                            n2144 = Build Array(w3540) -> (w3526:dbl[])
                            n2145 = Build Array(w3535) -> (w3531:dbl[])
                            n2146 = Build Array(w3533) -> (w3530:dbl[])
                            n2147 = Build Array(w3538) -> (w3525:dbl[])
                            n2148 = Build Array("AMPS ON", "AMPS OFF", "VOLTS", "PF", "TEMP Live", "TEMP Neut", "CYCLE") -> (w3508:string[])
                            n2149 = Bundle By Name("Y"=w3531, "t0"=w3524) -> (w3523:waveform(dbl))  [unwired: 1 in]
                            n2150 = Bundle By Name("Y"=w3530, "t0"=w3524) -> (w3522:waveform(dbl))  [unwired: 1 in]
                            n2151 = Bundle By Name("Y"=w3529, "t0"=w3524) -> (w3521:waveform(dbl))  [unwired: 1 in]
                            n2152 = Bundle By Name("Y"=w3528, "t0"=w3524) -> (w3520:waveform(dbl))  [unwired: 1 in]
                            n2153 = Bundle By Name("Y"=w3527, "t0"=w3524) -> (w3519:waveform(dbl))  [unwired: 1 in]
                            n2154 = Bundle By Name("Y"=w3526, "t0"=w3524) -> (w3518:waveform(dbl))  [unwired: 1 in]
                            n2155 = Bundle By Name("Y"=w3525, "t0"=w3524) -> (w3517:waveform(dbl))  [unwired: 1 in]
                            n2156 = Build Array(w3523, w3522, w3521, w3520, w3519, w3518, w3517) -> (w3516:waveform(dbl)[])
                            n2157 = TDMS Write(0:w3537, 5:"TEST VALUES", 7:w3508, 9:w3516) -> (4:w3507:refnum<k34>, 6:w3506:string, 15:w3505:errorcluster)  [unwired: 2 in, 1 out]
                            n2158 = TDMS Write(0:w3507, 5:w3506, 7:"TIME", 9:w3503, 11:w3505) -> (15:w3502:errorcluster)  [unwired: 1 in, 3 out]
                            n2159 = local write "data file error"(w3502) -> ()
                          }
                        }
                      }
                    }
                  }
                }
              }
              frame #9 {
                n2160 = case shown="True" w3541 {
                  tunnel: w3545 -> [_ w3550]
                  tunnel: w3544 -> [_ w3549]
                  tunnel: w3543 -> [_ w3547]
                  tunnel: w3542 -> [_ w3546]
                  frame False {
                  }
                  frame True {
                    n2161 = local read "DISP LAB05-2"() -> (w3551:T4)
                    n2162 = local read "SIG LAB05-2"() -> (w3552:T2)
                    n2163 = local read "ON L05-2"() -> (w3548:cluster{"amps":dbl, "volts":dbl, "pf":dbl})
                    n2164 = Unbundle(w3552) -> ("AMPS"=w3558:dbl, "VOLTS"=w3556:dbl, "PF"=w3555:dbl, "Tmp Live"=w3554:dbl, "Tmp Neut"=w3557:dbl)
                    n2165 = Unbundle(w3551) -> ("CYCLE"=w3553:dbl)  [unwired: 2 out]
                    n2166 = stacked-sequence {
                      tunnel: w3558 -> [w3562 w3581]
                      tunnel: w3557 -> [_ w3580]
                      tunnel: w3556 -> [w3561 w3579]
                      tunnel: w3555 -> [w3560 w3578]
                      tunnel: w3554 -> [_ w3577]
                      tunnel: w3553 -> [_ w3576]
                      tunnel: w3550 -> [_ w3575]
                      tunnel: w3549 -> [w3563 _]
                      tunnel: w3548 -> [w3559 w3573]
                      tunnel: w3547 -> [_ w3574]
                      tunnel: w3546 -> [_ w3569]
                      frame #0 {
                        n2167 = case shown="True" w3563 {
                          tunnel: w3562 -> [_ w3568]
                          tunnel: w3561 -> [_ w3567]
                          tunnel: w3560 -> [_ w3566]
                          tunnel: w3559 -> [_ w3564]
                          frame False {
                          }
                          frame True {
                            n2168 = Bundle(cluster=w3564, "amps"=w3568, "volts"=w3567, "pf"=w3566) -> (w3565:cluster{"amps":dbl, "volts":dbl, "pf":dbl})
                            n2169 = local write "ON L05-2"(w3565) -> ()
                          }
                        }
                      }
                      frame #1 {
                        n2170 = Unbundle(w3573) -> ("amps"=w3572:dbl, "volts"=w3571:dbl, "pf"=w3570:dbl)
                        n2171 = case shown="True" w3574 {
                          tunnel: w3581 -> [_ w3613]
                          tunnel: w3580 -> [_ w3620]
                          tunnel: w3579 -> [_ _]
                          tunnel: w3578 -> [_ _]
                          tunnel: w3577 -> [_ w3619]
                          tunnel: w3576 -> [_ w3618]
                          tunnel: w3575 -> [_ w3583]
                          tunnel: w3572 -> [_ w3615]
                          tunnel: w3571 -> [_ w3614]
                          tunnel: w3570 -> [_ w3612]
                          tunnel: w3569 -> [_ w3604]
                          frame False {
                          }
                          frame True {
                            n2172 = local read "TDMS LAB05-2"() -> (w3617:refnum<k34>)
                            n2173 = Build Array(w3614) -> (w3609:dbl[])
                            n2174 = Build Array(w3612) -> (w3608:dbl[])
                            n2175 = Build Array(w3619) -> (w3607:dbl[])
                            n2176 = Build Array(w3620) -> (w3606:dbl[])
                            n2177 = Build Array(w3615) -> (w3611:dbl[])
                            n2178 = Build Array(w3613) -> (w3610:dbl[])
                            n2179 = Build Array(w3618) -> (w3605:dbl[])
                            n2180 = Build Array("AMPS ON", "AMPS OFF", "VOLTS", "PF", "TEMP Live", "TEMP Neut", "CYCLE") -> (w3588:string[])
                            n2181 = Bundle By Name("Y"=w3611, "t0"=w3604) -> (w3603:waveform(dbl))  [unwired: 1 in]
                            n2182 = Bundle By Name("Y"=w3610, "t0"=w3604) -> (w3602:waveform(dbl))  [unwired: 1 in]
                            n2183 = Bundle By Name("Y"=w3609, "t0"=w3604) -> (w3601:waveform(dbl))  [unwired: 1 in]
                            n2184 = Bundle By Name("Y"=w3608, "t0"=w3604) -> (w3600:waveform(dbl))  [unwired: 1 in]
                            n2185 = Bundle By Name("Y"=w3607, "t0"=w3604) -> (w3599:waveform(dbl))  [unwired: 1 in]
                            n2186 = Bundle By Name("Y"=w3606, "t0"=w3604) -> (w3598:waveform(dbl))  [unwired: 1 in]
                            n2187 = Bundle By Name("Y"=w3605, "t0"=w3604) -> (w3597:waveform(dbl))  [unwired: 1 in]
                            n2188 = Build Array(w3603, w3602, w3601, w3600, w3599, w3598, w3597) -> (w3596:waveform(dbl)[])
                            n2189 = TDMS Write(0:w3617, 5:"TEST VALUES", 7:w3588, 9:w3596) -> (4:w3587:refnum<k34>, 6:w3586:string, 15:w3585:errorcluster)  [unwired: 2 in, 1 out]
                            n2190 = TDMS Write(0:w3587, 5:w3586, 7:"TIME", 9:w3583, 11:w3585) -> (15:w3582:errorcluster)  [unwired: 1 in, 3 out]
                            n2191 = local write "data file error"(w3582) -> ()
                          }
                        }
                      }
                    }
                  }
                }
              }
            }
          }
          frame #14 {
            # "display test values on chart"
            n2192 = case shown="\"OFF CYCLE\"" "Select  Cycle" {
              tunnel: [1 w3626] -> w3621
              frame "ON CYCLE", Default {
              }
              frame "OFF CYCLE" {
                n2193 = local read "on loops"() -> (w3628:dbl)
                n2194 = Add(x=w3628, y=2) -> (x+y=w3626:dbl)
              }
            }
            n2195 = local read "jig cycle"() -> (w3623:dbl)
            n2196 = Equal?(x=w3623, y=w3621) -> (x = y?=w3624:bool)
            n2197 = case shown="True" w3624 {
              frame False {
              }
              frame True {
                n2198 = local read "SIG LAB05-1"() -> (w3670:T2)
                n2199 = local read "SIG LAB04-2"() -> (w3671:T2)
                n2200 = local read "SIG LAB05-2"() -> (w3669:T2)
                n2201 = local read "SIG LAB04-1"() -> (w3672:T2)
                n2202 = local read "SIG LAB03-1"() -> (w3674:T2)
                n2203 = local read "SIG LAB03-2"() -> (w3673:T2)
                n2204 = local read "SIG LAB01-1"() -> (w3678:T2)
                n2205 = local read "SIG LAB02-2"() -> (w3675:T2)
                n2206 = local read "SIG LAB02-1"() -> (w3676:T2)
                n2207 = local read "SIG LAB01-2"() -> (w3677:T2)
                n2208 = Unbundle(w3671) -> ("AMPS"=w3661:dbl, "VOLTS"=w3651:dbl, "Tmp Live"=w3641:dbl, "Tmp Neut"=w3631:dbl)  [unwired: 1 out]
                n2209 = Unbundle(w3670) -> ("AMPS"=w3660:dbl, "VOLTS"=w3650:dbl, "Tmp Live"=w3640:dbl, "Tmp Neut"=w3630:dbl)  [unwired: 1 out]
                n2210 = Unbundle(w3669) -> ("AMPS"=w3659:dbl, "VOLTS"=w3649:dbl, "Tmp Live"=w3639:dbl, "Tmp Neut"=w3629:dbl)  [unwired: 1 out]
                n2211 = Unbundle(w3672) -> ("AMPS"=w3662:dbl, "VOLTS"=w3652:dbl, "Tmp Live"=w3642:dbl, "Tmp Neut"=w3632:dbl)  [unwired: 1 out]
                n2212 = Unbundle(w3673) -> ("AMPS"=w3663:dbl, "VOLTS"=w3653:dbl, "Tmp Live"=w3643:dbl, "Tmp Neut"=w3633:dbl)  [unwired: 1 out]
                n2213 = Unbundle(w3674) -> ("AMPS"=w3664:dbl, "VOLTS"=w3654:dbl, "Tmp Live"=w3644:dbl, "Tmp Neut"=w3634:dbl)  [unwired: 1 out]
                n2214 = Unbundle(w3675) -> ("AMPS"=w3665:dbl, "VOLTS"=w3655:dbl, "Tmp Live"=w3645:dbl, "Tmp Neut"=w3635:dbl)  [unwired: 1 out]
                n2215 = Unbundle(w3676) -> ("AMPS"=w3666:dbl, "VOLTS"=w3656:dbl, "Tmp Live"=w3646:dbl, "Tmp Neut"=w3636:dbl)  [unwired: 1 out]
                n2216 = Unbundle(w3678) -> ("AMPS"=w3668:dbl, "VOLTS"=w3658:dbl, "Tmp Live"=w3648:dbl, "Tmp Neut"=w3638:dbl)  [unwired: 1 out]
                n2217 = Unbundle(w3677) -> ("AMPS"=w3667:dbl, "VOLTS"=w3657:dbl, "Tmp Live"=w3647:dbl, "Tmp Neut"=w3637:dbl)  [unwired: 1 out]
                n2218 = stacked-sequence {
                  tunnel: w3668 -> [w3689 _ _ _]
                  tunnel: w3667 -> [w3688 _ _ _]
                  tunnel: w3666 -> [w3687 _ _ _]
                  tunnel: w3665 -> [w3686 _ _ _]
                  tunnel: w3664 -> [w3685 _ _ _]
                  tunnel: w3663 -> [w3684 _ _ _]
                  tunnel: w3662 -> [w3683 _ _ _]
                  tunnel: w3661 -> [w3682 _ _ _]
                  tunnel: w3660 -> [w3681 _ _ _]
                  tunnel: w3659 -> [w3680 _ _ _]
                  tunnel: w3658 -> [_ w3700 _ _]
                  tunnel: w3657 -> [_ w3699 _ _]
                  tunnel: w3656 -> [_ w3698 _ _]
                  tunnel: w3655 -> [_ w3697 _ _]
                  tunnel: w3654 -> [_ w3696 _ _]
                  tunnel: w3653 -> [_ w3695 _ _]
                  tunnel: w3652 -> [_ w3694 _ _]
                  tunnel: w3651 -> [_ w3693 _ _]
                  tunnel: w3650 -> [_ w3692 _ _]
                  tunnel: w3649 -> [_ w3691 _ _]
                  tunnel: w3648 -> [_ _ w3711 _]
                  tunnel: w3647 -> [_ _ w3710 _]
                  tunnel: w3646 -> [_ _ w3709 _]
                  tunnel: w3645 -> [_ _ w3708 _]
                  tunnel: w3644 -> [_ _ w3707 _]
                  tunnel: w3643 -> [_ _ w3706 _]
                  tunnel: w3642 -> [_ _ w3705 _]
                  tunnel: w3641 -> [_ _ w3704 _]
                  tunnel: w3640 -> [_ _ w3703 _]
                  tunnel: w3639 -> [_ _ w3702 _]
                  tunnel: w3638 -> [_ _ _ w3722]
                  tunnel: w3637 -> [_ _ _ w3721]
                  tunnel: w3636 -> [_ _ _ w3720]
                  tunnel: w3635 -> [_ _ _ w3719]
                  tunnel: w3634 -> [_ _ _ w3718]
                  tunnel: w3633 -> [_ _ _ w3717]
                  tunnel: w3632 -> [_ _ _ w3716]
                  tunnel: w3631 -> [_ _ _ w3715]
                  tunnel: w3630 -> [_ _ _ w3714]
                  tunnel: w3629 -> [_ _ _ w3713]
                  frame #0 {
                    n2219 = Bundle("AMPS"=w3689, "AMPS"=w3688, "AMPS"=w3687, "AMPS"=w3686, "AMPS"=w3685, "AMPS"=w3684, "AMPS"=w3683, "AMPS"=w3682, "AMPS"=w3681, "AMPS"=w3680) -> (→"TEST AMPS CHART":T9)  [unwired: 1 in]
                  }
                  frame #1 {
                    n2220 = Bundle("VOLTS"=w3700, "VOLTS"=w3699, "VOLTS"=w3698, "VOLTS"=w3697, "VOLTS"=w3696, "VOLTS"=w3695, "VOLTS"=w3694, "VOLTS"=w3693, "VOLTS"=w3692, "VOLTS"=w3691) -> (→"TEST VOLTS CHART":T27)  [unwired: 1 in]
                  }
                  frame #2 {
                    n2221 = Bundle("Tmp Live"=w3711, "Tmp Live"=w3710, "Tmp Live"=w3709, "Tmp Live"=w3708, "Tmp Live"=w3707, "Tmp Live"=w3706, "Tmp Live"=w3705, "Tmp Live"=w3704, "Tmp Live"=w3703, "Tmp Live"=w3702) -> (→"TEMPERATURE (L) CHART":T28)  [unwired: 1 in]
                  }
                  frame #3 {
                    n2222 = Bundle("Tmp Neut"=w3722, "Tmp Neut"=w3721, "Tmp Neut"=w3720, "Tmp Neut"=w3719, "Tmp Neut"=w3718, "Tmp Neut"=w3717, "Tmp Neut"=w3716, "Tmp Neut"=w3715, "Tmp Neut"=w3714, "Tmp Neut"=w3713) -> (→"TEMPERATURE (N) CHART":T29)  [unwired: 1 in]
                  }
                }
              }
            }
          }
          frame #15 {
            # "check for amps fail"
            # "check for cycle test & temperature rise fail conditions"
            n2223 = local read "on loops"() -> (w3748:dbl)
            n2224 = local read "jig cycle"() -> (w3745:dbl)
            n2225 = local read "jig cycle"() -> (w3750:dbl)
            n2226 = Add(x=w3748, y=3.0) -> (x+y=w3746:dbl)
            n2227 = Equal?(x=w3745, y=w3746) -> (x = y?=w3741:bool)
            n2228 = Equal?(x=w3750, y=1.0) -> (x = y?=w3743:bool)
            n2229 = stacked-sequence {
              tunnel: w3744 -> [w3753 _ _ _ _ _ _ _ _ _]
              tunnel: w3743 -> [w3754 w3774 w3794 w3814 w3834 w3854 w3874 w3894 w3914 w3934]
              tunnel: w3742 -> [w3751 _ _ _ _ _ _ _ _ _]
              tunnel: w3741 -> [w3752 w3773 w3793 w3813 w3833 w3853 w3873 w3893 w3913 w3933]
              tunnel: w3740 -> [_ w3772 _ _ _ _ _ _ _ _]
              tunnel: w3739 -> [_ w3771 _ _ _ _ _ _ _ _]
              tunnel: w3738 -> [_ _ w3792 _ _ _ _ _ _ _]
              tunnel: w3737 -> [_ _ w3791 _ _ _ _ _ _ _]
              tunnel: w3736 -> [_ _ _ w3812 _ _ _ _ _ _]
              tunnel: w3735 -> [_ _ _ w3811 _ _ _ _ _ _]
              tunnel: w3734 -> [_ _ _ _ w3832 _ _ _ _ _]
              tunnel: w3733 -> [_ _ _ _ w3831 _ _ _ _ _]
              tunnel: w3732 -> [_ _ _ _ _ w3852 _ _ _ _]
              tunnel: w3731 -> [_ _ _ _ _ w3851 _ _ _ _]
              tunnel: w3730 -> [_ _ _ _ _ _ w3872 _ _ _]
              tunnel: w3729 -> [_ _ _ _ _ _ w3871 _ _ _]
              tunnel: w3728 -> [_ _ _ _ _ _ _ w3892 _ _]
              tunnel: w3727 -> [_ _ _ _ _ _ _ w3891 _ _]
              tunnel: w3726 -> [_ _ _ _ _ _ _ _ w3912 _]
              tunnel: w3725 -> [_ _ _ _ _ _ _ _ w3911 _]
              tunnel: w3724 -> [_ _ _ _ _ _ _ _ _ w3932]
              tunnel: w3723 -> [_ _ _ _ _ _ _ _ _ w3931]
              frame #0 {
                # "LAB01-1"
                n2230 = case shown="True" w3751 {
                  tunnel: w3754 -> [_ w3767]
                  tunnel: w3753 -> [_ w3764]
                  tunnel: w3752 -> [_ w3763]
                  frame False {
                  }
                  frame True {
                    n2231 = local read "TEMP START LAB01-1"() -> (w3769:cluster{"TL":dbl, "TN":dbl})
                    n2232 = local read "RESULT LAB01-1"() -> (w3758:bool)
                    n2233 = local read "FAIL LAB01-1"() -> (w3761:cluster{"LO":dbl, "HI":dbl})
                    n2234 = local read "TDMS LAB01-1"() -> (w3768:refnum<k34>)
                    n2235 = local read "SET LAB01-1"() -> (w3765:T5)
                    n2236 = local read "DISP LAB01-1"() -> (w3766:T4)
                    n2237 = local read "SIG LAB01-1"() -> (w3770:T2)
                    n2238 = Bundle("FAIL LAB01-1"=w3761, "SIG LAB01-1"=w3770, "TEMP START LAB01-1"=w3769, "DISP LAB01-1"=w3766, "SET LAB01-1"=w3765, "TDMS LAB01-1"=w3768) -> (w3755:T30)  [unwired: 1 in]
                    n2239 = call "sub vi - cycle&temp fail v6.vi"("Amps Lo?"=w3767, "Input Cluster"=w3755, "SELECT"=w3764, "Amps Hi?"=w3763, "Result In"=w3758) -> ("(FAIL) out"=w3760:cluster{"FAIL LO":dbl, "FAIL HI":dbl}, "(DISP) out"=w3756:T4, "T-RISE"=w3757:cluster{"T-RISE (L)":dbl, "T-RISE (N)":dbl}, "Result Out"=w3759:bool, "file error"=w3762:errorcluster)  [unwired: 10 in]
                    n2240 = local write "TEMP RISE LAB01-1"(w3757) -> ()
                    n2241 = local write "FAIL LAB01-1"(w3760) -> ()
                    n2242 = local write "DISP LAB01-1"(w3756) -> ()
                    n2243 = local write "RESULT LAB01-1"(w3759) -> ()
                    n2244 = local write "data file error"(w3762) -> ()
                  }
                }
              }
              frame #1 {
                # "LAB01-2"
                n2245 = case shown="True" w3772 {
                  tunnel: w3774 -> [_ w3787]
                  tunnel: w3771 -> [_ w3784]
                  tunnel: w3773 -> [_ w3783]
                  frame False {
                  }
                  frame True {
                    n2246 = local read "TEMP START LAB01-2"() -> (w3789:cluster{"TL":dbl, "TN":dbl})
                    n2247 = local read "FAIL LAB01-2"() -> (w3780:cluster{"LO":dbl, "HI":dbl})
                    n2248 = local read "TDMS LAB01-2"() -> (w3788:refnum<k34>)
                    n2249 = local read "SET LAB01-2"() -> (w3785:T5)
                    n2250 = local read "DISP LAB01-2"() -> (w3786:T4)
                    n2251 = local read "RESULT LAB01-2"() -> (w3777:bool)
                    n2252 = local read "SIG LAB01-2"() -> (w3790:T2)
                    n2253 = Bundle("FAIL LAB01-2"=w3780, "SIG LAB01-2"=w3790, "TEMP START LAB01-2"=w3789, "DISP LAB01-2"=w3786, "SET LAB01-2"=w3785, "TDMS LAB01-2"=w3788) -> (w3775:T31)  [unwired: 1 in]
                    n2254 = call "sub vi - cycle&temp fail v6.vi"("Amps Lo?"=w3787, "Input Cluster"=w3775, "SELECT"=w3784, "Amps Hi?"=w3783, "Result In"=w3777) -> ("(FAIL) out"=w3779:cluster{"FAIL LO":dbl, "FAIL HI":dbl}, "(DISP) out"=w3782:T4, "T-RISE"=w3776:cluster{"T-RISE (L)":dbl, "T-RISE (N)":dbl}, "Result Out"=w3778:bool, "file error"=w3781:errorcluster)  [unwired: 10 in]
                    n2255 = local write "TEMP RISE LAB01-2"(w3776) -> ()
                    n2256 = local write "FAIL LAB01-2"(w3779) -> ()
                    n2257 = local write "DISP LAB01-2"(w3782) -> ()
                    n2258 = local write "RESULT LAB01-2"(w3778) -> ()
                    n2259 = local write "data file error"(w3781) -> ()
                  }
                }
              }
              frame #2 {
                # "LAB02-1"
                n2260 = case shown="True" w3792 {
                  tunnel: w3794 -> [_ w3807]
                  tunnel: w3791 -> [_ w3804]
                  tunnel: w3793 -> [_ w3803]
                  frame False {
                  }
                  frame True {
                    n2261 = local read "TEMP START LAB02-1"() -> (w3809:cluster{"TL":dbl, "TN":dbl})
                    n2262 = local read "FAIL LAB02-1"() -> (w3800:cluster{"LO":dbl, "HI":dbl})
                    n2263 = local read "TDMS LAB02-1"() -> (w3808:refnum<k34>)
                    n2264 = local read "SET LAB02-1"() -> (w3805:T5)
                    n2265 = local read "DISP LAB02-1"() -> (w3806:T4)
                    n2266 = local read "SIG LAB02-1"() -> (w3810:T2)
                    n2267 = local read "RESULT LAB02-1"() -> (w3797:bool)
                    n2268 = Bundle("FAIL LAB02-1"=w3800, "SIG LAB02-1"=w3810, "TEMP START LAB02-1"=w3809, "DISP LAB02-1"=w3806, "SET LAB02-1"=w3805, "TDMS LAB02-1"=w3808) -> (w3795:T32)  [unwired: 1 in]
                    n2269 = call "sub vi - cycle&temp fail v6.vi"("Amps Lo?"=w3807, "Input Cluster"=w3795, "SELECT"=w3804, "Amps Hi?"=w3803, "Result In"=w3797) -> ("(FAIL) out"=w3799:cluster{"FAIL LO":dbl, "FAIL HI":dbl}, "(DISP) out"=w3802:T4, "T-RISE"=w3796:cluster{"T-RISE (L)":dbl, "T-RISE (N)":dbl}, "Result Out"=w3798:bool, "file error"=w3801:errorcluster)  [unwired: 10 in]
                    n2270 = local write "TEMP RISE LAB02-1"(w3796) -> ()
                    n2271 = local write "FAIL LAB02-1"(w3799) -> ()
                    n2272 = local write "DISP LAB02-1"(w3802) -> ()
                    n2273 = local write "RESULT LAB02-1"(w3798) -> ()
                    n2274 = local write "data file error"(w3801) -> ()
                  }
                }
              }
              frame #3 {
                # "LAB02-2"
                n2275 = case shown="True" w3812 {
                  tunnel: w3814 -> [_ w3827]
                  tunnel: w3811 -> [_ w3824]
                  tunnel: w3813 -> [_ w3823]
                  frame False {
                  }
                  frame True {
                    n2276 = local read "TEMP START LAB02-2"() -> (w3829:cluster{"TL":dbl, "TN":dbl})
                    n2277 = local read "FAIL LAB02-2"() -> (w3820:cluster{"LO":dbl, "HI":dbl})
                    n2278 = local read "TDMS LAB02-2"() -> (w3828:refnum<k34>)
                    n2279 = local read "SET LAB02-2"() -> (w3825:T5)
                    n2280 = local read "DISP LAB02-2"() -> (w3826:T4)
                    n2281 = local read "SIG LAB02-2"() -> (w3830:T2)
                    n2282 = local read "RESULT LAB02-2"() -> (w3817:bool)
                    n2283 = Bundle("FAIL LAB02-2"=w3820, "SIG LAB02-2"=w3830, "TEMP START LAB02-2"=w3829, "DISP LAB02-2"=w3826, "SET LAB02-2"=w3825, "TDMS LAB02-2"=w3828) -> (w3815:T33)  [unwired: 1 in]
                    n2284 = call "sub vi - cycle&temp fail v6.vi"("Amps Lo?"=w3827, "Input Cluster"=w3815, "SELECT"=w3824, "Amps Hi?"=w3823, "Result In"=w3817) -> ("(FAIL) out"=w3819:cluster{"FAIL LO":dbl, "FAIL HI":dbl}, "(DISP) out"=w3822:T4, "T-RISE"=w3816:cluster{"T-RISE (L)":dbl, "T-RISE (N)":dbl}, "Result Out"=w3818:bool, "file error"=w3821:errorcluster)  [unwired: 10 in]
                    n2285 = local write "TEMP RISE LAB02-2"(w3816) -> ()
                    n2286 = local write "FAIL LAB02-2"(w3819) -> ()
                    n2287 = local write "DISP LAB02-2"(w3822) -> ()
                    n2288 = local write "RESULT LAB02-2"(w3818) -> ()
                    n2289 = local write "data file error"(w3821) -> ()
                  }
                }
              }
              frame #4 {
                # "LAB03-1"
                n2290 = case shown="True" w3832 {
                  tunnel: w3834 -> [_ w3847]
                  tunnel: w3831 -> [_ w3844]
                  tunnel: w3833 -> [_ w3843]
                  frame False {
                  }
                  frame True {
                    n2291 = local read "TEMP START LAB03-1"() -> (w3849:cluster{"TL":dbl, "TN":dbl})
                    n2292 = local read "FAIL LAB03-1"() -> (w3840:cluster{"LO":dbl, "HI":dbl})
                    n2293 = local read "TDMS LAB03-1"() -> (w3848:refnum<k34>)
                    n2294 = local read "SET LAB03-1"() -> (w3845:T5)
                    n2295 = local read "DISP LAB03-1"() -> (w3846:T4)
                    n2296 = local read "SIG LAB03-1"() -> (w3850:T2)
                    n2297 = local read "RESULT LAB03-1"() -> (w3837:bool)
                    n2298 = Bundle("FAIL LAB03-1"=w3840, "SIG LAB03-1"=w3850, "TEMP START LAB03-1"=w3849, "DISP LAB03-1"=w3846, "SET LAB03-1"=w3845, "TDMS LAB03-1"=w3848) -> (w3835:T34)  [unwired: 1 in]
                    n2299 = call "sub vi - cycle&temp fail v6.vi"("Amps Lo?"=w3847, "Input Cluster"=w3835, "SELECT"=w3844, "Amps Hi?"=w3843, "Result In"=w3837) -> ("(FAIL) out"=w3839:cluster{"FAIL LO":dbl, "FAIL HI":dbl}, "(DISP) out"=w3842:T4, "T-RISE"=w3836:cluster{"T-RISE (L)":dbl, "T-RISE (N)":dbl}, "Result Out"=w3838:bool, "file error"=w3841:errorcluster)  [unwired: 10 in]
                    n2300 = local write "TEMP RISE LAB03-1"(w3836) -> ()
                    n2301 = local write "FAIL LAB03-1"(w3839) -> ()
                    n2302 = local write "DISP LAB03-1"(w3842) -> ()
                    n2303 = local write "RESULT LAB03-1"(w3838) -> ()
                    n2304 = local write "data file error"(w3841) -> ()
                  }
                }
              }
              frame #5 {
                # "LAB03-2"
                n2305 = case shown="True" w3852 {
                  tunnel: w3854 -> [_ w3867]
                  tunnel: w3851 -> [_ w3864]
                  tunnel: w3853 -> [_ w3863]
                  frame False {
                  }
                  frame True {
                    n2306 = local read "TEMP START LAB03-2"() -> (w3869:cluster{"TL":dbl, "TN":dbl})
                    n2307 = local read "FAIL LAB03-2"() -> (w3860:cluster{"LO":dbl, "HI":dbl})
                    n2308 = local read "TDMS LAB03-2"() -> (w3868:refnum<k34>)
                    n2309 = local read "SET LAB03-2"() -> (w3865:T5)
                    n2310 = local read "DISP LAB03-2"() -> (w3866:T4)
                    n2311 = local read "RESULT LAB03-2"() -> (w3857:bool)
                    n2312 = local read "SIG LAB03-2"() -> (w3870:T2)
                    n2313 = Bundle("FAIL LAB03-2"=w3860, "SIG LAB03-2"=w3870, "TEMP START LAB03-2"=w3869, "DISP LAB03-2"=w3866, "SET LAB03-2"=w3865, "TDMS LAB03-2"=w3868) -> (w3855:T35)  [unwired: 1 in]
                    n2314 = call "sub vi - cycle&temp fail v6.vi"("Amps Lo?"=w3867, "Input Cluster"=w3855, "SELECT"=w3864, "Amps Hi?"=w3863, "Result In"=w3857) -> ("(FAIL) out"=w3859:cluster{"FAIL LO":dbl, "FAIL HI":dbl}, "(DISP) out"=w3862:T4, "T-RISE"=w3856:cluster{"T-RISE (L)":dbl, "T-RISE (N)":dbl}, "Result Out"=w3858:bool, "file error"=w3861:errorcluster)  [unwired: 10 in]
                    n2315 = local write "FAIL LAB03-2"(w3859) -> ()
                    n2316 = local write "TEMP RISE LAB03-2"(w3856) -> ()
                    n2317 = local write "DISP LAB03-2"(w3862) -> ()
                    n2318 = local write "RESULT LAB03-2"(w3858) -> ()
                    n2319 = local write "data file error"(w3861) -> ()
                  }
                }
              }
              frame #6 {
                # "LAB04-1"
                n2320 = case shown="True" w3872 {
                  tunnel: w3874 -> [_ w3887]
                  tunnel: w3871 -> [_ w3884]
                  tunnel: w3873 -> [_ w3883]
                  frame False {
                  }
                  frame True {
                    n2321 = local read "TEMP START LAB04-1"() -> (w3889:cluster{"TL":dbl, "TN":dbl})
                    n2322 = local read "FAIL LAB04-1"() -> (w3880:cluster{"LO":dbl, "HI":dbl})
                    n2323 = local read "TDMS LAB04-1"() -> (w3888:refnum<k34>)
                    n2324 = local read "SET LAB04-1"() -> (w3885:T5)
                    n2325 = local read "DISP LAB04-1"() -> (w3886:T4)
                    n2326 = local read "SIG LAB04-1"() -> (w3890:T2)
                    n2327 = local read "RESULT LAB04-1"() -> (w3877:bool)
                    n2328 = Bundle("FAIL LAB04-1"=w3880, "SIG LAB04-1"=w3890, "TEMP START LAB04-1"=w3889, "DISP LAB04-1"=w3886, "SET LAB04-1"=w3885, "TDMS LAB04-1"=w3888) -> (w3875:T36)  [unwired: 1 in]
                    n2329 = call "sub vi - cycle&temp fail v6.vi"("Amps Lo?"=w3887, "Input Cluster"=w3875, "SELECT"=w3884, "Amps Hi?"=w3883, "Result In"=w3877) -> ("(FAIL) out"=w3879:cluster{"FAIL LO":dbl, "FAIL HI":dbl}, "(DISP) out"=w3882:T4, "T-RISE"=w3876:cluster{"T-RISE (L)":dbl, "T-RISE (N)":dbl}, "Result Out"=w3878:bool, "file error"=w3881:errorcluster)  [unwired: 10 in]
                    n2330 = local write "TEMP RISE LAB04-1"(w3876) -> ()
                    n2331 = local write "FAIL LAB04-1"(w3879) -> ()
                    n2332 = local write "DISP LAB04-1"(w3882) -> ()
                    n2333 = local write "RESULT LAB04-1"(w3878) -> ()
                    n2334 = local write "data file error"(w3881) -> ()
                  }
                }
              }
              frame #7 {
                # "LAB04-2"
                n2335 = case shown="True" w3892 {
                  tunnel: w3894 -> [_ w3907]
                  tunnel: w3891 -> [_ w3904]
                  tunnel: w3893 -> [_ w3903]
                  frame False {
                  }
                  frame True {
                    n2336 = local read "TEMP START LAB04-2"() -> (w3909:cluster{"TL":dbl, "TN":dbl})
                    n2337 = local read "FAIL LAB04-2"() -> (w3900:cluster{"LO":dbl, "HI":dbl})
                    n2338 = local read "TDMS LAB04-2"() -> (w3908:refnum<k34>)
                    n2339 = local read "SET LAB04-2"() -> (w3905:T5)
                    n2340 = local read "DISP LAB04-2"() -> (w3906:T4)
                    n2341 = local read "SIG LAB04-2"() -> (w3910:T2)
                    n2342 = local read "RESULT LAB04-2"() -> (w3897:bool)
                    n2343 = Bundle("FAIL LAB04-2"=w3900, "SIG LAB04-2"=w3910, "TEMP START LAB04-2"=w3909, "DISP LAB04-2"=w3906, "SET LAB04-2"=w3905, "TDMS LAB04-2"=w3908) -> (w3895:T37)  [unwired: 1 in]
                    n2344 = call "sub vi - cycle&temp fail v6.vi"("Amps Lo?"=w3907, "Input Cluster"=w3895, "SELECT"=w3904, "Amps Hi?"=w3903, "Result In"=w3897) -> ("(FAIL) out"=w3899:cluster{"FAIL LO":dbl, "FAIL HI":dbl}, "(DISP) out"=w3902:T4, "T-RISE"=w3896:cluster{"T-RISE (L)":dbl, "T-RISE (N)":dbl}, "Result Out"=w3898:bool, "file error"=w3901:errorcluster)  [unwired: 10 in]
                    n2345 = local write "TEMP RISE LAB04-2"(w3896) -> ()
                    n2346 = local write "FAIL LAB04-2"(w3899) -> ()
                    n2347 = local write "DISP LAB04-2"(w3902) -> ()
                    n2348 = local write "RESULT LAB04-2"(w3898) -> ()
                    n2349 = local write "data file error"(w3901) -> ()
                  }
                }
              }
              frame #8 {
                # "LAB05-1"
                n2350 = case shown="True" w3912 {
                  tunnel: w3914 -> [_ w3927]
                  tunnel: w3911 -> [_ w3924]
                  tunnel: w3913 -> [_ w3923]
                  frame False {
                  }
                  frame True {
                    n2351 = local read "TEMP START LAB05-1"() -> (w3929:cluster{"TL":dbl, "TN":dbl})
                    n2352 = local read "FAIL LAB05-1"() -> (w3920:cluster{"LO":dbl, "HI":dbl})
                    n2353 = local read "TDMS LAB05-1"() -> (w3928:refnum<k34>)
                    n2354 = local read "SET LAB05-1"() -> (w3925:T5)
                    n2355 = local read "DISP LAB05-1"() -> (w3926:T4)
                    n2356 = local read "SIG LAB05-1"() -> (w3930:T2)
                    n2357 = local read "RESULT LAB05-1"() -> (w3917:bool)
                    n2358 = Bundle("FAIL LAB05-1"=w3920, "SIG LAB05-1"=w3930, "TEMP START LAB05-1"=w3929, "DISP LAB05-1"=w3926, "SET LAB05-1"=w3925, "TDMS LAB05-1"=w3928) -> (w3915:T38)  [unwired: 1 in]
                    n2359 = call "sub vi - cycle&temp fail v6.vi"("Amps Lo?"=w3927, "Input Cluster"=w3915, "SELECT"=w3924, "Amps Hi?"=w3923, "Result In"=w3917) -> ("(FAIL) out"=w3919:cluster{"FAIL LO":dbl, "FAIL HI":dbl}, "(DISP) out"=w3922:T4, "T-RISE"=w3916:cluster{"T-RISE (L)":dbl, "T-RISE (N)":dbl}, "Result Out"=w3918:bool, "file error"=w3921:errorcluster)  [unwired: 10 in]
                    n2360 = local write "TEMP RISE LAB05-1"(w3916) -> ()
                    n2361 = local write "FAIL LAB05-1"(w3919) -> ()
                    n2362 = local write "DISP LAB05-1"(w3922) -> ()
                    n2363 = local write "RESULT LAB05-1"(w3918) -> ()
                    n2364 = local write "data file error"(w3921) -> ()
                  }
                }
              }
              frame #9 {
                # "LAB05-2"
                n2365 = case shown="True" w3932 {
                  tunnel: w3934 -> [_ w3947]
                  tunnel: w3931 -> [_ w3944]
                  tunnel: w3933 -> [_ w3943]
                  frame False {
                  }
                  frame True {
                    n2366 = local read "TEMP START LAB05-2"() -> (w3949:cluster{"TL":dbl, "TN":dbl})
                    n2367 = local read "FAIL LAB05-2"() -> (w3940:cluster{"LO":dbl, "HI":dbl})
                    n2368 = local read "TDMS LAB05-2"() -> (w3948:refnum<k34>)
                    n2369 = local read "SET LAB05-2"() -> (w3945:T5)
                    n2370 = local read "DISP LAB05-2"() -> (w3946:T4)
                    n2371 = local read "SIG LAB05-2"() -> (w3950:T2)
                    n2372 = local read "RESULT LAB05-2"() -> (w3937:bool)
                    n2373 = Bundle("FAIL LAB05-2"=w3940, "SIG LAB05-2"=w3950, "TEMP START LAB05-2"=w3949, "DISP LAB05-2"=w3946, "SET LAB05-2"=w3945, "TDMS LAB05-2"=w3948) -> (w3935:T39)  [unwired: 1 in]
                    n2374 = call "sub vi - cycle&temp fail v6.vi"("Amps Lo?"=w3947, "Input Cluster"=w3935, "SELECT"=w3944, "Amps Hi?"=w3943, "Result In"=w3937) -> ("(FAIL) out"=w3939:cluster{"FAIL LO":dbl, "FAIL HI":dbl}, "(DISP) out"=w3942:T4, "T-RISE"=w3936:cluster{"T-RISE (L)":dbl, "T-RISE (N)":dbl}, "Result Out"=w3938:bool, "file error"=w3941:errorcluster)  [unwired: 10 in]
                    n2375 = local write "TEMP RISE LAB05-2"(w3936) -> ()
                    n2376 = local write "FAIL LAB05-2"(w3939) -> ()
                    n2377 = local write "DISP LAB05-2"(w3942) -> ()
                    n2378 = local write "RESULT LAB05-2"(w3938) -> ()
                    n2379 = local write "data file error"(w3941) -> ()
                  }
                }
              }
            }
          }
          frame #16 {
            # "run calibration routine"
            n2380 = local read "CALIBRATE"() -> (w3951:bool)
            n2381 = case shown="True" w3951 {
              frame False {
              }
              frame True {
                n2382 = stacked-sequence {
                  seq-local: [w3952 _ _] -> [_ w3954 _]
                  frame #0 {
                    n2383 = call "CALIBRATION PASSWORD"() -> ("PASSWORD"=w3952:string)  [unwired: 17 in, 2 out]
                  }
                  frame #1 {
                    n2384 = Equal?(x=w3954, y="7777") -> (x = y?=w3953:bool)
                    n2385 = case shown="True" w3953 {
                      frame False {
                      }
                      frame True {
                        n2386 = stacked-sequence {
                          frame #0 {
                            n2387 = call "sub vi - calibration v1.vi"() -> ()  [unwired: 12 in]
                          }
                          frame #1 {
                            n2388 = call "sub vi - get calibration values v1.vi"() -> ("LAB01 (CAL)"=w3960:T7, "LAB02 (CAL)"=w3959:T8, "LAB03 (CAL)"=w3958:T7, "LAB04 (CAL)"=w3957:T7, "calibration file error out"=w3961:errorcluster, "LAB05 (CAL)"=w3956:T7)  [unwired: 10 in]
                            n2389 = local write "calibration file error out"(w3961) -> ()
                            n2390 = local write "CAL LAB04"(w3957) -> ()
                            n2391 = local write "CAL LAB05"(w3956) -> ()
                            n2392 = local write "CAL LAB01"(w3960) -> ()
                            n2393 = local write "CAL LAB02"(w3959) -> ()
                            n2394 = local write "CAL LAB03"(w3958) -> ()
                          }
                        }
                      }
                    }
                  }
                  frame #2 {
                    n2395 = local write "CALIBRATE"(FALSE) -> ()
                  }
                }
              }
            }
          }
          frame #17 {
            # "save certain settings to file"
            n2396 = String To Path(string="c:\\crabtree\\Set Up\\") -> (path=w3964:path)
            n2397 = Build Path(base path=w3964, name or relative path="settings.bin") -> (appended path=w3966:path)
            n2398 = Build Path(base path=w3964, name or relative path="mail.bin") -> (appended path=w3963:path)
            n2399 = Create Folder(path (use dialog)=w3964) -> (error out=w3969:errorcluster)  [unwired: 2 in, 2 out]
            n2400 = call <vilib>:"Clear Errors.vi"("error in (no error)"=w3969) -> ()  [unwired: 6 in, 1 out]
            n2401 = stacked-sequence {
              seq-local: [w3974 _] -> [_ w3987]
              tunnel: w3966 -> [_ w3988]
              tunnel: w3963 -> [_ w3986]
              frame #0 {
                n2402 = local read "C drive data root dir"() -> (w3973:path)
                n2403 = local read "Select COM port"() -> (w3970:refnum<visa-resource-name>)
                n2404 = local read "Network Directory"() -> (w3979:path)
                n2405 = local read "SET LAB05-2"() -> (w3978:T5)
                n2406 = local read "SET LAB05-1"() -> (w3977:T5)
                n2407 = local read "SET LAB04-2"() -> (w3976:T5)
                n2408 = local read "SET LAB03-2"() -> (w3980:T5)
                n2409 = local read "SET LAB04-1"() -> (w3975:T5)
                n2410 = local read "SET LAB03-1"() -> (w3981:T5)
                n2411 = local read "SET LAB02-2"() -> (w3982:T5)
                n2412 = local read "SET LAB02-1"() -> (w3983:T5)
                n2413 = local read "SET LAB01-2"() -> (w3984:T5)
                n2414 = local read "SET LAB01-1"() -> (w3985:T5)
                n2415 = local read "RATE (Hz)"() -> (w3972:dbl)
                n2416 = local read "SAMPLES"() -> (w3971:dbl)
                n2417 = Bundle("SET LAB01-1"=w3985, "SET LAB01-2"=w3984, "SET LAB02-1"=w3983, "SET LAB02-2"=w3982, "SET LAB03-1"=w3981, "SET LAB03-2"=w3980, "SET LAB04-1"=w3975, "SET LAB04-2"=w3976, "SET LAB05-1"=w3977, "SET LAB05-2"=w3978, "Network Directory"=w3979, "C drive data root dir"=w3973, "RATE (Hz)"=w3972, "SAMPLES"=w3971, "Select COM port"=w3970) -> (w3974:T19)  [unwired: 1 in]
              }
              frame #1 {
                n2418 = event shown="[1] \"SET LAB01-1\", \"SET LAB01-2\", \"SET LAB02-1\", \"SET LAB02-2\", \"SET LAB03-1\", \"SET LAB03-2\", \"SET LAB04-1\", \"SET LAB04-2\", \"SET LAB05-1\", \"SET LAB05-2\", \"Network Directory\", \"C drive data root dir\", \"RATE (Hz)\", \"SAMPLES\", \"Select COM port\": Value Change" {
                  selector: _ -> [_ _ _]
                  dyn-events: _ -> [_ _ _]
                  timeout: 10.0 -> [_ _ _]
                  tunnel: w3988 -> [_ w3990 _]
                  tunnel: w3987 -> [_ w3991 _]
                  tunnel: w3986 -> [_ _ w4002]
                  event Timeout {
                    n2419 = event-data() -> ()  [unwired: 1 in, 3 out]
                  }
                  event "SET LAB01-1", "SET LAB01-2", "SET LAB02-1", "SET LAB02-2", "SET LAB03-1", "SET LAB03-2", "SET LAB04-1", "SET LAB04-2", "SET LAB05-1", "SET LAB05-2", "Network Directory", "C drive data root dir", "RATE (Hz)", "SAMPLES", "Select COM port": Value Change {
                    n2420 = event-data() -> ()  [unwired: 1 in, 6 out]
                    n2421 = Open/Create/Replace File(file path (use dialog)=w3990, operation (0:open)=T18."replace or create") -> (refnum out=w3996:refnum<file>, error out=w3995:errorcluster)  [unwired: 4 in, 1 out]
                    n2422 = Write to Binary File(file (use dialog)=w3996, data=w3991, error in=w3995) -> (refnum out=w3994:refnum<file>, error out=w3993:errorcluster)  [unwired: 3 in, 1 out]
                    n2423 = Close File(refnum=w3994, error in=w3993) -> (error out=w3992:errorcluster)  [unwired: 1 out]
                    n2424 = local write "data file error"(w3992) -> ()
                  }
                  event "MAIL SETTINGS.OUT SERVER ADDRESS", "MAIL SETTINGS.FROM ACCOUNT", "MAIL SETTINGS.USER NAME", "MAIL SETTINGS.PASSWORD", "Auto Mail Send", "TO (string):": Value Change {
                    n2425 = event-data() -> ()  [unwired: 1 in, 6 out]
                    n2426 = local read "MAIL SETTINGS"() -> (w4001:T6)
                    n2427 = local read "Auto Mail Send"() -> (w3999:bool)
                    n2428 = local read "TO (string):"() -> (w3998:string)
                    n2429 = Open/Create/Replace File(file path (use dialog)=w4002, operation (0:open)=T18."replace or create") -> (refnum out=w4007:refnum<file>, error out=w4006:errorcluster)  [unwired: 4 in, 1 out]
                    n2430 = Bundle("MAIL SETTINGS"=w4001, "Auto Mail Send"=w3999, "TO (string):"=w3998) -> (w4000:T40)  [unwired: 1 in]
                    n2431 = Write to Binary File(file (use dialog)=w4007, data=w4000, error in=w4006) -> (refnum out=w4005:refnum<file>, error out=w4004:errorcluster)  [unwired: 3 in, 1 out]
                    n2432 = Close File(refnum=w4005, error in=w4004) -> (error out=w4003:errorcluster)  [unwired: 1 out]
                    n2433 = local write "data file error"(w4003) -> ()
                  }
                }
              }
            }
          }
          frame #18 {
            # "mail control"
            n2434 = local read "MAIL SETTINGS"() -> (w4024:T6)
            n2435 = local read "Auto Mail Send"() -> (w4010:bool)
            n2436 = Unbundle(w4024) -> ("OUT SERVER ADDRESS"=w4023:string, "FROM ACCOUNT"=w4022:string, "TEST MAIL"=w4021:bool)  [unwired: 4 out]
            n2437 = stacked-sequence {
              tunnel: "TO (string):" -> [_ w4063]
              tunnel: w4024 -> [w4029 w4062]
              tunnel: w4023 -> [w4028 w4061]
              tunnel: w4022 -> [w4027 w4060]
              tunnel: w4021 -> [w4026 _]
              tunnel: w4010 -> [_ w4059]
              tunnel: w4020 -> [_ w4058]
              tunnel: w4019 -> [_ w4057]
              tunnel: w4018 -> [_ w4056]
              tunnel: w4017 -> [_ w4055]
              tunnel: w4016 -> [_ w4054]
              tunnel: w4015 -> [_ w4053]
              tunnel: w4014 -> [_ w4052]
              tunnel: w4013 -> [_ w4051]
              tunnel: w4012 -> [_ w4050]
              tunnel: w4011 -> [_ w4049]
              tunnel: "TO (string):" -> [w4025 _]
              frame #0 {
                # "mail test"
                n2438 = case shown="True" w4026 {
                  tunnel: w4029 -> [_ w4033]
                  tunnel: w4025 -> [_ w4032]
                  tunnel: w4028 -> [_ w4031]
                  tunnel: w4027 -> [_ w4030]
                  frame False {
                  }
                  frame True {
                    n2439 = stacked-sequence {
                      seq-local: [_ _ w4043 _] -> [_ _ _ w4044]
                      tunnel: w4033 -> [w4036 _ _ w4048]
                      tunnel: w4032 -> [_ _ w4041 _]
                      tunnel: w4031 -> [_ _ w4039 _]
                      tunnel: w4030 -> [_ _ w4040 _]
                      frame #0 {
                        n2440 = Bundle(cluster=w4036, "TEST MAIL STATUS"="TEST START") -> (w4034:T6)  [unwired: 6 in]
                        n2441 = local write "MAIL SETTINGS"(w4034) -> ()
                      }
                      frame #1 {
                        n2442 = Wait (ms)(milliseconds to wait=500) -> ()  [unwired: 1 out]
                      }
                      frame #2 {
                        n2443 = call "sub vi - send mail with attach v5.vi"("TO:"=w4041, "subject"="MAIL TEST FROM LAB PANEL", "from"=w4040, "out going server"=w4039, "message"="TEST MESSAGE") -> ("error out"=w4043:errorcluster)  [unwired: 10 in]
                      }
                      frame #3 {
                        n2444 = Bundle(cluster=w4048, "TEST MAIL"=FALSE, "TEST MAIL STATUS"="TEST END", "mail error"=w4044) -> (w4046:T6)  [unwired: 4 in]
                        n2445 = local write "MAIL SETTINGS"(w4046) -> ()
                      }
                    }
                  }
                }
              }
              frame #1 {
                # "mail report"
                n2446 = stacked-sequence {
                  seq-local: [_ w4128 _ _] -> [_ _ _ w4296]
                  seq-local: [_ _ w4209 _] -> [_ _ _ w4286]
                  seq-local: [w4073 _ _ _] -> [_ w4122 _ _]
                  seq-local: [w4072 _ _ _] -> [_ w4121 _ _]
                  seq-local: [w4070 _ _ _] -> [_ w4119 _ _]
                  seq-local: [w4071 _ _ _] -> [_ w4120 _ _]
                  seq-local: [w4069 _ _ _] -> [_ w4118 _ _]
                  seq-local: [w4068 _ _ _] -> [_ w4113 _ _]
                  seq-local: [w4067 _ _ _] -> [_ w4114 _ _]
                  seq-local: [w4066 _ _ _] -> [_ w4115 _ _]
                  seq-local: [w4065 _ _ _] -> [_ w4116 _ _]
                  seq-local: [w4064 _ _ _] -> [_ w4117 _ _]
                  tunnel: w4063 -> [_ _ _ w4297]
                  tunnel: w4062 -> [_ _ _ w4280]
                  tunnel: w4061 -> [_ _ _ w4294]
                  tunnel: w4060 -> [_ _ _ w4293]
                  tunnel: w4059 -> [w4104 _ _ w4288]
                  tunnel: w4058 -> [_ _ w4239 _]
                  tunnel: w4057 -> [_ _ w4236 _]
                  tunnel: w4056 -> [_ _ w4235 _]
                  tunnel: w4055 -> [_ _ w4234 _]
                  tunnel: w4054 -> [_ _ w4233 _]
                  tunnel: w4053 -> [_ _ w4232 _]
                  tunnel: w4052 -> [_ _ w4231 _]
                  tunnel: w4051 -> [_ _ w4230 _]
                  tunnel: w4050 -> [_ _ w4229 _]
                  tunnel: w4049 -> [_ _ w4228 _]
                  frame #0 {
                    n2447 = case shown="False" w4104 {
                      frame False {
                        n2448 = local write "mail control"("") -> ()
                      }
                      frame True {
                      }
                    }
                    n2449 = local read "SET LAB01-1"() -> (w4103:T5)
                    n2450 = local read "SET LAB01-2"() -> (w4102:T5)
                    n2451 = local read "SET LAB02-1"() -> (w4101:T5)
                    n2452 = local read "SET LAB02-2"() -> (w4100:T5)
                    n2453 = local read "SET LAB03-1"() -> (w4099:T5)
                    n2454 = local read "SET LAB04-1"() -> (w4097:T5)
                    n2455 = local read "SET LAB05-1"() -> (w4095:T5)
                    n2456 = local read "SET LAB03-2"() -> (w4098:T5)
                    n2457 = local read "SET LAB04-2"() -> (w4096:T5)
                    n2458 = local read "SET LAB05-2"() -> (w4094:T5)
                    n2459 = Unbundle(w4099) -> ("DESCRIPTION"=w4079:string)  [unwired: 4 out]
                    n2460 = Unbundle(w4098) -> ("DESCRIPTION"=w4078:string)  [unwired: 4 out]
                    n2461 = Unbundle(w4097) -> ("DESCRIPTION"=w4077:string)  [unwired: 4 out]
                    n2462 = Unbundle(w4094) -> ("DESCRIPTION"=w4074:string)  [unwired: 4 out]
                    n2463 = Unbundle(w4100) -> ("DESCRIPTION"=w4080:string)  [unwired: 4 out]
                    n2464 = Unbundle(w4096) -> ("DESCRIPTION"=w4076:string)  [unwired: 4 out]
                    n2465 = Unbundle(w4103) -> ("DESCRIPTION"=w4092:string)  [unwired: 4 out]
                    n2466 = Unbundle(w4101) -> ("DESCRIPTION"=w4081:string)  [unwired: 4 out]
                    n2467 = Unbundle(w4095) -> ("DESCRIPTION"=w4075:string)  [unwired: 4 out]
                    n2468 = Unbundle(w4102) -> ("DESCRIPTION"=w4082:string)  [unwired: 4 out]
                    n2469 = Concatenate Strings("[LAB05-1/", w4074) -> (w4064:string)
                    n2470 = Concatenate Strings("[LAB05-2/", w4075) -> (w4065:string)
                    n2471 = Concatenate Strings("[LAB04-2/", w4076) -> (w4066:string)
                    n2472 = Concatenate Strings("[LAB03-2/", w4078) -> (w4068:string)
                    n2473 = Concatenate Strings("[LAB04-1/", w4077) -> (w4067:string)
                    n2474 = Concatenate Strings("[LAB03-1/", w4079) -> (w4069:string)
                    n2475 = Concatenate Strings("[LAB01-2/", w4082) -> (w4072:string)
                    n2476 = Concatenate Strings("[LAB02-2/", w4080) -> (w4070:string)
                    n2477 = Concatenate Strings("[LAB01-1/", w4092) -> (w4073:string)
                    n2478 = Concatenate Strings("[LAB02-1/", w4081) -> (w4071:string)
                  }
                  frame #1 {
                    w4126 = "/"
                    w4127 = 2.0
                    n2479 = local read "DISP LAB01-2"() -> (w4207:T4)
                    n2480 = local read "DISP LAB01-1"() -> (w4208:T4)
                    n2481 = local read "DISP LAB02-1"() -> (w4206:T4)
                    n2482 = local read "DISP LAB03-2"() -> (w4203:T4)
                    n2483 = local read "DISP LAB02-2"() -> (w4205:T4)
                    n2484 = local read "DISP LAB03-1"() -> (w4204:T4)
                    n2485 = local read "DISP LAB04-2"() -> (w4201:T4)
                    n2486 = local read "DISP LAB04-1"() -> (w4202:T4)
                    n2487 = local read "DISP LAB05-1"() -> (w4200:T4)
                    n2488 = local read "DISP LAB05-2"() -> (w4199:T4)
                    n2489 = Unbundle(w4207) -> ("CYCLE"=w4191:dbl, "MINS"=w4190:dbl, "STATUS"=w4187:string)
                    n2490 = Unbundle(w4208) -> ("CYCLE"=w4196:dbl, "MINS"=w4195:dbl, "STATUS"=w4192:string)
                    n2491 = Unbundle(w4206) -> ("CYCLE"=w4184:dbl, "MINS"=w4183:dbl, "STATUS"=w4182:string)
                    n2492 = Unbundle(w4203) -> ("CYCLE"=w4171:dbl, "MINS"=w4170:dbl, "STATUS"=w4167:string)
                    n2493 = Unbundle(w4204) -> ("CYCLE"=w4176:dbl, "MINS"=w4175:dbl, "STATUS"=w4172:string)
                    n2494 = Unbundle(w4205) -> ("CYCLE"=w4181:dbl, "MINS"=w4180:dbl, "STATUS"=w4177:string)
                    n2495 = Unbundle(w4202) -> ("CYCLE"=w4166:dbl, "MINS"=w4165:dbl, "STATUS"=w4162:string)
                    n2496 = Unbundle(w4201) -> ("CYCLE"=w4161:dbl, "MINS"=w4160:dbl, "STATUS"=w4157:string)
                    n2497 = Unbundle(w4200) -> ("CYCLE"=w4156:dbl, "MINS"=w4155:dbl, "STATUS"=w4152:string)
                    n2498 = Unbundle(w4199) -> ("CYCLE"=w4198:dbl, "MINS"=w4197:dbl, "STATUS"=w4149:string)
                    n2499 = Number To Decimal String(number=w4184) -> (decimal integer string=w4186:string)  [unwired: 1 in]
                    n2500 = Number To Decimal String(number=w4181) -> (decimal integer string=w4179:string)  [unwired: 1 in]
                    n2501 = Number To Decimal String(number=w4176) -> (decimal integer string=w4174:string)  [unwired: 1 in]
                    n2502 = Number To Decimal String(number=w4191) -> (decimal integer string=w4189:string)  [unwired: 1 in]
                    n2503 = Number To Decimal String(number=w4171) -> (decimal integer string=w4169:string)  [unwired: 1 in]
                    n2504 = Number To Decimal String(number=w4196) -> (decimal integer string=w4194:string)  [unwired: 1 in]
                    n2505 = Number To Decimal String(number=w4198) -> (decimal integer string=w4151:string)  [unwired: 1 in]
                    n2506 = Number To Decimal String(number=w4166) -> (decimal integer string=w4164:string)  [unwired: 1 in]
                    n2507 = Number To Decimal String(number=w4161) -> (decimal integer string=w4159:string)  [unwired: 1 in]
                    n2508 = Number To Decimal String(number=w4156) -> (decimal integer string=w4154:string)  [unwired: 1 in]
                    n2509 = Number To Fractional String(number=w4183, precision (6)=w4127) -> (F-format string=w4185:string)  [unwired: 2 in]
                    n2510 = Number To Fractional String(number=w4170, precision (6)=w4127) -> (F-format string=w4168:string)  [unwired: 2 in]
                    n2511 = Number To Fractional String(number=w4180, precision (6)=w4127) -> (F-format string=w4178:string)  [unwired: 2 in]
                    n2512 = Number To Fractional String(number=w4175, precision (6)=w4127) -> (F-format string=w4173:string)  [unwired: 2 in]
                    n2513 = Number To Fractional String(number=w4160, precision (6)=w4127) -> (F-format string=w4158:string)  [unwired: 2 in]
                    n2514 = Number To Fractional String(number=w4165, precision (6)=w4127) -> (F-format string=w4163:string)  [unwired: 2 in]
                    n2515 = Number To Fractional String(number=w4190, precision (6)=w4127) -> (F-format string=w4188:string)  [unwired: 2 in]
                    n2516 = Number To Fractional String(number=w4155, precision (6)=w4127) -> (F-format string=w4153:string)  [unwired: 2 in]
                    n2517 = Number To Fractional String(number=w4195, precision (6)=w4127) -> (F-format string=w4193:string)  [unwired: 2 in]
                    n2518 = Number To Fractional String(number=w4197, precision (6)=w4127) -> (F-format string=w4150:string)  [unwired: 2 in]
                    n2519 = Concatenate Strings(w4126, w4169, w4126, w4168, w4126, w4167) -> (w4143:string)
                    n2520 = Concatenate Strings(w4126, w4164, w4126, w4163, w4126, w4162) -> (w4142:string)
                    n2521 = Concatenate Strings(w4126, w4159, w4126, w4158, w4126, w4157) -> (w4141:string)
                    n2522 = Concatenate Strings(w4126, w4154, w4126, w4153, w4126, w4152) -> (w4140:string)
                    n2523 = Concatenate Strings(w4126, w4151, w4126, w4150, w4126, w4149) -> (w4139:string)
                    n2524 = Concatenate Strings(w4126, w4194, w4126, w4193, w4126, w4192) -> (w4148:string)
                    n2525 = Concatenate Strings(w4126, w4174, w4126, w4173, w4126, w4172) -> (w4144:string)
                    n2526 = Concatenate Strings(w4126, w4189, w4126, w4188, w4126, w4187) -> (w4147:string)
                    n2527 = Concatenate Strings(w4126, w4186, w4126, w4185, w4126, w4182) -> (w4146:string)
                    n2528 = Concatenate Strings(w4126, w4179, w4126, w4178, w4126, w4177) -> (w4145:string)
                    n2529 = Concatenate Strings("]", "\r") -> (w4123:string)
                    n2530 = Concatenate Strings(w4118, w4144, w4123) -> (w4134:string)
                    n2531 = Concatenate Strings(w4120, w4146, w4123) -> (w4136:string)
                    n2532 = Concatenate Strings(w4119, w4145, w4123) -> (w4135:string)
                    n2533 = Concatenate Strings(w4115, w4141, w4123) -> (w4131:string)
                    n2534 = Concatenate Strings(w4116, w4140, w4123) -> (w4132:string)
                    n2535 = Concatenate Strings(w4114, w4142, w4123) -> (w4130:string)
                    n2536 = Concatenate Strings(w4113, w4143, w4123) -> (w4129:string)
                    n2537 = Concatenate Strings(w4117, w4139, w4123) -> (w4133:string)
                    n2538 = Concatenate Strings(w4121, w4147, w4123) -> (w4137:string)
                    n2539 = Concatenate Strings(w4122, w4148, w4123) -> (w4138:string)
                    n2540 = Concatenate Strings(w4138, w4137, w4136, w4135, w4134, w4129, w4130, w4131, w4132, w4133) -> (w4106:string)
                    n2541 = Concatenate Strings("[PANEL/", "DESC/", "CYCLES/", "MINS/", "STATUS]", "\r", w4106) -> (w4128:string)
                    "MAIL REPORT" <- w4128
                  }
                  frame #2 {
                    w4237 = "END"
                    n2542 = local read "mail control"() -> (w4238:string)
                    n2543 = case shown="False" w4233 {
                      tunnel: w4238 -> [w4262 _]
                      tunnel: w4237 -> [w4261 _]
                      tunnel: [w4260 FALSE] -> w4223
                      frame False {
                        n2544 = Equal?(x=w4262, y=w4261) -> (x = y?=w4260:bool)
                      }
                      frame True {
                      }
                    }
                    n2545 = case shown="False" w4239 {
                      tunnel: w4238 -> [w4278 _]
                      tunnel: w4237 -> [w4277 _]
                      tunnel: [w4276 FALSE] -> w4227
                      frame False {
                        n2546 = Equal?(x=w4278, y=w4277) -> (x = y?=w4276:bool)
                      }
                      frame True {
                      }
                    }
                    n2547 = case shown="False" w4236 {
                      tunnel: w4238 -> [w4274 _]
                      tunnel: w4237 -> [w4273 _]
                      tunnel: [w4272 FALSE] -> w4226
                      frame False {
                        n2548 = Equal?(x=w4274, y=w4273) -> (x = y?=w4272:bool)
                      }
                      frame True {
                      }
                    }
                    n2549 = case shown="False" w4234 {
                      tunnel: w4238 -> [w4266 _]
                      tunnel: w4237 -> [w4265 _]
                      tunnel: [w4264 FALSE] -> w4224
                      frame False {
                        n2550 = Equal?(x=w4266, y=w4265) -> (x = y?=w4264:bool)
                      }
                      frame True {
                      }
                    }
                    n2551 = case shown="False" w4235 {
                      tunnel: w4238 -> [w4270 _]
                      tunnel: w4237 -> [w4269 _]
                      tunnel: [w4268 FALSE] -> w4225
                      frame False {
                        n2552 = Equal?(x=w4270, y=w4269) -> (x = y?=w4268:bool)
                      }
                      frame True {
                      }
                    }
                    n2553 = Or(x=w4225, y=w4224) -> (x .or. y?=w4216:bool)
                    n2554 = Or(x=w4227, y=w4226) -> (x .or. y?=w4217:bool)
                    n2555 = Or(x=w4217, y=w4216) -> (x .or. y?=w4212:bool)
                    n2556 = case shown="False" w4229 {
                      tunnel: w4238 -> [w4246 _]
                      tunnel: w4237 -> [w4245 _]
                      tunnel: [w4244 FALSE] -> w4218
                      frame False {
                        n2557 = Equal?(x=w4246, y=w4245) -> (x = y?=w4244:bool)
                      }
                      frame True {
                      }
                    }
                    n2558 = case shown="False" w4228 {
                      tunnel: w4238 -> [w4242 _]
                      tunnel: w4237 -> [w4241 _]
                      tunnel: [w4240 FALSE] -> w4222
                      frame False {
                        n2559 = Equal?(x=w4242, y=w4241) -> (x = y?=w4240:bool)
                      }
                      frame True {
                      }
                    }
                    n2560 = case shown="False" w4230 {
                      tunnel: w4238 -> [w4250 _]
                      tunnel: w4237 -> [w4249 _]
                      tunnel: [w4248 FALSE] -> w4219
                      frame False {
                        n2561 = Equal?(x=w4250, y=w4249) -> (x = y?=w4248:bool)
                      }
                      frame True {
                      }
                    }
                    n2562 = case shown="False" w4232 {
                      tunnel: w4238 -> [w4258 _]
                      tunnel: w4237 -> [w4257 _]
                      tunnel: [w4256 FALSE] -> w4221
                      frame False {
                        n2563 = Equal?(x=w4258, y=w4257) -> (x = y?=w4256:bool)
                      }
                      frame True {
                      }
                    }
                    n2564 = case shown="False" w4231 {
                      tunnel: w4238 -> [w4254 _]
                      tunnel: w4237 -> [w4253 _]
                      tunnel: [w4252 FALSE] -> w4220
                      frame False {
                        n2565 = Equal?(x=w4254, y=w4253) -> (x = y?=w4252:bool)
                      }
                      frame True {
                      }
                    }
                    n2566 = Or(x=w4221, y=w4220) -> (x .or. y?=w4215:bool)
                    n2567 = Or(x=w4219, y=w4218) -> (x .or. y?=w4214:bool)
                    n2568 = Or(x=w4222, y=w4223) -> (x .or. y?=w4210:bool)
                    n2569 = Or(x=w4215, y=w4214) -> (x .or. y?=w4213:bool)
                    n2570 = Or(x=w4212, y=w4213) -> (x .or. y?=w4211:bool)
                    n2571 = Or(x=w4211, y=w4210) -> (x .or. y?=w4209:bool)
                  }
                  frame #3 {
                    n2572 = local read "on loops"() -> (w4292:dbl)
                    n2573 = local read "jig cycle"() -> (w4289:dbl)
                    n2574 = local read "Send Mail Now"() -> (w4283:bool)
                    n2575 = Add(x=w4292, y=3.0) -> (x+y=w4290:dbl)
                    n2576 = Equal?(x=w4289, y=w4290) -> (x = y?=w4284:bool)
                    n2577 = And(x=w4284, y=w4283) -> (x .and. y?=w4282:bool)
                    n2578 = And(x=w4288, y=w4284) -> (x .and. y?=w4287:bool)
                    n2579 = And(x=w4287, y=w4286) -> (x .and. y?=w4285:bool)
                    n2580 = Or(x=w4285, y=w4282) -> (x .or. y?=w4281:bool)
                    n2581 = case shown="True" w4281 {
                      tunnel: w4297 -> [_ w4303]
                      tunnel: w4296 -> [_ w4302]
                      tunnel: "Lab Panel Test Status" -> [_ w4301]
                      tunnel: w4294 -> [_ w4300]
                      tunnel: w4293 -> [_ w4299]
                      tunnel: w4280 -> [_ w4298]
                      frame False {
                      }
                      frame True {
                        n2582 = stacked-sequence {
                          tunnel: w4303 -> [w4311 _]
                          tunnel: w4302 -> [w4310 _]
                          tunnel: w4301 -> [w4309 _]
                          tunnel: w4300 -> [w4308 _]
                          tunnel: w4299 -> [w4307 _]
                          tunnel: w4298 -> [w4306 _]
                          frame #0 {
                            n2583 = call "sub vi - send mail with attach v5.vi"("TO:"=w4311, "subject"=w4309, "from"=w4307, "out going server"=w4308, "message"=w4310) -> ("error out"=w4305:errorcluster)  [unwired: 10 in]
                            n2584 = Bundle(cluster=w4306, "mail error"=w4305) -> (w4304:T6)  [unwired: 6 in]
                            n2585 = local write "MAIL SETTINGS"(w4304) -> ()
                          }
                          frame #1 {
                            n2586 = local write "mail control"("") -> ()
                            n2587 = local write "Send Mail Now"(FALSE) -> ()
                          }
                        }
                      }
                    }
                  }
                }
              }
            }
          }
        }
        n2588 = node-c288() -> ()  [unwired: 1 in, 1 out]
        "loops" <- w167
        "stop2" <- "stop"
      }
      n2589 = node-c288(w144) -> ()  [unwired: 1 out]
    }
  }
